vi "Path Generator.vi"() -> ()   [LabVIEW 2016]
uses:
  VIs/Waypoint.ctl
  VIs/Segment.ctl
  Constants/Private/Private Global.vi
  Pathfinder.lvlib
  Constants/Constants.lvlib
panel:
  in  "Name":string
  out "original":T1[](array[typedef])
  in  "Rear First?":bool=TRUE
  out "left":T1[](array[typedef])=[{"dt"=0.005, "x"=-0.0008758536007823281, "y"=232.00000002739714, "position"=-5.8139534883720933e-05, "velocity"=-0.023255813953488372, "acceleration"=-4.651162790697675, "jerk"=-930.232558139535, "heading"=-6.283122746208061}, {"dt"=0.005, "x"=-0.0008602070905170062, "y"=232.00000002642702, "position"=-7.378604517911754e-05, "velocity"=-0.003129302059079322, "acceleration"=4.02530237888181, "jerk"=1735.293033915897, "heading"=-6.2831238638159395}, {"dt"=0.005, "x"=-0.00082500305296863, "y"=232.0000000243082, "position"=-0.00010899008279125573, "velocity"=-0.007040807522427639, "acceleration"=-0.7823010926696634, "jerk"=-961.5206943102947, "heading"=-6.283126378390055}, {"dt"=0.005, "x"=-0.0007624201846368434, "y"=232.00000002076015, "position"=-0.0001715729512236183, "velocity"=-0.012516573686472514, "acceleration"=-1.095153232808975, "jerk"=-62.57042802786232, "heading"=-6.283130848594943}, {"dt"=0.005, "x"=-0.0006646398015586345, "y"=232.00000001577664, "position"=-0.0002693533344288234, "velocity"=-0.019556076641041014, "acceleration"=-1.4079005909137, "jerk"=-62.54947162094497, "heading"=-6.283137832908029}, {"dt"=0.005, "x"=-0.0005238475090722906, "y"=232.00000000980057, "position"=-0.0004101456270419971, "velocity"=-0.02815845852263474, "acceleration"=-1.7204763763187447, "jerk"=-62.515157081008965, "heading"=-6.283147889500358}, {"dt"=0.005, "x"=-0.00033223528885417756, "y"=232.00000000394215, "position"=-0.000601757847349669, "velocity"=-0.038322444061534386, "acceleration"=-2.0327971077799294, "jerk"=-62.46414629223693, "heading"=-6.283161576087523}, {"dt"=0.005, "x"=-8.200400317489167e-05, "y"=232.00000000024016, "position"=-0.000851989133056339, "velocity"=-0.05004625714133398, "acceleration"=-2.3447626159599193, "jerk"=-62.39310163599798, "heading"=-6.283179449750788}, {"dt"=0.005, "x"=0.0037243748096527536, "y"=232.0000000312099, "position"=-0.0046583679460099735, "velocity"=-0.7612757625907269, "acceleration"=-142.24590108987857, "jerk"=-27980.22769478373, "heading"=-1.6759390957965525e-05}, {"dt"=0.005, "x"=0.009929139702494224, "y"=232.00000022180532, "position"=-0.01086313284177876, "velocity"=-1.2409529791537575, "acceleration"=-95.9354433126061, "jerk"=9262.091555454495, "heading"=-4.4674576916869935e-05}, {"dt"=0.005, "x"=0.017436765282922654, "y"=232.00000068396733, "position"=-0.018370758436432308, "velocity"=-1.5015251189307095, "acceleration"=-52.114427955390404, "jerk"=8764.203071443138, "heading"=-7.844169176274285e-05}, {"dt"=0.005, "x"=0.02637126360589169, "y"=232.00000156426964, "position"=-0.027305256802768758, "velocity"=-1.78689967326729, "acceleration"=-57.074910867316085, "jerk"=-992.0965823851361, "heading"=-0.00011861272284025004}, {"dt"=0.005, "x"=0.0368565745058633, "y"=232.00000305503744, "position"=-0.03779056780871665, "velocity"=-2.097062201189579, "acceleration"=-62.03250558445781, "jerk"=-991.5189434283448, "heading"=-0.00016573742479814024}, {"dt"=0.005, "x"=0.04901668599989321, "y"=232.00000540258077, "position"=-0.04995067952934644, "velocity"=-2.432022344125958, "acceleration"=-66.99202858727577, "jerk"=-991.904600563592, "heading"=-0.00022036351598547776}, {"dt"=0.005, "x"=0.06297549095104837, "y"=232.00000891604873, "position"=-0.06390948492267617, "velocity"=-2.7917610786659455, "acceleration"=-71.94774690799753, "jerk"=-991.1436641443515, "heading"=-0.0002830356608759521}, {"dt"=0.005, "x"=0.07879481410486276, "y"=232.00001395498225, "position"=-0.07972880887901701, "velocity"=-3.163864791268167, "acceleration"=-74.42074252044435, "jerk"=-494.5991224893646, "heading"=-0.00035401708800802956}, {"dt"=0.005, "x"=0.09647442256013375, "y"=232.0000209147114, "position"=-0.09740841870416642, "velocity"=-3.5359219650298797, "acceleration"=-74.41143475234249, "jerk"=1.861553620372547, "heading"=-0.0004332902398125893}, {"dt"=0.005, "x"=0.11601398667715579, "y"=232.00003023642586, "position"=-0.11694798504473743, "velocity"=-3.9079132681142026, "acceleration"=-74.39826061686459, "jerk"=2.6348270955793396, "heading"=-0.0005208351885473417}, {"dt"=0.005, "x"=0.1374132670186076, "y"=232.00004240705323, "position"=-0.13834726884715046, "velocity"=-4.279856760482604, "acceleration"=-74.38869847368021, "jerk"=1.9124286368764842, "heading"=-0.000616630476134028}, {"dt"=0.005, "x"=0.16067187478210984, "y"=232.00005795891641, "position"=-0.16160588181002714, "velocity"=-4.651722592575338, "acceleration"=-74.37316641854679, "jerk"=3.106411026683986, "heading"=-0.0007206520430999008}, {"dt"=0.005, "x"=0.18578949376598203, "y"=232.00007746960773, "position"=-0.1867235083715885, "velocity"=-5.02352531231227, "acceleration"=-74.3605439473864, "jerk"=2.5244942320767905, "heading"=-0.0008328742248462917}, {"dt"=0.005, "x"=0.21276571116641288, "y"=232.00010156161397, "position"=-0.21369973653010008, "velocity"=-5.395245631702316, "acceleration"=-74.34406387800934, "jerk"=3.2960138754134505, "heading"=-0.0009532689972410191}, {"dt"=0.005, "x"=0.24160009922129633, "y"=232.0001309020737, "position"=-0.24253413951268638, "velocity"=-5.76688059651726, "acceleration"=-74.32699296298874, "jerk"=3.414183004119309, "heading"=-0.001081806344908287}, {"dt"=0.005, "x"=0.27229221516971464, "y"=232.00016620247234, "position"=-0.2732262757613951, "velocity"=-6.138427249741739, "acceleration"=-74.30933064489587, "jerk"=3.532463618574866, "heading"=-0.0012184542638269957}, {"dt"=0.005, "x"=0.30484160120819287, "y"=232.0002082183179, "position"=-0.30577568891759743, "velocity"=-6.509882631240475, "acceleration"=-74.29107629974716, "jerk"=3.6508690297409885, "heading"=-0.0013631787640525084}, {"dt"=0.005, "x"=0.33924770411668914, "y"=232.00025774867527, "position"=-0.3401818274775454, "velocity"=-6.881227711989586, "acceleration"=-74.26901614982224, "jerk"=4.412029984985111, "heading"=-0.0015159435161616885}, {"dt"=0.005, "x"=0.3755100406127911, "y"=232.00031563601584, "position"=-0.3764442101778138, "velocity"=-7.2524765400536815, "acceleration"=-74.24976561281902, "jerk"=3.85010740064331, "heading"=-0.0016767105896903223}, {"dt"=0.005, "x"=0.4136279823684332, "y"=232.0003827655038, "position"=-0.4145622110442637, "velocity"=-7.623600173289979, "acceleration"=-74.22472664725959, "jerk"=5.007793111886372, "heading"=-0.0018454395028453252}, {"dt"=0.005, "x"=0.4536009877800924, "y"=232.00046006494864, "position"=-0.45453529119634495, "velocity"=-7.994616030416249, "acceleration"=-74.20317142525387, "jerk"=4.311044401143249, "heading"=-0.0020220882541658325}, {"dt"=0.005, "x"=0.49542842005744236, "y"=232.0005485040674, "position"=-0.49636281697057677, "velocity"=-8.365505154846364, "acceleration"=-74.17782488602302, "jerk"=5.069307846170545, "heading"=-0.002206612520756379}, {"dt"=0.005, "x"=0.5391096274920242, "y"=232.0006490941584, "position"=-0.5400441402255948, "velocity"=-8.73626465100359, "acceleration"=-74.15189923144538, "jerk"=5.18513091552677, "heading"=-0.0023989660184867145}, {"dt"=0.005, "x"=0.5846439433956321, "y"=232.0007628876348, "position"=-0.5855785983179541, "velocity"=-9.106891618471872, "acceleration"=-74.12539349365623, "jerk"=5.301147557830177, "heading"=-0.0025991005059064487}, {"dt"=0.005, "x"=0.6320306093513414, "y"=232.0008909773236, "position"=-0.6329654373913335, "velocity"=-9.477367814675867, "acceleration"=-74.09523924079906, "jerk"=6.030850571434598, "heading"=-0.0028069654522328014}, {"dt"=0.005, "x"=0.6812689450670211, "y"=232.0010344963924, "position"=-0.6822039822700471, "velocity"=-9.84770897574272, "acceleration"=-74.06823221337042, "jerk"=5.401405485727651, "heading"=-0.0030225087880748625}, {"dt"=0.005, "x"=0.7323581382320017, "y"=232.00119461724273, "position"=-0.7332934263552533, "velocity"=-10.21788881704124, "acceleration"=-74.03596825970418, "jerk"=6.452790733249003, "heading"=-0.0032456759888707665}, {"dt"=0.005, "x"=0.7852974359433659, "y"=232.0013725515007, "position"=-0.786233023093164, "velocity"=-10.587919347582151, "acceleration"=-74.00610610818212, "jerk"=5.972430304410636, "heading"=-0.0034764109186699033}, {"dt"=0.005, "x"=0.8400859939140858, "y"=232.00156954897838, "position"=-0.8410219352243348, "velocity"=-10.957782426234143, "acceleration"=-73.97261573039842, "jerk"=6.698075556741401, "heading"=-0.003714655176530801}, {"dt"=0.005, "x"=0.8967229530826379, "y"=232.00178689730362, "position"=-0.897659311436115, "velocity"=-11.327475242356043, "acceleration"=-73.9385632243799, "jerk"=6.810501203702302, "heading"=-0.0039603484374847175}, {"dt"=0.005, "x"=0.95520743953518, "y"=232.00202592131672, "position"=-0.9561442863279315, "velocity"=-11.6969949783633, "acceleration"=-73.90394720145146, "jerk"=6.923204585689291, "heading"=-0.004213428457558621}, {"dt"=0.005, "x"=1.0155385644244324, "y"=232.00228798244848, "position"=-1.016475980373759, "velocity"=-12.066338809165526, "acceleration"=-73.86876616044518, "jerk"=7.0362082012565, "heading"=-0.004473831078898705}, {"dt"=0.005, "x"=1.0777153566651037, "y"=232.00257447776232, "position"=-1.0786534326607775, "velocity"=-12.435490457403692, "acceleration"=-73.83032964763316, "jerk"=7.687302562402465, "heading"=-0.004741489946012034}, {"dt"=0.005, "x"=1.1417368807834196, "y"=232.0028868397957, "position"=-1.1426757187842207, "velocity"=-12.804457224688617, "acceleration"=-73.79335345698514, "jerk"=7.395238129603854, "heading"=-0.005016337020701256}, {"dt"=0.005, "x"=1.2076021049041703, "y"=232.0032265352529, "position"=-1.208541818877367, "velocity"=-13.17322001862925, "acceleration"=-73.75255878812652, "jerk"=8.158933771724719, "heading"=-0.005298302020654566}, {"dt"=0.005, "x"=1.2753100465120997, "y"=232.00359506500843, "position"=-1.2762507634191589, "velocity"=-13.541788908358415, "acceleration"=-73.71377794583296, "jerk"=7.756168458712409, "heading"=-0.005587313051794995}, {"dt"=0.005, "x"=1.3448596413212155, "y"=232.00399396271462, "position"=-1.3458015021463083, "velocity"=-13.910147745429873, "acceleration"=-73.67176741429162, "jerk"=8.40210630826732, "heading"=-0.0058832960532334555}, {"dt"=0.005, "x"=1.4162498104026864, "y"=232.00442479438698, "position"=-1.4171929712263807, "velocity"=-14.278293816014447, "acceleration"=-73.62921411691481, "jerk"=8.510659475362559, "heading"=-0.006186175092258439}, {"dt"=0.005, "x"=1.4894794600891537, "y"=232.0048891576535, "position"=-1.490424093206356, "velocity"=-14.646224395995057, "acceleration"=-73.5861159961221, "jerk"=8.619624158541228, "heading"=-0.0064958723704272026}, {"dt"=0.005, "x"=1.5645474301298237, "y"=232.00538868063467, "position"=-1.5654937252104868, "velocity"=-15.01392640082618, "acceleration"=-73.5404009662247, "jerk"=9.1430059794817, "heading"=-0.006812308011973578}, {"dt"=0.005, "x"=1.6414525699167895, "y"=232.0059250216199, "position"=-1.6424007352115602, "velocity"=-15.381402000214662, "acceleration"=-73.49511987769617, "jerk"=9.056217705705194, "heading"=-0.007135400393883662}, {"dt"=0.005, "x"=1.7201936916842042, "y"=232.006499867955, "position"=-1.7211439552720822, "velocity"=-15.748644012104426, "acceleration"=-73.44840237795296, "jerk"=9.34349994864192, "heading"=-0.007465065955438832}, {"dt"=0.005, "x"=1.8007695950493774, "y"=232.00711493537773, "position"=-1.801722206128304, "velocity"=-16.115650171244383, "acceleration"=-73.40123182799125, "jerk"=9.434109992341178, "heading"=-0.007801219309015173}, {"dt"=0.005, "x"=1.8831790136592212, "y"=232.00777196675085, "position"=-1.884134243876668, "velocity"=-16.482407549672768, "acceleration"=-73.35147568567706, "jerk"=9.951228462838912, "heading"=-0.008143773025622747}, {"dt"=0.005, "x"=1.9674206668309744, "y"=232.00847273155964, "position"=-1.9683788116565977, "velocity"=-16.84891355598595, "acceleration"=-73.30120126263608, "jerk"=10.054884608194925, "heading"=-0.008492637859500662}, {"dt"=0.005, "x"=2.053493259443463, "y"=232.00921902504075, "position"=-2.0544546395817207, "velocity"=-17.215165585024632, "acceleration"=-73.25040580773674, "jerk"=10.159090979868779, "heading"=-0.008847722755006282}, {"dt"=0.005, "x"=2.1413954818246905, "y"=232.01001266729526, "position"=-2.1423604446664073, "velocity"=-17.58116101693729, "acceleration"=-73.19908638253168, "jerk"=10.263885041013054, "heading"=-0.009208934853559114}, {"dt"=0.005, "x"=2.2311259871620055, "y"=232.01085550217056, "position"=-2.2320949082727437, "velocity"=-17.9468927212673, "acceleration"=-73.14634086600194, "jerk"=10.549103305947938, "heading"=-0.009576179408844698}, {"dt"=0.005, "x"=2.3226833391094157, "y"=232.01174939578001, "position"=-2.3236566237514684, "velocity"=-18.31234309574498, "acceleration"=-73.09007489553565, "jerk"=11.25319409325698, "heading"=-0.009949359583154571}, {"dt"=0.005, "x"=2.416066177758609, "y"=232.01269623714148, "position"=-2.4170442624556623, "velocity"=-18.677527740838777, "acceleration"=-73.03692901875962, "jerk"=10.629175355205689, "heading"=-0.010328377133728417}, {"dt"=0.005, "x"=2.511273061021889, "y"=232.0136979357001, "position"=-2.5122564151501066, "velocity"=-19.042430538888823, "acceleration"=-72.98055961000927, "jerk"=11.273881750071268, "heading"=-0.010713131773046225}, {"dt"=0.005, "x"=2.608302510440957, "y"=232.01475642074277, "position"=-2.6092916378537883, "velocity"=-19.407044540736322, "acceleration"=-72.9228003694999, "jerk"=11.55184810187393, "heading"=-0.011103521366487179}, {"dt"=0.005, "x"=2.7071530335398117, "y"=232.0158736406307, "position"=-2.7081484742243456, "velocity"=-19.771367274111487, "acceleration"=-72.86454667503293, "jerk"=11.650738893393964, "heading"=-0.01149944203158998}, {"dt"=0.005, "x"=2.8078231236998734, "y"=232.01705156180276, "position"=-2.8088254554619776, "velocity"=-20.135396247526423, "acceleration"=-72.80579468298711, "jerk"=11.750398409162699, "heading"=-0.011900788145544128}, {"dt"=0.005, "x"=2.9103112600310195, "y"=232.0182921677638, "position"=-2.9113211002074113, "velocity"=-20.499128949086746, "acceleration"=-72.74654031206467, "jerk"=11.850874184489157, "heading"=-0.012307452352702253}, {"dt"=0.005, "x"=3.014615802597889, "y"=232.0195974567277, "position"=-3.0156338097847355, "velocity"=-20.862541915464828, "acceleration"=-72.68259327561637, "jerk"=12.789407289659493, "heading"=-0.012719325159919415}, {"dt"=0.005, "x"=3.1207352416957805, "y"=232.02096944363532, "position"=-3.121762117518939, "velocity"=-21.225661546840698, "acceleration"=-72.623926275174, "jerk"=11.7334000884739, "heading"=-0.013136295931937603}, {"dt"=0.005, "x"=3.2286678828591016, "y"=232.02241015513147, "position"=-3.229704373740056, "velocity"=-21.588451244223464, "acceleration"=-72.5579394765532, "jerk"=13.197359724159696, "heading"=-0.013558251657072029}, {"dt"=0.005, "x"=3.3384121057881533, "y"=232.02392163175864, "position"=-3.3394590047489383, "velocity"=-21.950926201776443, "acceleration"=-72.49499151059595, "jerk"=12.589593191449922, "heading"=-0.013985077976886029}, {"dt"=0.005, "x"=3.4499662436546443, "y"=232.0255059253226, "position"=-3.451024392128864, "velocity"=-22.313077475985125, "acceleration"=-72.43025484173629, "jerk"=12.947333771933245, "heading"=-0.014416658719868247}, {"dt"=0.005, "x"=3.5633285981346616, "y"=232.02716509795124, "position"=-3.5643988877928567, "velocity"=-22.674899132798593, "acceleration"=-72.36433136269369, "jerk"=13.184695808519109, "heading"=-0.014852875970709278}, {"dt"=0.005, "x"=3.6784974020173635, "y"=232.02890122037624, "position"=-3.679580776598549, "velocity"=-23.036377761138443, "acceleration"=-72.29572566796989, "jerk"=13.721138944760014, "heading"=-0.015293609937738706}, {"dt"=0.005, "x"=3.7954709407839147, "y"=232.03071637260283, "position"=-3.7965683979487395, "velocity"=-23.397524270038073, "acceleration"=-72.22930177992595, "jerk"=13.284777608788545, "heading"=-0.015738739428503346}, {"dt"=0.005, "x"=3.914247437266812, "y"=232.03261264105586, "position"=-3.915360030443616, "velocity"=-23.758326498975247, "acceleration"=-72.16044578743492, "jerk"=13.77119849820474, "heading"=-0.016188141415762913}, {"dt"=0.005, "x"=4.034825082010761, "y"=232.03459211782888, "position"=-4.035953922247027, "velocity"=-24.118778360682324, "acceleration"=-72.09037234141533, "jerk"=14.014689203918351, "heading"=-0.01664169116497438}, {"dt"=0.005, "x"=4.157202017359324, "y"=232.0366568992095, "position"=-4.158348275170093, "velocity"=-24.47887058461313, "acceleration"=-72.01844478616124, "jerk"=14.385511050818423, "heading"=-0.01709926218535751}, {"dt"=0.005, "x"=4.28137642432246, "y"=232.0388090859533, "position"=-4.282541331547761, "velocity"=-24.838611275533633, "acceleration"=-71.94813818410069, "jerk"=14.061320412110945, "heading"=-0.017560726563973728}, {"dt"=0.005, "x"=4.40734641963408, "y"=232.041050780364, "position"=-4.408531271275664, "velocity"=-25.197987945580614, "acceleration"=-71.87533400939614, "jerk"=14.560834940908762, "heading"=-0.018025954589003357}, {"dt"=0.005, "x"=4.535110106951593, "y"=232.04338408592685, "position"=-4.536316263007153, "velocity"=-25.55699834629788, "acceleration"=-71.8020801434534, "jerk"=14.650773188549238, "heading"=-0.01849481495111488}, {"dt"=0.005, "x"=4.664665502149558, "y"=232.04581110468416, "position"=-4.665894389421101, "velocity"=-25.915625282789705, "acceleration"=-71.72538729836475, "jerk"=15.338569017728787, "heading"=-0.018967174480118587}, {"dt"=0.005, "x"=4.796010725282278, "y"=232.0483339395721, "position"=-4.797263839201695, "velocity"=-26.273889956118634, "acceleration"=-71.65293466578575, "jerk"=14.490526515800184, "heading"=-0.019442898855028645}, {"dt"=0.005, "x"=4.929143750482188, "y"=232.05095468848643, "position"=-4.930422656873496, "velocity"=-26.631763534360207, "acceleration"=-71.57471564831468, "jerk"=15.643803494214126, "heading"=-0.019921851701201476}, {"dt"=0.005, "x"=5.064062616109224, "y"=232.0536754470116, "position"=-5.065368952965825, "velocity"=-26.989259218465765, "acceleration"=-71.49913682111162, "jerk"=15.115765440611995, "heading"=-0.02040389536281534}, {"dt"=0.005, "x"=5.200765274045972, "y"=232.05649830420577, "position"=-5.2021007532527745, "velocity"=-27.346360057389894, "acceleration"=-71.42016778482585, "jerk"=15.793807257153958, "heading"=-0.020888890368426838}, {"dt"=0.005, "x"=5.339249664073405, "y"=232.05942534274948, "position"=-5.340616073112733, "velocity"=-27.703063971991547, "acceleration"=-71.34078292033053, "jerk"=15.876972899064867, "heading"=-0.021376695709081128}, {"dt"=0.005, "x"=5.479513713696131, "y"=232.06245863766975, "position"=-5.480912917320434, "velocity"=-28.059368841540277, "acceleration"=-71.26097390974593, "jerk"=15.961802116919444, "heading"=-0.021867168845404295}, {"dt"=0.005, "x"=5.621555337961084, "y"=232.0656002550529, "position"=-5.622989279828798, "velocity"=-28.415272501672856, "acceleration"=-71.18073202651587, "jerk"=16.048376646011775, "heading"=-0.02236016571457}, {"dt"=0.005, "x"=5.7653724392696315, "y"=232.06885225074691, "position"=-5.766843143540506, "velocity"=-28.77077274234173, "acceleration"=-71.10004813377486, "jerk"=16.13677854820139, "heading"=-0.022855540737134694}, {"dt"=0.005, "x"=5.910962833735542, "y"=232.07221666733747, "position"=-5.912472406601659, "velocity"=-29.125852612230506, "acceleration"=-71.01597397775521, "jerk"=16.81483120393068, "heading"=-0.02335314657368609}, {"dt"=0.005, "x"=6.058324406713837, "y"=232.0756955363611, "position"=-6.059875037922544, "velocity"=-29.48052626417701, "acceleration"=-70.93473038930043, "jerk"=16.248717690956482, "heading"=-0.023852834667305756}, {"dt"=0.005, "x"=6.207454896354211, "y"=232.07929087191326, "position"=-6.209048860619793, "velocity"=-29.834764539449775, "acceleration"=-70.84765505455337, "jerk"=17.415066949411084, "heading"=-0.02435445451454049}, {"dt"=0.005, "x"=6.358352145790647, "y"=232.0830046752474, "position"=-6.359991804219972, "velocity"=-30.188588720035764, "acceleration"=-70.76483611719766, "jerk"=16.563787471142177, "heading"=-0.024857854528733958}, {"dt"=0.005, "x"=6.511013914784371, "y"=232.08683892894962, "position"=-6.512701716189517, "velocity"=-30.541982393908977, "acceleration"=-70.67873477464275, "jerk"=17.22026851098235, "heading"=-0.025362881410148364}, {"dt"=0.005, "x"=6.665437951155562, "y"=232.09079559725666, "position"=-6.667176433322331, "velocity"=-30.894943426562786, "acceleration"=-70.59220653076181, "jerk"=17.3056487761869, "heading"=-0.025869380395809882}, {"dt"=0.005, "x"=6.821621942756571, "y"=232.09487662342906, "position"=-6.823413733628769, "velocity"=-31.24746006128742, "acceleration"=-70.50332694492667, "jerk"=17.775917167028865, "heading"=-0.026377195110501683}, {"dt"=0.005, "x"=6.979563621943135, "y"=232.09908393107014, "position"=-6.981411440769911, "velocity"=-31.599541428228484, "acceleration"=-70.41627338821286, "jerk"=17.410711342762397, "heading"=-0.02688616791512355}, {"dt"=0.005, "x"=7.139260666788392, "y"=232.10341942018542, "position"=-7.14116732516287, "velocity"=-31.95117687859191, "acceleration"=-70.32709007268494, "jerk"=17.83666310558374, "heading"=-0.02739613959058068}, {"dt"=0.005, "x"=7.300710736537575, "y"=232.10788496667857, "position"=-7.302679139366967, "velocity"=-32.302362840819406, "acceleration"=-70.23719244549937, "jerk"=17.979525437112898, "heading"=-0.027906949461475872}, {"dt"=0.005, "x"=7.463911432514355, "y"=232.11248241982824, "position"=-7.465944578890367, "velocity"=-32.653087904679886, "acceleration"=-70.14501277209604, "jerk"=18.435934680667287, "heading"=-0.02841843528086402}, {"dt"=0.005, "x"=7.6288604046938335, "y"=232.1172136038516, "position"=-7.630961388716909, "velocity"=-33.00336196530847, "acceleration"=-70.05481212571709, "jerk"=18.04012927578924, "heading"=-0.02893043357182906}, {"dt"=0.005, "x"=7.795555243613974, "y"=232.1220803134656, "position"=-7.797727255083736, "velocity"=-33.35317327336539, "acceleration"=-69.96226161138424, "jerk"=18.510102866571287, "heading"=-0.029442779292969234}, {"dt"=0.005, "x"=7.963993521310489, "y"=232.12708431357262, "position"=-7.966239846335665, "velocity"=-33.70251825038574, "acceleration"=-69.86899540406881, "jerk"=18.65324146308467, "heading"=-0.02995530597451057}, {"dt"=0.005, "x"=8.134172755342203, "y"=232.13222733672063, "position"=-8.13649677683402, "velocity"=-34.05138609967093, "acceleration"=-69.77356985703835, "jerk"=19.08510940609176, "heading"=-0.030467845616262257}, {"dt"=0.005, "x"=8.306090538201579, "y"=232.13751108556986, "position"=-8.30849573632269, "velocity"=-34.39979189773406, "acceleration"=-69.68115961262669, "jerk"=18.4820488823334, "heading"=-0.030980229082420263}, {"dt"=0.005, "x"=8.47974432712428, "y"=232.14293722505158, "position"=-8.48223427953313, "velocity"=-34.747708642087595, "acceleration"=-69.58334887070663, "jerk"=19.56214838401138, "heading"=-0.03149228547556426}, {"dt"=0.005, "x"=8.65513165873618, "y"=232.14850738747435, "position"=-8.657710040820431, "velocity"=-35.09515225746054, "acceleration"=-69.48872307458913, "jerk"=18.925159223499577, "heading"=-0.03200384278277996}, {"dt"=0.005, "x"=8.832249986433196, "y"=232.1542231660108, "position"=-8.834920571349702, "velocity"=-35.44210610585407, "acceleration"=-69.39076967870648, "jerk"=19.59067917653101, "heading"=-0.03251472739815203}, {"dt"=0.005, "x"=9.011096753948054, "y"=232.1600861154812, "position"=-9.01386341257842, "velocity"=-35.78856824574363, "acceleration"=-69.29242797791204, "jerk"=19.668340158887077, "heading"=-0.033024764346155366}, {"dt"=0.005, "x"=9.191669395060012, "y"=232.16609775087773, "position"=-9.194536095843734, "velocity"=-36.13453665306298, "acceleration"=-69.19368146386944, "jerk"=19.749302808520497, "heading"=-0.033533777283453525}, {"dt"=0.005, "x"=9.373965333293208, "y"=232.17225954588017, "position"=-9.376936141934664, "velocity"=-36.48000921818594, "acceleration"=-69.09451302459217, "jerk"=19.83368785545281, "heading"=-0.034041588500349274}, {"dt"=0.005, "x"=9.557981981603383, "y"=232.17857293136328, "position"=-9.561061060649022, "velocity"=-36.82498374287164, "acceleration"=-68.99490493713927, "jerk"=19.92161749058141, "heading"=-0.03454801892188025}, {"dt"=0.005, "x"=9.743716677291463, "y"=232.1850392916245, "position"=-9.746908285533795, "velocity"=-37.16944497695459, "acceleration"=-68.89224681658987, "jerk"=20.53162410987852, "heading"=-0.03505288793361572}, {"dt"=0.005, "x"=9.931166827296574, "y"=232.19165996789127, "position"=-9.93447531912757, "velocity"=-37.51340671875481, "acceleration"=-68.79234836004429, "jerk"=19.979691309117698, "heading"=-0.03555601378151152}, {"dt"=0.005, "x"=10.120329712999787, "y"=232.19843624997839, "position"=-10.123759537504304, "velocity"=-37.85684367534683, "acceleration"=-68.68739131840442, "jerk"=20.99140832797275, "heading"=-0.036057213045198655}, {"dt"=0.005, "x"=10.311202693907404, "y"=232.2053693819383, "position"=-10.314758393938925, "velocity"=-38.199771286924374, "acceleration"=-68.58552231550874, "jerk"=20.373800579136514, "heading"=-0.0365563011874076}, {"dt"=0.005, "x"=10.503783070481315, "y"=232.21246055568147, "position"=-10.507469281504743, "velocity"=-38.542177513163494, "acceleration"=-68.48124524782406, "jerk"=20.85541353693543, "heading"=-0.03705309218711178}, {"dt"=0.005, "x"=10.69806813000994, "y"=232.21971091105453, "position"=-10.701889578822376, "velocity"=-38.88405946352661, "acceleration"=-68.3763900726234, "jerk"=20.971035040133756, "heading"=-0.03754739866352075}, {"dt"=0.005, "x"=10.894055118378315, "y"=232.22712153322956, "position"=-10.898016621656165, "velocity"=-39.22540856675767, "acceleration"=-68.26982064621205, "jerk"=21.313885282268075, "heading"=-0.03803903180539625}, {"dt"=0.005, "x"=11.091741299506669, "y"=232.23469345338236, "position"=-11.095847762238007, "velocity"=-39.56622811636853, "acceleration"=-68.16390992217123, "jerk"=21.18214480816505, "heading"=-0.03852780152119517}, {"dt"=0.005, "x"=11.291123919607498, "y"=232.24242764582416, "position"=-11.295380333341068, "velocity"=-39.90651422061238, "acceleration"=-68.05722084877033, "jerk"=21.337814680180145, "heading"=-0.03901351634569983}, {"dt"=0.005, "x"=11.492200174596395, "y"=232.25032502514583, "position"=-11.496611615502937, "velocity"=-40.24625643237385, "acceleration"=-67.94844235229363, "jerk"=21.75569929534049, "heading"=-0.03949598336140597}, {"dt"=0.005, "x"=11.69496725951251, "y"=232.25838644654192, "position"=-11.699538886317642, "velocity"=-40.58545416294082, "acceleration"=-67.83954611339453, "jerk"=21.779247779818434, "heading"=-0.03997500831889661}, {"dt"=0.005, "x"=11.899422370613742, "y"=232.26661270435605, "position"=-11.904159422366792, "velocity"=-40.924107209830176, "acceleration"=-67.73060937787108, "jerk"=21.787347104691435, "heading"=-0.04045039563659941}, {"dt"=0.005, "x"=12.105562668398935, "y"=232.2750045290249, "position"=-12.11047046204291, "velocity"=-41.26220793522368, "acceleration"=-67.62014507870049, "jerk"=22.092859834117462, "heading"=-0.040921948310822076}, {"dt"=0.005, "x"=12.313385304065063, "y"=232.28356258653767, "position"=-12.318469231855637, "velocity"=-41.59975396254553, "acceleration"=-67.50920546436987, "jerk"=22.1879228661237, "heading"=-0.0413894679751019}, {"dt"=0.005, "x"=12.522887390519298, "y"=232.2922874756424, "position"=-12.528152917245244, "velocity"=-41.93673707792135, "acceleration"=-67.39662307516454, "jerk"=22.516477841065807, "heading"=-0.04185275483144346}, {"dt"=0.005, "x"=12.734066052780351, "y"=232.3011797283262, "position"=-12.73951871285125, "velocity"=-42.27315912120136, "acceleration"=-67.28440865600192, "jerk"=22.44288383252524, "heading"=-0.042311607758638736}, {"dt"=0.005, "x"=12.946918397050695, "y"=232.31023980694772, "position"=-12.952563791381614, "velocity"=-42.6090157060729, "acceleration"=-67.17131697430858, "jerk"=22.618336338666722, "heading"=-0.042765824236329686}, {"dt"=0.005, "x"=13.161441504538459, "y"=232.3194681023479, "position"=-13.167285297249563, "velocity"=-42.944301173589984, "acceleration"=-67.05709350341635, "jerk"=22.84469417844548, "heading"=-0.04321520032698328}, {"dt"=0.005, "x"=13.377632416159262, "y"=232.3288649315395, "position"=-13.38368033107957, "velocity"=-43.27900676600132, "acceleration"=-66.9411184822664, "jerk"=23.19500422998999, "heading"=-0.04365953064015782}, {"dt"=0.005, "x"=13.595488206038283, "y"=232.33843053926833, "position"=-13.601746023096984, "velocity"=-43.613138403482964, "acceleration"=-66.82632749632944, "jerk"=22.95819718739267, "heading"=-0.04409860847703356}, {"dt"=0.005, "x"=13.815005905858886, "y"=232.34816509311503, "position"=-13.821479457223706, "velocity"=-43.946686825344464, "acceleration"=-66.70968437230016, "jerk"=23.32862480585618, "heading"=-0.044532225665005754}, {"dt"=0.005, "x"=14.036182524213768, "y"=232.35806868266545, "position"=-14.042877690262916, "velocity"=-44.27964660784193, "acceleration"=-66.59195649949368, "jerk"=23.54557456129669, "heading"=-0.0449601725916855}, {"dt"=0.005, "x"=14.259015056293384, "y"=232.3681413182868, "position"=-14.265937761412761, "velocity"=-44.612014229968956, "acceleration"=-66.47352442540466, "jerk"=23.68641481780287, "heading"=-0.045382238215472714}, {"dt"=0.005, "x"=14.483500519658685, "y"=232.37838293111682, "position"=-14.490656727892437, "velocity"=-44.94379329593529, "acceleration"=-66.35581319326747, "jerk"=23.542246427439295, "heading"=-0.045798210120846394}, {"dt"=0.005, "x"=14.709635837903399, "y"=232.38879336610046, "position"=-14.717031548299182, "velocity"=-45.27496408134917, "acceleration"=-66.23415708277491, "jerk"=24.331222098510352, "heading"=-0.04620787429158624}, {"dt"=0.005, "x"=14.937418003242483, "y"=232.39937238774368, "position"=-14.945059245181579, "velocity"=-45.60553937647911, "acceleration"=-66.11505902598793, "jerk"=23.819611357396298, "heading"=-0.04661101540011764}, {"dt"=0.005, "x"=15.166843942263128, "y"=232.4101196722917, "position"=-15.17473677046575, "velocity"=-45.93550505683414, "acceleration"=-65.99313607100612, "jerk"=24.384590996362476, "heading"=-0.0470074165486688}, {"dt"=0.005, "x"=15.397910572260642, "y"=232.42103480861653, "position"=-15.406061061666215, "velocity"=-46.264858240093005, "acceleration"=-65.8706366517734, "jerk"=24.49988384654489, "heading"=-0.04739685936065724}, {"dt"=0.005, "x"=15.630614800556488, "y"=232.43211729650523, "position"=-15.639029041020821, "velocity"=-46.59359587092137, "acceleration"=-65.74752616567281, "jerk"=24.62209722011721, "heading"=-0.04777912396457673}, {"dt"=0.005, "x"=15.864953523793961, "y"=232.44336654493742, "position"=-15.873637614604265, "velocity"=-46.92171471668871, "acceleration"=-65.62376915346846, "jerk"=24.75140244087015, "heading"=-0.048153988977164996}, {"dt"=0.005, "x"=16.100923627211305, "y"=232.45478187035107, "position"=-16.109883671420228, "velocity"=-47.24921136319276, "acceleration"=-65.499329300809, "jerk"=24.887970531892734, "heading"=-0.048521231485842475}, {"dt"=0.005, "x"=16.338521934198965, "y"=232.46636249246657, "position"=-16.347764032719738, "velocity"=-47.57607225990164, "acceleration"=-65.37217934177733, "jerk"=25.429991806333874, "heading"=-0.048880626956336604}, {"dt"=0.005, "x"=16.577745329194098, "y"=232.47810753853548, "position"=-16.587275574863657, "velocity"=-47.90230842878369, "acceleration"=-65.24723377640953, "jerk"=24.98911307355911, "heading"=-0.04923194940349945}, {"dt"=0.005, "x"=16.818590620295264, "y"=232.49001603492664, "position"=-16.82841509160014, "velocity"=-48.2279033472963, "acceleration"=-65.1189837025214, "jerk"=25.650014777625074, "heading"=-0.0495749711637084}, {"dt"=0.005, "x"=17.061054613836543, "y"=232.50208690900453, "position"=-17.07117936855412, "velocity"=-48.5528553907963, "acceleration"=-64.99040870000101, "jerk"=25.71500050407849, "heading"=-0.049909462990579245}, {"dt"=0.005, "x"=17.30513411636937, "y"=232.51431898750369, "position"=-17.315565185043297, "velocity"=-48.87716329783543, "acceleration"=-64.8615814078255, "jerk"=25.765458435103028, "heading"=-0.05023519403457111}, {"dt"=0.005, "x"=17.550825903190383, "y"=232.52671099320244, "position"=-17.561569282400516, "velocity"=-49.20081947144375, "acceleration"=-64.73123472166407, "jerk"=26.069337232286216, "heading"=-0.050551931778636094}, {"dt"=0.005, "x"=17.798126726314784, "y"=232.5392615435357, "position"=-17.809188371793226, "velocity"=-49.52381787854173, "acceleration"=-64.59968141959536, "jerk"=26.31066041374197, "heading"=-0.05085944202959397}, {"dt"=0.005, "x"=18.047033349946975, "y"=232.55196915062186, "position"=-18.058419169580805, "velocity"=-49.8461595575159, "acceleration"=-64.46833579483382, "jerk"=26.269124952307266, "heading"=-0.05115748893864153}, {"dt"=0.005, "x"=18.297542490160286, "y"=232.56483221641068, "position"=-18.30925833676149, "velocity"=-50.16783343613695, "acceleration"=-64.33477572421111, "jerk"=26.712014124541383, "heading"=-0.05144583490291749}, {"dt"=0.005, "x"=18.549650871378745, "y"=232.57784903376205, "position"=-18.56170253537685, "velocity"=-50.48883972307184, "acceleration"=-64.20125738697777, "jerk"=26.703667446668078, "heading"=-0.051724240609072214}, {"dt"=0.005, "x"=18.80335516660653, "y"=232.59101778156142, "position"=-18.81574836851652, "velocity"=-50.809166627934445, "acceleration"=-64.06538097252081, "jerk"=27.175282891391817, "heading"=-0.05199246493973941}, {"dt"=0.005, "x"=19.058652069287344, "y"=232.6043365266114, "position"=-19.07139245213303, "velocity"=-51.12881672330155, "acceleration"=-63.9300190734204, "jerk"=27.07237982008337, "heading"=-0.05225026502561936}, {"dt"=0.005, "x"=19.31553823733918, "y"=232.6178032189088, "position"=-19.328631358867195, "velocity"=-51.44778134683291, "acceleration"=-63.79292470627291, "jerk"=27.41887342949667, "heading"=-0.052497396156023224}, {"dt"=0.005, "x"=19.574010311488827, "y"=232.63141569074594, "position"=-19.587461636278356, "velocity"=-51.76605548223202, "acceleration"=-63.65482707982153, "jerk"=27.61952529027667, "heading"=-0.05273361177038338}, {"dt"=0.005, "x"=19.83406490413545, "y"=232.64517165426676, "position"=-19.847879795570265, "velocity"=-52.08363185838199, "acceleration"=-63.51527522999447, "jerk"=27.91036996541152, "heading"=-0.05295866341853034}, {"dt"=0.005, "x"=20.09569863634288, "y"=232.65906870155803, "position"=-20.109882348520053, "velocity"=-52.400510589957435, "acceleration"=-63.37574631508858, "jerk"=27.905782981179073, "heading"=-0.053172300761148206}, {"dt"=0.005, "x"=20.358908081003232, "y"=232.6731042997623, "position"=-20.37346575045455, "velocity"=-52.71668038689909, "acceleration"=-63.233959388331584, "jerk"=28.357385351398534, "heading"=-0.053374271488402514}, {"dt"=0.005, "x"=20.623689813993888, "y"=232.68727579189922, "position"=-20.638626451379334, "velocity"=-53.03214018495663, "acceleration"=-63.091959611507775, "jerk"=28.39995536476181, "heading"=-0.05356432132894945}, {"dt"=0.005, "x"=20.890040374846606, "y"=232.70158039286616, "position"=-20.90536085650057, "velocity"=-53.34688102424764, "acceleration"=-62.94816785820103, "jerk"=28.758350661348686, "heading"=-0.053742193984267494}, {"dt"=0.005, "x"=21.157956288534407, "y"=232.71601518868061, "position"=-21.173665347960135, "velocity"=-53.66089829191245, "acceleration"=-62.80345353296326, "jerk"=28.942865047554278, "heading"=-0.053907631109661125}, {"dt"=0.005, "x"=21.427434062974207, "y"=232.7305771344183, "position"=-21.443536282261505, "velocity"=-53.97418686027413, "acceleration"=-62.65771367233555, "jerk"=29.147972125542765, "heading"=-0.05406037227421545}, {"dt"=0.005, "x"=21.698470180035933, "y"=232.74526305178213, "position"=-21.714969981202362, "velocity"=-54.28673978817115, "acceleration"=-62.510585579403255, "jerk"=29.425618586458313, "heading"=-0.054200154916931975}, {"dt"=0.005, "x"=21.97106110694498, "y"=232.76006962775836, "position"=-21.98796274324061, "velocity"=-54.59855240765008, "acceleration"=-62.36252389578709, "jerk"=29.612336723232602, "heading"=-0.05432671431317021}, {"dt"=0.005, "x"=22.245203282920937, "y"=232.77499341191796, "position"=-22.262510830071452, "velocity"=-54.909617366168185, "acceleration"=-62.212991703620446, "jerk"=29.906438433329186, "heading"=-0.054439783526560204}, {"dt"=0.005, "x"=22.520893122869943, "y"=232.79003081462434, "position"=-22.53861047029444, "velocity"=-55.219928044597296, "acceleration"=-62.062135685822284, "jerk"=30.17120355963243, "heading"=-0.054539093369314506}, {"dt"=0.005, "x"=22.798127022256207, "y"=232.80517810529375, "position"=-22.816257864273812, "velocity"=-55.529478795874375, "acceleration"=-61.910150255415886, "jerk"=30.397086081279667, "heading"=-0.0546243723602482}, {"dt"=0.005, "x"=23.076901352771202, "y"=232.8204314101386, "position"=-23.095449179795576, "velocity"=-55.838263104353125, "acceleration"=-61.756861695749876, "jerk"=30.65771193320188, "heading"=-0.05469534667763892}, {"dt"=0.005, "x"=23.357212459268812, "y"=232.83578670996178, "position"=-23.37618054900567, "velocity"=-56.146273842018736, "acceleration"=-61.60214753312232, "jerk"=30.94283252551122, "heading"=-0.05475174011212991}, {"dt"=0.005, "x"=23.639056662287622, "y"=232.85123983824042, "position"=-23.65844807095764, "velocity"=-56.45350439039344, "acceleration"=-61.446109674940885, "jerk"=31.207571636286957, "heading"=-0.05479327401972045}, {"dt"=0.005, "x"=23.922430256443075, "y"=232.86678647896673, "position"=-23.942247810038655, "velocity"=-56.75994781620308, "acceleration"=-61.28868516192796, "jerk"=31.484902602585407, "heading"=-0.05481966727206555}, {"dt"=0.005, "x"=24.20732950855389, "y"=232.88242216445724, "position"=-24.22757579414477, "velocity"=-57.06559682122316, "acceleration"=-61.12980100401586, "jerk"=31.776831582419618, "heading"=-0.05483063620565576}, {"dt"=0.005, "x"=24.493750659336676, "y"=232.8981422733397, "position"=-24.514428016445752, "velocity"=-57.370444460196225, "acceleration"=-60.96952779461304, "jerk"=32.054641880563395, "heading"=-0.054825894569789146}, {"dt"=0.005, "x"=24.781631949327103, "y"=232.9139388479658, "position"=-24.802742374216, "velocity"=-57.66287155404955, "acceleration"=-58.485418770665376, "jerk"=496.8218047895334, "heading"=-0.05480515926312368}, {"dt"=0.005, "x"=25.070853843731797, "y"=232.92980061535675, "position"=-25.092398894715373, "velocity"=-57.93130409987497, "acceleration"=-53.68650916508386, "jerk"=959.7819211163028, "heading"=-0.054768166503874616}, {"dt"=0.005, "x"=25.361297143228736, "y"=232.94571619285443, "position"=-25.383277934575162, "velocity"=-58.175807971957994, "acceleration"=-48.90077441660452, "jerk"=957.1469496958684, "heading"=-0.05471467597547924}, {"dt"=0.005, "x"=25.652842986392535, "y"=232.9616741055907, "position"=-25.675260183427707, "velocity"=-58.39644977050885, "acceleration"=-44.128359710171594, "jerk"=954.4829412865852, "heading"=-0.05464447112317222}, {"dt"=0.005, "x"=25.94537285178495, "y"=232.97766280438464, "position"=-25.96822666723708, "velocity"=-58.593296761874335, "acceleration"=-39.36939827309658, "jerk"=951.7922874150031, "heading"=-0.054557359431673225}, {"dt"=0.005, "x"=26.238768559929433, "y"=232.99367068403154, "position"=-26.262058751544416, "velocity"=-58.76641686146704, "acceleration"=-34.62401991854165, "jerk"=949.075670910986, "heading"=-0.05445317268427069}, {"dt"=0.005, "x"=26.53291227516193, "y"=233.00968610193388, "position"=-26.5566381446142, "velocity"=-58.91587861395703, "acceleration"=-29.892350497996745, "jerk"=946.3338841089808, "heading"=-0.0543317672035496}, {"dt"=0.005, "x"=26.827686507858076, "y"=233.02569739705203, "position"=-26.851846900976476, "velocity"=-59.0417512724552, "acceleration"=-25.174531699634883, "jerk"=943.5637596723723, "heading"=-0.05419302407372539}, {"dt"=0.005, "x"=27.122974127042678, "y"=233.04169290966598, "position"=-27.147567435379305, "velocity"=-59.144106880565516, "acceleration"=-20.471121622063038, "jerk"=940.6820155143691, "heading"=-0.054036849338967796}, {"dt"=0.005, "x"=27.418658330179557, "y"=233.0576609990164, "position"=-27.44368249386535, "velocity"=-59.2230116972092, "acceleration"=-15.78096332873713, "jerk"=938.0316586651816, "heading"=-0.05386317420634379}, {"dt"=0.005, "x"=27.71462268425564, "y"=233.07359006495878, "position"=-27.740075196247627, "velocity"=-59.27854047645569, "acceleration"=-11.105755849297339, "jerk"=935.0414958879583, "heading"=-0.053671955193917265}, {"dt"=0.005, "x"=28.010751095921027, "y"=233.08946856587582, "position"=-28.03662900753124, "velocity"=-59.31076225672255, "acceleration"=-6.444356053371791, "jerk"=932.2799591851094, "heading"=-0.05346317429916836}, {"dt"=0.005, "x"=28.306927829841573, "y"=233.10528503924502, "position"=-28.333227757605613, "velocity"=-59.31975001487475, "acceleration"=-1.7975516304403527, "jerk"=929.3608845862877, "heading"=-0.053236839122346336}, {"dt"=0.005, "x"=28.60303749678439, "y"=233.12102812057682, "position"=-28.629755630607132, "velocity"=-59.305574600303736, "acceleration"=2.835082914202758, "jerk"=926.5269089286221, "heading"=-0.05299298299170385}, {"dt"=0.005, "x"=28.898965068985028, "y"=233.1366865637598, "position"=-28.926097181577425, "velocity"=-59.268310194058856, "acceleration"=7.452881248975984, "jerk"=923.5596669546453, "heading"=-0.0527316650505078}, {"dt"=0.005, "x"=29.19465313492539, "y"=233.15225226641317, "position"=-29.222194671331465, "velocity"=-59.21949795080808, "acceleration"=9.762448650154454, "jerk"=461.9134802356939, "heading"=-0.05245291464960161}, {"dt"=0.005, "x"=29.49010170963538, "y"=233.16772019425196, "position"=-29.518047873257338, "velocity"=-59.1706403851743, "acceleration"=9.771513126756304, "jerk"=1.8128953203699893, "heading"=-0.052156714461370934}, {"dt"=0.005, "x"=29.785310750472597, "y"=233.1830853177075, "position"=-29.813656507790963, "velocity"=-59.121726906725094, "acceleration"=9.782695689841603, "jerk"=2.236512617059816, "heading"=-0.05184304612444818}, {"dt"=0.005, "x"=30.080280246226685, "y"=233.19834261632923, "position"=-30.109020331890417, "velocity"=-59.07276481989091, "acceleration"=9.79241736683747, "jerk"=1.9443353991732693, "heading"=-0.05151189015327118}, {"dt"=0.005, "x"=30.37501010581721, "y"=233.21348707275214, "position"=-30.404139027832567, "velocity"=-59.02373918843039, "acceleration"=9.805126292103239, "jerk"=2.5417850531539443, "heading"=-0.05116322605858303}, {"dt"=0.005, "x"=30.669500273001184, "y"=233.2285136783902, "position"=-30.69901231832366, "velocity"=-58.97465809821897, "acceleration"=9.816218042284675, "jerk"=2.21835003628712, "heading"=-0.05079703222036941}, {"dt"=0.005, "x"=30.963750627509864, "y"=233.243417428109, "position"=-30.993639867755423, "velocity"=-58.92550988635239, "acceleration"=9.829642373316005, "jerk"=2.684866206266179, "heading"=-0.05041328600416811}, {"dt"=0.005, "x"=31.257761056611102, "y"=233.25819332365788, "position"=-31.288021354112097, "velocity"=-58.876297271334984, "acceleration"=9.842523003480608, "jerk"=2.576126032920456, "heading"=-0.050011963675561155}, {"dt"=0.005, "x"=31.5515314155381, "y"=233.27283637142045, "position"=-31.58215642959932, "velocity"=-58.8270150974447, "acceleration"=9.856434778056666, "jerk"=2.7823549152117266, "heading"=-0.049593040450436554}, {"dt"=0.005, "x"=31.845061528732884, "y"=233.2873415822749, "position"=-31.87604472214272, "velocity"=-58.777658508679885, "acceleration"=9.871317752963193, "jerk"=2.976594981305425, "heading"=-0.04915649049779214}, {"dt"=0.005, "x"=32.13835123149809, "y"=233.3017039734271, "position"=-32.16968587734361, "velocity"=-58.72823104017769, "acceleration"=9.885493700438985, "jerk"=2.8351894951583745, "heading"=-0.04870228687831463}, {"dt"=0.005, "x"=32.43140028397624, "y"=233.31591856396997, "position"=-32.46307947260881, "velocity"=-58.67871905304032, "acceleration"=9.902397427474341, "jerk"=3.3807454070711174, "heading"=-0.04823040167711945}, {"dt"=0.005, "x"=32.724208491006024, "y"=233.32998038052867, "position"=-32.75622513740522, "velocity"=-58.62913295928176, "acceleration"=9.917218751711232, "jerk"=2.9642648473782174, "heading"=-0.04774080581776119}, {"dt"=0.005, "x"=33.01677556882678, "y"=233.34388445059218, "position"=-33.049122420064016, "velocity"=-58.57945653175951, "acceleration"=9.935285504450064, "jerk"=3.6133505477664585, "heading"=-0.04723346927862704}, {"dt"=0.005, "x"=33.3091012563951, "y"=233.35762580768665, "position"=-33.341770899484445, "velocity"=-58.52969588408598, "acceleration"=9.952129534705989, "jerk"=3.368806051184947, "heading"=-0.04670836091198527}, {"dt"=0.005, "x"=33.60118525794875, "y"=233.37119948841112, "position"=-33.63417012788972, "velocity"=-58.47984568105524, "acceleration"=9.9700406061487, "jerk"=3.582214288542218, "heading"=-0.04616544854046578}, {"dt"=0.005, "x"=33.89302722944521, "y"=233.38460053166256, "position"=-33.92631961751304, "velocity"=-58.42989792466434, "acceleration"=9.989551278179931, "jerk"=3.902134406246205, "heading"=-0.045604698989398784}, {"dt"=0.005, "x"=34.184626870330014, "y"=233.39782398266084, "position"=-34.218218932723694, "velocity"=-58.37986304213154, "acceleration"=10.006976506559795, "jerk"=3.485045675972742, "heading"=-0.04502607791204849}, {"dt"=0.005, "x"=34.4759837678989, "y"=233.4108648856573, "position"=-34.509867534489466, "velocity"=-58.329720353154876, "acceleration"=10.028537795332682, "jerk"=4.312257754577331, "heading"=-0.04442955009455285}, {"dt"=0.005, "x"=34.76709755357121, "y"=233.4237182908803, "position"=-34.80126493707619, "velocity"=-58.27948051734474, "acceleration"=10.04796716202776, "jerk"=3.8858733390156885, "heading"=-0.04381507915168836}, {"dt"=0.005, "x"=35.057967812978156, "y"=233.4363792502773, "position"=-35.092410618308655, "velocity"=-58.22913624649281, "acceleration"=10.068854170386032, "jerk"=4.177401671654479, "heading"=-0.04318262770643133}, {"dt"=0.005, "x"=35.34859408215386, "y"=233.4488428172602, "position"=-35.38330401602838, "velocity"=-58.17867954394501, "acceleration"=10.091340509559643, "jerk"=4.497267834722152, "heading"=-0.042532157408386395}, {"dt"=0.005, "x"=35.63897594100262, "y"=233.46110405055097, "position"=-35.673944621915226, "velocity"=-58.12812117736892, "acceleration"=10.111673315218184, "jerk"=4.066561131708113, "heading"=-0.04186362872677135}, {"dt"=0.005, "x"=35.929112863508124, "y"=233.47315800763127, "position"=-35.96433183183029, "velocity"=-58.07744198301374, "acceleration"=10.135838871035219, "jerk"=4.833111163407011, "heading"=-0.04117700129097934}, {"dt"=0.005, "x"=36.219004339998456, "y"=233.48499974983008, "position"=-36.25446506846486, "velocity"=-58.02664732691285, "acceleration"=10.158931220178147, "jerk"=4.618469828585603, "heading"=-0.04047223361892255}, {"dt"=0.005, "x"=36.50864986476125, "y"=233.49662434155184, "position"=-36.54434376921366, "velocity"=-57.9757401497604, "acceleration"=10.181435430490637, "jerk"=4.500842062498123, "heading"=-0.0397492831385996}, {"dt"=0.005, "x"=36.798048833844334, "y"=233.5080268460489, "position"=-36.83396728416912, "velocity"=-57.924702991091905, "acceleration"=10.207431733698513, "jerk"=5.199260641575165, "heading"=-0.03900810644742114}, {"dt"=0.005, "x"=37.08720067704438, "y"=233.519202330619, "position"=-37.12333500849469, "velocity"=-57.87354486511449, "acceleration"=10.231625195483218, "jerk"=4.83869235694101, "heading"=-0.03824865898894908}, {"dt"=0.005, "x"=37.37610479491622, "y"=233.530145863902, "position"=-37.41244631966052, "velocity"=-57.822262233165624, "acceleration"=10.256526389773057, "jerk"=4.980238857967834, "heading"=-0.0374708952092942}, {"dt"=0.005, "x"=37.66476051523433, "y"=233.54085251418073, "position"=-37.701300534157305, "velocity"=-57.77084289935701, "acceleration"=10.28386676172346, "jerk"=5.468074390080346, "heading"=-0.03667476868408692}, {"dt"=0.005, "x"=37.95316719246809, "y"=233.5513173530317, "position"=-37.98989700732563, "velocity"=-57.71929463366451, "acceleration"=10.309653138499186, "jerk"=5.15727535514543, "heading"=-0.03586023185428849}, {"dt"=0.005, "x"=38.241324145571944, "y"=233.56153545283127, "position"=-38.27823507138519, "velocity"=-57.66761281191134, "acceleration"=10.336364350634142, "jerk"=5.342242426991106, "heading"=-0.03502723619537218}, {"dt"=0.005, "x"=38.52923062546143, "y"=233.5715018855853, "position"=-38.566314003180274, "velocity"=-57.6157863590164, "acceleration"=10.365290578988606, "jerk"=5.785245670892891, "heading"=-0.03417573232263721}, {"dt"=0.005, "x"=38.816885899983404, "y"=233.58121172585206, "position"=-38.854133109492416, "velocity"=-57.563821262427794, "acceleration"=10.393019317720587, "jerk"=5.545747746396046, "heading"=-0.03330566975052851}, {"dt"=0.005, "x"=39.10428922260308, "y"=233.59066004945785, "position"=-39.14169169599574, "velocity"=-57.51171730066439, "acceleration"=10.420792352681474, "jerk"=5.554606992177469, "heading"=-0.03241699698138045}, {"dt"=0.005, "x"=39.39143975686065, "y"=233.59984193098256, "position"=-39.4289889919676, "velocity"=-57.45945919437175, "acceleration"=10.4516212585267, "jerk"=6.165781169045204, "heading"=-0.03150966174817038}, {"dt"=0.005, "x"=39.67833667671374, "y"=233.60875244704866, "position"=-39.71602425098251, "velocity"=-57.40705180298169, "acceleration"=10.481478278012446, "jerk"=5.97140389714923, "heading"=-0.030583610714597365}, {"dt"=0.005, "x"=39.96497917231792, "y"=233.617386676261, "position"=-40.00279675698732, "velocity"=-57.354501200963, "acceleration"=10.510120403738199, "jerk"=5.728425145150595, "heading"=-0.02963878944937004}, {"dt"=0.005, "x"=40.25136632533163, "y"=233.6257396953659, "position"=-40.28930569984856, "velocity"=-57.30178857224853, "acceleration"=10.54252574289336, "jerk"=6.4810678310323055, "heading"=-0.028675142841681656}, {"dt"=0.005, "x"=40.537497220922006, "y"=233.63380658269625, "position"=-40.57555028771452, "velocity"=-57.24891757319116, "acceleration"=10.574199811475182, "jerk"=6.334813716364351, "heading"=-0.02769261474747392}, {"dt"=0.005, "x"=40.82337093127035, "y"=233.64158241754157, "position"=-40.86152973081467, "velocity"=-57.195888620028846, "acceleration"=10.60579063246223, "jerk"=6.318164197409715, "heading"=-0.026691148044279245}, {"dt"=0.005, "x"=41.10898652058099, "y"=233.64906228016847, "position"=-41.14724324677459, "velocity"=-57.14270319198561, "acceleration"=10.637085608647112, "jerk"=6.258995236976261, "heading"=-0.025670684615507144}, {"dt"=0.005, "x"=41.39434295718699, "y"=233.65624124952305, "position"=-41.43268997300117, "velocity"=-57.08934524531487, "acceleration"=10.671589334148734, "jerk"=6.900745100324457, "heading"=-0.024631165674522115}, {"dt"=0.005, "x"=41.679439219124866, "y"=233.6631144060541, "position"=-41.7178690726064, "velocity"=-57.03581992104566, "acceleration"=10.705064853841861, "jerk"=6.69510393862538, "heading"=-0.023572531400882835}, {"dt"=0.005, "x"=41.96427425786584, "y"=233.6696768306875, "position"=-42.0027796984378, "velocity"=-56.98212516628016, "acceleration"=10.738950953098936, "jerk"=6.777219851414884, "heading"=-0.022494721074098778}, {"dt"=0.005, "x"=42.24884703283148, "y"=233.67592360555022, "position"=-42.28742102791725, "velocity"=-56.92826589589032, "acceleration"=10.771854077968612, "jerk"=6.580624973935301, "heading"=-0.021397672947609525}, {"dt"=0.005, "x"=42.533156393582175, "y"=233.68184981137884, "position"=-42.57179214551886, "velocity"=-56.87422352032358, "acceleration"=10.808475113347527, "jerk"=7.3242070757828515, "heading"=-0.020281324711831306}, {"dt"=0.005, "x"=42.81720120206014, "y"=233.68745053032413, "position"=-42.85589216536397, "velocity"=-56.82000396902064, "acceleration"=10.84391026058853, "jerk"=7.08702944820061, "heading"=-0.01914561303977602}, {"dt"=0.005, "x"=43.100980290768575, "y"=233.6927208449863, "position"=-43.139720189711156, "velocity"=-56.76560486943771, "acceleration"=10.879819916586086, "jerk"=7.181931199511382, "heading"=-0.01799047375417162}, {"dt"=0.005, "x"=43.38449246921197, "y"=233.6976558385518, "position"=-43.42327531572233, "velocity"=-56.71102520223425, "acceleration"=10.915933440692527, "jerk"=7.222704821288062, "heading"=-0.016815841811278875}, {"dt"=0.005, "x"=43.667736534467714, "y"=233.70225059495533, "position"=-43.706556646362046, "velocity"=-56.65626612794306, "acceleration"=10.95181485823673, "jerk"=7.176283508840697, "heading"=-0.015621651264711545}, {"dt"=0.005, "x"=43.95071119809306, "y"=233.7065001977645, "position"=-43.98956321762482, "velocity"=-56.6013142525555, "acceleration"=10.990375077513193, "jerk"=7.71204385529245, "heading"=-0.01440783558692399}, {"dt"=0.005, "x"=44.23341517307498, "y"=233.7103997317168, "position"=-44.27229408582924, "velocity"=-56.5461736408834, "acceleration"=11.02812233441881, "jerk"=7.5494513811236175, "heading"=-0.013174327319233403}, {"dt"=0.005, "x"=44.51584714215469, "y"=233.7139442822114, "position"=-44.554748296271306, "velocity"=-56.4908420884132, "acceleration"=11.06631049404001, "jerk"=7.63763192423994, "heading"=-0.011921058214635183}, {"dt"=0.005, "x"=44.79800575767962, "y"=233.7171289353779, "position"=-44.83692488341265, "velocity"=-56.43531742826825, "acceleration"=11.104932028990788, "jerk"=7.724306990155583, "heading"=-0.01064795925167522}, {"dt"=0.005, "x"=45.07988964146061, "y"=233.71994877815283, "position"=-45.11882287107615, "velocity"=-56.37959753270012, "acceleration"=11.143979113626301, "jerk"=7.809416927102575, "heading"=-0.00935496064885355}, {"dt"=0.005, "x"=45.36149740601544, "y"=233.7223988985379, "position"=-45.400441294030806, "velocity"=-56.32368459093158, "acceleration"=11.182588353707956, "jerk"=7.721848016331023, "heading"=-0.008041991779076774}, {"dt"=0.005, "x"=45.64282759470994, "y"=233.72447438515155, "position"=-45.68177913847334, "velocity"=-56.26756888850583, "acceleration"=11.22314048514994, "jerk"=8.110426288396866, "heading"=-0.0067089814623131905}, {"dt"=0.005, "x"=45.9238787308381, "y"=233.72617032785163, "position"=-45.96283539145585, "velocity"=-56.21125059650211, "acceleration"=11.263658400743282, "jerk"=8.103583118668212, "heading"=-0.005355857757466886}, {"dt"=0.005, "x"=46.20464931265738, "y"=233.7274818177584, "position"=-46.24360903626767, "velocity"=-56.15472896236404, "acceleration"=11.304326827614375, "jerk"=8.133685374218658, "heading"=-0.003982547998840569}, {"dt"=0.005, "x"=46.48513780726226, "y"=233.7284039473204, "position"=-46.524099046657774, "velocity"=-56.09800207802121, "acceleration"=11.345376868565893, "jerk"=8.210008190303597, "heading"=-0.002588978841237932}, {"dt"=0.005, "x"=46.76534265047772, "y"=233.72893181044668, "position"=-46.80430438707954, "velocity"=-56.041068084353775, "acceleration"=11.386798733487069, "jerk"=8.284372984235233, "heading"=-0.0011750762778853785}, {"dt"=0.005, "x"=47.04526224675975, "y"=233.72906050264788, "position"=-47.084224012944496, "velocity"=-55.98392517299089, "acceleration"=11.428582272577614, "jerk"=8.356707818109044, "heading"=-6.282926072838585}, {"dt"=0.005, "x"=47.32489496910334, "y"=233.72878512118703, "position"=-47.36385687088547, "velocity"=-55.92657158819504, "acceleration"=11.470716959169636, "jerk"=8.42693731840427, "heading"=-6.281471278890596}, {"dt"=0.005, "x"=47.60423915895815, "y"=233.72810076524, "position"=-47.64320189902935, "velocity"=-55.86900562877523, "acceleration"=11.513191883962293, "jerk"=8.494984958531404, "heading"=-6.279995925736066}, {"dt"=0.005, "x"=47.88329312615206, "y"=233.72700253606544, "position"=-47.922258027279526, "velocity"=-55.81122565003555, "acceleration"=11.555995747934844, "jerk"=8.560772794510285, "heading"=-6.2784999369142875}, {"dt"=0.005, "x"=48.162055148823214, "y"=233.72548553718454, "position"=-48.201024177608645, "velocity"=-55.75323006582373, "acceleration"=11.599116842364765, "jerk"=8.624218885984192, "heading"=-6.2769832354026125}, {"dt"=0.005, "x"=48.44052347336074, "y"=233.7235448745706, "position"=-48.47949926436169, "velocity"=-55.6950173506101, "acceleration"=11.642543042725606, "jerk"=8.685240072168199, "heading"=-6.275445743638507}, {"dt"=0.005, "x"=48.71869631435453, "y"=233.7211756568483, "position"=-48.7576821945698, "velocity"=-55.63658604162263, "acceleration"=11.686261797494524, "jerk"=8.743750953783547, "heading"=-6.273887383542361}, {"dt"=0.005, "x"=48.99657185455442, "y"=233.71837299550293, "position"=-49.03557186827503, "velocity"=-55.57793474104465, "acceleration"=11.73026011559557, "jerk"=8.79966362020923, "heading"=-6.272308076541074}, {"dt"=0.005, "x"=49.274148244839054, "y"=233.71513200509966, "position"=-49.31316717886626, "velocity"=-55.51906211824652, "acceleration"=11.774524559626798, "jerk"=8.852888806245574, "heading"=-6.2707077435924266}, {"dt"=0.005, "x"=49.55142360419519, "y"=233.71144780351256, "position"=-49.590467013426995, "velocity"=-55.459966912146804, "acceleration"=11.819041219942505, "jerk"=8.903332063141534, "heading"=-6.269086305210262}, {"dt"=0.005, "x"=49.82839601970718, "y"=233.70731551216377, "position"=-49.867470253094574, "velocity"=-55.400647933515955, "acceleration"=11.863795726169712, "jerk"=8.9509012454414, "heading"=-6.267443681490498}, {"dt"=0.005, "x"=50.10506354655761, "y"=233.70273025627284, "position"=-50.14417577343185, "velocity"=-55.34110406745407, "acceleration"=11.908773212377355, "jerk"=8.995497241528483, "heading"=-6.2657797921379865}, {"dt"=0.005, "x"=50.38142420803939, "y"=233.69768716511572, "position"=-50.420582444811295, "velocity"=-55.28133427588989, "acceleration"=11.953958312835766, "jerk"=9.03702009168228, "heading"=-6.264094556494244}, {"dt"=0.005, "x"=50.65747599557904, "y"=233.69218137229439, "position"=-50.69668913281147, "velocity"=-55.22133760003561, "acceleration"=11.99933517085583, "jerk"=9.075371604012616, "heading"=-6.262387893566057}, {"dt"=0.005, "x"=50.93321686877289, "y"=233.68620801601597, "position"=-50.9724946986272, "velocity"=-55.16111316314567, "acceleration"=12.044887377987834, "jerk"=9.11044142640094, "heading"=-6.260659722055016}, {"dt"=0.005, "x"=51.208644755435074, "y"=233.67976223938248, "position"=-51.24799799949238, "velocity"=-55.10066017303485, "acceleration"=12.09059802216359, "jerk"=9.142128835151198, "heading"=-6.258909960387953}, {"dt"=0.005, "x"=51.48375755165901, "y"=233.67283919069035, "position"=-51.523197889116894, "velocity"=-55.03997792490358, "acceleration"=12.136449626254375, "jerk"=9.170320818157052, "heading"=-6.257138526748338}, {"dt"=0.005, "x"=51.75855312189213, "y"=233.66543402373992, "position"=-51.798093218137424, "velocity"=-54.97906580410681, "acceleration"=12.182424159354355, "jerk"=9.19490661999589, "heading"=-6.255345339108642}, {"dt"=0.005, "x"=52.03302929902426, "y"=233.65754189815553, "position"=-52.07268283458223, "velocity"=-54.91792328896199, "acceleration"=12.22850302896461, "jerk"=9.215773922051085, "heading"=-6.253530315263679}, {"dt"=0.005, "x"=52.307183898587475, "y"=233.64915797927068, "position"=-52.34696559845473, "velocity"=-54.85655277449944, "acceleration"=12.27410289250912, "jerk"=9.119972708901969, "heading"=-6.251693372769886}, {"dt"=0.005, "x"=52.581014699502795, "y"=233.64027743898316, "position"=-52.62094036285051, "velocity"=-54.79495287915629, "acceleration"=12.319979068630005, "jerk"=9.175235224176959, "heading"=-6.249834429106812}, {"dt"=0.005, "x"=52.85451942076768, "y"=233.63089545697738, "position"=-52.89460595100609, "velocity"=-54.73311763111589, "acceleration"=12.36704960808055, "jerk"=9.41410789010888, "heading"=-6.247953401878108}, {"dt"=0.005, "x"=53.12769577021988, "y"=233.62100721954917, "position"=-53.167961205463484, "velocity"=-54.671050891479, "acceleration"=12.413347927378027, "jerk"=9.259663859495504, "heading"=-6.2460502085209475}, {"dt"=0.005, "x"=53.40054142480029, "y"=233.61060792056574, "position"=-53.44100496870073, "velocity"=-54.60875264744948, "acceleration"=12.459648805904067, "jerk"=9.260175705207985, "heading"=-6.244124766477078}, {"dt"=0.005, "x"=53.673054030733454, "y"=233.59969276184418, "position"=-53.713736083688374, "velocity"=-54.54622299752815, "acceleration"=12.505929984266118, "jerk"=9.256235672410185, "heading"=-6.242176993232494}, {"dt"=0.005, "x"=53.94523123140558, "y"=233.58825695235012, "position"=-53.98615342216832, "velocity"=-54.48346769598968, "acceleration"=12.551060307693263, "jerk"=9.026064685428992, "heading"=-6.240206806156601}, {"dt"=0.005, "x"=54.21707061175909, "y"=233.576295710831, "position"=-54.25825582937866, "velocity"=-54.42048144206741, "acceleration"=12.597250784453706, "jerk"=9.238095352088749, "heading"=-6.238214122943167}, {"dt"=0.005, "x"=54.488569702916685, "y"=233.5638042662951, "position"=-54.530042129044396, "velocity"=-54.35725993314705, "acceleration"=12.644301784072809, "jerk"=9.410199923820528, "heading"=-6.2361988616334925}, {"dt"=0.005, "x"=54.759726030359886, "y"=233.55077785631926, "position"=-54.80151117197442, "velocity"=-54.29380858600484, "acceleration"=12.69026942844107, "jerk"=9.193528873652212, "heading"=-6.234160940309314}, {"dt"=0.005, "x"=55.03053710113032, "y"=233.53721172789847, "position"=-55.072661823627996, "velocity"=-54.230130330715205, "acceleration"=12.735651057927555, "jerk"=9.07632589729701, "heading"=-6.232100277227126}, {"dt"=0.005, "x"=55.30100042649221, "y"=233.5231011365741, "position"=-55.34349298718443, "velocity"=-54.166232711287506, "acceleration"=12.779523885539845, "jerk"=8.774565522458033, "heading"=-6.2300167906862045}, {"dt"=0.005, "x"=55.5711133913476, "y"=233.5084413537633, "position"=-55.61400347314576, "velocity"=-54.102097192264516, "acceleration"=12.827103804598039, "jerk"=9.515983811638762, "heading"=-6.227910400087494}, {"dt"=0.005, "x"=55.84087340471953, "y"=233.49322765961193, "position"=-55.884192150377345, "velocity"=-54.03773544631729, "acceleration"=12.872349189444776, "jerk"=9.049076969347425, "heading"=-6.225781024836646}, {"dt"=0.005, "x"=56.11027788974326, "y"=233.47745534351546, "position"=-56.15405793647471, "velocity"=-53.97315721947232, "acceleration"=12.915645368994433, "jerk"=8.65923590993134, "heading"=-6.223628584452614}, {"dt"=0.005, "x"=56.37932419296334, "y"=233.46111970975397, "position"=-56.42359970727615, "velocity"=-53.908354160289626, "acceleration"=12.96061183653876, "jerk"=8.993293508865463, "heading"=-6.221452999339665}, {"dt"=0.005, "x"=56.64800960629776, "y"=233.44421607711462, "position"=-56.692816319198776, "velocity"=-53.84332238452474, "acceleration"=13.006355152977278, "jerk"=9.148663287703585, "heading"=-6.219254190686253}, {"dt"=0.005, "x"=56.916331461892185, "y"=233.4267397734232, "position"=-56.961706704635574, "velocity"=-53.778077087359065, "acceleration"=13.049059433134857, "jerk"=8.540856031515887, "heading"=-6.217032079745915}, {"dt"=0.005, "x"=57.18428705015985, "y"=233.40868614092872, "position"=-57.230269790204154, "velocity"=-53.71261711371659, "acceleration"=13.091994728495138, "jerk"=8.587059072056036, "heading"=-6.2147865885543645}, {"dt"=0.005, "x"=57.45187356586966, "y"=233.39005054081414, "position"=-57.49850444303885, "velocity"=-53.64693056693782, "acceleration"=13.137309355754212, "jerk"=9.062925451814863, "heading"=-6.212517640457433}, {"dt"=0.005, "x"=57.71908828097319, "y"=233.37082834190042, "position"=-57.766409644367485, "velocity"=-53.581040265727644, "acceleration"=13.178060242034917, "jerk"=8.150177256140978, "heading"=-6.210225158716788}, {"dt"=0.005, "x"=57.98592837962764, "y"=233.35101493245284, "position"=-58.033984324492216, "velocity"=-53.51493602494658, "acceleration"=13.220848156213094, "jerk"=8.557582835635458, "heading"=-6.207909067962685}, {"dt"=0.005, "x"=58.25239099101944, "y"=233.3306057189108, "position"=-58.30122739599669, "velocity"=-53.44861430089409, "acceleration"=13.264344810497164, "jerk"=8.699330856813958, "heading"=-6.205569294001157}, {"dt"=0.005, "x"=58.51847335756178, "y"=233.3095961133373, "position"=-58.568137922786335, "velocity"=-53.38210535792931, "acceleration"=13.301788592956143, "jerk"=7.488756491795812, "heading"=-6.2032057623941865}, {"dt"=0.005, "x"=58.78417250902315, "y"=233.28798155925728, "position"=-58.8347147935673, "velocity"=-53.31537415619262, "acceleration"=13.346240347338778, "jerk"=8.890350876527009, "heading"=-6.2008184014030965}, {"dt"=0.005, "x"=59.04948559979517, "y"=233.26575750585263, "position"=-59.10095706046858, "velocity"=-53.24845338025643, "acceleration"=13.384155187237923, "jerk"=7.582967979828936, "heading"=-6.198407139073686}, {"dt"=0.005, "x"=59.31440969528062, "y"=233.2429194254461, "position"=-59.36686372508125, "velocity"=-53.18133292253504, "acceleration"=13.424091544277417, "jerk"=7.987271407898788, "heading"=-6.19597190520698}, {"dt"=0.005, "x"=59.57894183656435, "y"=233.21946280910024, "position"=-59.63243380363408, "velocity"=-53.11401571056468, "acceleration"=13.463442394072445, "jerk"=7.87016995900558, "heading"=-6.193512630863166}, {"dt"=0.005, "x"=59.84307910261579, "y"=233.19538316151414, "position"=-59.897666389763685, "velocity"=-53.046517225921875, "acceleration"=13.499696928560923, "jerk"=7.250906897695586, "heading"=-6.191029247850655}, {"dt"=0.005, "x"=60.10681844824245, "y"=233.17067601628537, "position"=-60.162560492108256, "velocity"=-52.97882046891379, "acceleration"=13.539351401617239, "jerk"=7.930894611263284, "heading"=-6.18852169032162}, {"dt"=0.005, "x"=60.370156944667364, "y"=233.14533691439252, "position"=-60.42711527619667, "velocity"=-52.91095681768425, "acceleration"=13.572730245907394, "jerk"=6.675768858031006, "heading"=-6.185989892580465}, {"dt"=0.005, "x"=60.63309148701355, "y"=233.1193614323627, "position"=-60.69132977092677, "velocity"=-52.84289894601939, "acceleration"=13.61157433297251, "jerk"=7.768817413023044, "heading"=-6.183433791951375}, {"dt"=0.005, "x"=60.895619118402166, "y"=233.09274515165768, "position"=-60.955203194448515, "velocity"=-52.77468470434832, "acceleration"=13.642848334214364, "jerk"=6.254800248370884, "heading"=-6.18085332574224}, {"dt"=0.005, "x"=61.15773670023185, "y"=233.06548369188013, "position"=-61.21873462311205, "velocity"=-52.70628573270722, "acceleration"=13.679794328218975, "jerk"=7.389198800922259, "heading"=-6.178248434533795}, {"dt"=0.005, "x"=61.419441228327685, "y"=233.0375726794494, "position"=-61.481923309496494, "velocity"=-52.637737276889716, "acceleration"=13.709691163501248, "jerk"=5.979367056454521, "heading"=-6.175619059161447}, {"dt"=0.005, "x"=61.680729555493166, "y"=233.00900777695716, "position"=-61.74476840373895, "velocity"=-52.56901884849147, "acceleration"=13.743685679649786, "jerk"=6.798903229707776, "heading"=-6.172965143553779}, {"dt"=0.005, "x"=61.94159861242743, "y"=232.97978466048949, "position"=-62.007269175931825, "velocity"=-52.50015443857446, "acceleration"=13.772881983400964, "jerk"=5.839260750235553, "heading"=-6.170286632611656}, {"dt"=0.005, "x"=62.20204526743896, "y"=232.9498990353293, "position"=-62.26942487527462, "velocity"=-52.431139868559775, "acceleration"=13.802914002937428, "jerk"=6.006403907292679, "heading"=-6.167583473711987}, {"dt"=0.005, "x"=62.462066369835945, "y"=232.91934663213019, "position"=-62.531234773928176, "velocity"=-52.36197973071086, "acceleration"=13.832027569783634, "jerk"=5.822713369241228, "heading"=-6.1648556163699935}, {"dt"=0.005, "x"=62.72165882630481, "y"=232.88812319838516, "position"=-62.79269824416899, "velocity"=-52.2926940481632, "acceleration"=13.857136509531642, "jerk"=5.02178794960173, "heading"=-6.162103011523147}, {"dt"=0.005, "x"=62.980819412603346, "y"=232.85622452157608, "position"=-63.053814568960775, "velocity"=-52.2232649583575, "acceleration"=13.88581796114039, "jerk"=5.736290321749493, "heading"=-6.159325613616925}, {"dt"=0.005, "x"=63.23954502821702, "y"=232.82364639911904, "position"=-63.314583198664394, "velocity"=-52.15372594072344, "acceleration"=13.907803526811335, "jerk"=4.397113134189112, "heading"=-6.156523377998246}, {"dt"=0.005, "x"=63.49783245898948, "y"=232.79038466805534, "position"=-63.575003512097105, "velocity"=-52.08406268654163, "acceleration"=13.93265083636237, "jerk"=4.969461910206974, "heading"=-6.15369626355041}, {"dt"=0.005, "x"=63.75567850722992, "y"=232.75643518991836, "position"=-63.835074947781585, "velocity"=-52.01428713689613, "acceleration"=13.955109929099763, "jerk"=4.491818547478488, "heading"=-6.150844231407743}, {"dt"=0.005, "x"=64.01308005257135, "y"=232.72179384279562, "position"=-64.09479706558182, "velocity"=-51.94442356004536, "acceleration"=13.972715370154276, "jerk"=3.5210882109026898, "heading"=-6.147967244360675}, {"dt"=0.005, "x"=64.27003382898073, "y"=232.6864565517745, "position"=-64.35416932190032, "velocity"=-51.8744512637, "acceleration"=13.994459269071058, "jerk"=4.348779783356349, "heading"=-6.1450652694423376}, {"dt"=0.005, "x"=64.5265366475664, "y"=232.65041926006404, "position"=-64.61319129459032, "velocity"=-51.804394538000494, "acceleration"=14.01134513990172, "jerk"=3.3771741661325905, "heading"=-6.142138275560648}, {"dt"=0.005, "x"=64.78258535534539, "y"=232.61367793445186, "position"=-64.87186264159851, "velocity"=-51.73426940163732, "acceleration"=14.025027272634816, "jerk"=2.7364265466189863, "heading"=-6.1391862340354955}, {"dt"=0.005, "x"=65.03817668924798, "y"=232.57622858700503, "position"=-65.13018295359565, "velocity"=-51.664062399426676, "acceleration"=14.041400442128804, "jerk"=3.274633898797674, "heading"=-6.136209120393161}, {"dt"=0.005, "x"=65.293307444818, "y"=232.53806725190532, "position"=-65.38815192447068, "velocity"=-51.59379417500639, "acceleration"=14.053644884057803, "jerk"=2.448888385799819, "heading"=-6.133206912545325}, {"dt"=0.005, "x"=65.5479744665308, "y"=232.49918998671967, "position"=-65.6457693417708, "velocity"=-51.52348346002454, "acceleration"=14.06214299636872, "jerk"=1.69962246218347, "heading"=-6.130179590980567}, {"dt"=0.005, "x"=65.80217450474439, "y"=232.45959289482755, "position"=-65.90303494210264, "velocity"=-51.453120066367106, "acceleration"=14.072678731487542, "jerk"=2.1071470237643553, "heading"=-6.127127140573875}, {"dt"=0.005, "x"=66.0559043523094, "y"=232.41927210566826, "position"=-66.15994854934016, "velocity"=-51.38272144750315, "acceleration"=14.079723772790942, "jerk"=1.4090082606799115, "heading"=-6.124049549092932}, {"dt"=0.005, "x"=66.30916082345276, "y"=232.3782237782526, "position"=-66.41651005338862, "velocity"=-51.312300809693156, "acceleration"=14.084127561999082, "jerk"=0.8807578416281103, "heading"=-6.120946807548997}, {"dt"=0.005, "x"=66.56194074817186, "y"=232.3364441024918, "position"=-66.67271940459906, "velocity"=-51.24187024208745, "acceleration"=14.08611352114093, "jerk"=0.3971918283696141, "heading"=-6.117818910371953}, {"dt"=0.005, "x"=66.81424090466436, "y"=232.29392931118656, "position"=-66.9285765452965, "velocity"=-51.17142813948687, "acceleration"=14.088420520116074, "jerk"=0.461399795028683, "heading"=-6.11466585636935}, {"dt"=0.005, "x"=67.06605811548185, "y"=232.2506756649629, "position"=-67.18408150723567, "velocity"=-51.10099238783646, "acceleration"=14.0871503300815, "jerk"=-0.25403800691492506, "heading"=-6.111487647660861}, {"dt"=0.005, "x"=67.31738921277234, "y"=232.20667945847828, "position"=-67.43923437641467, "velocity"=-51.030573835801086, "acceleration"=14.0837104070755, "jerk"=-0.687984601199787, "heading"=-6.108284290219658}, {"dt"=0.005, "x"=67.56823107285783, "y"=232.16193701483854, "position"=-67.69403532820647, "velocity"=-50.960190358357835, "acceleration"=14.07669548865016, "jerk"=-1.4029836850681932, "heading"=-6.10505579354443}, {"dt"=0.005, "x"=67.8185805128121, "y"=232.1164447046417, "position"=-67.94848452229532, "velocity"=-50.88983881777004, "acceleration"=14.070308117558739, "jerk"=-1.2774742182841692, "heading"=-6.101802172108957}, {"dt"=0.005, "x"=68.06843440064097, "y"=232.07019892722752, "position"=-68.20258221451593, "velocity"=-50.81953844412218, "acceleration"=14.060074729572136, "jerk"=-2.0466775973204676, "heading"=-6.098523444074759}, {"dt"=0.005, "x"=68.31778961928111, "y"=232.02319611751744, "position"=-68.4563287202726, "velocity"=-50.74930115133315, "acceleration"=14.04745855780618, "jerk"=-2.5232343531911283, "heading"=-6.095219631867775}, {"dt"=0.005, "x"=68.56664306806147, "y"=231.97543274634248, "position"=-68.70972441596585, "velocity"=-50.67913913865264, "acceleration"=14.032402536102495, "jerk"=-3.0112043407370948, "heading"=-6.091890762279957}, {"dt"=0.005, "x"=68.8149916853855, "y"=231.9269053165715, "position"=-68.96276976203437, "velocity"=-50.609069213702675, "acceleration"=14.013984989992423, "jerk"=-3.683509222014436, "heading"=-6.088536866282909}, {"dt"=0.005, "x"=69.06283238722524, "y"=231.87761037566796, "position"=-69.21546524020346, "velocity"=-50.539095633817, "acceleration"=13.994715977135286, "jerk"=-3.8538025714274227, "heading"=-6.0851579799781605}, {"dt"=0.005, "x"=69.31016212784438, "y"=231.82754450459893, "position"=-69.46781141521039, "velocity"=-50.469235001386465, "acceleration"=13.972126486106617, "jerk"=-4.5178982057336725, "heading"=-6.081754143905792}, {"dt"=0.005, "x"=69.55697788705884, "y"=231.7767043207379, "position"=-69.71980892172907, "velocity"=-50.39950130373575, "acceleration"=13.946739530143759, "jerk"=-5.0773911925716675, "heading"=-6.078325403332127}, {"dt"=0.005, "x"=69.80327666853086, "y"=231.7250864787153, "position"=-69.97145846249892, "velocity"=-50.329908153968724, "acceleration"=13.918629953404604, "jerk"=-5.621915347830964, "heading"=-6.074871808392415}, {"dt"=0.005, "x"=70.04905550127734, "y"=231.6726876706262, "position"=-70.22276080971315, "velocity"=-50.26046944284563, "acceleration"=13.887742224618194, "jerk"=-6.177545757282132, "heading"=-6.071393414189597}, {"dt"=0.005, "x"=70.29431144291739, "y"=231.6195046258361, "position"=-70.47371680817284, "velocity"=-50.19119969193616, "acceleration"=13.853950181893993, "jerk"=-6.758408544840222, "heading"=-6.067890280867222}, {"dt"=0.005, "x"=70.53904158747073, "y"=231.565534109714, "position"=-70.72432738309654, "velocity"=-50.122114984739305, "acceleration"=13.816941439371533, "jerk"=-7.401748504491934, "heading"=-6.064362473614072}, {"dt"=0.005, "x"=70.78324303572484, "y"=231.51077293066461, "position"=-70.9745935095705, "velocity"=-50.05322529479228, "acceleration"=13.777937989405586, "jerk"=-7.80068999318928, "heading"=-6.0608100632095585}, {"dt"=0.005, "x"=71.02691293329961, "y"=231.45521793227385, "position"=-71.22451625129341, "velocity"=-49.98454834458316, "acceleration"=13.735390041823337, "jerk"=-8.509589516449978, "heading"=-6.057233125594233}, {"dt"=0.005, "x"=71.27004845870232, "y"=231.39886599629457, "position"=-71.47409674813052, "velocity"=-49.916099367423755, "acceleration"=13.68979543188118, "jerk"=-9.118921988431339, "heading"=-6.053631742153799}, {"dt"=0.005, "x"=71.51264682481926, "y"=231.34171404271802, "position"=-71.72333621739698, "velocity"=-49.84789385329073, "acceleration"=13.641102826605334, "jerk"=-9.738521055169258, "heading"=-6.050005999810359}, {"dt"=0.005, "x"=71.75470528039709, "y"=231.28375902982162, "position"=-71.97223595511589, "velocity"=-49.77994754378426, "acceleration"=13.589261901293526, "jerk"=-10.36818506236159, "heading"=-6.046355991111911}, {"dt"=0.005, "x"=71.99622111151253, "y"=231.2249979541936, "position"=-72.22079733724985, "velocity"=-49.71227642679048, "acceleration"=13.534223398755785, "jerk"=-11.00770050754818, "heading"=-6.0426818143199315}, {"dt"=0.005, "x"=72.23719164302774, "y"=231.16542785073332, "position"=-72.46902182090325, "velocity"=-49.64489673067936, "acceleration"=13.475939222223587, "jerk"=-11.656835306439461, "heading"=-6.038983573494877}, {"dt"=0.005, "x"=72.47761424002928, "y"=231.10504579262837, "position"=-72.71691094549317, "velocity"=-49.577824917983044, "acceleration"=13.414362539263891, "jerk"=-12.315336591939285, "heading"=-6.035261378579466}, {"dt"=0.005, "x"=72.71748630924843, "y"=231.04384889130787, "position"=-72.96446633388676, "velocity"=-49.51107767871986, "acceleration"=13.349447852637297, "jerk"=-12.982937325318744, "heading"=-6.031515345479562}, {"dt"=0.005, "x"=72.95680530320968, "y"=230.9818342956545, "position"=-73.21168969634402, "velocity"=-49.44467249145303, "acceleration"=13.281037453366196, "jerk"=-13.68207985422032, "heading"=-6.027745596099019}, {"dt"=0.005, "x"=73.19556871381428, "y"=230.91899919392182, "position"=-73.45858282353329, "velocity"=-49.37862543785465, "acceleration"=13.209410719674963, "jerk"=-14.32534673824648, "heading"=-6.023952258537759}, {"dt"=0.005, "x"=73.43377407962957, "y"=230.85534081212103, "position"=-73.70514759367836, "velocity"=-49.31295402901411, "acceleration"=13.134281768108735, "jerk"=-15.02579031324558, "heading"=-6.02013546707234}, {"dt"=0.005, "x"=73.67141898776333, "y"=230.79085641371336, "position"=-73.95138597411469, "velocity"=-49.24767608726422, "acceleration"=13.055588349978109, "jerk"=-15.738683626125294, "heading"=-6.016295362216069}, {"dt"=0.005, "x"=73.90850107370177, "y"=230.72554329982302, "position"=-74.19730002072238, "velocity"=-49.182809321540056, "acceleration"=12.973353144832345, "jerk"=-16.447041029152842, "heading"=-6.012432090808252}, {"dt"=0.005, "x"=74.1450180225683, "y"=230.65939880905447, "position"=-74.4428918788125, "velocity"=-49.118371618025115, "acceleration"=12.887540702988076, "jerk"=-17.1624883688537, "heading"=-6.008545806077238}, {"dt"=0.005, "x"=74.38096757034694, "y"=230.59242031728905, "position"=-74.68816378396292, "velocity"=-49.054381030083945, "acceleration"=12.798117588233993, "jerk"=-17.88462295081672, "heading"=-6.004636667699919}, {"dt"=0.005, "x"=74.61634750506859, "y"=230.52460523746086, "position"=-74.93311806280221, "velocity"=-48.990855767856175, "acceleration"=12.705052445554088, "jerk"=-18.613028535980902, "heading"=-6.0007048418574795}, {"dt"=0.005, "x"=74.85115566795712, "y"=230.45595101931275, "position"=-75.17775713373858, "velocity"=-48.92781418727529, "acceleration"=12.60831611617732, "jerk"=-19.347265875353514, "heading"=-5.996750501287242}, {"dt"=0.005, "x"=75.0853899545334, "y"=230.3864551491339, "position"=-75.42208350763181, "velocity"=-48.86527477864661, "acceleration"=12.50788172573607, "jerk"=-20.08687808825016, "heading"=-5.992773825330433}, {"dt"=0.005, "x"=75.31904831567483, "y"=230.3161151494787, "position"=-75.66609978840586, "velocity"=-48.80325615480844, "acceleration"=12.403724767634117, "jerk"=-20.831391620390605, "heading"=-5.988774999975715}, {"dt"=0.005, "x"=75.5521287586282, "y"=230.2449285788691, "position"=-75.90980867359984, "velocity"=-48.74177703879596, "acceleration"=12.295823202495626, "jerk"=-21.58031302769814, "heading"=-5.984754217898294}, {"dt"=0.005, "x"=75.78462934797334, "y"=230.1728930314803, "position"=-76.1532129548552, "velocity"=-48.68085625107215, "acceleration"=12.184157544761831, "jerk"=-22.333131546758977, "heading"=-5.98071167849446}, {"dt"=0.005, "x"=76.016548206536, "y"=230.10000613681203, "position"=-76.39631551833695, "velocity"=-48.62051269634789, "acceleration"=12.068710944852512, "jerk"=-23.08931998186381, "heading"=-5.976647587911389}, {"dt"=0.005, "x"=76.24788351624723, "y"=230.02626555934523, "position"=-76.6391193450867, "velocity"=-48.560765349951176, "acceleration"=11.949469279342395, "jerk"=-23.84833310202339, "heading"=-5.972562159072042}, {"dt"=0.005, "x"=76.47863351894739, "y"=229.95166899818685, "position"=-76.88162751130545, "velocity"=-48.50163324375041, "acceleration"=11.82642124015274, "jerk"=-24.60960783793098, "heading"=-5.968455611695016}, {"dt"=0.005, "x"=76.70879651713322, "y"=229.87621418670273, "position"=-77.12384318856436, "velocity"=-48.44313545178342, "acceleration"=11.69955839339849, "jerk"=-25.37256935084997, "heading"=-5.96432817230919}, {"dt"=0.005, "x"=76.93837087195496, "y"=229.79989889304142, "position"=-77.36576964110404, "velocity"=-48.3852905079336, "acceleration"=11.568988769964506, "jerk"=-26.113924686796963, "heading"=-5.960180074311807}, {"dt"=0.005, "x"=77.1673550101893, "y"=229.72272091765754, "position"=-77.60741023257674, "velocity"=-48.32811829454015, "acceleration"=11.434442678690004, "jerk"=-26.909218254900225, "heading"=-5.956011557858135}, {"dt"=0.005, "x"=77.39574742068905, "y"=229.64467809425017, "position"=-77.84876842170502, "velocity"=-48.27163782565538, "acceleration"=11.296093776952887, "jerk"=-27.66978034742351, "heading"=-5.951822869932884}, {"dt"=0.005, "x"=77.62354665471095, "y"=229.5657682894353, "position"=-78.08984776199962, "velocity"=-48.21586805892173, "acceleration"=11.153953346730816, "jerk"=-28.428086044414158, "heading"=-5.947614264346094}, {"dt"=0.005, "x"=77.85075132696598, "y"=229.48598940214075, "position"=-78.3306519022308, "velocity"=-48.16082804623415, "acceleration"=11.008002537515438, "jerk"=-29.190161843075657, "heading"=-5.943386001708555}, {"dt"=0.005, "x"=78.0773601159858, "y"=229.40533936320224, "position"=-78.57118458616753, "velocity"=-48.106536787347856, "acceleration"=10.858251777258943, "jerk"=-29.95015205129903, "heading"=-5.9391383494123104}, {"dt"=0.005, "x"=78.30337176442083, "y"=229.32381613495897, "position"=-78.81144965223316, "velocity"=-48.053013213127635, "acceleration"=10.70471484404436, "jerk"=-30.70738664291639, "heading"=-5.934871581605034}, {"dt"=0.005, "x"=78.52878507926889, "y"=229.24141771085016, "position"=-79.05145103307586, "velocity"=-48.00027616854084, "acceleration"=10.547408917358325, "jerk"=-31.461185337207098, "heading"=-5.9305859791581845}, {"dt"=0.005, "x"=78.75359893203331, "y"=229.15814211501416, "position"=-79.29119275505313, "velocity"=-47.94834439545387, "acceleration"=10.386354617394034, "jerk"=-32.21085999285833, "heading"=-5.926281829628833}, {"dt"=0.005, "x"=78.97781225880973, "y"=229.07398740189245, "position"=-79.53067893762896, "velocity"=-47.89723651516734, "acceleration"=10.221576057305981, "jerk"=-32.955712017610495, "heading"=-5.921959427215067}, {"dt"=0.005, "x"=79.20142406030115, "y"=228.98895165583954, "position"=-79.7699137926836, "velocity"=-47.846971010926545, "acceleration"=10.053100848159602, "jerk"=-33.69504182927585, "heading"=-5.917619072704923}, {"dt"=0.005, "x"=79.4244333925326, "y"=228.9030329943193, "position"=-80.00890161383721, "velocity"=-47.79756423072276, "acceleration"=9.881356040756373, "jerk"=-34.34896148064581, "heading"=-5.913261073599663}, {"dt"=0.005, "x"=79.64683938431422, "y"=228.8162295608545, "position"=-80.24764679439933, "velocity"=-47.74903611242331, "acceleration"=9.70562365989025, "jerk"=-35.14647617322453, "heading"=-5.908885743708284}, {"dt"=0.005, "x"=79.86864123622914, "y"=228.72853952477934, "position"=-80.48615382561593, "velocity"=-47.701406243318466, "acceleration"=9.525973820969114, "jerk"=-35.9299677842273, "heading"=-5.904493403087157}, {"dt"=0.005, "x"=80.08983820579525, "y"=228.6399610865676, "position"=-80.724427279994, "velocity"=-47.65469087561411, "acceleration"=9.343073540871671, "jerk"=-36.58005601948844, "heading"=-5.900084378248678}, {"dt"=0.005, "x"=80.31042961410097, "y"=228.55049247482785, "position"=-80.96247181764387, "velocity"=-47.608907529974694, "acceleration"=9.156669127882822, "jerk"=-37.28088259776996, "heading"=-5.895659001940866}, {"dt"=0.005, "x"=80.5304148453827, "y"=228.46013194598916, "position"=-81.20029218505188, "velocity"=-47.56407348160227, "acceleration"=8.966809674484466, "jerk"=-37.971890679671105, "heading"=-5.891217613056247}, {"dt"=0.005, "x"=80.74979334612426, "y"=228.3688777841755, "position"=-81.43789321332392, "velocity"=-47.52020565440812, "acceleration"=8.773565438829678, "jerk"=-38.64884713095762, "heading"=-5.886760556542263}, {"dt"=0.005, "x"=80.96856458967152, "y"=228.27672831569924, "position"=-81.67527977895826, "velocity"=-47.477313126869, "acceleration"=8.57850550782473, "jerk"=-39.01198620098967, "heading"=-5.882288184010929}, {"dt"=0.005, "x"=81.18672817701427, "y"=228.1836818662178, "position"=-81.91245691234882, "velocity"=-47.43542667811265, "acceleration"=8.377289751270212, "jerk"=-40.24315131090361, "heading"=-5.877800851557132}, {"dt"=0.005, "x"=81.40428373889841, "y"=228.08973680097432, "position"=-82.14942969093387, "velocity"=-47.39455571701228, "acceleration"=8.17419222007345, "jerk"=-40.61950623935218, "heading"=-5.8732989216162235}, {"dt"=0.005, "x"=81.62123096602015, "y"=227.99489151179228, "position"=-82.38620327103908, "velocity"=-47.35471602104107, "acceleration"=7.967939194242035, "jerk"=-41.250605166283094, "heading"=-5.868782762212121}, {"dt"=0.005, "x"=81.83756958953268, "y"=227.89914442520302, "position"=-82.62278286570782, "velocity"=-47.31591893374809, "acceleration"=7.759417458596829, "jerk"=-41.70434712904125, "heading"=-5.8642527472177575}, {"dt"=0.005, "x"=82.05329939495758, "y"=227.80249399612524, "position"=-82.8591737589114, "velocity"=-47.27817864071531, "acceleration"=7.54805860655523, "jerk"=-42.27177040831975, "heading"=-5.859709255915605}, {"dt"=0.005, "x"=82.26842028090483, "y"=227.70493868062283, "position"=-83.09538136918995, "velocity"=-47.2415220557114, "acceleration"=7.331317000782178, "jerk"=-43.3483211546104, "heading"=-5.855152671587654}, {"dt"=0.005, "x"=82.48293216828338, "y"=227.60647697572537, "position"=-83.33141114942546, "velocity"=-47.205956047101445, "acceleration"=7.113201721990947, "jerk"=-43.62305575824621, "heading"=-5.85058338324868}, {"dt"=0.005, "x"=82.69683498324869, "y"=227.5071074277589, "position"=-83.56726856676302, "velocity"=-47.171483467511095, "acceleration"=6.894515918069999, "jerk"=-43.737160784189655, "heading"=-5.846001785852594}, {"dt"=0.005, "x"=82.91012876999085, "y"=227.40682857983035, "position"=-83.80295922590057, "velocity"=-47.13813182750815, "acceleration"=6.67032800058962, "jerk"=-44.837583496075695, "heading"=-5.841408277698225}, {"dt"=0.005, "x"=83.1228136367988, "y"=227.30563899528065, "position"=-84.0384888091602, "velocity"=-47.10591665192619, "acceleration"=6.443035116392082, "jerk"=-45.458576839507714, "heading"=-5.836803261367771}, {"dt"=0.005, "x"=83.33488966278009, "y"=227.20353730196283, "position"=-84.27386297208889, "velocity"=-47.07483258573859, "acceleration"=6.216813237519148, "jerk"=-45.24437577458684, "heading"=-5.832187145554138}, {"dt"=0.005, "x"=83.54635703209941, "y"=227.10052212819727, "position"=-84.50908749103363, "velocity"=-47.044903788947174, "acceleration"=5.98575935828336, "jerk"=-46.21077584715749, "heading"=-5.827560341953144}, {"dt"=0.005, "x"=83.75721601938125, "y"=226.99659210788795, "position"=-84.7441682466029, "velocity"=-47.01615111385376, "acceleration"=5.750535018682967, "jerk"=-47.04486792007856, "heading"=-5.822923265338563}, {"dt"=0.005, "x"=83.96746679614785, "y"=226.89174597584528, "position"=-84.97911100672813, "velocity"=-46.98855202504835, "acceleration"=5.519817761081924, "jerk"=-46.1434515202086, "heading"=-5.818276337606002}, {"dt"=0.005, "x"=84.17710976594904, "y"=226.78598240156728, "position"=-85.21392179956169, "velocity"=-46.96215856671103, "acceleration"=5.27869166746342, "jerk"=-48.22521872370089, "heading"=-5.813619980165323}, {"dt"=0.005, "x"=84.3861452435323, "y"=226.6793001479531, "position"=-85.44860655433853, "velocity"=-46.93695095536723, "acceleration"=5.0415222687604455, "jerk"=-47.433879740594875, "heading"=-5.80895462078329}, {"dt"=0.005, "x"=84.59457362492108, "y"=226.5716979863798, "position"=-85.68317129027211, "velocity"=-46.912947186716664, "acceleration"=4.800753730113172, "jerk"=-48.15370772945471, "heading"=-5.804280689592593}, {"dt"=0.005, "x"=84.80239537807476, "y"=226.4631746999684, "position"=-85.91762210553493, "velocity"=-46.890163052564766, "acceleration"=4.556826830379634, "jerk"=-48.78537994670751, "heading"=-5.799598619037334}, {"dt"=0.005, "x"=85.0096109287986, "y"=226.35372914276925, "position"=-86.15196504750762, "velocity"=-46.86858839453568, "acceleration"=4.314931605817662, "jerk"=-48.37904491239442, "heading"=-5.794908846195476}, {"dt"=0.005, "x"=85.21622084251726, "y"=226.24336014408578, "position"=-86.38620631696547, "velocity"=-46.848253891570415, "acceleration"=4.06690059305248, "jerk"=-49.60620255303638, "heading"=-5.790211808424604}, {"dt"=0.005, "x"=85.42222562338328, "y"=226.13206661408205, "position"=-86.62035203988253, "velocity"=-46.82914458341129, "acceleration"=3.8218616318246745, "jerk"=-49.00779224556118, "heading"=-5.785507947649204}, {"dt"=0.005, "x"=85.62762586655732, "y"=226.0198474626329, "position"=-86.85440843874385, "velocity"=-46.81127977226121, "acceleration"=3.5729622300166852, "jerk"=-49.77988036159786, "heading"=-5.7807977066471015}, {"dt"=0.005, "x"=85.8324222151638, "y"=225.90670162108776, "position"=-87.08838178308355, "velocity"=-46.79466886793957, "acceleration"=3.3221808643276063, "jerk"=-50.15627313781579, "heading"=-5.776081529749057}, {"dt"=0.005, "x"=86.03661521371392, "y"=225.7926281237268, "position"=-87.32227822054477, "velocity"=-46.7792874922443, "acceleration"=3.076275139054019, "jerk"=-49.18114505471749, "heading"=-5.771359865959071}, {"dt"=0.005, "x"=86.24020564285041, "y"=225.67762592126948, "position"=-87.55610415881085, "velocity"=-46.765187653216564, "acceleration"=2.8199678055472077, "jerk"=-51.261466701362224, "heading"=-5.766633160955895}, {"dt"=0.005, "x"=86.44319412751794, "y"=225.56169409907213, "position"=-87.7898658158584, "velocity"=-46.75233140951083, "acceleration"=2.5712487411468032, "jerk"=-49.743812880080895, "heading"=-5.761901865874054}, {"dt"=0.005, "x"=86.64558136446355, "y"=225.44483175044107, "position"=-88.0235694790861, "velocity"=-46.74073264554005, "acceleration"=2.3197527941562157, "jerk"=-50.299189398117505, "heading"=-5.757166431777991}, {"dt"=0.005, "x"=86.84736815826469, "y"=225.32703795373038, "position"=-88.25722154669104, "velocity"=-46.73041352098632, "acceleration"=2.063824910746348, "jerk"=-51.185576681973544, "heading"=-5.752427308515466}, {"dt"=0.005, "x"=87.04855525831216, "y"=225.20831186609587, "position"=-88.49082833835283, "velocity"=-46.7213583323566, "acceleration"=1.8110377259432653, "jerk"=-50.55743696061654, "heading"=-5.747684948252241}, {"dt"=0.005, "x"=87.2491433445387, "y"=225.08865273424684, "position"=-88.72439607621679, "velocity"=-46.71354757279168, "acceleration"=1.5621519129837225, "jerk"=-49.777162591908564, "heading"=-5.742939805564259}, {"dt"=0.005, "x"=87.44913328520552, "y"=224.96805974083426, "position"=-88.95793118370199, "velocity"=-46.707021497040365, "acceleration"=1.3052151502634501, "jerk"=-51.387352544054465, "heading"=-5.738192331064355}, {"dt"=0.005, "x"=87.64852589173636, "y"=224.84653214897057, "position"=-89.19143999964552, "velocity"=-46.70176318870619, "acceleration"=1.0516616668354573, "jerk"=-50.71069668559858, "heading"=-5.733442976902621}, {"dt"=0.005, "x"=87.84732197675088, "y"=224.72406926848385, "position"=-89.42492884416322, "velocity"=-46.69776890353801, "acceleration"=0.7988570336351586, "jerk"=-50.56092664005973, "heading"=-5.728692195128212}, {"dt"=0.005, "x"=88.04552236439807, "y"=224.60067044974483, "position"=-89.65840402941785, "velocity"=-46.695037050925265, "acceleration"=0.5463705225494664, "jerk"=-50.49730221713844, "heading"=-5.7239404371684195}, {"dt"=0.005, "x"=88.24312788880346, "y"=224.47633508457878, "position"=-89.89187185655149, "velocity"=-46.69356542672803, "acceleration"=0.294324839447313, "jerk"=-50.40913662043067, "heading"=-5.719188153589799}, {"dt"=0.005, "x"=88.44013939255632, "y"=224.35106260718567, "position"=-90.12533861265003, "velocity"=-46.69335121970629, "acceleration"=0.042841404348337164, "jerk"=-50.29668701979517, "heading"=-5.714435793860156}, {"dt"=0.005, "x"=88.63655772523919, "y"=224.22485249506548, "position"=-90.3588105677438, "velocity"=-46.694391018754594, "acceleration"=-0.2079598096614177, "jerk"=-50.16024280195097, "heading"=-5.709683806111728}, {"dt"=0.005, "x"=88.8323837420029, "y"=224.0977042699463, "position"=-90.5922939718489, "velocity"=-46.69668082101895, "acceleration"=-0.45796045287147535, "jerk"=-50.00012864201153, "heading"=-5.704932636905834}, {"dt"=0.005, "x"=89.02761830219066, "y"=223.9696174987111, "position"=-90.82579505205446, "velocity"=-46.70021604111164, "acceleration"=-0.7070440185373172, "jerk"=-49.81671313316838, "heading"=-5.700182730999352}, {"dt"=0.005, "x"=89.22226226801274, "y"=223.84059179432091, "position"=-91.05932000965927, "velocity"=-46.704991520963375, "acceleration"=-0.955095970347486, "jerk"=-49.61039036203374, "heading"=-5.695434531113294}, {"dt"=0.005, "x"=89.41631650327511, "y"=223.7106268167308, "position"=-91.29287501736252, "velocity"=-46.71100154064792, "acceleration"=-1.2020039369090796, "jerk"=-49.38159331231873, "heading"=-5.690688477703819}, {"dt"=0.005, "x"=89.60978187216426, "y"=223.57972227379557, "position"=-91.52646621651287, "velocity"=-46.71823983007033, "acceleration"=-1.447657884482112, "jerk"=-49.13078951460648, "heading"=-5.685945008735936}, {"dt"=0.005, "x"=89.80265923809017, "y"=223.44787792216155, "position"=-91.76009971441998, "velocity"=-46.726699581421755, "acceleration"=-1.6919502702847922, "jerk"=-48.85847716053604, "heading"=-5.681204559460232}, {"dt"=0.005, "x"=89.99494946258945, "y"=223.31509356814198, "position"=-91.99378158173188, "velocity"=-46.73637346238053, "acceleration"=-1.9347761917543949, "jerk"=-48.56518429392054, "heading"=-5.676467562192888}, {"dt"=0.005, "x"=90.18665333324071, "y"=223.1813691183836, "position"=-92.22751776311135, "velocity"=-46.74723627589463, "acceleration"=-2.1725627028203576, "jerk"=-47.55730221319254, "heading"=-5.671734447855372}, {"dt"=0.005, "x"=90.37777167610466, "y"=223.0467045028995, "position"=-92.46131421227716, "velocity"=-46.759289833161645, "acceleration"=-2.4107114534032803, "jerk"=-47.629750116584546, "heading"=-5.667005642971311}, {"dt"=0.005, "x"=90.56830541419946, "y"=222.9110996319214, "position"=-92.69517696344838, "velocity"=-46.77255023424255, "acceleration"=-2.6520802161812185, "jerk"=-48.273752555587635, "heading"=-5.662281567972211}, {"dt"=0.005, "x"=90.75825533329963, "y"=222.7745545616331, "position"=-92.92911184324657, "velocity"=-46.78697595963934, "acceleration"=-2.8851450793581535, "jerk"=-46.612972635386996, "heading"=-5.6575626427712296}, {"dt"=0.005, "x"=90.94762213919616, "y"=222.63706945727796, "position"=-93.16312453754968, "velocity"=-46.802538860619606, "acceleration"=-3.112580196052761, "jerk"=-45.48702333892152, "heading"=-5.652849285149673}, {"dt"=0.005, "x"=91.13640681933327, "y"=222.49864432955476, "position"=-93.39722103782181, "velocity"=-46.819300054424986, "acceleration"=-3.3522387610759097, "jerk"=-47.93171300462973, "heading"=-5.648141901534325}, {"dt"=0.005, "x"=91.32460994120129, "y"=222.35927954645476, "position"=-93.63140677148075, "velocity"=-46.83714673178905, "acceleration"=-3.5693354728124405, "jerk"=-43.419342347306156, "heading"=-5.643440904268049}, {"dt"=0.005, "x"=91.51223249169973, "y"=222.21897521773127, "position"=-93.8656876416219, "velocity"=-46.85617402822835, "acceleration"=-3.805459287860913, "jerk"=-47.22476300969447, "heading"=-5.63874669047986}, {"dt"=0.005, "x"=91.69927501867201, "y"=222.0777318308923, "position"=-94.10006895747689, "velocity"=-46.876263170998065, "acceleration"=-4.017828553942593, "jerk"=-42.47385321633601, "heading"=-5.634059663334965}, {"dt"=0.005, "x"=91.8857384891377, "y"=221.93554960965605, "position"=-94.3345565048089, "velocity"=-46.89750946640194, "acceleration"=-4.249259080775403, "jerk"=-46.28610536656197, "heading"=-5.6293802103784625}, {"dt"=0.005, "x"=92.07162338902816, "y"=221.79242919482704, "position"=-94.56915541603425, "velocity"=-46.91978224506933, "acceleration"=-4.45455573347715, "jerk"=-41.05933054034949, "heading"=-5.624708725920152}, {"dt"=0.005, "x"=92.25693060320356, "y"=221.6483709746439, "position"=-94.8038712749526, "velocity"=-46.94317178366881, "acceleration"=-4.677907719896268, "jerk"=-44.670397283823604, "heading"=-5.620045588785963}, {"dt"=0.005, "x"=92.44166083534682, "y"=221.50337552723857, "position"=-95.03870938607594, "velocity"=-46.96762222466816, "acceleration"=-4.89008819987049, "jerk"=-42.436095994844436, "heading"=-5.615391176713777}, {"dt"=0.005, "x"=92.62581460854227, "y"=221.35744362679526, "position"=-95.2736747702267, "velocity"=-46.993076830153626, "acceleration"=-5.09092109709286, "jerk"=-40.16657944447388, "heading"=-5.61074586621205}, {"dt"=0.005, "x"=92.80939267817044, "y"=221.21057591833883, "position"=-95.50877268905128, "velocity"=-47.01958376491507, "acceleration"=-5.301386952288567, "jerk"=-42.09317103914145, "heading"=-5.606110022003944}, {"dt"=0.005, "x"=92.9923957094773, "y"=221.06277317038067, "position"=-95.74400823434894, "velocity"=-47.04710905952992, "acceleration"=-5.505058922970818, "jerk"=-40.73439413645019, "heading"=-5.601484005010324}, {"dt"=0.005, "x"=93.1748243118783, "y"=220.91403625004537, "position"=-95.97938636936749, "velocity"=-47.07562700371031, "acceleration"=-5.703588836077245, "jerk"=-39.70598262128533, "heading"=-5.596868171361825}, {"dt"=0.005, "x"=93.35667907937052, "y"=220.7643660915951, "position"=-96.21491197899452, "velocity"=-47.10512192540535, "acceleration"=-5.8989843390079955, "jerk"=-39.07910058615016, "heading"=-5.592262871257847}, {"dt"=0.005, "x"=93.53794341661808, "y"=220.6137780310779, "position"=-96.45056749861611, "velocity"=-47.13110392431778, "acceleration"=-5.196399782485628, "jerk"=140.51691130447352, "heading"=-5.587668884272488}, {"dt"=0.005, "x"=93.71856596390948, "y"=220.46231728306705, "position"=-96.6862895017852, "velocity"=-47.14440063381708, "acceleration"=-2.6593418998601237, "jerk"=507.4115765251008, "heading"=-5.583087866632939}, {"dt"=0.005, "x"=93.89847821773314, "y"=220.31004532718293, "position"=-96.92199093925362, "velocity"=-47.14028749368559, "acceleration"=0.8226280262974228, "jerk"=696.3939852315093, "heading"=-5.578521906190406}, {"dt"=0.005, "x"=94.07761254818591, "y"=220.15702513942304, "position"=-97.1575844158374, "velocity"=-47.11869531675703, "acceleration"=4.31843538571286, "jerk"=699.1614718830874, "heading"=-5.5739730649440276}, {"dt"=0.005, "x"=94.25590219984323, "y"=220.0033211792382, "position"=-97.39298217977026, "velocity"=-47.07955278657126, "acceleration"=7.828506037152749, "jerk"=702.0141302879779, "heading"=-5.569443377687035}, {"dt"=0.005, "x"=94.43328129275567, "y"=219.8489993737289, "position"=-97.62809611440215, "velocity"=-47.02278692637901, "acceleration"=11.353172038450055, "jerk"=704.933200259461, "heading"=-5.564934850715913}, {"dt"=0.005, "x"=94.60968454193603, "y"=219.69412734731074, "position"=-97.8628373568123, "velocity"=-46.948248482028994, "acceleration"=14.90768887000371, "jerk"=710.9033663107311, "heading"=-5.560449467768328}, {"dt"=0.005, "x"=94.78504798318562, "y"=219.53877376648762, "position"=-98.09711725693492, "velocity"=-46.85598002452291, "acceleration"=18.453691501217406, "jerk"=709.2005262427392, "heading"=-5.555989170446278}, {"dt"=0.005, "x"=94.95930800748299, "y"=219.38300916583674, "position"=-98.3308460888835, "velocity"=-46.74576638971637, "acceleration"=22.04272696130687, "jerk"=717.8070920178925, "heading"=-5.55155588172029}, {"dt"=0.005, "x"=95.13240223695021, "y"=219.22690514919503, "position"=-98.563934218754, "velocity"=-46.61762597409962, "acceleration"=25.628083123351075, "jerk"=717.0712324088413, "heading"=-5.547151482680746}, {"dt"=0.005, "x"=95.3042688573329, "y"=219.07053495659085, "position"=-98.79629121205706, "velocity"=-46.471398660611385, "acceleration"=29.245462697646474, "jerk"=723.4759148590797, "heading"=-5.542777828624852}, {"dt"=0.005, "x"=95.47484690069037, "y"=218.9139731844157, "position"=-99.0278262145562, "velocity"=-46.30700049982998, "acceleration"=32.879632156280536, "jerk"=726.8338917268125, "heading"=-5.5384367410519815}, {"dt"=0.005, "x"=95.64407624658212, "y"=218.75729575097182, "position"=-99.25844796041186, "velocity"=-46.12434917113258, "acceleration"=36.53026573948068, "jerk"=730.1267166400294, "heading"=-5.534130006898206}, {"dt"=0.005, "x"=95.81189762337385, "y"=218.60057985901818, "position"=-99.4880647831821, "velocity"=-45.923364554047254, "acceleration"=40.19692341706502, "jerk"=733.3315355168679, "heading"=-5.529859377848392}, {"dt"=0.005, "x"=95.97825260963901, "y"=218.44390395533335, "position"=-99.716584629696, "velocity"=-45.703969302781495, "acceleration"=43.879050253151775, "jerk"=736.4253672173504, "heading"=-5.525626569726361}, {"dt"=0.005, "x"=96.14309948726446, "y"=218.28733256815713, "position"=-99.94393698254318, "velocity"=-45.470470569435996, "acceleration"=46.699746669099795, "jerk"=564.1392831896042, "heading"=-5.521432858738992}, {"dt"=0.005, "x"=96.30643106572214, "y"=218.13089848860767, "position"=-100.17009804410321, "velocity"=-45.23221231200626, "acceleration"=47.6516514859469, "jerk"=190.3809633694209, "heading"=-5.517278628273556}, {"dt"=0.005, "x"=96.46825687521489, "y"=217.9746186547454, "position"=-100.39506688436782, "velocity"=-44.99376805292228, "acceleration"=47.688851816796785, "jerk"=7.440066169976944, "heading"=-5.513163822743499}, {"dt"=0.005, "x"=96.62858643851132, "y"=217.81850983537262, "position"=-100.6188425138559, "velocity"=-44.755125897615564, "acceleration"=47.72843106134275, "jerk"=7.915848909192391, "heading"=-5.509088373742463}, {"dt"=0.005, "x"=96.78742927415253, "y"=217.66258862264178, "position"=-100.84142389451024, "velocity"=-44.51627613087056, "acceleration"=47.76995334900107, "jerk"=8.304457531664866, "heading"=-5.505052200442722}, {"dt"=0.005, "x"=96.94479469291728, "y"=217.5068716300131, "position"=-101.06280965922045, "velocity"=-44.27715294204161, "acceleration"=47.824637765789646, "jerk"=10.936883357715033, "heading"=-5.501055215236881}, {"dt"=0.005, "x"=97.10069207840789, "y"=217.35137521517308, "position"=-101.28299850959873, "velocity"=-44.03777007565612, "acceleration"=47.87657327709809, "jerk"=10.387102261688597, "heading"=-5.497097317069667}, {"dt"=0.005, "x"=97.25513057653413, "y"=217.19611578632217, "position"=-101.50198878324255, "velocity"=-43.79805472876607, "acceleration"=47.94306937801025, "jerk"=13.299220182432236, "heading"=-5.493178399776215}, {"dt"=0.005, "x"=97.4081194746473, "y"=217.04110942177766, "position"=-101.71977899421445, "velocity"=-43.558042194379816, "acceleration"=48.00250687725054, "jerk"=11.887499848057814, "heading"=-5.489298342901389}, {"dt"=0.005, "x"=97.55966785297545, "y"=216.88637221764301, "position"=-101.93636734412576, "velocity"=-43.317669982261144, "acceleration"=48.074442423734354, "jerk"=14.387109296762901, "heading"=-5.485457020980899}, {"dt"=0.005, "x"=97.7097847936565, "y"=216.73192007610496, "position"=-102.15175202302639, "velocity"=-43.07693578012661, "acceleration"=48.14684042690658, "jerk"=14.479600634444978, "heading"=-5.4816542986619865}, {"dt"=0.005, "x"=97.85847903249261, "y"=216.57776906389228, "position"=-102.36593071297767, "velocity"=-42.83573799025531, "acceleration"=48.239557974260094, "jerk"=18.543509470703157, "heading"=-5.4778900399363515}, {"dt"=0.005, "x"=98.00575981805663, "y"=216.42393452133072, "position"=-102.5789018290509, "velocity"=-42.594223214646355, "acceleration"=48.30295512179106, "jerk"=12.679429506192719, "heading"=-5.474164086793973}, {"dt"=0.005, "x"=98.15163562231925, "y"=216.27043240049883, "position"=-102.79066266435609, "velocity"=-42.35216706103836, "acceleration"=48.41123072159945, "jerk"=21.655119961678793, "heading"=-5.470476292252356}, {"dt"=0.005, "x"=98.29611545375033, "y"=216.11727789477527, "position"=-103.00121129131382, "velocity"=-42.10972539154514, "acceleration"=48.48833389864353, "jerk"=15.420635408815997, "heading"=-5.466826487516799}, {"dt"=0.005, "x"=98.43920797396383, "y"=215.96448636117833, "position"=-103.21054528778825, "velocity"=-41.86679929488552, "acceleration"=48.585219331924634, "jerk"=19.3770866562204, "heading"=-5.463214504699889}, {"dt"=0.005, "x"=98.58092185007224, "y"=215.81207295005413, "position"=-103.41866225147018, "velocity"=-41.62339273638557, "acceleration"=48.68131169998975, "jerk"=19.21847361302298, "heading"=-5.459640168274068}, {"dt"=0.005, "x"=98.72126546972561, "y"=215.6600529112918, "position"=-103.62555938475796, "velocity"=-41.379426657557474, "acceleration"=48.793215765618925, "jerk"=22.380813125835175, "heading"=-5.456103302609979}, {"dt"=0.005, "x"=98.86024757495846, "y"=215.5084409079104, "position"=-103.83123443220973, "velocity"=-41.1350094903517, "acceleration"=48.88343344115498, "jerk"=18.043535107210573, "heading"=-5.452603716342383}, {"dt"=0.005, "x"=98.9978764202938, "y"=215.35725192737274, "position"=-104.03568444298095, "velocity"=-40.890002154245366, "acceleration"=49.00146722126664, "jerk"=23.606756022331865, "heading"=-5.449141223918887}, {"dt"=0.005, "x"=99.13416054260253, "y"=215.2065004425958, "position"=-104.2389069125947, "velocity"=-40.64449392275076, "acceleration"=49.1016462989208, "jerk"=20.035815530832224, "heading"=-5.445715626532774}, {"dt"=0.005, "x"=99.26910819782367, "y"=215.05620102767128, "position"=-104.44089895148815, "velocity"=-40.398407778691556, "acceleration"=49.217228811841096, "jerk"=23.116502584059617, "heading"=-5.442326726612822}, {"dt"=0.005, "x"=99.40272764882154, "y"=214.90636804171837, "position"=-104.64165771559207, "velocity"=-40.15175282078612, "acceleration"=49.33099158108689, "jerk"=22.752553849159085, "heading"=-5.43897432088119}, {"dt"=0.005, "x"=99.5350271664979, "y"=214.75701562448228, "position"=-104.84118041332759, "velocity"=-39.90453954710392, "acceleration"=49.442654736439806, "jerk"=22.33263107058292, "heading"=-5.435658200625364}, {"dt"=0.005, "x"=99.66601472486198, "y"=214.60815804091916, "position"=-105.03946384841593, "velocity"=-39.65668701766879, "acceleration"=49.57050588702714, "jerk"=25.570230117466508, "heading"=-5.432378159620651}, {"dt"=0.005, "x"=99.79569861891906, "y"=214.45980898047705, "position"=-105.23650535701721, "velocity"=-39.40830172025505, "acceleration"=49.67705948274812, "jerk"=21.310719144196355, "heading"=-5.429133978923922}, {"dt"=0.005, "x"=99.92408661164838, "y"=214.31198252778464, "position"=-105.43230151835007, "velocity"=-39.15923226657295, "acceleration"=49.81389073641935, "jerk"=27.366250734246478, "heading"=-5.4259254484911}, {"dt"=0.005, "x"=100.05118686459713, "y"=214.16469209802318, "position"=-105.62684957153732, "velocity"=-38.90961063745068, "acceleration"=49.92432582445332, "jerk"=22.087017606793324, "heading"=-5.422752344150146}, {"dt"=0.005, "x"=100.17700724003429, "y"=214.01795123604902, "position"=-105.82014635746008, "velocity"=-38.65935718455165, "acceleration"=50.0506905798062, "jerk"=25.272951070576255, "heading"=-5.4196144452989365}, {"dt"=0.005, "x"=100.30155560755057, "y"=213.87177326406623, "position"=-106.01218878856312, "velocity"=-38.40848622060995, "acceleration"=50.17419278834012, "jerk"=24.700441706784204, "heading"=-5.4165115274752305}, {"dt"=0.005, "x"=100.42483960133256, "y"=213.72617156652456, "position"=-106.20297347728278, "velocity"=-38.15693774393209, "acceleration"=50.30969533557226, "jerk"=27.100509446427168, "heading"=-5.413443368629285}, {"dt"=0.005, "x"=100.54686707779278, "y"=213.58115905091807, "position"=-106.39249744593522, "velocity"=-37.904793730486965, "acceleration"=50.428802689025076, "jerk"=23.82147069056373, "heading"=-5.410409737947433}, {"dt"=0.005, "x"=100.66764563846844, "y"=213.43674870958066, "position"=-106.58075739229682, "velocity"=-37.65198927232085, "acceleration"=50.56089163322355, "jerk"=26.417788839694367, "heading"=-5.4074104079406}, {"dt"=0.005, "x"=100.78718297899216, "y"=213.29295320572368, "position"=-106.76775023362762, "velocity"=-37.398568266160225, "acceleration"=50.68420123212434, "jerk"=24.66191978015786, "heading"=-5.404445145967095}, {"dt"=0.005, "x"=100.90548655689294, "y"=213.1497852711033, "position"=-106.95347259105287, "velocity"=-37.14447148504877, "acceleration"=50.81935622229139, "jerk"=27.03099803341047, "heading"=-5.40151372267339}, {"dt"=0.005, "x"=101.02256383526574, "y"=213.00725741502035, "position"=-107.13792117161337, "velocity"=-36.88971611210098, "acceleration"=50.95107458955823, "jerk"=26.34367345336841, "heading"=-5.398615906126887}, {"dt"=0.005, "x"=101.13842228305377, "y"=212.8653819217271, "position"=-107.32109277290859, "velocity"=-36.63432025904228, "acceleration"=51.07917061173879, "jerk"=25.61920443611143, "heading"=-5.395751461995211}, {"dt"=0.005, "x"=101.25306937525453, "y"=212.7241708479944, "position"=-107.50298428753979, "velocity"=-36.378302926239996, "acceleration"=51.2034665604574, "jerk"=24.859189743722254, "heading"=-5.39292015372012}, {"dt"=0.005, "x"=101.36651219051636, "y"=212.58363652093334, "position"=-107.68359206538182, "velocity"=-36.121555568405974, "acceleration"=51.34947156680454, "jerk"=29.201001269427707, "heading"=-5.390121752610247}, {"dt"=0.005, "x"=101.47875827111794, "y"=212.44379047569038, "position"=-107.8629132827001, "velocity"=-35.86424346365766, "acceleration"=51.46242094966311, "jerk"=22.58987657171474, "heading"=-5.387356016771849}, {"dt"=0.005, "x"=101.58981451677691, "y"=212.30464482715155, "position"=-108.04094418228543, "velocity"=-35.60617991706339, "acceleration"=51.61270931885298, "jerk"=30.057673837973198, "heading"=-5.384622718540851}, {"dt"=0.005, "x"=101.69968821406812, "y"=212.1662109901465, "position"=-108.21768171815253, "velocity"=-35.34750717342159, "acceleration"=51.73454872836061, "jerk"=24.367881901525834, "heading"=-5.381921619250733}, {"dt"=0.005, "x"=101.80838647130483, "y"=212.02850038211528, "position"=-108.39312265605082, "velocity"=-35.08818757965617, "acceleration"=51.86391875308374, "jerk"=25.874004944625995, "heading"=-5.379252483299963}, {"dt"=0.005, "x"=101.91591621297158, "y"=211.89152443478864, "position"=-108.56726356304556, "velocity"=-34.82818139894811, "acceleration"=52.00123614161214, "jerk"=27.46347770568036, "heading"=-5.376615078401357}, {"dt"=0.005, "x"=102.02228437296662, "y"=211.75529435076314, "position"=-108.74010112046386, "velocity"=-34.56751148366078, "acceleration"=52.13398305746608, "jerk"=26.549383170788587, "heading"=-5.3740091709566045}, {"dt"=0.005, "x"=102.12749812183858, "y"=211.61982080822102, "position"=-108.91163249858636, "velocity"=-34.30627562449903, "acceleration"=52.24717183235015, "jerk"=22.637754976813085, "heading"=-5.371434520626398}, {"dt"=0.005, "x"=102.23156384174362, "y"=211.4851152816944, "position"=-109.0818536868567, "velocity"=-34.044237654070294, "acceleration"=52.40759408574718, "jerk"=32.08445067940602, "heading"=-5.36889090552446}, {"dt"=0.005, "x"=102.33448867980206, "y"=211.35118804087074, "position"=-109.25076202923206, "velocity"=-33.781668475072756, "acceleration"=52.51383579950755, "jerk"=21.248342752073768, "heading"=-5.366378084319444}, {"dt"=0.005, "x"=102.43627926265356, "y"=211.21804980890272, "position"=-109.41835412799813, "velocity"=-33.518419753214246, "acceleration"=52.649744371701956, "jerk"=27.181714438881954, "heading"=-5.363895827781472}, {"dt"=0.005, "x"=102.53694221721497, "y"=211.0857110922134, "position"=-109.58462669445457, "velocity"=-33.254513291288966, "acceleration"=52.78129238505613, "jerk"=26.309602670835375, "heading"=-5.3614439061364445}, {"dt"=0.005, "x"=102.63648417053147, "y"=210.95418217931189, "position"=-109.74957655168129, "velocity"=-32.989971445344224, "acceleration"=52.90836918894826, "jerk"=25.415360778424656, "heading"=-5.359022089169735}, {"dt"=0.005, "x"=102.73491174959024, "y"=210.82347313972937, "position"=-109.91320063715757, "velocity"=-32.72481709525798, "acceleration"=53.03087001724833, "jerk"=24.500165660015227, "heading"=-5.356630146326033}, {"dt"=0.005, "x"=102.83223118927496, "y"=210.6935943472737, "position"=-110.07549535078157, "velocity"=-32.45894272479966, "acceleration"=53.17487409166404, "jerk"=28.8008148831409, "heading"=-5.354267856310927}, {"dt"=0.005, "x"=102.92844925778462, "y"=210.5645552475361, "position"=-110.23645809792765, "velocity"=-32.192549429217166, "acceleration"=53.27865911649923, "jerk"=20.75700496703803, "heading"=-5.351934984698101}, {"dt"=0.005, "x"=103.02357194653416, "y"=210.43636610908032, "position"=-110.39608510420472, "velocity"=-31.92540125541253, "acceleration"=53.42963476092706, "jerk"=30.19512888556619, "heading"=-5.349631315795363}, {"dt"=0.005, "x"=103.1176058357349, "y"=210.30903619396275, "position"=-110.55437370013654, "velocity"=-31.657719186363163, "acceleration"=53.53641380987355, "jerk"=21.35580978929852, "heading"=-5.347356619600318}, {"dt"=0.005, "x"=103.21055711096828, "y"=210.18257507873372, "position"=-110.71132067599935, "velocity"=-31.389395172562157, "acceleration"=53.66480276020127, "jerk"=25.677790065543604, "heading"=-5.345110675704622}, {"dt"=0.005, "x"=103.30243195477381, "y"=210.05699212953198, "position"=-110.86692293836882, "velocity"=-31.1204524738941, "acceleration"=53.788539733611174, "jerk"=24.74739468198095, "heading"=-5.342893263864422}, {"dt"=0.005, "x"=103.39323654638876, "y"=209.932296501481, "position"=-111.02117751208831, "velocity"=-30.850914743900276, "acceleration"=53.907545998765016, "jerk"=23.80125303076852, "heading"=-5.34070416407318}, {"dt"=0.005, "x"=103.4829767619333, "y"=209.80849755233587, "position"=-111.17408103099949, "velocity"=-30.58070378223567, "acceleration"=54.042192332921246, "jerk"=26.929266831245968, "heading"=-5.338543163840311}, {"dt"=0.005, "x"=103.57165881064093, "y"=209.68560396732536, "position"=-111.32563082149659, "velocity"=-30.309958099420054, "acceleration"=54.14913656312308, "jerk"=21.388846040366616, "heading"=-5.33641004291532}, {"dt"=0.005, "x"=103.65928851289378, "y"=209.5636247550312, "position"=-111.47582367401903, "velocity"=-30.03857050448656, "acceleration"=54.27751898669868, "jerk"=25.676484715120296, "heading"=-5.334304590726418}, {"dt"=0.005, "x"=103.74587190384318, "y"=209.4425684127097, "position"=-111.62465687463153, "velocity"=-29.76664012249892, "acceleration"=54.38607639752817, "jerk"=21.711482165898133, "heading"=-5.332226591903446}, {"dt"=0.005, "x"=103.83141471339795, "y"=209.32244365063895, "position"=-111.77212731481897, "velocity"=-29.4940880374895, "acceleration"=54.51041700188384, "jerk"=24.868120871133215, "heading"=-5.330175838817026}, {"dt"=0.005, "x"=103.91592266548467, "y"=209.2032589776143, "position"=-111.91823200416837, "velocity"=-29.22093786987982, "acceleration"=54.63003352193638, "jerk"=23.923304010509128, "heading"=-5.3281521244238625}, {"dt"=0.005, "x"=103.99940147776147, "y"=209.08502270067805, "position"=-112.06296807183254, "velocity"=-28.94721353283493, "acceleration"=54.74486740897788, "jerk"=22.966777408299777, "heading"=-5.326155242318435}, {"dt"=0.005, "x"=104.0818568613182, "y"=208.96774292493072, "position"=-112.20633276789414, "velocity"=-28.67293921231885, "acceleration"=54.85486410321627, "jerk"=21.99933884767802, "heading"=-5.324184986782299}, {"dt"=0.005, "x"=104.16329452036487, "y"=208.8514275534206, "position"=-112.34832346463354, "velocity"=-28.398139347880115, "acceleration"=54.959972887746744, "jerk"=21.021756906094424, "heading"=-5.3222411528310944}, {"dt"=0.005, "x"=104.24371963824638, "y"=208.73608502529277, "position"=-112.48893675839047, "velocity"=-28.122658751385565, "acceleration"=55.09611929890994, "jerk"=27.229282232639207, "heading"=-5.32032354850015}, {"dt"=0.005, "x"=104.32313807759577, "y"=208.62172259857533, "position"=-112.62817056589925, "velocity"=-27.846761501757687, "acceleration"=55.1794499255756, "jerk"=16.666125333131276, "heading"=-5.3184319662441615}, {"dt"=0.005, "x"=104.40155497527017, "y"=208.5083483652342, "position"=-112.76602166900172, "velocity"=-27.57022062049128, "acceleration"=55.30817625328126, "jerk"=25.745265541132767, "heading"=-5.316566216469471}, {"dt"=0.005, "x"=104.4789757241026, "y"=208.39596984361117, "position"=-112.90248743200458, "velocity"=-27.293152600572906, "acceleration"=55.413603983674875, "jerk"=21.085546078722928, "heading"=-5.314726104152716}, {"dt"=0.005, "x"=104.55540569440883, "y"=208.28459437702782, "position"=-113.03756531664034, "velocity"=-27.0155769271522, "acceleration"=55.51513468414129, "jerk"=20.306140093282465, "heading"=-5.312911435511433}, {"dt"=0.005, "x"=104.63085012236432, "y"=208.17422929744254, "position"=-113.17125268515882, "velocity"=-26.737473703695972, "acceleration"=55.6206446912455, "jerk"=21.102001420842953, "heading"=-5.311122020675102}, {"dt"=0.005, "x"=104.70531398314961, "y"=208.06488211528247, "position"=-113.30354657318618, "velocity"=-26.45877760547287, "acceleration"=55.739219644620164, "jerk"=23.714990674932324, "heading"=-5.309357676698809}, {"dt"=0.005, "x"=104.77880255715218, "y"=207.9565596899474, "position"=-113.43444469517196, "velocity"=-26.17962439715568, "acceleration"=55.83064166343803, "jerk"=18.28440376357321, "heading"=-5.307618214161055}, {"dt"=0.005, "x"=104.85132096115507, "y"=207.84926891572252, "position"=-113.5639446146812, "velocity"=-25.89998390184873, "acceleration"=55.92809906138996, "jerk"=19.491479590385552, "heading"=-5.305903448303006}, {"dt"=0.005, "x"=104.92287395743529, "y"=207.74301700978012, "position"=-113.69204339997236, "velocity"=-25.61975705823114, "acceleration"=56.04536872351815, "jerk"=23.453932425638868, "heading"=-5.3042132035372}, {"dt"=0.005, "x"=104.99346659275064, "y"=207.637810567218, "position"=-113.81873876578084, "velocity"=-25.33907316169468, "acceleration"=56.13677930729182, "jerk"=18.282116754733124, "heading"=-5.302547298353757}, {"dt"=0.005, "x"=105.06310377209182, "y"=207.5336561915739, "position"=-113.94402831327946, "velocity"=-25.057909499723852, "acceleration"=56.23273239416591, "jerk"=19.190617374817975, "heading"=-5.3009055554160724}, {"dt"=0.005, "x"=105.13179024909641, "y"=207.43056051257992, "position"=-114.0679095110075, "velocity"=-24.776239545606597, "acceleration"=56.333990823451074, "jerk"=20.251685857033408, "heading"=-5.299287801786878}, {"dt"=0.005, "x"=105.19953076590545, "y"=207.328529978677, "position"=-114.19037994607682, "velocity"=-24.494087013863187, "acceleration"=56.43050634868203, "jerk"=19.30310504619115, "heading"=-5.29769386563739}, {"dt"=0.005, "x"=105.26633005289607, "y"=207.2275708572749, "position"=-114.31143732477278, "velocity"=-24.211475739193045, "acceleration"=56.52225493402838, "jerk"=18.349717069270355, "heading"=-5.296123576266811}, {"dt"=0.005, "x"=105.33219275953482, "y"=207.1276893396931, "position"=-114.43107934782584, "velocity"=-23.928404610612997, "acceleration"=56.614225716009514, "jerk"=18.394156396226435, "heading"=-5.29457676573744}, {"dt"=0.005, "x"=105.39712319898382, "y"=207.0288919320987, "position"=-114.54930324437139, "velocity"=-23.64477930910943, "acceleration"=56.72506030071318, "jerk"=22.166916940733472, "heading"=-5.2930532748674874}, {"dt"=0.005, "x"=105.46112626717459, "y"=206.931184058194, "position"=-114.66610744532672, "velocity"=-23.360840191064458, "acceleration"=56.787823608994614, "jerk"=12.552661656286546, "heading"=-5.291552931671084}, {"dt"=0.005, "x"=105.52420609377769, "y"=206.8345721138191, "position"=-114.78148912636914, "velocity"=-23.076336208485014, "acceleration"=56.900796515888885, "jerk"=22.594581378854173, "heading"=-5.290075583011444}, {"dt"=0.005, "x"=105.58636717204843, "y"=206.7390617467954, "position"=-114.89544626682459, "velocity"=-22.791428091090204, "acceleration"=56.98162347896201, "jerk"=16.165392614624352, "heading"=-5.2886210681029056}, {"dt"=0.005, "x"=105.6476138794456, "y"=206.64465858771018, "position"=-115.0079767765198, "velocity"=-22.506101939039837, "acceleration"=57.0652304100733, "jerk"=16.72138622225816, "heading"=-5.287189229759931}, {"dt"=0.005, "x"=105.70795045588545, "y"=206.5513682861192, "position"=-115.11907845439829, "velocity"=-22.220335575698204, "acceleration"=57.15327266832659, "jerk"=17.608451650659163, "heading"=-5.285779914900134}, {"dt"=0.005, "x"=105.76738112771751, "y"=206.45919632097005, "position"=-115.22874921583391, "velocity"=-21.93415228712394, "acceleration"=57.23665771485287, "jerk"=16.677009305254842, "heading"=-5.2843929716448965}, {"dt"=0.005, "x"=105.82591005246971, "y"=206.36814808671934, "position"=-115.336986991092, "velocity"=-21.647555051617005, "acceleration"=57.319447101387055, "jerk"=16.557877306837554, "heading"=-5.283028250611857}, {"dt"=0.005, "x"=105.88354108714185, "y"=206.27822925672905, "position"=-115.44378929511306, "velocity"=-21.360460804210486, "acceleration"=57.418849481303624, "jerk"=19.880475983313772, "heading"=-5.281685610309124}, {"dt"=0.005, "x"=105.94027868048352, "y"=206.18944439157497, "position"=-115.54915488142393, "velocity"=-21.0731172621734, "acceleration"=57.46870840741707, "jerk"=9.971785222688823, "heading"=-5.280364896349182}, {"dt"=0.005, "x"=105.99612634700317, "y"=206.10179932364056, "position"=-115.6530809117961, "velocity"=-20.785206074433418, "acceleration"=57.582237547996584, "jerk"=22.70582811590316, "heading"=-5.279065976987491}, {"dt"=0.005, "x"=106.0510883557414, "y"=206.01529851629093, "position"=-115.75556609158654, "velocity"=-20.497035958089366, "acceleration"=57.63402326881035, "jerk"=10.357144162753684, "heading"=-5.277788703806548}, {"dt"=0.005, "x"=106.10516845462497, "y"=205.9299470629452, "position"=-115.85660829902228, "velocity"=-20.208441487147592, "acceleration"=57.71889418835485, "jerk"=16.97418390889993, "heading"=-5.276532941399424}, {"dt"=0.005, "x"=106.15837037688655, "y"=205.84574989580682, "position"=-115.95620552532128, "velocity"=-19.919445259799513, "acceleration"=57.79924546961581, "jerk"=16.07025625219194, "heading"=-5.275298555577919}, {"dt"=0.005, "x"=106.21069784087307, "y"=205.76271178624097, "position"=-116.054355874926, "velocity"=-19.630069920945083, "acceleration"=57.87506777088609, "jerk"=15.164460254055712, "heading"=-5.274085413377754}, {"dt"=0.005, "x"=106.26215454985788, "y"=205.680837345182, "position"=-116.15105756569854, "velocity"=-19.34033815450704, "acceleration"=57.94635328760833, "jerk"=14.257103344448296, "heading"=-5.272893383063071}, {"dt"=0.005, "x"=106.31274419185591, "y"=205.60013102357235, "position"=-116.24630892907592, "velocity"=-19.050272675476048, "acceleration"=58.01309580619858, "jerk"=13.348503718049187, "heading"=-5.271722334130329}, {"dt"=0.005, "x"=106.36247035114711, "y"=205.52059725423524, "position"=-116.34010824348078, "velocity"=-18.759862880971305, "acceleration"=58.08195890094865, "jerk"=13.772618950014248, "heading"=-5.27057213935315}, {"dt"=0.005, "x"=106.41133626017513, "y"=205.44224085219994, "position"=-116.43245326394779, "velocity"=-18.469004093401647, "acceleration"=58.17175751393151, "jerk"=17.959722596572192, "heading"=-5.269442680505774}, {"dt"=0.005, "x"=106.45934568208399, "y"=205.36506560114415, "position"=-116.52334288913983, "velocity"=-18.17792503840552, "acceleration"=58.21581099922568, "jerk"=8.810697058834194, "heading"=-5.268333827957143}, {"dt"=0.005, "x"=106.50650190730661, "y"=205.28907586163598, "position"=-116.61277526631815, "velocity"=-17.88647543566563, "acceleration"=58.28992054797766, "jerk"=14.821909750395434, "heading"=-5.267245463865186}, {"dt"=0.005, "x"=106.55280806490953, "y"=205.21427607679897, "position"=-116.70074837609386, "velocity"=-17.594621955142, "acceleration"=58.37069610472625, "jerk"=16.155111349718254, "heading"=-5.266177474958598}, {"dt"=0.005, "x"=106.59826762565861, "y"=205.1406699597184, "position"=-116.78726098867247, "velocity"=-17.30252251572386, "acceleration"=58.41988788362755, "jerk"=9.8383557802606, "heading"=-5.26512974093265}, {"dt"=0.005, "x"=106.64288378263694, "y"=205.06826149321247, "position"=-116.87231148829036, "velocity"=-17.010099923579933, "acceleration"=58.48451842878575, "jerk"=12.926109031639044, "heading"=-5.264102148735701}, {"dt"=0.005, "x"=106.68665967980154, "y"=204.99705456277272, "position"=-116.955898306122, "velocity"=-16.71736356632528, "acceleration"=58.54727145093079, "jerk"=12.550604429009127, "heading"=-5.263094587286882}, {"dt"=0.005, "x"=106.72959820858433, "y"=204.92705328932368, "position"=-117.03801953077506, "velocity"=-16.42424493061167, "acceleration"=58.62372714272155, "jerk"=15.291138358151102, "heading"=-5.262106952147439}, {"dt"=0.005, "x"=106.7717026889082, "y"=204.8582609197434, "position"=-117.11867421058852, "velocity"=-16.130935962693595, "acceleration"=58.66179358361521, "jerk"=7.613288178731636, "heading"=-5.261139129851073}, {"dt"=0.005, "x"=106.81297599258203, "y"=204.79068125605286, "position"=-117.19786067749214, "velocity"=-15.837293380723132, "acceleration"=58.72851639409262, "jerk"=13.34456209548307, "heading"=-5.260191018063948}, {"dt"=0.005, "x"=106.85342102863325, "y"=204.72431786603366, "position"=-117.27557747410668, "velocity"=-15.543359322908278, "acceleration"=58.7868115629707, "jerk"=11.659033775615057, "heading"=-5.25926251441117}, {"dt"=0.005, "x"=106.89304057619808, "y"=204.65917435753065, "position"=-117.3518230329893, "velocity"=-15.24911177652469, "acceleration"=58.84950927671753, "jerk"=12.53954274936575, "heading"=-5.258353520309939}, {"dt"=0.005, "x"=106.93183759209843, "y"=204.59525387328424, "position"=-117.42659626850221, "velocity"=-14.954647102580617, "acceleration"=58.8929347888147, "jerk"=8.685102419434543, "heading"=-5.257463933907583}, {"dt"=0.005, "x"=106.96981476048958, "y"=204.53255983214427, "position"=-117.49989570992894, "velocity"=-14.659888285344119, "acceleration"=58.951763447299754, "jerk"=11.765731697011006, "heading"=-5.256593660407974}, {"dt"=0.005, "x"=107.00697474888125, "y"=204.47109550958618, "position"=-117.57171999332107, "velocity"=-14.36485667842762, "acceleration"=59.00632138329982, "jerk"=10.911587200013173, "heading"=-5.255742606188441}, {"dt"=0.005, "x"=107.0433202080249, "y"=204.41086403808694, "position"=-117.64206786151425, "velocity"=-14.069573638637042, "acceleration"=59.05660795811549, "jerk"=10.057314963134445, "heading"=-5.25491067879841}, {"dt"=0.005, "x"=107.07885377180617, "y"=204.35186840751962, "position"=-117.7109381641202, "velocity"=-13.774060521188174, "acceleration"=59.10262348977362, "jerk"=9.203106331625577, "heading"=-5.254097786957748}, {"dt"=0.005, "x"=107.11357789387182, "y"=204.29411173737856, "position"=-117.77832954041578, "velocity"=-13.478275259117847, "acceleration"=59.15705241406535, "jerk"=10.88578485834546, "heading"=-5.2533038442868785}, {"dt"=0.005, "x"=107.1474949513368, "y"=204.2375971064826, "position"=-117.84424061909294, "velocity"=-13.18221573543323, "acceleration"=59.211904736923415, "jerk"=10.970464571613547, "heading"=-5.252528766923235}, {"dt"=0.005, "x"=107.18060757049258, "y"=204.18232700989267, "position"=-117.90867065187594, "velocity"=-12.886006556597861, "acceleration"=59.24183576707378, "jerk"=5.986206030073049, "heading"=-5.2517724660762815}, {"dt"=0.005, "x"=107.21291795604398, "y"=204.12830447780738, "position"=-117.97161820931375, "velocity"=-12.589511487563056, "acceleration"=59.29901380696094, "jerk"=11.435607977432483, "heading"=-5.251034863347463}, {"dt"=0.005, "x"=107.24442834350765, "y"=204.07553232319057, "position"=-118.03308205902242, "velocity"=-12.292769941734702, "acceleration"=59.3483091656708, "jerk"=9.859071741971093, "heading"=-5.250315880382631}, {"dt"=0.005, "x"=107.27514111148182, "y"=204.02401295278892, "position"=-118.09306138582106, "velocity"=-11.99586535972674, "acceleration"=59.38091640159264, "jerk"=6.521447184368867, "heading"=-5.249615436310891}, {"dt"=0.005, "x"=107.30505840335925, "y"=203.97374900128457, "position"=-118.15155505363315, "velocity"=-11.698733562418376, "acceleration"=59.42635946167272, "jerk"=9.088612016014963, "heading"=-5.248933456370173}, {"dt"=0.005, "x"=107.33418234539224, "y"=203.9247429671735, "position"=-118.20856203021353, "velocity"=-11.401395316076298, "acceleration"=59.46764926841546, "jerk"=8.257961348547838, "heading"=-5.248269866923766}, {"dt"=0.005, "x"=107.3625150466134, "y"=203.87699721309656, "position"=-118.264081387116, "velocity"=-11.103871380493132, "acceleration"=59.504787116633295, "jerk"=7.427569643567722, "heading"=-5.247624595457939}, {"dt"=0.005, "x"=107.39005839652793, "y"=203.83051430772446, "position"=-118.31811190271918, "velocity"=-10.8061031206378, "acceleration"=59.5536519710663, "jerk"=9.772970886601229, "heading"=-5.2469975751821964}, {"dt"=0.005, "x"=107.41681438546037, "y"=203.7852964866115, "position"=-118.37065268963713, "velocity"=-10.508157383589657, "acceleration"=59.58914740962875, "jerk"=7.099087712489904, "heading"=-5.246388737727301}, {"dt"=0.005, "x"=107.44278510369863, "y"=203.74134565243102, "position"=-118.4217031943454, "velocity"=-10.21010094165479, "acceleration"=59.61128838697327, "jerk"=4.42819546890405, "heading"=-5.245798013166371}, {"dt"=0.005, "x"=107.46797211909276, "y"=203.69866442930305, "position"=-118.47126197310521, "velocity"=-9.911755751962858, "acceleration"=59.66903793838654, "jerk"=11.549910282653286, "heading"=-5.2452253441644885}, {"dt"=0.005, "x"=107.49237738707069, "y"=203.65725462350542, "position"=-118.51932848037661, "velocity"=-9.613301454280107, "acceleration"=59.69085953655018, "jerk"=4.3643196327280975, "heading"=-5.24467066527342}, {"dt"=0.005, "x"=107.51600267730167, "y"=203.6171181938986, "position"=-118.56590194191945, "velocity"=-9.314692308567817, "acceleration"=59.72182914245785, "jerk"=6.193921181534279, "heading"=-5.244133915968822}, {"dt"=0.005, "x"=107.53884961161661, "y"=203.57825718939802, "position"=-118.61098142814528, "velocity"=-9.015897245166322, "acceleration"=59.75901268029915, "jerk"=7.4367075682602035, "heading"=-5.243615039777961}, {"dt"=0.005, "x"=107.56091979450031, "y"=203.54067352812436, "position"=-118.65456611085897, "velocity"=-8.716936542737455, "acceleration"=59.79214048577326, "jerk"=6.625561094821819, "heading"=-5.243113981308587}, {"dt"=0.005, "x"=107.58221481303516, "y"=203.50436899765398, "position"=-118.69665526322717, "velocity"=-8.417830473641729, "acceleration"=59.82121381914531, "jerk"=5.814666674410773, "heading"=-5.242630686246613}, {"dt"=0.005, "x"=107.60273623684921, "y"=203.46934525528366, "position"=-118.73724825972877, "velocity"=-8.118599300319646, "acceleration"=59.84623466441654, "jerk"=5.004169054245722, "heading"=-5.242165101353676}, {"dt"=0.005, "x"=107.62248559747097, "y"=203.43560386351703, "position"=-118.77634453529713, "velocity"=-7.819255113672109, "acceleration"=59.86883732950741, "jerk"=4.520533018173012, "heading"=-5.241717174931665}, {"dt"=0.005, "x"=107.64146393933397, "y"=203.40314705870884, "position"=-118.8139426953349, "velocity"=-7.519632007554895, "acceleration"=59.92462122344282, "jerk"=11.156778787082544, "heading"=-5.241286866997227}, {"dt"=0.005, "x"=107.65967313872143, "y"=203.37197549618193, "position"=-118.8500431281952, "velocity"=-7.220086572060029, "acceleration"=59.909087098973224, "jerk"=-3.1068248939192245, "heading"=-5.240874119370667}, {"dt"=0.005, "x"=107.67711398355773, "y"=203.3420915352213, "position"=-118.8846442003072, "velocity"=-6.920214422401943, "acceleration"=59.974429931617124, "jerk"=13.068566528779968, "heading"=-5.240478899207243}, {"dt"=0.005, "x"=107.6937880542608, "y"=203.31349602055923, "position"=-118.91774598413527, "velocity"=-6.620356765613004, "acceleration"=59.97153135778781, "jerk"=-0.5797147658626045, "heading"=-5.240101156356424}, {"dt"=0.005, "x"=107.70969648428945, "y"=203.28619040474683, "position"=-118.94934780055253, "velocity"=-6.320363283452668, "acceleration"=59.998696432067256, "jerk"=5.433014855888985, "heading"=-5.239740851451684}, {"dt"=0.005, "x"=107.72484035905899, "y"=203.26017606591407, "position"=-118.97944900929805, "velocity"=-6.020241749103883, "acceleration"=60.02430686975693, "jerk"=5.122087537934306, "heading"=-5.239397946863345}, {"dt"=0.005, "x"=107.73922074649917, "y"=203.235454255529, "position"=-119.00804906964144, "velocity"=-5.7200120686773435, "acceleration"=60.04593608530797, "jerk"=4.3258431102088934, "heading"=-5.239072406003404}, {"dt"=0.005, "x"=107.75283869701983, "y"=203.21202609857113, "position"=-119.03514754035153, "velocity"=-5.419694142016637, "acceleration"=60.06358533214122, "jerk"=3.5298493666502395, "heading"=-5.238764193323682}, {"dt"=0.005, "x"=107.76569524348089, "y"=203.1898925937163, "position"=-119.06074407965012, "velocity"=-5.119307859716749, "acceleration"=60.07725645997759, "jerk"=2.7342255672735405, "heading"=-5.238473274313909}, {"dt"=0.005, "x"=107.77779121415188, "y"=203.16905493580512, "position"=-119.08483807254663, "velocity"=-4.818798579301537, "acceleration"=60.10185608304255, "jerk"=4.919924612991622, "heading"=-5.238199619730278}, {"dt"=0.005, "x"=107.78912742124479, "y"=203.14951419188827, "position"=-119.10742900577387, "velocity"=-4.518186645446236, "acceleration"=60.12238677106012, "jerk"=4.106137603514526, "heading"=-5.237943201324963}, {"dt"=0.005, "x"=107.79970484673821, "y"=203.13127098069913, "position"=-119.12851683839271, "velocity"=-4.217566523770043, "acceleration"=60.1240243352386, "jerk"=0.3275128356960977, "heading"=-5.23770398764198}, {"dt"=0.005, "x"=107.80952415572223, "y"=203.11432631192164, "position"=-119.14810103173588, "velocity"=-3.916838668632155, "acceleration"=60.145571027577645, "jerk"=4.309338467808743, "heading"=-5.237481955021797}, {"dt"=0.005, "x"=107.81858592844938, "y"=203.09868118691074, "position"=-119.16618101131455, "velocity"=-3.6159959157355313, "acceleration"=60.16855057932471, "jerk"=4.595910349412691, "heading"=-5.237277082348053}, {"dt"=0.005, "x"=107.826890984201, "y"=203.08433603946176, "position"=-119.18275681314645, "velocity"=-3.315160366380119, "acceleration"=60.16710987108249, "jerk"=-0.28814164844419565, "heading"=-5.237089343724299}, {"dt"=0.005, "x"=107.83443987397382, "y"=203.07129161176348, "position"=-119.19782807158023, "velocity"=-3.014251686755699, "acceleration"=60.18173592488392, "jerk"=2.925210760285779, "heading"=-5.236918719941918}, {"dt"=0.005, "x"=107.84123313122127, "y"=203.05954852185963, "position"=-119.211394519329, "velocity"=-2.7132895497545735, "acceleration"=60.19242740022514, "jerk"=2.1382950682450996, "heading"=-5.236765192808557}, {"dt"=0.005, "x"=107.84727127183724, "y"=203.04910726373694, "position"=-119.22345598745203, "velocity"=-2.4122936246047426, "acceleration"=60.19918502996617, "jerk"=1.3515259482062447, "heading"=-5.23662874514713}, {"dt"=0.005, "x"=107.85256696857485, "y"=203.0399471460634, "position"=-119.23403673221455, "velocity"=-2.1161489525041697, "acceleration"=59.228934420114584, "jerk"=-194.05012197031795, "heading"=-5.236509085717763}, {"dt"=0.005, "x"=107.85715789776785, "y"=203.03200403755156, "position"=-119.24321113157833, "velocity"=-1.834879872756916, "acceleration"=56.25381594945073, "jerk"=-595.0236941327702, "heading"=-5.2364053590698845}, {"dt"=0.005, "x"=107.86109493036061, "y"=203.02519076934627, "position"=-119.25108011177107, "velocity"=-1.5737960385474414, "acceleration"=52.21676684189491, "jerk"=-807.4098215111646, "heading"=-5.236316412467169}, {"dt"=0.005, "x"=107.8644280698076, "y"=203.01942148037344, "position"=-119.25774303258893, "velocity"=-1.3325841635725688, "acceleration"=48.242374994974526, "jerk"=-794.8783693840767, "heading"=-5.236241113541984}, {"dt"=0.005, "x"=107.86720816948622, "y"=203.01460867376713, "position"=-119.26330109534972, "velocity"=-1.1116125521563192, "acceleration"=44.19432228324993, "jerk"=-809.6105423449188, "heading"=-5.2361783113812415}, {"dt"=0.005, "x"=107.86948529293812, "y"=203.01066608123165, "position"=-119.26785404243002, "velocity"=-0.9105894160605831, "acceleration"=40.20462721914721, "jerk"=-797.9390128205438, "heading"=-5.236126873465969}, {"dt"=0.005, "x"=107.87130980640848, "y"=203.00750679592295, "position"=-119.27150232052595, "velocity"=-0.729655619186313, "acceleration"=36.186759374854006, "jerk"=-803.5735688586414, "heading"=-5.2360856608943855}, {"dt"=0.005, "x"=107.87273210198688, "y"=203.0050437732632, "position"=-119.27434650851812, "velocity"=-0.5688375984345158, "acceleration"=32.16360415035946, "jerk"=-804.631044898909, "heading"=-5.236053534550423}, {"dt"=0.005, "x"=107.87380240464388, "y"=203.0031901845223, "position"=-119.27648691478748, "velocity"=-0.42808125387206913, "acceleration"=28.151268912489325, "jerk"=-802.4670475740272, "heading"=-5.236029359385066}, {"dt"=0.005, "x"=107.87457093290513, "y"=203.00185915573317, "position"=-119.27802388366351, "velocity"=-0.30739377520380673, "acceleration"=24.13749573365248, "jerk"=-802.7546357673692, "heading"=-5.236012000718892}, {"dt"=0.005, "x"=107.87508790054409, "y"=203.00096377957746, "position"=-119.27905778597994, "velocity"=-0.2067804632885725, "acceleration"=20.122662383046848, "jerk"=-802.9666701211262, "heading"=-5.23600032414495}, {"dt"=0.005, "x"=107.87540351801557, "y"=203.00041712544797, "position"=-119.27968901107894, "velocity"=-0.12624501979874622, "acceleration"=16.107088697965256, "jerk"=-803.1147370163183, "heading"=-5.235993195446554}, {"dt"=0.005, "x"=107.87556799362923, "y"=203.0001322476851, "position"=-119.2800179602654, "velocity"=-0.06578983729172543, "acceleration"=12.09103650140416, "jerk"=-803.2104393122193, "heading"=-5.235989480529987}, {"dt"=0.005, "x"=107.8756315344632, "y"=203.00002219198825, "position"=-119.28014504171168, "velocity"=-0.02541628925470979, "acceleration"=8.074709607403127, "jerk"=-803.2653788002065, "heading"=-5.235988045372129}, {"dt"=0.005, "x"=107.87564434701756, "y"=203.0000000000005, "position"=-119.280170666814, "velocity"=-0.005125020464460322, "acceleration"=4.058253758049894, "jerk"=-803.2911698706467, "heading"=-5.235987755982995}, {"dt"=0.005, "x"=107.87564434701756, "y"=203.0000000000005, "position"=-119.280170666814, "velocity"=-0.0, "acceleration"=1.0250040928920643, "jerk"=-606.6499330315659, "heading"=-5.235987755982995}]
  out "right":T1[](array[typedef])=[{"dt"=0.005, "x"=0.0008758536007823281, "y"=259.9999999726029, "position"=-5.8139534883720933e-05, "velocity"=-0.023255813953488372, "acceleration"=-4.651162790697675, "jerk"=-930.232558139535, "heading"=-6.283122746208061}, {"dt"=0.005, "x"=0.0008602070905170062, "y"=259.999999973573, "position"=-7.378604517911578e-05, "velocity"=-0.00312930205907897, "acceleration"=4.02530237888188, "jerk"=1735.2930339159109, "heading"=-6.2831238638159395}, {"dt"=0.005, "x"=0.00082500305296863, "y"=259.99999997569176, "position"=-0.00010899008279125226, "velocity"=-0.0070408075224272955, "acceleration"=-0.7823010926696652, "jerk"=-961.520694310309, "heading"=-6.283126378390055}, {"dt"=0.005, "x"=0.0007624201846368434, "y"=259.9999999792398, "position"=-0.00017157295122361484, "velocity"=-0.012516573686472514, "acceleration"=-1.0951532328090436, "jerk"=-62.57042802787569, "heading"=-6.283130848594943}, {"dt"=0.005, "x"=0.0006646398015586345, "y"=259.99999998422334, "position"=-0.00026935333442881993, "velocity"=-0.019556076641041014, "acceleration"=-1.4079005909137, "jerk"=-62.54947162093125, "heading"=-6.283137832908029}, {"dt"=0.005, "x"=0.0005238475090722906, "y"=259.9999999901994, "position"=-0.00041014562704199363, "velocity"=-0.02815845852263474, "acceleration"=-1.7204763763187447, "jerk"=-62.515157081008965, "heading"=-6.283147889500358}, {"dt"=0.005, "x"=0.00033223528885417756, "y"=259.99999999605785, "position"=-0.0006017578473496664, "velocity"=-0.03832244406153456, "acceleration"=-2.032797107779964, "jerk"=-62.46414629224386, "heading"=-6.283161576087523}, {"dt"=0.005, "x"=8.200400317489167e-05, "y"=259.99999999975984, "position"=-0.0008519891330563364, "velocity"=-0.05004625714133398, "acceleration"=-2.3447626159598847, "jerk"=-62.393101635984124, "heading"=-6.283179449750788}, {"dt"=0.005, "x"=0.0032551118628516866, "y"=260.0000000272776, "position"=-0.004025096992852451, "velocity"=-0.6346215719592229, "acceleration"=-116.91506296357778, "jerk"=-22914.06006952358, "heading"=-1.6759390957965525e-05}, {"dt"=0.005, "x"=0.008678251549237957, "y"=260.00000019386385, "position"=-0.009448236681797293, "velocity"=-1.0846279377889683, "acceleration"=-90.00127316594907, "jerk"=5382.757959525742, "heading"=-4.4674576916869935e-05}, {"dt"=0.005, "x"=0.015240397915818266, "y"=260.00000059782394, "position"=-0.016010383060811317, "velocity"=-1.3124292758028053, "acceleration"=-45.56026760276741, "jerk"=8888.201112636332, "heading"=-7.844169176274285e-05}, {"dt"=0.005, "x"=0.023050107374152237, "y"=260.0000013673039, "position"=-0.023820092557053193, "velocity"=-1.5619418992483751, "acceleration"=-49.90252468911396, "jerk"=-868.4514172693099, "heading"=-0.00011861272284025004}, {"dt"=0.005, "x"=0.03221592663276095, "y"=260.00000267047295, "position"=-0.03298591190830226, "velocity"=-1.833163870249813, "acceleration"=-54.24439420028757, "jerk"=-868.3739022347226, "heading"=-0.00016573742479814024}, {"dt"=0.005, "x"=0.04284650760223722, "y"=260.0000047227397, "position"=-0.04361649307587677, "velocity"=-2.1261162335149013, "acceleration"=-58.59047265301766, "jerk"=-869.215690546018, "heading"=-0.00022036351598547776}, {"dt"=0.005, "x"=0.055050492552332575, "y"=260.0000077945201, "position"=-0.0558204784125604, "velocity"=-2.4407970673367263, "acceleration"=-62.936166764365, "jerk"=-869.1388222694669, "heading"=-0.0002830356608759521}, {"dt"=0.005, "x"=0.06888233584768995, "y"=260.0000122003889, "position"=-0.06965232240962031, "velocity"=-2.766368799411982, "acceleration"=-65.11434641505112, "jerk"=-435.6359301372237, "heading"=-0.00035401708800802956}, {"dt"=0.005, "x"=0.08434229622499637, "y"=260.0000182863454, "position"=-0.08511228398482323, "velocity"=-3.091992315040585, "acceleration"=-65.12470312572063, "jerk"=-2.0713421339024762, "heading"=-0.0004332902398125893}, {"dt"=0.005, "x"=0.10143060205716764, "y"=260.0000264386558, "position"=-0.10220059176160395, "velocity"=-3.417661555356143, "acceleration"=-65.13384806311161, "jerk"=-1.8289874781970639, "heading"=-0.0005208351885473417}, {"dt"=0.005, "x"=0.12014761478101707, "y"=260.0000370837894, "position"=-0.12091760751261538, "velocity"=-3.743403150202286, "acceleration"=-65.14831896922857, "jerk"=-2.8941812233910014, "heading"=-0.000616630476134028}, {"dt"=0.005, "x"=0.14049361932187313, "y"=260.0000506881656, "position"=-0.14126361660176076, "velocity"=-4.069201817829078, "acceleration"=-65.15973352535838, "jerk"=-2.2829112259614703, "heading"=-0.0007206520430999008}, {"dt"=0.005, "x"=0.16246901816644194, "y"=260.00006775809567, "position"=-0.16323902207607202, "velocity"=-4.395081094862253, "acceleration"=-65.17585540663511, "jerk"=-3.2243762553463284, "heading"=-0.0008328742248462917}, {"dt"=0.005, "x"=0.18607418328619355, "y"=260.00008883951, "position"=-0.18684419660956716, "velocity"=-4.721034906699031, "acceleration"=-65.1907623673555, "jerk"=-2.981392144079109, "heading"=-0.0009532689972410191}, {"dt"=0.005, "x"=0.21130952747206622, "y"=260.00011451780574, "position"=-0.21207955385994762, "velocity"=-5.047071450076093, "acceleration"=-65.20730867541235, "jerk"=-3.309261611369152, "heading"=-0.001081806344908287}, {"dt"=0.005, "x"=0.2381755042243468, "y"=260.0001454176438, "position"=-0.23894554838190926, "velocity"=-5.373198904392329, "acceleration"=-65.22549086324733, "jerk"=-3.6364375669961646, "heading"=-0.0012184542638269957}, {"dt"=0.005, "x"=0.2666726076360209, "y"=260.00018220273313, "position"=-0.26744267553533374, "velocity"=-5.699425430684901, "acceleration"=-65.24530525851428, "jerk"=-3.9628790533896563, "heading"=-0.0013631787640525084}, {"dt"=0.005, "x"=0.2968013019217378, "y"=260.000225575495, "position"=-0.29757140104038393, "velocity"=-6.025745101010039, "acceleration"=-65.26393406502766, "jerk"=-3.7257613026753233, "heading"=-0.0015159435161616885}, {"dt"=0.005, "x"=0.3285621660993529, "y"=260.00027627700746, "position"=-0.3293323056866984, "velocity"=-6.352180929262892, "acceleration"=-65.2871656505706, "jerk"=-4.64631710858896, "heading"=-0.0016767105896903223}, {"dt"=0.005, "x"=0.3619557056183644, "y"=260.00033508645987, "position"=-0.36272589699041224, "velocity"=-6.678718260742772, "acceleration"=-65.30746629597601, "jerk"=-4.060129081082664, "heading"=-0.0018454395028453252}, {"dt"=0.005, "x"=0.396982555247428, "y"=260.00040282119545, "position"=-0.3977528121119504, "velocity"=-7.005383024307628, "acceleration"=-65.33295271297116, "jerk"=-5.0972833990300614, "heading"=-0.0020220882541658325}, {"dt"=0.005, "x"=0.43364331961633074, "y"=260.0004803361516, "position"=-0.43441365842897695, "velocity"=-7.332169263405308, "acceleration"=-65.35724781953593, "jerk"=-4.859021312952905, "heading"=-0.002206612520756379}, {"dt"=0.005, "x"=0.47193864340303326, "y"=260.00056852366566, "position"=-0.4727090837558488, "velocity"=-7.659085065374374, "acceleration"=-65.38316039381317, "jerk"=-5.182514855448517, "heading"=-0.0023989660184867145}, {"dt"=0.005, "x"=0.5118692111664584, "y"=260.0006683131599, "position"=-0.5126397762098077, "velocity"=-7.9861384907917845, "acceleration"=-65.41068508348218, "jerk"=-5.504937933801557, "heading"=-0.0025991005059064487}, {"dt"=0.005, "x"=0.5534356798978805, "y"=260.0007806706253, "position"=-0.5542063967965275, "velocity"=-8.313324117343956, "acceleration"=-65.4371253104344, "jerk"=-5.288045390443585, "heading"=-0.0028069654522328014}, {"dt"=0.005, "x"=0.5966388278583057, "y"=260.00090659865856, "position"=-0.5974097282833464, "velocity"=-8.640666297363767, "acceleration"=-65.46843600396208, "jerk"=-6.262138705537268, "heading"=-0.0030225087880748625}, {"dt"=0.005, "x"=0.64147937010289, "y"=260.00104713559546, "position"=-0.6422504907592341, "velocity"=-8.968152495177554, "acceleration"=-65.49723956275741, "jerk"=-5.760711759066339, "heading"=-0.0032456759888707665}, {"dt"=0.005, "x"=0.6879581262855005, "y"=260.00120335561087, "position"=-0.6887295094771004, "velocity"=-9.295803743573256, "acceleration"=-65.53024967914034, "jerk"=-6.602023276585101, "heading"=-0.0034764109186699033}, {"dt"=0.005, "x"=0.7360758881716761, "y"=260.0013763679174, "position"=-0.7368475824039427, "velocity"=-9.623614585368435, "acceleration"=-65.56216835903577, "jerk"=-6.383735979085259, "heading"=-0.003714655176530801}, {"dt"=0.005, "x"=0.7858334867053101, "y"=260.00156731655414, "position"=-0.7866055473263164, "velocity"=-9.951592984474743, "acceleration"=-65.59567982126175, "jerk"=-6.7022924451976, "heading"=-0.0039603484374847175}, {"dt"=0.005, "x"=0.837231791794135, "y"=260.00177737997325, "position"=-0.8380042816749749, "velocity"=-10.27974686973171, "acceleration"=-65.63077705139335, "jerk"=-7.019446026319542, "heading"=-0.004213428457558621}, {"dt"=0.005, "x"=0.8902717120890209, "y"=260.0020077706125, "position"=-0.8910447023438809, "velocity"=-10.60808413378121, "acceleration"=-65.66745280989998, "jerk"=-7.335151701326481, "heading"=-0.004473831078898705}, {"dt"=0.005, "x"=0.9449541356283241, "y"=260.00225973417525, "position"=-0.9457277063740975, "velocity"=-10.93660080604332, "acceleration"=-65.70333445242191, "jerk"=-7.176328504385765, "heading"=-0.004741489946012034}, {"dt"=0.005, "x"=1.001280033273037, "y"=260.00253454961495, "position"=-1.0020542744304648, "velocity"=-11.265313611273436, "acceleration"=-65.74256104602334, "jerk"=-7.845318720285377, "heading"=-0.005016337020701256}, {"dt"=0.005, "x"=1.059250342416668, "y"=260.00283352811203, "position"=-1.060025354551072, "velocity"=-11.594216024121453, "acceleration"=-65.7804825696033, "jerk"=-7.584304715990697, "heading"=-0.005298302020654566}, {"dt"=0.005, "x"=1.1188660950444342, "y"=260.00315801320545, "position"=-1.1196419902490957, "velocity"=-11.92332713960474, "acceleration"=-65.8222230966576, "jerk"=-8.348105410860285, "heading"=-0.005587313051794995}, {"dt"=0.005, "x"=1.1801283021468916, "y"=260.0035093796981, "position"=-1.1809052049662203, "velocity"=-12.25264294342492, "acceleration"=-65.86316076403591, "jerk"=-8.187533475663145, "heading"=-0.0058832960532334555}, {"dt"=0.005, "x"=1.2430380125912346, "y"=260.0038890334238, "position"=-1.2438160609860085, "velocity"=-12.582171203957637, "acceleration"=-65.9056521065434, "jerk"=-8.498268501497819, "heading"=-0.006186175092258439}, {"dt"=0.005, "x"=1.3075963128578838, "y"=260.0042984107209, "position"=-1.3083756592119131, "velocity"=-12.91191964518092, "acceleration"=-65.94968824465646, "jerk"=-8.807227622611435, "heading"=-0.0064958723704272026}, {"dt"=0.005, "x"=1.3738042811226185, "y"=260.004738977581, "position"=-1.3745850932897117, "velocity"=-13.241886815559702, "acceleration"=-65.9934340757566, "jerk"=-8.74916622002786, "heading"=-0.006812308011973578}, {"dt"=0.005, "x"=1.4416630542433122, "y"=260.00521222950124, "position"=-1.4424455166366508, "velocity"=-13.572084669387827, "acceleration"=-66.03957076562494, "jerk"=-9.227337973669592, "heading"=-0.007135400393883662}, {"dt"=0.005, "x"=1.5111737862938894, "y"=260.005719690642, "position"=-1.5119581010154275, "velocity"=-13.90251687575534, "acceleration"=-66.08644127350267, "jerk"=-9.374101575545524, "heading"=-0.007465065955438832}, {"dt"=0.005, "x"=1.5823376700049316, "y"=260.00626291338097, "position"=-1.583124058015828, "velocity"=-14.233191400080083, "acceleration"=-66.1349048649484, "jerk"=-9.692718289144864, "heading"=-0.007801219309015173}, {"dt"=0.005, "x"=1.655155889416376, "y"=260.0068434773351, "position"=-1.6559445917460753, "velocity"=-14.564106746049493, "acceleration"=-66.1830691938821, "jerk"=-9.632865786741718, "heading"=-0.008143773025622747}, {"dt"=0.005, "x"=1.7296296652309573, "y"=260.00746298905926, "position"=-1.7304209442269594, "velocity"=-14.895270496176794, "acceleration"=-66.23275002546016, "jerk"=-9.936166315611672, "heading"=-0.008492637859500662}, {"dt"=0.005, "x"=1.8057602545134952, "y"=260.0081230814189, "position"=-1.8065543951301577, "velocity"=-15.226690180639665, "acceleration"=-66.28393689257415, "jerk"=-10.237373422796736, "heading"=-0.008847722755006282}, {"dt"=0.005, "x"=1.883548950384645, "y"=260.00882541294976, "position"=-1.8843462615103488, "velocity"=-15.558373276038207, "acceleration"=-66.33661907970847, "jerk"=-10.536437426864609, "heading"=-0.009208934853559114}, {"dt"=0.005, "x"=1.9629970618054824, "y"=260.0095716670126, "position"=-1.963797877626474, "velocity"=-15.890323223225023, "acceleration"=-66.38998943736318, "jerk"=-10.674071530942797, "heading"=-0.009576179408844698}, {"dt"=0.005, "x"=2.0441058668868397, "y"=260.0103635506265, "position"=-2.0449105482851544, "velocity"=-16.222534131736083, "acceleration"=-66.44218170221201, "jerk"=-10.438452969765422, "heading"=-0.009949359583154571}, {"dt"=0.005, "x"=2.126876759643103, "y"=260.01120279517863, "position"=-2.127685695636803, "velocity"=-16.55502947032969, "acceleration"=-66.49906771872125, "jerk"=-11.377203301847771, "heading"=-0.010328377133728417}, {"dt"=0.005, "x"=2.211311109285237, "y"=260.01209115437445, "position"=-2.212124718496799, "velocity"=-16.88780457199924, "acceleration"=-66.55502033391016, "jerk"=-11.190523037782896, "heading"=-0.010713131773046225}, {"dt"=0.005, "x"=2.2974103004940085, "y"=260.0130304038617, "position"=-2.2982290326535466, "velocity"=-17.220862831349535, "acceleration"=-66.61165187005906, "jerk"=-11.326307229779786, "heading"=-0.011103521366487179}, {"dt"=0.005, "x"=2.3851757529920103, "y"=260.0140223406932, "position"=-2.3860000904736314, "velocity"=-17.554211564016992, "acceleration"=-66.66974653349129, "jerk"=-11.61893268644576, "heading"=-0.01149944203158998}, {"dt"=0.005, "x"=2.4746089212069045, "y"=260.0150687825857, "position"=-2.47543938059597, "velocity"=-17.88785802446773, "acceleration"=-66.7292920901474, "jerk"=-11.909111331220856, "heading"=-0.011900788145544128}, {"dt"=0.005, "x"=2.5657112939295623, "y"=260.01617156716406, "position"=-2.5665484276194377, "velocity"=-18.221809404693506, "acceleration"=-66.7902760451554, "jerk"=-12.19679100159965, "heading"=-0.012307452352702253}, {"dt"=0.005, "x"=2.6584843008669403, "y"=260.01733255000755, "position"=-2.659328698676197, "velocity"=-18.556054211351785, "acceleration"=-66.84896133165594, "jerk"=-11.737057300109655, "heading"=-0.012719325159919415}, {"dt"=0.005, "x"=2.75292953404585, "y"=260.0185536065845, "position"=-2.753781824878471, "velocity"=-18.890625240454803, "acceleration"=-66.91420582060346, "jerk"=-13.04889778950269, "heading"=-0.013136295931937603}, {"dt"=0.005, "x"=2.8490484673755314, "y"=260.0198366279234, "position"=-2.8499093208834734, "velocity"=-19.225499201000524, "acceleration"=-66.97479210914423, "jerk"=-12.117257708155194, "heading"=-0.013558251657072029}, {"dt"=0.005, "x"=2.9468426867414497, "y"=260.02118352270196, "position"=-2.9477128150282836, "velocity"=-19.56069882896202, "acceleration"=-67.03992559229945, "jerk"=-13.026696631044388, "heading"=-0.013985077976886029}, {"dt"=0.005, "x"=3.046313782361921, "y"=260.0225962150383, "position"=-3.047193941698492, "velocity"=-19.896225334041684, "acceleration"=-67.10530101593264, "jerk"=-13.075084726636987, "heading"=-0.014416658719868247}, {"dt"=0.005, "x"=3.147463361876133, "y"=260.0240766437856, "position"=-3.1483543544357766, "velocity"=-20.232082547456898, "acceleration"=-67.17144268304267, "jerk"=-13.228333422006244, "heading"=-0.014852875970709278}, {"dt"=0.005, "x"=3.2502930166583095, "y"=260.02562676113115, "position"=-3.2511956922645244, "velocity"=-20.568267565749533, "acceleration"=-67.23700365852707, "jerk"=-13.112195096880441, "heading"=-0.015293609937738706}, {"dt"=0.005, "x"=3.3548044300756343, "y"=260.02724853332484, "position"=-3.355719687976204, "velocity"=-20.904799142335907, "acceleration"=-67.30631531727482, "jerk"=-13.862331749550094, "heading"=-0.015738739428503346}, {"dt"=0.005, "x"=3.460999274291608, "y"=260.0289439382591, "position"=-3.461928064933702, "velocity"=-21.241675391499573, "acceleration"=-67.37524983273318, "jerk"=-13.78690309167041, "heading"=-0.016188141415762913}, {"dt"=0.005, "x"=3.568879237050449, "y"=260.0307149649226, "position"=-3.5698225638680396, "velocity"=-21.578899786867538, "acceleration"=-67.444879073593, "jerk"=-13.925848171965072, "heading"=-0.01664169116497438}, {"dt"=0.005, "x"=3.678446007125939, "y"=260.03256361220355, "position"=-3.679404928332148, "velocity"=-21.916472892821677, "acceleration"=-67.51462119082774, "jerk"=-13.9484234469478, "heading"=-0.01709926218535751}, {"dt"=0.005, "x"=3.78970135182788, "y"=260.0344918892551, "position"=-3.7906769822232094, "velocity"=-22.254410778212264, "acceleration"=-67.58757707811753, "jerk"=-14.591177457958793, "heading"=-0.017560726563973728}, {"dt"=0.005, "x"=3.902647024597757, "y"=260.0365018129988, "position"=-3.9036405373677585, "velocity"=-22.592711028909797, "acceleration"=-67.66005013950647, "jerk"=-14.4946122777867, "heading"=-0.018025954589003357}, {"dt"=0.005, "x"=4.01728481056159, "y"=260.03859540790864, "position"=-4.018297439080373, "velocity"=-22.931380342522996, "acceleration"=-67.73386272263977, "jerk"=-14.762516626660727, "heading"=-0.01849481495111488}, {"dt"=0.005, "x"=4.133616459186402, "y"=260.0407747037669, "position"=-4.134649498805177, "velocity"=-23.270411944960774, "acceleration"=-67.80632048755564, "jerk"=-14.491552983173506, "heading"=-0.018967174480118587}, {"dt"=0.005, "x"=4.251643856354486, "y"=260.0430417378688, "position"=-4.252698666213897, "velocity"=-23.609833481743895, "acceleration"=-67.88430735662416, "jerk"=-15.597373813704962, "heading"=-0.019442898855028645}, {"dt"=0.005, "x"=4.371368799526998, "y"=260.0453985497973, "position"=-4.372446804321041, "velocity"=-23.94962762142881, "acceleration"=-67.95882793698311, "jerk"=-14.904116071789986, "heading"=-0.019921851701201476}, {"dt"=0.005, "x"=4.492793186256888, "y"=260.0478471839735, "position"=-4.493895878018861, "velocity"=-24.289814739564108, "acceleration"=-68.03742362705947, "jerk"=-15.719138015271028, "heading"=-0.02040389536281534}, {"dt"=0.005, "x"=4.615918878434284, "y"=260.05038968596153, "position"=-4.617047818281783, "velocity"=-24.630388052584266, "acceleration"=-68.11466260403165, "jerk"=-15.447795394436525, "heading"=-0.020888890368426838}, {"dt"=0.005, "x"=4.74074776886485, "y"=260.0530281026915, "position"=-4.741904588738843, "velocity"=-24.971354091412064, "acceleration"=-68.19320776555955, "jerk"=-15.70903230557974, "heading"=-0.021376695709081128}, {"dt"=0.005, "x"=4.867281780884391, "y"=260.05576448139686, "position"=-4.868468185267153, "velocity"=-25.31271930566186, "acceleration"=-68.27304284995961, "jerk"=-15.967016880011897, "heading"=-0.021867168845404295}, {"dt"=0.005, "x"=4.995522867970051, "y"=260.0586008685369, "position"=-4.996740635578668, "velocity"=-25.65449006230298, "acceleration"=-68.35415132822362, "jerk"=-16.221695652802737, "heading"=-0.02236016571457}, {"dt"=0.005, "x"=5.125473013348254, "y"=260.0615393087038, "position"=-5.126723998800391, "velocity"=-25.99667264434457, "acceleration"=-68.43651640831823, "jerk"=-16.473016018920816, "heading"=-0.022855540737134694}, {"dt"=0.005, "x"=5.257134163151461, "y"=260.06458184196185, "position"=-5.2584202985818544, "velocity"=-26.339259956292608, "acceleration"=-68.51746238960743, "jerk"=-16.189196257840877, "heading"=-0.02335314657368609}, {"dt"=0.005, "x"=5.390508366748472, "y"=260.0677305059157, "position"=-5.39183166342695, "velocity"=-26.682272969019028, "acceleration"=-68.60260254528399, "jerk"=-17.02803113531104, "heading"=-0.023852834667305756}, {"dt"=0.005, "x"=5.525597580691242, "y"=260.07098732998946, "position"=-5.526960130548882, "velocity"=-27.025693424386414, "acceleration"=-68.6840910734773, "jerk"=-16.29770563866373, "heading"=-0.02435445451454049}, {"dt"=0.005, "x"=5.662403896723788, "y"=260.0743543396459, "position"=-5.663807873900474, "velocity"=-27.369548670318423, "acceleration"=-68.77104918640171, "jerk"=-17.39162258488136, "heading"=-0.024857854528733958}, {"dt"=0.005, "x"=5.800929371042386, "y"=260.0778335511623, "position"=-5.802377033340693, "velocity"=-27.7138318880437, "acceleration"=-68.85664354505536, "jerk"=-17.118871730730234, "heading"=-0.025362881410148364}, {"dt"=0.005, "x"=5.941176088718928, "y"=260.08142697196166, "position"=-5.942669779026579, "velocity"=-28.058549137177252, "acceleration"=-68.94344982671043, "jerk"=-17.361256331014374, "heading"=-0.025869380395809882}, {"dt"=0.005, "x"=6.083146119830054, "y"=260.0851365982659, "position"=-6.084688267474425, "velocity"=-28.40369768956919, "acceleration"=-69.02971047838733, "jerk"=-17.25213033537898, "heading"=-0.026377195110501683}, {"dt"=0.005, "x"=6.226841614162525, "y"=260.0889644163277, "position"=-6.228434736239984, "velocity"=-28.749293753111743, "acceleration"=-69.11921270851096, "jerk"=-17.900446024725625, "heading"=-0.02688616791512355}, {"dt"=0.005, "x"=6.372264711260202, "y"=260.0929123988766, "position"=-6.373911413874877, "velocity"=-29.09533552697876, "acceleration"=-69.20835477340361, "jerk"=-17.828412978531105, "heading"=-0.02739613959058068}, {"dt"=0.005, "x"=6.519417572401147, "y"=260.0969825046785, "position"=-6.5211205518494095, "velocity"=-29.44182759490653, "acceleration"=-69.29841358555393, "jerk"=-18.011762430063527, "heading"=-0.027906949461475872}, {"dt"=0.005, "x"=6.668302344714063, "y"=260.10117667624917, "position"=-6.670064388586057, "velocity"=-29.78876734732943, "acceleration"=-69.38795048457962, "jerk"=-17.90737980513768, "heading"=-0.02841843528086402}, {"dt"=0.005, "x"=6.8189212581753775, "y"=260.10549684128756, "position"=-6.820745246422166, "velocity"=-30.136171567221897, "acceleration"=-69.48084397849357, "jerk"=-18.578698782789616, "heading"=-0.02893043357182906}, {"dt"=0.005, "x"=6.971276526867872, "y"=260.10994490862754, "position"=-6.973165432753974, "velocity"=-30.484037266361586, "acceleration"=-69.57313982793778, "jerk"=-18.459169888842553, "heading"=-0.029442779292969234}, {"dt"=0.005, "x"=7.1253703860902595, "y"=260.11452276794125, "position"=-7.127327277079816, "velocity"=-30.832368865168473, "acceleration"=-69.66631976137734, "jerk"=-18.635986687911554, "heading"=-0.02995530597451057}, {"dt"=0.005, "x"=7.281205059222914, "y"=260.11923228740045, "position"=-7.283233097766209, "velocity"=-31.181164137278582, "acceleration"=-69.7590544220219, "jerk"=-18.54693212891334, "heading"=-0.030467845616262257}, {"dt"=0.005, "x"=7.438782876073455, "y"=260.12407531591464, "position"=-7.440885320359397, "velocity"=-31.530444518637605, "acceleration"=-69.85607627180457, "jerk"=-19.40436995653272, "heading"=-0.030980229082420263}, {"dt"=0.005, "x"=7.598106080190919, "y"=260.1290536759196, "position"=-7.600286284718443, "velocity"=-31.88019287180921, "acceleration"=-69.94967063432114, "jerk"=-18.718872503313833, "heading"=-0.03149228547556426}, {"dt"=0.005, "x"=7.759177025414545, "y"=260.13416916801884, "position"=-7.761438441559889, "velocity"=-32.23043136828919, "acceleration"=-70.04769929599561, "jerk"=-19.605732334895265, "heading"=-0.03200384278277996}, {"dt"=0.005, "x"=7.921998026602283, "y"=260.13942356496494, "position"=-7.92434420301431, "velocity"=-32.581152290884106, "acceleration"=-70.14418451898337, "jerk"=-19.29704459755044, "heading"=-0.03251472739815203}, {"dt"=0.005, "x"=8.086571426930659, "y"=260.1448186123214, "position"=-8.089006009853728, "velocity"=-32.93236136788376, "acceleration"=-70.24181539993037, "jerk"=-19.526176189401667, "heading"=-0.033024764346155366}, {"dt"=0.005, "x"=8.252899597539573, "y"=260.15035602704546, "position"=-8.255426331028561, "velocity"=-33.284064234966436, "acceleration"=-70.34057341653579, "jerk"=-19.751603321083167, "heading"=-0.033533777283453525}, {"dt"=0.005, "x"=8.420984937175708, "y"=260.15603749605367, "position"=-8.423607663199187, "velocity"=-33.63626643412513, "acceleration"=-70.44043983173935, "jerk"=-19.973283040712886, "heading"=-0.034041588500349274}, {"dt"=0.005, "x"=8.590829871834611, "y"=260.1618646747692, "position"=-8.593552530262214, "velocity"=-33.988973412605354, "acceleration"=-70.54139569604416, "jerk"=-20.191172860961615, "heading"=-0.03454801892188025}, {"dt"=0.005, "x"=8.762436794535287, "y"=260.1678391835527, "position"=-8.765263422968529, "velocity"=-34.342178541262946, "acceleration"=-70.64102573151843, "jerk"=-19.926007094852594, "heading"=-0.03505288793361572}, {"dt"=0.005, "x"=8.935808199410692, "y"=260.1739626108457, "position"=-8.93874293296981, "velocity"=-34.69590200025618, "acceleration"=-70.74469179864735, "jerk"=-20.73321342578538, "heading"=-0.03555601378151152}, {"dt"=0.005, "x"=9.110946501237546, "y"=260.1802365053553, "position"=-9.11399357211019, "velocity"=-35.05012782807604, "acceleration"=-70.84516556397205, "jerk"=-20.094753064938686, "heading"=-0.036057213045198655}, {"dt"=0.005, "x"=9.287854223732928, "y"=260.1866623811653, "position"=-9.291017960708, "velocity"=-35.40487771956228, "acceleration"=-70.94997829724718, "jerk"=-20.962546655027836, "heading"=-0.0365563011874076}, {"dt"=0.005, "x"=9.466533872638394, "y"=260.19324171171024, "position"=-9.469818700425149, "velocity"=-35.7601479434298, "acceleration"=-71.05404477350419, "jerk"=-20.813295251400632, "heading"=-0.03705309218711178}, {"dt"=0.005, "x"=9.646987978110012, "y"=260.19997592971157, "position"=-9.65039841654424, "velocity"=-36.1159432238181, "acceleration"=-71.15905607765995, "jerk"=-21.002260831153308, "heading"=-0.03754739866352075}, {"dt"=0.005, "x"=9.82921906845559, "y"=260.206866424611, "position"=-9.832759731544153, "velocity"=-36.472262999982526, "acceleration"=-71.26395523288522, "jerk"=-20.979831045053743, "heading"=-0.03803903180539625}, {"dt"=0.005, "x"=10.013229725362212, "y"=260.2139145430488, "position"=-10.016905320219852, "velocity"=-36.82911773513995, "acceleration"=-71.37094703148534, "jerk"=-21.39835972002402, "heading"=-0.03852780152119517}, {"dt"=0.005, "x"=10.199022550756675, "y"=260.22112158603795, "position"=-10.202837876370475, "velocity"=-37.186511230124694, "acceleration"=-71.47869899694825, "jerk"=-21.550393092582, "heading"=-0.03901351634569983}, {"dt"=0.005, "x"=10.386600136407207, "y"=260.2284888061297, "position"=-10.3905600822236, "velocity"=-37.5444411706248, "acceleration"=-71.58598810002132, "jerk"=-21.45782061461432, "heading"=-0.03949598336140597}, {"dt"=0.005, "x"=10.57596510996823, "y"=260.23601740753134, "position"=-10.580074654356805, "velocity"=-37.90291442664106, "acceleration"=-71.69465120325214, "jerk"=-21.732620646162104, "heading"=-0.03997500831889661}, {"dt"=0.005, "x"=10.76712013707558, "y"=260.2437085445594, "position"=-10.77138434563562, "velocity"=-38.261938255763326, "acceleration"=-71.80476582445294, "jerk"=-22.0229242401615, "heading"=-0.04045039563659941}, {"dt"=0.005, "x"=10.960067886879717, "y"=260.2515633185814, "position"=-10.96449191055584, "velocity"=-38.62151298404387, "acceleration"=-71.91494565610839, "jerk"=-22.03596633108873, "heading"=-0.040921948310822076}, {"dt"=0.005, "x"=11.154811056837373, "y"=260.259582777295, "position"=-11.159400129887953, "velocity"=-38.98164386642278, "acceleration"=-72.02617647578222, "jerk"=-22.246163934767083, "heading"=-0.0413894679751019}, {"dt"=0.005, "x"=11.35135234564325, "y"=260.26776791188564, "position"=-11.356111783416008, "velocity"=-39.342330705611154, "acceleration"=-72.13736783767501, "jerk"=-22.238272378558577, "heading"=-0.04185275483144346}, {"dt"=0.005, "x"=11.5496945005979, "y"=260.2761196572408, "position"=-11.554629697173262, "velocity"=-39.703582751450696, "acceleration"=-72.25040916790846, "jerk"=-22.60826604668864, "heading"=-0.042311607758638736}, {"dt"=0.005, "x"=11.749840288802432, "y"=260.28463888901473, "position"=-11.754956714437611, "velocity"=-40.06540345286981, "acceleration"=-72.36414028382256, "jerk"=-22.746223182821268, "heading"=-0.042765824236329686}, {"dt"=0.005, "x"=11.951792491483708, "y"=260.2933264215933, "position"=-11.957095689873134, "velocity"=-40.42779508710461, "acceleration"=-72.47832684696078, "jerk"=-22.83731262764377, "heading"=-0.04321520032698328}, {"dt"=0.005, "x"=12.15555388969597, "y"=260.30218300564644, "position"=-12.161049475036602, "velocity"=-40.790757032693705, "acceleration"=-72.59238911781836, "jerk"=-22.812454171514673, "heading"=-0.04365953064015782}, {"dt"=0.005, "x"=12.36112733378129, "y"=260.31120932931776, "position"=-12.366820987720258, "velocity"=-41.15430253673117, "acceleration"=-72.7091008074936, "jerk"=-23.342337935048363, "heading"=-0.04409860847703356}, {"dt"=0.005, "x"=12.568515672347939, "y"=260.3204060133159, "position"=-12.574413140678882, "velocity"=-41.51843059172466, "acceleration"=-72.82561099869724, "jerk"=-23.30203824072896, "heading"=-0.044532225665005754}, {"dt"=0.005, "x"=12.777721770674273, "y"=260.32977360982, "position"=-12.783828859862497, "velocity"=-41.88314383672319, "acceleration"=-72.9426489997067, "jerk"=-23.407600201892365, "heading"=-0.0449601725916855}, {"dt"=0.005, "x"=12.988748520106649, "y"=260.3393126010029, "position"=-12.99507109363402, "velocity"=-42.24844675430456, "acceleration"=-73.06058351627343, "jerk"=-23.58690331334401, "heading"=-0.045382238215472714}, {"dt"=0.005, "x"=13.201598872292267, "y"=260.3490233986942, "position"=-13.208142846847213, "velocity"=-42.61435064263836, "acceleration"=-73.18077766675941, "jerk"=-24.038830097197206, "heading"=-0.045798210120846394}, {"dt"=0.005, "x"=13.416275729192673, "y"=260.35890633743463, "position"=-13.423047070553459, "velocity"=-42.98084474124913, "acceleration"=-73.29881972215446, "jerk"=-23.60841107901024, "heading"=-0.04620787429158624}, {"dt"=0.005, "x"=13.632782097588398, "y"=260.36896167957417, "position"=-13.639786816473418, "velocity"=-43.34794918399194, "acceleration"=-73.42088854856286, "jerk"=-24.413765281678934, "heading"=-0.04661101540011764}, {"dt"=0.005, "x"=13.851120962080863, "y"=260.3791896074794, "position"=-13.85836510967083, "velocity"=-43.71565863948235, "acceleration"=-73.54189109808118, "jerk"=-24.200509903664624, "heading"=-0.0470074165486688}, {"dt"=0.005, "x"=14.071295338884472, "y"=260.38959022398564, "position"=-14.078785002204528, "velocity"=-44.083978506739584, "acceleration"=-73.6639734514469, "jerk"=-24.41647067314534, "heading"=-0.04739685936065724}, {"dt"=0.005, "x"=14.293308275609283, "y"=260.4001635503703, "position"=-14.301049572714565, "velocity"=-44.45291410200736, "acceleration"=-73.78711905355573, "jerk"=-24.629120421764128, "heading"=-0.04777912396457673}, {"dt"=0.005, "x"=14.517162851042961, "y"=260.41090952429914, "position"=-14.525161926006998, "velocity"=-44.822470658486615, "acceleration"=-73.91131129585062, "jerk"=-24.8384484589792, "heading"=-0.048153988977164996}, {"dt"=0.005, "x"=14.742862174932165, "y"=260.42182799774594, "position"=-14.751125192637776, "velocity"=-45.19265332615563, "acceleration"=-74.03653353380264, "jerk"=-25.04444759040325, "heading"=-0.048521231485842475}, {"dt"=0.005, "x"=14.970409340141991, "y"=260.4329187325542, "position"=-14.978942480817613, "velocity"=-45.56345763596729, "acceleration"=-74.16086196233209, "jerk"=-24.865685705890428, "heading"=-0.048880626956336604}, {"dt"=0.005, "x"=15.19980754079359, "y"=260.4441814040479, "position"=-15.208616994491566, "velocity"=-45.93490273479059, "acceleration"=-74.28901976466022, "jerk"=-25.631560465626535, "heading"=-0.04923194940349945}, {"dt"=0.005, "x"=15.431059941266186, "y"=260.4556155925037, "position"=-15.440151901989292, "velocity"=-46.30698149954524, "acceleration"=-74.41575295092946, "jerk"=-25.346637253846893, "heading"=-0.0495749711637084}, {"dt"=0.005, "x"=15.664169748118129, "y"=260.46722078445606, "position"=-15.673550407834554, "velocity"=-46.67970116905244, "acceleration"=-74.54393390144105, "jerk"=-25.636190102318324, "heading"=-0.049909462990579245}, {"dt"=0.005, "x"=15.899140212664651, "y"=260.47899637063733, "position"=-15.908815755132284, "velocity"=-47.053069459545895, "acceleration"=-74.67365809869051, "jerk"=-25.944839449891788, "heading"=-0.05023519403457111}, {"dt"=0.005, "x"=16.135974601332546, "y"=260.4909416422589, "position"=-16.145951195692756, "velocity"=-47.42708811209419, "acceleration"=-74.8037305096588, "jerk"=-26.014482193659205, "heading"=-0.050551931778636094}, {"dt"=0.005, "x"=16.374676203903718, "y"=260.5030557891356, "position"=-16.384959998092576, "velocity"=-47.801760479963825, "acceleration"=-74.93447357392711, "jerk"=-26.148612853660325, "heading"=-0.05085944202959397}, {"dt"=0.005, "x"=16.61524836844311, "y"=260.5153378991604, "position"=-16.625845482457716, "velocity"=-48.17709687302813, "acceleration"=-75.06727861286038, "jerk"=-26.561007786654045, "heading"=-0.05115748893864153}, {"dt"=0.005, "x"=16.857694443763688, "y"=260.5277869530491, "position"=-16.868610962666654, "velocity"=-48.5530960417874, "acceleration"=-75.19983375185433, "jerk"=-26.51102779879011, "heading"=-0.05144583490291749}, {"dt"=0.005, "x"=17.102017834724208, "y"=260.54040182479287, "position"=-17.113259801534856, "velocity"=-48.92976777364034, "acceleration"=-75.33434637058889, "jerk"=-26.902523746912266, "heading"=-0.051724240609072214}, {"dt"=0.005, "x"=17.348221945110268, "y"=260.5531812763216, "position"=-17.35979535343836, "velocity"=-49.307110380701204, "acceleration"=-75.46852141217215, "jerk"=-26.83500831665242, "heading"=-0.05199246493973941}, {"dt"=0.005, "x"=17.596310248075316, "y"=260.5661239587112, "position"=-17.608221034670226, "velocity"=-49.6851362463729, "acceleration"=-75.60517313433905, "jerk"=-27.33034443338056, "heading"=-0.05225026502561936}, {"dt"=0.005, "x"=17.84628623271667, "y"=260.5792284069587, "position"=-17.858540269770696, "velocity"=-50.06384702009403, "acceleration"=-75.7421547442263, "jerk"=-27.39632197744868, "heading"=-0.052497396156023224}, {"dt"=0.005, "x"=18.09815342268908, "y"=260.5924930384409, "position"=-18.11075650999515, "velocity"=-50.44324804489035, "acceleration"=-75.88020495926457, "jerk"=-27.61004300765535, "heading"=-0.05273361177038338}, {"dt"=0.005, "x"=18.35191536622254, "y"=260.6059161498496, "position"=-18.364873223152248, "velocity"=-50.823342631419784, "acceleration"=-76.01891730588619, "jerk"=-27.742469324323338, "heading"=-0.05295866341853034}, {"dt"=0.005, "x"=18.60757567314709, "y"=260.61949591657765, "position"=-18.62089393052012, "velocity"=-51.20414147357386, "acceleration"=-76.15976843081569, "jerk"=-28.170224985899495, "heading"=-0.053172300761148206}, {"dt"=0.005, "x"=18.865137960378757, "y"=260.63323038722353, "position"=-18.878822152101105, "velocity"=-51.58564431619745, "acceleration"=-76.30056852471796, "jerk"=-28.160018780454266, "heading"=-0.053374271488402514}, {"dt"=0.005, "x"=19.12460590287351, "y"=260.64711748364385, "position"=-19.13866145749859, "velocity"=-51.96786107949678, "acceleration"=-76.44335265986513, "jerk"=-28.556827029433407, "heading"=-0.05356432132894945}, {"dt"=0.005, "x"=19.385983196182984, "y"=260.6611549962701, "position"=-19.400415428277487, "velocity"=-52.350794155779575, "acceleration"=-76.5866152565593, "jerk"=-28.65251933883428, "heading"=-0.053742193984267494}, {"dt"=0.005, "x"=19.649273578824875, "y"=260.67534058257064, "position"=-19.664087680231315, "velocity"=-52.734450390765666, "acceleration"=-76.73124699721825, "jerk"=-28.92634813179029, "heading"=-0.053907631109661125}, {"dt"=0.005, "x"=19.914480830959143, "y"=260.6896717642116, "position"=-19.929681861929325, "velocity"=-53.11883633960177, "acceleration"=-76.87718976722095, "jerk"=-29.18855400054099, "heading"=-0.05406037227421545}, {"dt"=0.005, "x"=20.181608766679226, "y"=260.70414592382605, "position"=-20.19720164687731, "velocity"=-53.50395698959749, "acceleration"=-77.02412999914401, "jerk"=-29.38804638461079, "heading"=-0.054200154916931975}, {"dt"=0.005, "x"=20.45066124640993, "y"=260.7187603028255, "position"=-20.46665074582325, "velocity"=-53.889819789188486, "acceleration"=-77.17255991819911, "jerk"=-29.685983811020833, "heading"=-0.05432671431317021}, {"dt"=0.005, "x"=20.72164216494947, "y"=260.73351199784815, "position"=-20.73803289468086, "velocity"=-54.27642977152194, "acceleration"=-77.32199646669073, "jerk"=-29.887309698324316, "heading"=-0.054439783526560204}, {"dt"=0.005, "x"=20.994555456331646, "y"=260.7483979580701, "position"=-21.011351859307872, "velocity"=-54.66379292540263, "acceleration"=-77.47263077613837, "jerk"=-30.126861889527845, "heading"=-0.054539093369314506}, {"dt"=0.005, "x"=21.2694050999328, "y"=260.7634149825399, "position"=-21.286611441541822, "velocity"=-55.05191644679024, "acceleration"=-77.62470427752106, "jerk"=-30.414700276537587, "heading"=-0.0546243723602482}, {"dt"=0.005, "x"=21.54619511752201, "y"=260.7785597169722, "position"=-21.56381547617707, "velocity"=-55.440806927049564, "acceleration"=-77.77809605186548, "jerk"=-30.678354868882707, "heading"=-0.05469534667763892}, {"dt"=0.005, "x"=21.824929571577282, "y"=260.79382865055715, "position"=-21.842967829221624, "velocity"=-55.83047060891085, "acceleration"=-77.93273637225724, "jerk"=-30.92806407835269, "heading"=-0.05475174011212991}, {"dt"=0.005, "x"=22.1056125691877, "y"=260.80921811302517, "position"=-22.12407240176114, "velocity"=-56.22091450790303, "acceleration"=-78.08877979843629, "jerk"=-31.208685235810663, "heading"=-0.05479327401972045}, {"dt"=0.005, "x"=22.388248261901676, "y"=260.82472427143676, "position"=-22.40713312977652, "velocity"=-56.612145603075525, "acceleration"=-78.24621903449867, "jerk"=-31.487847212474662, "heading"=-0.05481966727206555}, {"dt"=0.005, "x"=22.672840845341824, "y"=260.84034312690494, "position"=-22.692153983742106, "velocity"=-57.00417079311766, "acceleration"=-78.40503800842669, "jerk"=-31.763794785604205, "heading"=-0.05483063620565576}, {"dt"=0.005, "x"=22.959394562422652, "y"=260.8560705114596, "position"=-22.979138971847355, "velocity"=-57.39699762104985, "acceleration"=-78.56536558643796, "jerk"=-32.065515602255346, "heading"=-0.054825894569789146}, {"dt"=0.005, "x"=23.247855568958638, "y"=260.87189889541963, "position"=-23.268033918204228, "velocity"=-57.7789892713743, "acceleration"=-76.39833006489027, "jerk"=433.4071043095378, "heading"=-0.05480515926312368}, {"dt"=0.005, "x"=23.53811170649768, "y"=260.8878173823012, "position"=-23.55872623596251, "velocity"=-58.13846355165643, "acceleration"=-71.89485605642574, "jerk"=900.6948016929073, "heading"=-0.054768166503874616}, {"dt"=0.005, "x"=23.830050497276428, "y"=260.90381490698843, "position"=-23.851103010617194, "velocity"=-58.47535493093684, "acceleration"=-67.37827585608187, "jerk"=903.3160400687734, "heading"=-0.05471467597547924}, {"dt"=0.005, "x"=24.123559138403174, "y"=260.9198802517704, "position"=-24.145050995333932, "velocity"=-58.78959694334775, "acceleration"=-62.84840248218302, "jerk"=905.9746747797703, "heading"=-0.05464447112317222}, {"dt"=0.005, "x"=24.418524496223622, "y"=260.93600206298726, "position"=-24.4404566065045, "velocity"=-59.08112223411376, "acceleration"=-58.30505815320066, "jerk"=908.6688657964714, "heading"=-0.054557359431673225}, {"dt"=0.005, "x"=24.71483310107984, "y"=260.9521688682556, "position"=-24.737205919737782, "velocity"=-59.34986264665618, "acceleration"=-53.748082508484174, "jerk"=911.3951289432975, "heading"=-0.05445317268427069}, {"dt"=0.005, "x"=25.01237114244716, "y"=260.96836909423024, "position"=-25.035184666265668, "velocity"=-59.59574930557731, "acceleration"=-49.17733178422594, "jerk"=914.1501448516465, "heading"=-0.0543317672035496}, {"dt"=0.005, "x"=25.311024464949924, "y"=260.984591084886, "position"=-25.334278230259905, "velocity"=-59.818712798847336, "acceleration"=-44.59269865400586, "jerk"=916.9266260440168, "heading"=-0.05419302407372539}, {"dt"=0.005, "x"=25.610678575418692, "y"=261.00082312082486, "position"=-25.63437165723149, "velocity"=-60.01868539431677, "acceleration"=-39.99451909388654, "jerk"=919.635912023864, "heading"=-0.054036849338967796}, {"dt"=0.005, "x"=25.911218606986363, "y"=261.01705343663815, "position"=-25.935349619424898, "velocity"=-60.19559243868133, "acceleration"=-35.381408872912345, "jerk"=922.6220441948385, "heading"=-0.05386317420634379}, {"dt"=0.005, "x"=26.212529355999383, "y"=261.0332702425504, "position"=-26.237096454146958, "velocity"=-60.349366944411784, "acceleration"=-30.754901146090674, "jerk"=925.3015453643343, "heading"=-0.053671955193917265}, {"dt"=0.005, "x"=26.51449524740445, "y"=261.0494617424805, "position"=-26.539496130472916, "velocity"=-60.479935265191784, "acceleration"=-26.113664156000027, "jerk"=928.2473980181294, "heading"=-0.05346317429916836}, {"dt"=0.005, "x"=26.817000349595343, "y"=261.065616155017, "position"=-26.84243226548477, "velocity"=-60.58722700237102, "acceleration"=-21.458347435847713, "jerk"=931.0633440304628, "heading"=-0.053236839122346336}, {"dt"=0.005, "x"=27.11992835892783, "y"=261.0817217329536, "position"=-27.145788110127356, "velocity"=-60.67116892851687, "acceleration"=-16.788385229169478, "jerk"=933.9924413356471, "heading"=-0.05299298299170385}, {"dt"=0.005, "x"=27.423162612573094, "y"=261.0977667844818, "position"=-27.44944656343031, "velocity"=-60.73169066059091, "acceleration"=-12.10434641480731, "jerk"=936.8077628724336, "heading"=-0.0527316650505078}, {"dt"=0.005, "x"=27.726644898070056, "y"=261.11374278134326, "position"=-27.753349064384444, "velocity"=-60.78050019082672, "acceleration"=-9.761906047162938, "jerk"=468.48807352887434, "heading"=-0.05245291464960161}, {"dt"=0.005, "x"=28.0303757358102, "y"=261.1296443068974, "position"=-28.057495871550454, "velocity"=-60.82936143320187, "acceleration"=-9.772248475029244, "jerk"=-2.068485573261114, "heading"=-0.052156714461370934}, {"dt"=0.005, "x"=28.3343556185468, "y"=261.14546592460755, "position"=-28.361887219481904, "velocity"=-60.878269586290045, "acceleration"=-9.781630617635528, "jerk"=-1.876428521256912, "heading"=-0.05184304612444818}, {"dt"=0.005, "x"=28.638585102996913, "y"=261.1612021824392, "position"=-28.666523410731934, "velocity"=-60.92723825000581, "acceleration"=-9.793732743152361, "jerk"=-2.420425103366597, "heading"=-0.05151189015327118}, {"dt"=0.005, "x"=28.943064695136435, "y"=261.17684760650826, "position"=-28.971404701275894, "velocity"=-60.97625810879214, "acceleration"=-9.803971757266083, "jerk"=-2.0478028227444156, "heading"=-0.05116322605858303}, {"dt"=0.005, "x"=29.247794968425204, "y"=261.19239670680633, "position"=-29.276531419179666, "velocity"=-61.02534358075412, "acceleration"=-9.817094392396086, "jerk"=-2.624527026000578, "heading"=-0.05079703222036941}, {"dt"=0.005, "x"=29.552776461653945, "y"=261.2078439715461, "position"=-29.581903862599127, "velocity"=-61.074488683892405, "acceleration"=-9.829020627657314, "jerk"=-2.3852470522456315, "heading"=-0.05041328600416811}, {"dt"=0.005, "x"=29.858009752857967, "y"=261.22318387054776, "position"=-29.887522374081367, "velocity"=-61.12370229644828, "acceleration"=-9.842722511174884, "jerk"=-2.7403767035139026, "heading"=-0.050011963675561155}, {"dt"=0.005, "x"=30.16349541829863, "y"=261.23841085274245, "position"=-30.1933872997863, "velocity"=-61.172985140986015, "acceleration"=-9.856568907547114, "jerk"=-2.769279274446035, "heading"=-0.049593040450436554}, {"dt"=0.005, "x"=30.469234033584215, "y"=261.25351934584484, "position"=-30.499498990906666, "velocity"=-61.222338224073525, "acceleration"=-9.870616617502037, "jerk"=-2.8095419909845987, "heading"=-0.04915649049779214}, {"dt"=0.005, "x"=30.775226216993083, "y"=261.2685037580794, "position"=-30.805857847343596, "velocity"=-61.271771287385654, "acceleration"=-9.886612662425875, "jerk"=-3.1992089847676652, "heading"=-0.04870228687831463}, {"dt"=0.005, "x"=31.08147253969198, "y"=261.2833584733577, "position"=-31.112464228119656, "velocity"=-61.321276155212225, "acceleration"=-9.900973565314075, "jerk"=-2.872180577639938, "heading"=-0.04823040167711945}, {"dt"=0.005, "x"=31.387973650742826, "y"=261.298077856969, "position"=-31.41931857684116, "velocity"=-61.37086974430109, "acceleration"=-9.918717817772915, "jerk"=-3.5488504917680075, "heading"=-0.04774080581776119}, {"dt"=0.005, "x"=31.694730137701733, "y"=261.3126562484034, "position"=-31.72642128244335, "velocity"=-61.42054112043815, "acceleration"=-9.93427522741257, "jerk"=-3.1114819279309813, "heading"=-0.04723346927862704}, {"dt"=0.005, "x"=32.001742642940435, "y"=261.32708796654526, "position"=-32.03377279596081, "velocity"=-61.47030270349097, "acceleration"=-9.952316610564083, "jerk"=-3.6082766303024982, "heading"=-0.04670836091198527}, {"dt"=0.005, "x"=32.309011803453394, "y"=261.341367306347, "position"=-32.34137357058193, "velocity"=-61.52015492422391, "acceleration"=-9.970444146587454, "jerk"=-3.62550720467425, "heading"=-0.04616544854046578}, {"dt"=0.005, "x"=32.61653823633061, "y"=261.35548853777453, "position"=-32.6492240474294, "velocity"=-61.57009536949418, "acceleration"=-9.988089054054683, "jerk"=-3.5289814934458263, "heading"=-0.045604698989398784}, {"dt"=0.005, "x"=32.9243226353506, "y"=261.3694459098086, "position"=-32.95732475257983, "velocity"=-61.62014103008562, "acceleration"=-10.009132118287312, "jerk"=-4.208612846525739, "heading"=-0.04502607791204849}, {"dt"=0.005, "x"=33.23236560674666, "y"=261.3832336425083, "position"=-33.26567613298782, "velocity"=-61.67027608159838, "acceleration"=-10.027010302552242, "jerk"=-3.5756368529860083, "heading"=-0.04442955009455285}, {"dt"=0.005, "x"=33.54066783392077, "y"=261.39684593408026, "position"=-33.57427872170405, "velocity"=-61.72051774324547, "acceleration"=-10.048332329418486, "jerk"=-4.264405373248792, "heading"=-0.04381507915168836}, {"dt"=0.005, "x"=33.84922998243736, "y"=261.4102769561212, "position"=-33.88313304310855, "velocity"=-61.770864280900604, "acceleration"=-10.069307531026084, "jerk"=-4.1950403215196275, "heading"=-0.04318262770643133}, {"dt"=0.005, "x"=34.15805269562359, "y"=261.4235208530654, "position"=-34.192239608852425, "velocity"=-61.82131314877519, "acceleration"=-10.08977357491716, "jerk"=-4.093208778215285, "heading"=-0.042532157408386395}, {"dt"=0.005, "x"=34.46713669374983, "y"=261.4365717459908, "position"=-34.501599017475876, "velocity"=-61.871881724690745, "acceleration"=-10.113715183111083, "jerk"=-4.78832163878451, "heading"=-0.04186362872677135}, {"dt"=0.005, "x"=34.77648261463082, "y"=261.4494237253673, "position"=-34.81121179521543, "velocity"=-61.92255554791102, "acceleration"=-10.134764644054428, "jerk"=-4.209892188669073, "heading"=-0.04117700129097934}, {"dt"=0.005, "x"=35.08609114340593, "y"=261.4620708561662, "position"=-35.12107852625916, "velocity"=-61.97334620874717, "acceleration"=-10.158132167229894, "jerk"=-4.673504635093195, "heading"=-0.04047223361892255}, {"dt"=0.005, "x"=35.39596299946392, "y"=261.47450717674496, "position"=-35.43119984001615, "velocity"=-62.02426275139784, "acceleration"=-10.183308530135093, "jerk"=-5.035272581039862, "heading"=-0.0397492831385996}, {"dt"=0.005, "x"=35.70609882689767, "y"=261.48672669401054, "position"=-35.741576301849555, "velocity"=-62.07529236668101, "acceleration"=-10.205923056633992, "jerk"=-4.5229052997797226, "heading"=-0.03900810644742114}, {"dt"=0.005, "x"=36.016499335442845, "y"=261.4987233886552, "position"=-36.052208554501306, "velocity"=-62.12645053034933, "acceleration"=-10.231632733663787, "jerk"=-5.141935405958975, "heading"=-0.03824865898894908}, {"dt"=0.005, "x"=36.32716523301418, "y"=261.51049121194006, "position"=-36.36309725094855, "velocity"=-62.17773928944846, "acceleration"=-10.257751819825955, "jerk"=-5.223817232433703, "heading"=-0.0374708952092942}, {"dt"=0.005, "x"=36.638097178513256, "y"=261.5220240835242, "position"=-36.67424300756242, "velocity"=-62.22915132277389, "acceleration"=-10.282406665085375, "jerk"=-4.930969051883949, "heading"=-0.03667476868408692}, {"dt"=0.005, "x"=36.94929588859115, "y"=261.5333158950453, "position"=-36.98564651133457, "velocity"=-62.280700754431116, "acceleration"=-10.309886331445739, "jerk"=-5.495933272072762, "heading"=-0.03586023185428849}, {"dt"=0.005, "x"=37.26076207059669, "y"=261.5443605070877, "position"=-37.29730845316943, "velocity"=-62.33238836697154, "acceleration"=-10.337522508085328, "jerk"=-5.527235327917879, "heading"=-0.03502723619537218}, {"dt"=0.005, "x"=37.57249638699313, "y"=261.5551517475483, "position"=-37.60922949268077, "velocity"=-62.38420790226766, "acceleration"=-10.36390705922372, "jerk"=-5.2769102276784, "heading"=-0.03417573232263721}, {"dt"=0.005, "x"=37.88449954694724, "y"=261.5656834144273, "position"=-37.9214103502435, "velocity"=-62.43617151254575, "acceleration"=-10.392722055617298, "jerk"=-5.762999278715597, "heading"=-0.03330566975052851}, {"dt"=0.005, "x"=38.19677227241325, "y"=261.57594927406865, "position"=-38.233851773464146, "velocity"=-62.48828464412984, "acceleration"=-10.42262631681865, "jerk"=-5.980852240270451, "heading"=-0.03241699698138045}, {"dt"=0.005, "x"=38.509315215671776, "y"=261.58594305803905, "position"=-38.546554455094395, "velocity"=-62.54053632605029, "acceleration"=-10.450336384089098, "jerk"=-5.542013454089556, "heading"=-0.03150966174817038}, {"dt"=0.005, "x"=38.82212906793701, "y"=261.59565846630477, "position"=-38.8595191421228, "velocity"=-62.59293740568076, "acceleration"=-10.48021592609416, "jerk"=-5.975908401012475, "heading"=-0.030583610714597365}, {"dt"=0.005, "x"=39.1352145657247, "y"=261.6050891667772, "position"=-39.17274664256994, "velocity"=-62.64550008942885, "acceleration"=-10.512536749618562, "jerk"=-6.464164704880204, "heading"=-0.02963878944937004}, {"dt"=0.005, "x"=39.44857235439204, "y"=261.61422879071046, "position"=-39.48623768940242, "velocity"=-62.69820936649671, "acceleration"=-10.54185541357242, "jerk"=-5.863732790771792, "heading"=-0.028675142841681656}, {"dt"=0.005, "x"=39.76220310990168, "y"=261.623070936041, "position"=-39.79999306279958, "velocity"=-62.75107467943201, "acceleration"=-10.573062587059212, "jerk"=-6.241434697358272, "heading"=-0.02769261474747392}, {"dt"=0.005, "x"=40.07610752064636, "y"=261.6316091662809, "position"=-40.114013572417335, "velocity"=-62.804101923551514, "acceleration"=-10.605448823901042, "jerk"=-6.477247368366079, "heading"=-0.026691148044279245}, {"dt"=0.005, "x"=40.39028629274686, "y"=261.6398370101132, "position"=-40.428300063143084, "velocity"=-62.85729814514932, "acceleration"=-10.63924431956167, "jerk"=-6.759099132125357, "heading"=-0.025670684615507144}, {"dt"=0.005, "x"=40.70474005293069, "y"=261.6477479584239, "position"=-40.74285331840668, "velocity"=-62.910651052719246, "acceleration"=-10.6705815139847, "jerk"=-6.267438884606236, "heading"=-0.024631165674522115}, {"dt"=0.005, "x"=41.019469464127674, "y"=261.6553354669576, "position"=-41.05767417628962, "velocity"=-62.964171576587844, "acceleration"=-10.704104773719791, "jerk"=-6.704651947018192, "heading"=-0.023572531400882835}, {"dt"=0.005, "x"=41.33447518529154, "y"=261.66259295473907, "position"=-41.3727634898102, "velocity"=-63.017862704114116, "acceleration"=-10.738225505254206, "jerk"=-6.824146306882994, "heading"=-0.022494721074098778}, {"dt"=0.005, "x"=41.64975790927228, "y"=261.669513804416, "position"=-41.68812216529094, "velocity"=-63.07173509614856, "acceleration"=-10.774478406888477, "jerk"=-7.250580326854106, "heading"=-0.021397672947609525}, {"dt"=0.005, "x"=41.96531823186605, "y"=261.67609135892036, "position"=-42.003751031871204, "velocity"=-63.12577331605241, "acceleration"=-10.807643980770365, "jerk"=-6.633114776377624, "heading"=-0.020281324711831306}, {"dt"=0.005, "x"=42.281156786595595, "y"=261.68231892409676, "position"=-42.31965097682478, "velocity"=-63.17998899071582, "acceleration"=-10.84313493268212, "jerk"=-7.098190382350822, "heading"=-0.01914561303977602}, {"dt"=0.005, "x"=42.597274198023854, "y"=261.68818976715534, "position"=-42.6358228993706, "velocity"=-63.23438450916445, "acceleration"=-10.879103689725866, "jerk"=-7.193751408749449, "heading"=-0.01799047375417162}, {"dt"=0.005, "x"=42.91367108845417, "y"=261.69369711633647, "position"=-42.9522677178919, "velocity"=-63.28896370425989, "acceleration"=-10.91583901908848, "jerk"=-7.347065872522762, "heading"=-0.016815841811278875}, {"dt"=0.005, "x"=43.230348089315875, "y"=261.6988341605986, "position"=-43.26898638184859, "velocity"=-63.34373279133894, "acceleration"=-10.953817415808942, "jerk"=-7.595679344092332, "heading"=-0.015621651264711545}, {"dt"=0.005, "x"=43.54730575886572, "y"=261.7035940478698, "position"=-43.58597979000293, "velocity"=-63.3986816308674, "acceleration"=-10.989767905692815, "jerk"=-7.190097976774723, "heading"=-0.01440783558692399}, {"dt"=0.005, "x"=43.86454467872465, "y"=261.70796988625693, "position"=-43.903248887512994, "velocity"=-63.453819502012976, "acceleration"=-11.027574229115089, "jerk"=-7.561264684454727, "heading"=-0.013174327319233403}, {"dt"=0.005, "x"=44.18206541798674, "y"=261.7119547429676, "position"=-44.2207946305872, "velocity"=-63.5091486148415, "acceleration"=-11.065822565704764, "jerk"=-7.649667317934927, "heading"=-0.011921058214635183}, {"dt"=0.005, "x"=44.499868532459104, "y"=261.71554164386794, "position"=-44.538617986284045, "velocity"=-63.56467113936864, "acceleration"=-11.104504905428314, "jerk"=-7.736467944710057, "heading"=-0.01064795925167522}, {"dt"=0.005, "x"=44.817954563885706, "y"=261.71872357304585, "position"=-44.85671993230453, "velocity"=-63.62038920409682, "acceleration"=-11.143612945635084, "jerk"=-7.821608041354011, "heading"=-0.00935496064885355}, {"dt"=0.005, "x"=45.13632406334924, "y"=261.72149347257283, "position"=-45.175101480972245, "velocity"=-63.67630973354282, "acceleration"=-11.184105889201135, "jerk"=-8.09858871321012, "heading"=-0.008041991779076774}, {"dt"=0.005, "x"=45.45497752297473, "y"=261.7238442414635, "position"=-45.493763611520684, "velocity"=-63.73242610968749, "acceleration"=-11.223275228933005, "jerk"=-7.833867946374085, "heading"=-0.0067089814623131905}, {"dt"=0.005, "x"=45.77391543058627, "y"=261.72576873583915, "position"=-45.81270732534842, "velocity"=-63.788742765547624, "acceleration"=-11.263331172027335, "jerk"=-8.011188618866072, "heading"=-0.005355857757466886}, {"dt"=0.005, "x"=46.093138263464056, "y"=261.727259768412, "position"=-46.13193364038001, "velocity"=-63.845263006319016, "acceleration"=-11.304048154278235, "jerk"=-8.143396450179807, "heading"=-0.003982547998840569}, {"dt"=0.005, "x"=46.412646480690285, "y"=261.72831010801264, "position"=-46.451443584025526, "velocity"=-63.901988729102854, "acceleration"=-11.34514455676765, "jerk"=-8.219280497883119, "heading"=-0.002588978841237932}, {"dt"=0.005, "x"=46.73244052226883, "y"=261.72891247918926, "position"=-46.77123819292345, "velocity"=-63.95892177958466, "acceleration"=-11.386610096360528, "jerk"=-8.293107918575515, "heading"=-0.0011750762778853785}, {"dt"=0.005, "x"=47.052520808226504, "y"=261.7290595618137, "position"=-47.09131851267467, "velocity"=-64.01606395024419, "acceleration"=-11.428434131906329, "jerk"=-8.36480710916021, "heading"=-6.282926072838585}, {"dt"=0.005, "x"=47.372887737695464, "y"=261.7287439906954, "position"=-47.41168559756714, "velocity"=-64.07341697849445, "acceleration"=-11.470605650052335, "jerk"=-8.434303629201167, "heading"=-6.281471278890596}, {"dt"=0.005, "x"=47.693541687976705, "y"=261.7279583552048, "position"=-47.73234051029122, "velocity"=-64.1309825448163, "acceleration"=-11.5131132643711, "jerk"=-8.501522863753053, "heading"=-6.279995925736066}, {"dt"=0.005, "x"=48.01448301358395, "y"=261.72669519890434, "position"=-48.05328432164514, "velocity"=-64.18876227078202, "acceleration"=-11.555945193143202, "jerk"=-8.56638575442048, "heading"=-6.2784999369142875}, {"dt"=0.005, "x"=48.33571204526797, "y"=261.72494701919015, "position"=-48.374518110230596, "velocity"=-64.24675771709136, "acceleration"=-11.59908926186688, "jerk"=-8.628813744735453, "heading"=-6.2769832354026125}, {"dt"=0.005, "x"=48.65722908902099, "y"=261.7227062669434, "position"=-48.696042962138364, "velocity"=-64.30497038155356, "acceleration"=-11.642532892440727, "jerk"=-8.688726114769452, "heading"=-6.275445743638507}, {"dt"=0.005, "x"=48.97903442506069, "y"=261.7199653461923, "position"=-49.01785997062329, "velocity"=-64.36340169698605, "acceleration"=-11.686263086497206, "jerk"=-8.746038811295875, "heading"=-6.273887383542361}, {"dt"=0.005, "x"=49.30112830679377, "y"=261.7167166137851, "position"=-49.339970235768845, "velocity"=-64.42205302911049, "acceleration"=-11.730266424888214, "jerk"=-8.800667678201535, "heading"=-6.272308076541074}, {"dt"=0.005, "x"=49.62351095975838, "y"=261.71295237907566, "position"=-49.66237486414047, "velocity"=-64.4809256743249, "acceleration"=-11.774529042881454, "jerk"=-8.852523598648077, "heading"=-6.2707077435924266}, {"dt"=0.005, "x"=49.94618258054592, "y"=261.70866490362073, "position"=-49.98507496842839, "velocity"=-64.54002085758516, "acceleration"=-11.819036652053683, "jerk"=-8.901521834445703, "heading"=-6.269086305210262}, {"dt"=0.005, "x"=50.269143335700925, "y"=261.70384640089077, "position"=-50.308071667078465, "velocity"=-64.59933973001509, "acceleration"=-11.863774485985346, "jerk"=-8.947566786332573, "heading"=-6.267443681490498}, {"dt"=0.005, "x"=50.592393360599466, "y"=261.6984890359942, "position"=-50.6313660839117, "velocity"=-64.65888336664736, "acceleration"=-11.908727326454027, "jerk"=-8.990568093736329, "heading"=-6.2657797921379865}, {"dt"=0.005, "x"=50.91593275830586, "y"=261.6925849254165, "position"=-50.954959347732085, "velocity"=-64.7186527640766, "acceleration"=-11.953879485847096, "jerk"=-9.030431878613854, "heading"=-6.264094556494244}, {"dt"=0.005, "x"=51.23976159840675, "y"=261.6861261367741, "position"=-51.278852591921925, "velocity"=-64.77864883796761, "acceleration"=-11.999214778202827, "jerk"=-9.067058471146083, "heading"=-6.262387893566057}, {"dt"=0.005, "x"=51.56387991582318, "y"=261.6791046885843, "position"=-51.60304695402518, "velocity"=-64.83887242065151, "acceleration"=-12.044716536780697, "jerk"=-9.100351715574106, "heading"=-6.260659722055016}, {"dt"=0.005, "x"=51.888287709599695, "y"=261.6715125500518, "position"=-51.92754357531798, "velocity"=-64.89932425856007, "acceleration"=-12.090367581711803, "jerk"=-9.130208986221078, "heading"=-6.258909960387953}, {"dt"=0.005, "x"=52.212984941670896, "y"=261.66334164087255, "position"=-52.252343600366494, "velocity"=-64.96000500970273, "acceleration"=-12.13615022853105, "jerk"=-9.156529363849586, "heading"=-6.257138526748338}, {"dt"=0.005, "x"=52.53797153560452, "y"=261.65458383105573, "position"=-52.57744817657139, "velocity"=-65.02091524097924, "acceleration"=-12.18204625530177, "jerk"=-9.17920535414396, "heading"=-6.255345339108642}, {"dt"=0.005, "x"=52.8632473753216, "y"=261.64523094076475, "position"=-52.902858453699274, "velocity"=-65.08205542557681, "acceleration"=-12.228036919515262, "jerk"=-9.198132842698215, "heading"=-6.253530315263679}, {"dt"=0.005, "x"=53.188812320550646, "y"=261.6352747396501, "position"=-53.22857560016631, "velocity"=-65.1434292934071, "acceleration"=-12.274773566056751, "jerk"=-9.347329308297958, "heading"=-6.251693372769886}, {"dt"=0.005, "x"=53.51466618259969, "y"=261.62470694733855, "position"=-53.5546007796335, "velocity"=-65.20503589343905, "acceleration"=-12.321320006390124, "jerk"=-9.309288066674526, "heading"=-6.249834429106812}, {"dt"=0.005, "x"=53.84080869495552, "y"=261.61351923437934, "position"=-53.88093512242787, "velocity"=-65.26686855887304, "acceleration"=-12.366533086799336, "jerk"=-9.042616081842425, "heading"=-6.247953401878108}, {"dt"=0.005, "x"=54.167239569705636, "y"=261.601703220345, "position"=-54.20757978284311, "velocity"=-65.32893208304766, "acceleration"=-12.412704834923716, "jerk"=-9.234349624875904, "heading"=-6.2460502085209475}, {"dt"=0.005, "x"=54.493958472530046, "y"=261.5892504744806, "position"=-54.534535914980665, "velocity"=-65.3912264275107, "acceleration"=-12.458868892608166, "jerk"=-9.23281153689004, "heading"=-6.244124766477078}, {"dt"=0.005, "x"=54.82096502127804, "y"=261.57615251567626, "position"=-54.86180467219546, "velocity"=-65.45375144295862, "acceleration"=-12.50500308958351, "jerk"=-9.226839395068964, "heading"=-6.242176993232494}, {"dt"=0.005, "x"=55.14825881784163, "y"=261.5624008110328, "position"=-55.18938723987819, "velocity"=-65.51651353654546, "acceleration"=-12.552418717368141, "jerk"=-9.483125556926097, "heading"=-6.240206806156601}, {"dt"=0.005, "x"=55.47583937969954, "y"=261.54798677856695, "position"=-55.517284767833296, "velocity"=-65.57950559102211, "acceleration"=-12.598410895330403, "jerk"=-9.19843559245237, "heading"=-6.238214122943167}, {"dt"=0.005, "x"=55.80370614337205, "y"=261.5329017873627, "position"=-55.84549837462119, "velocity"=-65.64272135757754, "acceleration"=-12.643153311086053, "jerk"=-8.948483151129949, "heading"=-6.2361988616334925}, {"dt"=0.005, "x"=56.13185852065665, "y"=261.5171371551102, "position"=-56.17402920475375, "velocity"=-65.70616602651276, "acceleration"=-12.688933787043766, "jerk"=-9.15609519154259, "heading"=-6.234160940309314}, {"dt"=0.005, "x"=56.460295881527585, "y"=261.50068414871697, "position"=-56.502878412499854, "velocity"=-65.76984154922121, "acceleration"=-12.735104541690134, "jerk"=-9.23415092927371, "heading"=-6.232100277227126}, {"dt"=0.005, "x"=56.78901757993391, "y"=261.4835339828493, "position"=-56.83204718865037, "velocity"=-65.83375523010338, "acceleration"=-12.782736176433218, "jerk"=-9.52632694861677, "heading"=-6.2300167906862045}, {"dt"=0.005, "x"=57.118022793043885, "y"=261.4656778284749, "position"=-57.161536600472026, "velocity"=-65.8978823643311, "acceleration"=-12.825426845543575, "jerk"=-8.538133822071359, "heading"=-6.227910400087494}, {"dt"=0.005, "x"=57.44731070183177, "y"=261.44710680384605, "position"=-57.49134777346297, "velocity"=-65.96223459818874, "acceleration"=-12.870446771529487, "jerk"=-9.003985197182374, "heading"=-6.225781024836646}, {"dt"=0.005, "x"=57.77688047744513, "y"=261.42781197477626, "position"=-57.82148187867883, "velocity"=-66.0268210431719, "acceleration"=-12.917288996632692, "jerk"=-9.368445020641047, "heading"=-6.223628584452614}, {"dt"=0.005, "x"=58.10673116832879, "y"=261.4077843612192, "position"=-58.15194002062909, "velocity"=-66.09162839005185, "acceleration"=-12.961469375989054, "jerk"=-8.836075871272442, "heading"=-6.221452999339665}, {"dt"=0.005, "x"=58.436861724420424, "y"=261.3870149365612, "position"=-58.48272326244463, "velocity"=-66.15664836310762, "acceleration"=-13.003994611153757, "jerk"=-8.505047032940638, "heading"=-6.219254190686253}, {"dt"=0.005, "x"=58.76727111149005, "y"=261.36549462065193, "position"=-58.813832741409755, "velocity"=-66.22189579302511, "acceleration"=-13.049485983498244, "jerk"=-9.098274468897216, "heading"=-6.217032079745915}, {"dt"=0.005, "x"=59.09795820851794, "y"=261.343214286177, "position"=-59.14526956713232, "velocity"=-66.2873651445127, "acceleration"=-13.093870297518606, "jerk"=-8.876862804072516, "heading"=-6.2147865885543645}, {"dt"=0.005, "x"=59.42892173841102, "y"=261.32016476405806, "position"=-59.477034753053324, "velocity"=-66.3530371842014, "acceleration"=-13.134407937738501, "jerk"=-8.107528043979073, "heading"=-6.212517640457433}, {"dt"=0.005, "x"=59.76016047914256, "y"=261.29633682933644, "position"=-59.80912942906382, "velocity"=-66.41893520209914, "acceleration"=-13.17960357954746, "jerk"=-9.039128361791882, "heading"=-6.210225158716788}, {"dt"=0.005, "x"=60.09167305754802, "y"=261.2717212156293, "position"=-60.14155463580846, "velocity"=-66.48504134892696, "acceleration"=-13.221229365564113, "jerk"=-8.325157203330491, "heading"=-6.207909067962685}, {"dt"=0.005, "x"=60.42345798689033, "y"=261.2463086135083, "position"=-60.47431136329153, "velocity"=-66.55134549661354, "acceleration"=-13.260829537315999, "jerk"=-7.920034350377136, "heading"=-6.205569294001157}, {"dt"=0.005, "x"=60.755513874031685, "y"=261.2200896547936, "position"=-60.80740075967231, "velocity"=-66.61787927615767, "acceleration"=-13.306755908826062, "jerk"=-9.185274302012658, "heading"=-6.2032057623941865}, {"dt"=0.005, "x"=61.08783901072604, "y"=261.1930549447356, "position"=-61.140823722329124, "velocity"=-66.68459253136164, "acceleration"=-13.342651040795772, "jerk"=-7.179026393941967, "heading"=-6.2008184014030965}, {"dt"=0.005, "x"=61.42043179157971, "y"=261.16519502985415, "position"=-61.474581318097634, "velocity"=-66.75151915370203, "acceleration"=-13.385324468077897, "jerk"=-8.534685456424995, "heading"=-6.198407139073686}, {"dt"=0.005, "x"=61.7532904447491, "y"=261.13650041982316, "position"=-61.80867451412917, "velocity"=-66.81863920630815, "acceleration"=-13.42401052122284, "jerk"=-7.737210628988578, "heading"=-6.19597190520698}, {"dt"=0.005, "x"=62.08641310977368, "y"=261.1069615820994, "position"=-62.1431042569559, "velocity"=-66.8859485653452, "acceleration"=-13.46187180741083, "jerk"=-7.5722572375980235, "heading"=-6.193512630863166}, {"dt"=0.005, "x"=62.419797913330896, "y"=261.07656893562546, "position"=-62.47787154956761, "velocity"=-66.95345852234203, "acceleration"=-13.50199139936592, "jerk"=-8.023918391018015, "heading"=-6.191029247850655}, {"dt"=0.005, "x"=62.75344276199645, "y"=261.0453128702759, "position"=-62.81297724433002, "velocity"=-67.02113895248239, "acceleration"=-13.536086028071281, "jerk"=-6.818925741072235, "heading"=-6.18852169032162}, {"dt"=0.005, "x"=63.087345643222285, "y"=261.01318371992176, "position"=-63.14842234623701, "velocity"=-67.08902038139797, "acceleration"=-13.57628578311676, "jerk"=-8.039951009095603, "heading"=-6.185989892580465}, {"dt"=0.005, "x"=63.421504252175176, "y"=260.9801717983783, "position"=-63.48420763909738, "velocity"=-67.15705857207308, "acceleration"=-13.607638135022171, "jerk"=-6.270470381082305, "heading"=-6.183433791951375}, {"dt"=0.005, "x"=63.75591639974006, "y"=260.946267360929, "position"=-63.82033409642811, "velocity"=-67.22529146614671, "acceleration"=-13.64657881472624, "jerk"=-7.788135940813845, "heading"=-6.18085332574224}, {"dt"=0.005, "x"=64.090579590435, "y"=260.9114606469339, "position"=-64.1568024583067, "velocity"=-67.29367237571627, "acceleration"=-13.676181913911023, "jerk"=-5.9206198369565755, "heading"=-6.178248434533795}, {"dt"=0.005, "x"=64.42549142192192, "y"=260.87574184039806, "position"=-64.4936136339085, "velocity"=-67.36223512036042, "acceleration"=-13.71254892883087, "jerk"=-7.27340298396939, "heading"=-6.175619059161447}, {"dt"=0.005, "x"=64.76064922778384, "y"=260.83910110795836, "position"=-64.83076834335787, "velocity"=-67.43094188987672, "acceleration"=-13.741353903259323, "jerk"=-5.760994885690707, "heading"=-6.172965143553779}, {"dt"=0.005, "x"=65.09605035677808, "y"=260.80152857047045, "position"=-65.16826739951046, "velocity"=-67.49981123051748, "acceleration"=-13.77386812815189, "jerk"=-6.502844978513167, "heading"=-6.170286632611656}, {"dt"=0.005, "x"=65.43169198996455, "y"=260.76301432376255, "position"=-65.50611152499965, "velocity"=-67.56882509783865, "acceleration"=-13.802773464234974, "jerk"=-5.781067216616975, "heading"=-6.167583473711987}, {"dt"=0.005, "x"=65.76757119278521, "y"=260.723548434474, "position"=-65.84430140554723, "velocity"=-67.6379761095136, "acceleration"=-13.830202334989394, "jerk"=-5.485774150884026, "heading"=-6.1648556163699935}, {"dt"=0.005, "x"=66.10368501062857, "y"=260.68312092978545, "position"=-66.18283778716756, "velocity"=-67.70727632406465, "acceleration"=-13.860042910209813, "jerk"=-5.968115044083788, "heading"=-6.162103011523147}, {"dt"=0.005, "x"=66.44003022181627, "y"=260.64172182821835, "position"=-66.52172122833791, "velocity"=-67.77668823407194, "acceleration"=-13.882382001457927, "jerk"=-4.467818249622724, "heading"=-6.159325613616925}, {"dt"=0.005, "x"=66.77660366400396, "y"=260.5993411016284, "position"=-66.86095242969232, "velocity"=-67.84624027088294, "acceleration"=-13.910407362200772, "jerk"=-5.605072148568979, "heading"=-6.156523377998246}, {"dt"=0.005, "x"=67.11340192286991, "y"=260.5559687147102, "position"=-67.20053192130234, "velocity"=-67.91589832200371, "acceleration"=-13.931610224153701, "jerk"=-4.2405723905858395, "heading"=-6.15369626355041}, {"dt"=0.005, "x"=67.45042149724831, "y"=260.51159460646124, "position"=-67.54046022991622, "velocity"=-67.98566172277536, "acceleration"=-13.952680154329755, "jerk"=-4.213986035210837, "heading"=-6.150844231407743}, {"dt"=0.005, "x"=67.78765887578103, "y"=260.4662086808739, "position"=-67.88073795725235, "velocity"=-68.05554546722642, "acceleration"=-13.97674889021232, "jerk"=-4.813747176513061, "heading"=-6.147967244360675}, {"dt"=0.005, "x"=68.12511024144936, "y"=260.41980084801884, "position"=-68.22136548277211, "velocity"=-68.125505103954, "acceleration"=-13.99192734551491, "jerk"=-3.03569106051782, "heading"=-6.1450652694423376}, {"dt"=0.005, "x"=68.46277175942704, "y"=260.3723609875866, "position"=-68.56234325489343, "velocity"=-68.19555442426449, "acceleration"=-14.009864062097677, "jerk"=-3.587343316553415, "heading"=-6.142138275560648}, {"dt"=0.005, "x"=68.80063952023772, "y"=260.32387895732415, "position"=-68.90367173459238, "velocity"=-68.26569593978888, "acceleration"=-14.02830310487957, "jerk"=-3.6878085563785135, "heading"=-6.1391862340354955}, {"dt"=0.005, "x"=69.13870934336659, "y"=260.27434462316364, "position"=-69.24535119779013, "velocity"=-68.33589263955078, "acceleration"=-14.039339952378782, "jerk"=-2.207369499842571, "heading"=-6.136209120393161}, {"dt"=0.005, "x"=69.47697699580067, "y"=260.223747830287, "position"=-69.58738195683479, "velocity"=-68.40615180893303, "acceleration"=-14.051833876450814, "jerk"=-2.498784814406463, "heading"=-6.133206912545325}, {"dt"=0.005, "x"=69.81543817636992, "y"=260.17207840634813, "position"=-69.92976434557946, "velocity"=-68.47647774893382, "acceleration"=-14.065188000157036, "jerk"=-2.6708247412443598, "heading"=-6.130179590980567}, {"dt"=0.005, "x"=70.15408832198813, "y"=260.1193261930227, "position"=-70.27249852411724, "velocity"=-68.54683570755509, "acceleration"=-14.071591724254517, "jerk"=-1.280744819496249, "heading"=-6.127127140573875}, {"dt"=0.005, "x"=70.49292278502796, "y"=260.0654810216791, "position"=-70.61558465881305, "velocity"=-68.61722693916205, "acceleration"=-14.078246321392385, "jerk"=-1.3309194275734626, "heading"=-6.124049549092932}, {"dt"=0.005, "x"=70.8319368018925, "y"=260.0105327199398, "position"=-70.95902289124308, "velocity"=-68.68764648600504, "acceleration"=-14.083909368596892, "jerk"=-1.1326094409014331, "heading"=-6.120946807548997}, {"dt"=0.005, "x"=71.17112548199334, "y"=259.95447111546844, "position"=-71.3028133277076, "velocity"=-68.75808729290253, "acceleration"=-14.088161379498843, "jerk"=-0.8504021803901196, "heading"=-6.117818910371953}, {"dt"=0.005, "x"=71.51048371315224, "y"=259.89728605423005, "position"=-71.64695594390636, "velocity"=-68.82852323975385, "acceleration"=-14.087189370263786, "jerk"=0.19440184701124963, "heading"=-6.11466585636935}, {"dt"=0.005, "x"=71.85000628668256, "y"=259.8389673825605, "position"=-71.99145071222941, "velocity"=-68.89895366460968, "acceleration"=-14.086084971165747, "jerk"=0.22087981960794423, "heading"=-6.111487647660861}, {"dt"=0.005, "x"=72.18968784717471, "y"=259.77950495782096, "position"=-72.33629755141209, "velocity"=-68.96936783653712, "acceleration"=-14.082834385487786, "jerk"=0.6501171355921542, "heading"=-6.108284290219658}, {"dt"=0.005, "x"=72.52952293564121, "y"=259.7188886432803, "position"=-72.68149637085028, "velocity"=-69.03976388763961, "acceleration"=-14.07921022049834, "jerk"=0.7248329978892798, "heading"=-6.10505579354443}, {"dt"=0.005, "x"=72.8695058456947, "y"=259.65710833647245, "position"=-73.02704692494869, "velocity"=-69.1101108196811, "acceleration"=-14.069386408297646, "jerk"=1.9647624401386565, "heading"=-6.101802172108957}, {"dt"=0.005, "x"=73.20963076882373, "y"=259.59415394651546, "position"=-73.37294896100569, "velocity"=-69.18040721140093, "acceleration"=-14.059278343967208, "jerk"=2.0216128660877075, "heading"=-6.098523444074759}, {"dt"=0.005, "x"=73.54989174211067, "y"=259.5300154061281, "position"=-73.71920216648573, "velocity"=-69.2506410960078, "acceleration"=-14.046776921372839, "jerk"=2.500284518873741, "heading"=-6.095219631867775}, {"dt"=0.005, "x"=73.89028264655451, "y"=259.4646826749655, "position"=-74.06580616760121, "velocity"=-69.3208002230948, "acceleration"=-14.031825417401933, "jerk"=2.9903007941811666, "heading"=-6.091890762279957}, {"dt"=0.005, "x"=74.23079723456279, "y"=259.3981457373006, "position"=-74.41276055757238, "velocity"=-69.39087799423531, "acceleration"=-14.015554228100768, "jerk"=3.2542378602329336, "heading"=-6.088536866282909}, {"dt"=0.005, "x"=74.57142904205973, "y"=259.3303946223404, "position"=-74.7600648072685, "velocity"=-69.46084993922385, "acceleration"=-13.994388997707574, "jerk"=4.233046078638836, "heading"=-6.0851579799781605}, {"dt"=0.005, "x"=74.91217146799626, "y"=259.2614193922784, "position"=-75.1077183462915, "velocity"=-69.53070780459919, "acceleration"=-13.971573075068022, "jerk"=4.56318452791038, "heading"=-6.081754143905792}, {"dt"=0.005, "x"=75.25301775351265, "y"=259.1912101495828, "position"=-75.45572054184524, "velocity"=-69.60043911074554, "acceleration"=-13.946261229270362, "jerk"=5.062369159531954, "heading"=-6.078325403332127}, {"dt"=0.005, "x"=75.59396097617403, "y"=259.11975704160426, "position"=-75.80407069286935, "velocity"=-69.67003020482151, "acceleration"=-13.918218815194905, "jerk"=5.60848281509152, "heading"=-6.074871808392415}, {"dt"=0.005, "x"=75.93499404867549, "y"=259.04705026441553, "position"=-76.1527680286621, "velocity"=-69.73946715854878, "acceleration"=-13.887390745452421, "jerk"=6.165613948496684, "heading"=-6.071393414189597}, {"dt"=0.005, "x"=76.2761097200438, "y"=258.97308006620165, "position"=-76.50181170999275, "velocity"=-69.80873626613138, "acceleration"=-13.853821516519815, "jerk"=6.713845786521233, "heading"=-6.067890280867222}, {"dt"=0.005, "x"=76.61730058330596, "y"=258.8978367492566, "position"=-76.85120083678187, "velocity"=-69.87782535782469, "acceleration"=-13.817818338662846, "jerk"=7.200635571393832, "heading"=-6.064362473614072}, {"dt"=0.005, "x"=76.95855903099996, "y"=258.82131068367306, "position"=-77.20093440228027, "velocity"=-69.94671309967843, "acceleration"=-13.777548370748605, "jerk"=8.053993582848307, "heading"=-6.0608100632095585}, {"dt"=0.005, "x"=77.29987730510221, "y"=258.74349230039934, "position"=-77.5510113438395, "velocity"=-70.01538831184881, "acceleration"=-13.73504243407524, "jerk"=8.501187334672977, "heading"=-6.057233125594233}, {"dt"=0.005, "x"=77.64124747748116, "y"=258.6643720994849, "position"=-77.9014305225138, "velocity"=-70.08383573485914, "acceleration"=-13.68948460206525, "jerk"=9.111566401998061, "heading"=-6.053631742153799}, {"dt"=0.005, "x"=77.98266144912526, "y"=258.5839406543822, "position"=-78.25219072178834, "velocity"=-70.15203985490615, "acceleration"=-13.640824009402763, "jerk"=9.732118532497225, "heading"=-6.050005999810359}, {"dt"=0.005, "x"=78.32411094947166, "y"=258.5021886163193, "position"=-78.60329064633154, "velocity"=-70.21998490864165, "acceleration"=-13.589010747099906, "jerk"=10.362652460571553, "heading"=-6.046355991111911}, {"dt"=0.005, "x"=78.66558753584049, "y"=258.41910671874126, "position"=-78.95472892077426, "velocity"=-70.2876548885436, "acceleration"=-13.533995980390046, "jerk"=11.002953341971988, "heading"=-6.0426818143199315}, {"dt"=0.005, "x"=79.00708259297902, "y"=258.33468578181726, "position"=-79.30650408851805, "velocity"=-70.35503354875895, "acceleration"=-13.47573204307082, "jerk"=11.652787463845016, "heading"=-6.038983573494877}, {"dt"=0.005, "x"=79.34858733271906, "y"=258.2489167170108, "position"=-79.65861461057426, "velocity"=-70.4221044112409, "acceleration"=-13.414172496388233, "jerk"=12.311909336517601, "heading"=-6.035261378579466}, {"dt"=0.005, "x"=79.69009279375224, "y"=258.16179053171, "position"=-80.01105886443656, "velocity"=-70.48885077246028, "acceleration"=-13.349272243877408, "jerk"=12.980050502164886, "heading"=-6.031515345479562}, {"dt"=0.005, "x"=80.03158984545439, "y"=258.0732983328898, "position"=-80.3638351470482, "velocity"=-70.55525652232858, "acceleration"=-13.281149973659012, "jerk"=13.62445404367918, "heading"=-6.027745596099019}, {"dt"=0.005, "x"=80.37306917679541, "y"=257.98343133472065, "position"=-80.71694166227137, "velocity"=-70.62130304463247, "acceleration"=-13.209304460778526, "jerk"=14.369102576097248, "heading"=-6.023952258537759}, {"dt"=0.005, "x"=80.7145213049328, "y"=257.89218086123253, "position"=-81.07037652857824, "velocity"=-70.686973261375, "acceleration"=-13.134043348506452, "jerk"=15.052222454414732, "heading"=-6.02013546707234}, {"dt"=0.005, "x"=81.05593657630624, "y"=257.7995383509072, "position"=-81.42413777892425, "velocity"=-70.75225006920303, "acceleration"=-13.055361565605494, "jerk"=15.736356580191568, "heading"=-6.016295362216069}, {"dt"=0.005, "x"=81.39730516498848, "y"=257.7054953620919, "position"=-81.77822335768202, "velocity"=-70.81711575155394, "acceleration"=-12.973136470182567, "jerk"=16.44501908458551, "heading"=-6.012432090808252}, {"dt"=0.005, "x"=81.73861707324973, "y"=257.61004357791836, "position"=-82.13263111976244, "velocity"=-70.88155241608128, "acceleration"=-12.88733290546702, "jerk"=17.160712943109502, "heading"=-6.008545806077238}, {"dt"=0.005, "x"=82.07986213226573, "y"=257.5131748112563, "position"=-82.48735882978445, "velocity"=-70.94554200440318, "acceleration"=-12.79791766438052, "jerk"=17.8830482172998, "heading"=-6.004636667699919}, {"dt"=0.005, "x"=82.42103000297546, "y"=257.41488100969616, "position"=-82.84240416129826, "velocity"=-71.00906630276255, "acceleration"=-12.704859671873692, "jerk"=18.611598501365734, "heading"=-6.0007048418574795}, {"dt"=0.005, "x"=82.76211017708967, "y"=257.3151542605564, "position"=-83.19776469606226, "velocity"=-71.07210695280105, "acceleration"=-12.608130007700424, "jerk"=19.345932834653468, "heading"=-5.996750501287242}, {"dt"=0.005, "x"=83.10309197825539, "y"=257.21398679591056, "position"=-83.55343792337787, "velocity"=-71.1346454631202, "acceleration"=-12.507702063828674, "jerk"=20.08558877435007, "heading"=-5.992773825330433}, {"dt"=0.005, "x"=83.44396456337789, "y"=257.11137099762857, "position"=-83.90942123948291, "velocity"=-71.19666322100882, "acceleration"=-12.403551577725125, "jerk"=20.83009722070983, "heading"=-5.988774999975715}, {"dt"=0.005, "x"=83.7847169241049, "y"=257.0072994024275, "position"=-84.26571194700799, "velocity"=-71.25814150501563, "acceleration"=-12.295656801362043, "jerk"=21.57895527261644, "heading"=-5.984754217898294}, {"dt"=0.005, "x"=84.12533788847425, "y"=256.90176470692546, "position"=-84.6223072544962, "velocity"=-71.319061497644, "acceleration"=-12.183998525674156, "jerk"=22.3316551375774, "heading"=-5.98071167849446}, {"dt"=0.005, "x"=84.46581612272904, "y"=256.7947597726932, "position"=-84.97920427599023, "velocity"=-71.37940429880433, "acceleration"=-12.068560232066261, "jerk"=23.08765872157892, "heading"=-5.976647587911389}, {"dt"=0.005, "x"=84.80614013330172, "y"=256.6862776312975, "position"=-85.33640003068795, "velocity"=-71.43915093954497, "acceleration"=-11.949328148128302, "jerk"=23.846416787591806, "heading"=-5.972562159072042}, {"dt"=0.005, "x"=85.14629826897027, "y"=256.57631148933046, "position"=-85.69389144266958, "velocity"=-71.49828239632555, "acceleration"=-11.826291356115348, "jerk"=24.607358402590762, "heading"=-5.968455611695016}, {"dt"=0.005, "x"=85.48627872318788, "y"=256.46485473341727, "position"=-86.05167534069841, "velocity"=-71.55677960576651, "acceleration"=-11.699441888191586, "jerk"=25.36989358475239, "heading"=-5.96432817230919}, {"dt"=0.005, "x"=85.82606953260233, "y"=256.351900936532, "position"=-86.40974845389364, "velocity"=-71.61462263904757, "acceleration"=-11.568606656211955, "jerk"=26.167046395926263, "heading"=-5.960180074311807}, {"dt"=0.005, "x"=86.16565858912016, "y"=256.2374438598533, "position"=-86.76810742156223, "velocity"=-71.67179353371966, "acceleration"=-11.434178934419492, "jerk"=26.885544358492552, "heading"=-5.956011557858135}, {"dt"=0.005, "x"=86.50503363670202, "y"=256.12147745963335, "position"=-87.12674878685793, "velocity"=-71.72827305913928, "acceleration"=-11.295905083923685, "jerk"=27.654770099161397, "heading"=-5.951822869932884}, {"dt"=0.005, "x"=86.8441822741406, "y"=256.00399589216437, "position"=-87.48566899661411, "velocity"=-71.78404195123524, "acceleration"=-11.153778419190985, "jerk"=28.42533294654004, "heading"=-5.947614264346094}, {"dt"=0.005, "x"=87.18309195919339, "y"=255.88499351828264, "position"=-87.84486440250353, "velocity"=-71.83908117788349, "acceleration"=-11.007845329649513, "jerk"=29.186617908294465, "heading"=-5.943386001708555}, {"dt"=0.005, "x"=87.52175001198465, "y"=255.76446490811276, "position"=-88.20433126132345, "velocity"=-71.89337176398163, "acceleration"=-10.858117219629548, "jerk"=29.945622003992867, "heading"=-5.9391383494123104}, {"dt"=0.005, "x"=87.86014361858895, "y"=255.64240484574248, "position"=-88.56406573536854, "velocity"=-71.94689480901924, "acceleration"=-10.704609007521526, "jerk"=30.701642421604447, "heading"=-5.934871581605034}, {"dt"=0.005, "x"=88.19825983479609, "y"=255.51880833382148, "position"=-88.92406389289337, "velocity"=-71.9996315049654, "acceleration"=-10.547339189230343, "jerk"=31.453963658236717, "heading"=-5.9305859791581845}, {"dt"=0.005, "x"=88.53608559005689, "y"=255.3936705980768, "position"=-89.2843217086654, "velocity"=-72.05156315440591, "acceleration"=-10.386329888103774, "jerk"=32.201860225313794, "heading"=-5.926281829628833}, {"dt"=0.005, "x"=88.87360769160958, "y"=255.26698709173667, "position"=-89.64483506461103, "velocity"=-72.10267118912475, "acceleration"=-10.22160694376737, "jerk"=32.9445888672808, "heading"=-5.921959427215067}, {"dt"=0.005, "x"=89.2108128287856, "y"=255.13875349985622, "position"=-90.00559975055529, "velocity"=-72.15293718885303, "acceleration"=-10.053199945656388, "jerk"=33.681399622196295, "heading"=-5.917619072704923}, {"dt"=0.005, "x"=89.5476875635424, "y"=255.00896574894676, "position"=-90.36661145009367, "velocity"=-72.20233990767704, "acceleration"=-9.880543764802496, "jerk"=34.53123617077836, "heading"=-5.913261073599663}, {"dt"=0.005, "x"=89.88421836165021, "y"=254.8776200010133, "position"=-90.72786576989523, "velocity"=-72.25086396031128, "acceleration"=-9.70481052684704, "jerk"=35.146647591091096, "heading"=-5.908885743708284}, {"dt"=0.005, "x"=90.22039159640812, "y"=254.74471265766985, "position"=-91.08935823964005, "velocity"=-72.29849394896367, "acceleration"=-9.525997730477798, "jerk"=35.76255927384864, "heading"=-5.904493403087157}, {"dt"=0.005, "x"=90.55619353161921, "y"=254.61024037258215, "position"=-91.4510842895013, "velocity"=-72.34520997224976, "acceleration"=-9.343204657218962, "jerk"=36.55861465176713, "heading"=-5.900084378248678}, {"dt"=0.005, "x"=90.89161033730889, "y"=254.4742000511529, "position"=-91.81303926265906, "velocity"=-72.39099463155311, "acceleration"=-9.15693186067017, "jerk"=37.254559309758406, "heading"=-5.895659001940866}, {"dt"=0.005, "x"=91.22662809506568, "y"=254.3365888540998, "position"=-92.17521841662402, "velocity"=-72.43583079299192, "acceleration"=-8.967232287761817, "jerk"=37.939914581670564, "heading"=-5.891217613056247}, {"dt"=0.005, "x"=91.56123280292532, "y"=254.19740420114178, "position"=-92.53761692398972, "velocity"=-72.47970147313798, "acceleration"=-8.774136029211377, "jerk"=38.619251710088065, "heading"=-5.886760556542263}, {"dt"=0.005, "x"=91.8954103278018, "y"=254.05664379684669, "position"=-92.9002298161349, "velocity"=-72.52257842903516, "acceleration"=-8.57539117943702, "jerk"=39.74896995487143, "heading"=-5.882288184010929}, {"dt"=0.005, "x"=92.22914656617264, "y"=253.91430556870074, "position"=-93.26305215281451, "velocity"=-72.5644673359213, "acceleration"=-8.377781377225801, "jerk"=39.52196044224365, "heading"=-5.877800851557132}, {"dt"=0.005, "x"=92.56242730179656, "y"=253.77038773177736, "position"=-93.6260788632956, "velocity"=-72.60534209621842, "acceleration"=-8.174952059425777, "jerk"=40.5658635600048, "heading"=-5.8732989216162235}, {"dt"=0.005, "x"=92.89523825902431, "y"=253.62488877198115, "position"=-93.98930479925369, "velocity"=-72.64518719161825, "acceleration"=-7.969019079965278, "jerk"=41.18659589209983, "heading"=-5.868782762212121}, {"dt"=0.005, "x"=93.22756508037864, "y"=253.47780746138432, "position"=-94.35272470531052, "velocity"=-72.68398121136558, "acceleration"=-7.758803949465687, "jerk"=42.04302609991828, "heading"=-5.8642527472177575}, {"dt"=0.005, "x"=93.55939335556087, "y"=253.32914285118977, "position"=-94.71633324554949, "velocity"=-72.721708047793, "acceleration"=-7.545367285484872, "jerk"=42.68733279616299, "heading"=-5.859709255915605}, {"dt"=0.005, "x"=93.89070871992597, "y"=253.17889423213063, "position"=-95.08012510663706, "velocity"=-72.75837221751335, "acceleration"=-7.332833944070671, "jerk"=42.50666828284011, "heading"=-5.855152671587654}, {"dt"=0.005, "x"=94.22149672316192, "y"=253.0270611977874, "position"=-95.4440948490645, "velocity"=-72.79394848548992, "acceleration"=-7.11525359531322, "jerk"=43.51606975149025, "heading"=-5.85058338324868}, {"dt"=0.005, "x"=94.55174281105394, "y"=252.87364365946075, "position"=-95.8082368812912, "velocity"=-72.8284064453396, "acceleration"=-6.891591969935007, "jerk"=44.73232507564262, "heading"=-5.846001785852594}, {"dt"=0.005, "x"=94.88143250811424, "y"=252.71864176675143, "position"=-96.17254565567247, "velocity"=-72.86175487625493, "acceleration"=-6.6696861830678245, "jerk"=44.38115737343651, "heading"=-5.841408277698225}, {"dt"=0.005, "x"=95.21055134347274, "y"=252.56205594493233, "position"=-96.53701558225421, "velocity"=-72.8939853163484, "acceleration"=-6.44608801869424, "jerk"=44.71963287471681, "heading"=-5.836803261367771}, {"dt"=0.005, "x"=95.53908471538045, "y"=252.40388696457833, "position"=-96.9016408732082, "velocity"=-72.92505819079507, "acceleration"=-6.21457488933288, "jerk"=46.302625872272074, "heading"=-5.832187145554138}, {"dt"=0.005, "x"=95.86701810799066, "y"=252.24413584327448, "position"=-97.26641577742541, "velocity"=-72.95498084344301, "acceleration"=-5.984530529588028, "jerk"=46.00887194897041, "heading"=-5.827560341953144}, {"dt"=0.005, "x"=96.194337078454, "y"=252.08280385382457, "position"=-97.6313345618762, "velocity"=-72.98375689015855, "acceleration"=-5.755209343107026, "jerk"=45.86423729620037, "heading"=-5.822923265338563}, {"dt"=0.005, "x"=96.52102696577535, "y"=251.91989267246552, "position"=-97.99639118144341, "velocity"=-73.0113239134418, "acceleration"=-5.513404656650778, "jerk"=48.360937291249684, "heading"=-5.818276337606002}, {"dt"=0.005, "x"=96.84707342074924, "y"=251.75540412066286, "position"=-98.36157986483212, "velocity"=-73.03773667774185, "acceleration"=-5.2825528600095595, "jerk"=46.17035932824365, "heading"=-5.813619980165323}, {"dt"=0.005, "x"=97.17246191733855, "y"=251.58934041121125, "position"=-98.72689456383762, "velocity"=-73.06293980110033, "acceleration"=-5.040624671696037, "jerk"=48.38563766270454, "heading"=-5.80895462078329}, {"dt"=0.005, "x"=97.49717802663415, "y"=251.42170401561233, "position"=-99.09232925398821, "velocity"=-73.08693803012, "acceleration"=-4.799645803933572, "jerk"=48.19577355249294, "heading"=-5.804280689592593}, {"dt"=0.005, "x"=97.8212074124183, "y"=251.25249766802122, "position"=-99.45787792505239, "velocity"=-73.10973421283475, "acceleration"=-4.559236542951339, "jerk"=48.08185219644656, "heading"=-5.799598619037334}, {"dt"=0.005, "x"=98.14453566319625, "y"=251.08172445621327, "position"=-99.82353438625925, "velocity"=-73.13129224137424, "acceleration"=-4.31160570789757, "jerk"=49.52616701075385, "heading"=-5.794908846195476}, {"dt"=0.005, "x"=98.46714858565576, "y"=250.9093876707493, "position"=-100.18929259240359, "velocity"=-73.15164122886559, "acceleration"=-4.069797498269168, "jerk"=48.36164192568049, "heading"=-5.790211808424604}, {"dt"=0.005, "x"=98.78903190124835, "y"=250.73549096781838, "position"=-100.55514629560628, "velocity"=-73.17074064053894, "acceleration"=-3.8198823346704103, "jerk"=49.98303271975146, "heading"=-5.785507947649204}, {"dt"=0.005, "x"=99.11017149390067, "y"=250.56003824034698, "position"=-100.92108932060614, "velocity"=-73.18860499997157, "acceleration"=-3.572871886527196, "jerk"=49.4020896286429, "heading"=-5.7807977066471015}, {"dt"=0.005, "x"=99.43055335298814, "y"=250.38303364936624, "position"=-101.28711549570924, "velocity"=-73.20523502062068, "acceleration"=-3.3260041298206033, "jerk"=49.37355134131849, "heading"=-5.776081529749057}, {"dt"=0.005, "x"=99.75016335394339, "y"=250.20448174866908, "position"=-101.65321839648058, "velocity"=-73.2205801542663, "acceleration"=-3.0690267291248574, "jerk"=51.395480139149186, "heading"=-5.771359865959071}, {"dt"=0.005, "x"=100.06898779210653, "y"=250.02438718983282, "position"=-102.01939195163233, "velocity"=-73.23471103034808, "acceleration"=-2.826175216355864, "jerk"=48.57030255379868, "heading"=-5.766633160955895}, {"dt"=0.005, "x"=100.38701277944482, "y"=249.84275506028584, "position"=-102.38562974740891, "velocity"=-73.24755915531712, "acceleration"=-2.5696249938079063, "jerk"=51.310044509591535, "heading"=-5.761901865874054}, {"dt"=0.005, "x"=100.70422461047941, "y"=249.65959068133387, "position"=-102.75192544143927, "velocity"=-73.25913880607219, "acceleration"=-2.31593015101339, "jerk"=50.73896855890325, "heading"=-5.757166431777991}, {"dt"=0.005, "x"=101.02060982879536, "y"=249.47489956814115, "position"=-103.11827283621804, "velocity"=-73.26947895575367, "acceleration"=-2.0680299362965116, "jerk"=49.5800429433757, "heading"=-5.752427308515466}, {"dt"=0.005, "x"=101.33615498128633, "y"=249.28868757238558, "position"=-103.48466559081865, "velocity"=-73.2785509201217, "acceleration"=-1.8143928736066073, "jerk"=50.727412537980854, "heading"=-5.747684948252241}, {"dt"=0.005, "x"=101.65084660521062, "y"=249.10096089467888, "position"=-103.85109719929547, "velocity"=-73.28632169536257, "acceleration"=-1.554155048174266, "jerk"=52.04756508646824, "heading"=-5.742939805564259}, {"dt"=0.005, "x"=101.96467164213844, "y"=248.91172583874854, "position"=-104.21756146794345, "velocity"=-73.2928537295987, "acceleration"=-1.3064068472260715, "jerk"=49.54964018963892, "heading"=-5.738192331064355}, {"dt"=0.005, "x"=102.2776170628096, "y"=248.72098903302194, "position"=-104.5840520754327, "velocity"=-73.29812149784846, "acceleration"=-1.053553649950345, "jerk"=50.57063945514528, "heading"=-5.733442976902621}, {"dt"=0.005, "x"=102.58966996735482, "y"=248.52875737238338, "position"=-104.95056268453831, "velocity"=-73.30212182112285, "acceleration"=-0.8000646548794066, "jerk"=50.697799014187694, "heading"=-5.728692195128212}, {"dt"=0.005, "x"=102.9008176105834, "y"=248.3350380029084, "position"=-105.31708696749442, "velocity"=-73.30485659122118, "acceleration"=-0.5469540196656908, "jerk"=50.62212704274316, "heading"=-5.7239404371684195}, {"dt"=0.005, "x"=103.21104740844874, "y"=248.1398383174778, "position"=-105.68361860961521, "velocity"=-73.30632842415945, "acceleration"=-0.2943665876529167, "jerk"=50.51748640255482, "heading"=-5.719188153589799}, {"dt"=0.005, "x"=103.52034694438433, "y"=247.9431659511817, "position"=-106.05015131292349, "velocity"=-73.30654066165737, "acceleration"=-0.04244749958388638, "jerk"=50.38381761380606, "heading"=-5.714435793860156}, {"dt"=0.005, "x"=103.82870397550187, "y"=247.7450287765186, "position"=-106.41667879978237, "velocity"=-73.3054973717779, "acceleration"=0.208657975892379, "jerk"=50.22109509525308, "heading"=-5.709683806111728}, {"dt"=0.005, "x"=104.13610643864372, "y"=247.54543489839563, "position"=-106.78319481652632, "velocity"=-73.30320334879006, "acceleration"=0.45880459756801883, "jerk"=50.02932433512797, "heading"=-5.704932636905834}, {"dt"=0.005, "x"=104.44254245628238, "y"=247.3443926489366, "position"=-107.14969313708698, "velocity"=-73.29966411213209, "acceleration"=0.7078473315942801, "jerk"=49.80854680525226, "heading"=-5.700182730999352}, {"dt"=0.005, "x"=104.74800034225893, "y"=247.14191058210417, "position"=-107.5161675666097, "velocity"=-73.29488590454231, "acceleration"=0.9556415179559963, "jerk"=49.558837272343226, "heading"=-5.695434531113294}, {"dt"=0.005, "x"=105.05246860735357, "y"=246.93799746814383, "position"=-107.88261194505579, "velocity"=-73.28887568921857, "acceleration"=1.2020430647481817, "jerk"=49.28030935843708, "heading"=-5.690688477703819}, {"dt"=0.005, "x"=105.35593596468235, "y"=246.7326622878559, "position"=-108.24902015078811, "velocity"=-73.28164114646593, "acceleration"=1.446908550528292, "jerk"=48.97309715602205, "heading"=-5.685945008735936}, {"dt"=0.005, "x"=105.65839133491241, "y"=246.5259142267045, "position"=-108.61538610413378, "velocity"=-73.27319066913202, "acceleration"=1.6900954667818269, "jerk"=48.63738325070699, "heading"=-5.681204559460232}, {"dt"=0.005, "x"=105.95982385129084, "y"=246.31776266876997, "position"=-108.98170377092148, "velocity"=-73.26353335754303, "acceleration"=1.9314623177990597, "jerk"=48.273370203446575, "heading"=-5.676467562192888}, {"dt"=0.005, "x"=106.26022275316862, "y"=246.10821726859297, "position"=-109.34796703004629, "velocity"=-73.25265182496004, "acceleration"=2.1763065165970374, "jerk"=48.96883975959554, "heading"=-5.671734447855372}, {"dt"=0.005, "x"=106.55957756848557, "y"=245.8972878228348, "position"=-109.71416989259829, "velocity"=-73.24057251040155, "acceleration"=2.415862911698241, "jerk"=47.91127902024073, "heading"=-5.667005642971311}, {"dt"=0.005, "x"=106.85787821103581, "y"=245.68498419509086, "position"=-110.08030662074658, "velocity"=-73.22734562965688, "acceleration"=2.6453761489335648, "jerk"=45.90264744706474, "heading"=-5.662281567972211}, {"dt"=0.005, "x"=107.15511461922641, "y"=245.47131656764438, "position"=-110.44637128357633, "velocity"=-73.2129325659498, "acceleration"=2.882612741416324, "jerk"=47.447318496551816, "heading"=-5.6575626427712296}, {"dt"=0.005, "x"=107.45127685136525, "y"=245.25629537554272, "position"=-110.81235786912049, "velocity"=-73.1973171088337, "acceleration"=3.1230914232196483, "jerk"=48.09573636066489, "heading"=-5.652849285149673}, {"dt"=0.005, "x"=107.74635565603074, "y"=245.03993088649938, "position"=-111.17826098892381, "velocity"=-73.18062396066419, "acceleration"=3.3386296339017463, "jerk"=43.1076421364196, "heading"=-5.648141901534325}, {"dt"=0.005, "x"=108.0403413796742, "y"=244.8222339932066, "position"=-111.54407452483453, "velocity"=-73.16270718214226, "acceleration"=3.583355704387259, "jerk"=48.94521409710251, "heading"=-5.643440904268049}, {"dt"=0.005, "x"=108.33322528279129, "y"=244.60321524329493, "position"=-111.90979326036495, "velocity"=-73.14374710608396, "acceleration"=3.792015211658395, "jerk"=41.73190145422723, "heading"=-5.63874669047986}, {"dt"=0.005, "x"=108.62499820292103, "y"=244.3828858247605, "position"=-112.27541121615043, "velocity"=-73.12359115709612, "acceleration"=4.031189797569823, "jerk"=47.83491718228561, "heading"=-5.634059663334965}, {"dt"=0.005, "x"=108.91565189795271, "y"=244.1612565565287, "position"=-112.64092332671933, "velocity"=-73.10242211377921, "acceleration"=4.2338086633805005, "jerk"=40.52377316213551, "heading"=-5.6293802103784625}, {"dt"=0.005, "x"=109.20517764521, "y"=243.93833894246382, "position"=-113.00632368384187, "velocity"=-73.08007142450715, "acceleration"=4.47013785441186, "jerk"=47.26583820627184, "heading"=-5.624708725920152}, {"dt"=0.005, "x"=109.4935676163091, "y"=243.71414411945892, "position"=-113.37160726421845, "velocity"=-73.0567160753154, "acceleration"=4.67106983834924, "jerk"=40.18639678747604, "heading"=-5.620045588785963}, {"dt"=0.005, "x"=109.78081397548897, "y"=243.48868353924286, "position"=-113.73676879572672, "velocity"=-73.03230630165216, "acceleration"=4.881954732650229, "jerk"=42.17697886019778, "heading"=-5.615391176713777}, {"dt"=0.005, "x"=110.0669088838996, "y"=243.2619689692467, "position"=-114.1018027569783, "velocity"=-73.00679225031769, "acceleration"=5.102810266893698, "jerk"=44.17110684869385, "heading"=-5.61074586621205}, {"dt"=0.005, "x"=110.3518451433545, "y"=243.03401197929767, "position"=-114.46670419739581, "velocity"=-72.98028808350153, "acceleration"=5.300833363230595, "jerk"=39.60461926737935, "heading"=-5.606110022003944}, {"dt"=0.005, "x"=110.63561569646534, "y"=242.80482432685497, "position"=-114.83146810301838, "velocity"=-72.95278112451379, "acceleration"=5.501391797548649, "jerk"=40.111686863610885, "heading"=-5.601484005010324}, {"dt"=0.005, "x"=110.91821368162786, "y"=242.57441791042842, "position"=-115.19608946545954, "velocity"=-72.92427248823041, "acceleration"=5.701727256675326, "jerk"=40.06709182533541, "heading"=-5.596868171361825}, {"dt"=0.005, "x"=111.19963249685956, "y"=242.3428047130829, "position"=-115.5605633640463, "velocity"=-72.89477971735208, "acceleration"=5.898554175666959, "jerk"=39.36538379832655, "heading"=-5.592262871257847}, {"dt"=0.005, "x"=111.47983926670526, "y"=242.11001894209824, "position"=-115.92485040614399, "velocity"=-72.85740841953681, "acceleration"=7.47425956305392, "jerk"=315.1410774773922, "heading"=-5.587668884272488}, {"dt"=0.005, "x"=111.75874786687193, "y"=241.87614078350774, "position"=-116.2888407910618, "velocity"=-72.79807698356215, "acceleration"=11.866287194931147, "jerk"=878.4055263754453, "heading"=-5.583087866632939}, {"dt"=0.005, "x"=112.03624640150584, "y"=241.6412751396369, "position"=-116.6523890098648, "velocity"=-72.70964376059977, "acceleration"=17.686644592475886, "jerk"=1164.071479508948, "heading"=-5.578521906190406}, {"dt"=0.005, "x"=112.31222512270095, "y"=241.40552871631846, "position"=-117.01534993153534, "velocity"=-72.59218433410719, "acceleration"=23.491885298517445, "jerk"=1161.0481412083118, "heading"=-5.5739730649440276}, {"dt"=0.005, "x"=112.58657645192201, "y"=241.16900995764027, "position"=-117.37757883023343, "velocity"=-72.44577973961884, "acceleration"=29.28091889766904, "jerk"=1157.8067198303188, "heading"=-5.569443377687035}, {"dt"=0.005, "x"=112.85919499846916, "y"=240.93182897768858, "position"=-117.73893141313872, "velocity"=-72.27051658105782, "acceleration"=35.05263171220463, "jerk"=1154.342562907118, "heading"=-5.564934850715913}, {"dt"=0.005, "x"=113.1299771429194, "y"=240.69409787047957, "position"=-118.0992632728013, "velocity"=-72.06637193251603, "acceleration"=40.82892970835701, "jerk"=1155.259599230476, "heading"=-5.560449467768328}, {"dt"=0.005, "x"=113.39882216250689, "y"=240.45592966305333, "position"=-118.45843139441793, "velocity"=-71.83362432332811, "acceleration"=46.54952183758496, "jerk"=1144.1184258455905, "heading"=-5.555989170446278}, {"dt"=0.005, "x"=113.6656307567467, "y"=240.2174395444283, "position"=-118.81629220904004, "velocity"=-71.57216292442345, "acceleration"=52.292279780931494, "jerk"=1148.5515886693065, "heading"=-5.55155588172029}, {"dt"=0.005, "x"=113.9303063955144, "y"=239.97874360378586, "position"=-119.17270341233797, "velocity"=-71.28224065958396, "acceleration"=57.98445296789794, "jerk"=1138.4346373932885, "heading"=-5.547151482680746}, {"dt"=0.005, "x"=114.19275429810547, "y"=239.7399596644467, "position"=-119.52752262159922, "velocity"=-70.9638418522488, "acceleration"=63.679761467031426, "jerk"=1139.0616998266978, "heading"=-5.542777828624852}, {"dt"=0.005, "x"=114.4528818655155, "y"=239.5012068226167, "position"=-119.88060798069608, "velocity"=-70.61707181937253, "acceleration"=69.35400657525577, "jerk"=1134.8490216448681, "heading"=-5.5384367410519815}, {"dt"=0.005, "x"=114.71059867792447, "y"=239.2626053651942, "position"=-120.23181818966272, "velocity"=-70.24204179332621, "acceleration"=75.00600520926355, "jerk"=1130.3997268015564, "heading"=-5.534130006898206}, {"dt"=0.005, "x"=114.96581648948961, "y"=239.02427668574995, "position"=-120.58101253495734, "velocity"=-69.83886905892338, "acceleration"=80.63454688056595, "jerk"=1125.7083342604801, "heading"=-5.529859377848392}, {"dt"=0.005, "x"=115.2184492205032, "y"=238.78634319882846, "position"=-120.9280509204106, "velocity"=-69.4076770906519, "acceleration"=86.23839365429546, "jerk"=1120.769354745903, "heading"=-5.525626569726361}, {"dt"=0.005, "x"=115.46843696857354, "y"=238.54890534110615, "position"=-121.27282709485576, "velocity"=-68.9552348890323, "acceleration"=90.48844032392083, "jerk"=850.0093339250725, "heading"=-5.521432858738992}, {"dt"=0.005, "x"=115.71577279329364, "y"=238.31201475363008, "position"=-121.61530652580706, "velocity"=-68.49588619026024, "acceleration"=91.8697397544122, "jerk"=276.25988609827345, "heading"=-5.517278628273556}, {"dt"=0.005, "x"=115.96047542164747, "y"=238.07569862916742, "position"=-121.95548983963113, "velocity"=-68.03666276481438, "acceleration"=91.84468508917121, "jerk"=-5.01093304819733, "heading"=-5.513163822743499}, {"dt"=0.005, "x"=116.20256380879272, "y"=237.83998355504949, "position"=-122.29337796217617, "velocity"=-67.5776245090071, "acceleration"=91.80765116145722, "jerk"=-7.406785542798389, "heading"=-5.509088373742463}, {"dt"=0.005, "x"=116.44205712604376, "y"=237.60489551035315, "position"=-122.62897211851245, "velocity"=-67.11883126725576, "acceleration"=91.75864835026744, "jerk"=-9.800562237956001, "heading"=-5.505052200442722}, {"dt"=0.005, "x"=116.6789744382874, "y"=237.37046017230386, "position"=-122.96227339448815, "velocity"=-66.66025519513943, "acceleration"=91.71521442326593, "jerk"=-8.686785400300323, "heading"=-5.501055215236881}, {"dt"=0.005, "x"=116.91333511186019, "y"=237.1367025066028, "position"=-123.29328332121469, "velocity"=-66.20198534530633, "acceleration"=91.65396996662025, "jerk"=-12.248891329136313, "heading"=-5.497097317069667}, {"dt"=0.005, "x"=117.14515833257082, "y"=236.90364723661017, "position"=-123.62200320885762, "velocity"=-65.74397752858751, "acceleration"=91.60156334376381, "jerk"=-10.481324571287587, "heading"=-5.493178399776215}, {"dt"=0.005, "x"=117.37446366129055, "y"=236.67131828007808, "position"=-123.94843494417536, "velocity"=-65.28634706354846, "acceleration"=91.5260930078091, "jerk"=-15.09406719094386, "heading"=-5.489298342901389}, {"dt"=0.005, "x"=117.60127049671337, "y"=236.43973927987852, "position"=-124.27258024173179, "velocity"=-64.82905951128458, "acceleration"=91.45751045277564, "jerk"=-13.71651100669169, "heading"=-5.485457020980899}, {"dt"=0.005, "x"=117.82559837592802, "y"=236.20893329485338, "position"=-124.5944410814069, "velocity"=-64.3721679350234, "acceleration"=91.37831525223703, "jerk"=-15.839040107721303, "heading"=-5.4816542986619865}, {"dt"=0.005, "x"=118.04746644178955, "y"=235.9789233436574, "position"=-124.91401895344798, "velocity"=-63.91557440821657, "acceleration"=91.31870536136546, "jerk"=-11.921978174314063, "heading"=-5.4778900399363515}, {"dt"=0.005, "x"=118.26689471291319, "y"=235.74973108376057, "position"=-125.2313166971603, "velocity"=-63.459548742464555, "acceleration"=91.20513315040313, "jerk"=-22.714442192466322, "heading"=-5.474164086793973}, {"dt"=0.005, "x"=118.48390214888434, "y"=235.5213788160058, "position"=-125.5463357211184, "velocity"=-63.00380479162051, "acceleration"=91.14879016880906, "jerk"=-11.268596318814161, "heading"=-5.470476292252356}, {"dt"=0.005, "x"=118.69850859604284, "y"=235.2938874508813, "position"=-125.85907882394915, "velocity"=-62.54862056615055, "acceleration"=91.03684509399272, "jerk"=-22.389014963266618, "heading"=-5.466826487516799}, {"dt"=0.005, "x"=118.91073346089941, "y"=235.06727789115496, "position"=-126.16954828431966, "velocity"=-62.09389207410146, "acceleration"=90.94569840981706, "jerk"=-18.229336835133836, "heading"=-5.463214504699889}, {"dt"=0.005, "x"=119.12059622447292, "y"=234.8415704892323, "position"=-126.47774661464834, "velocity"=-61.63966606573506, "acceleration"=90.84520167328094, "jerk"=-20.09934730722307, "heading"=-5.459640168274068}, {"dt"=0.005, "x"=119.32811601069392, "y"=234.61678550903116, "position"=-126.78367593491242, "velocity"=-61.18586405281552, "acceleration"=90.76040258390776, "jerk"=-16.95981787463552, "heading"=-5.456103302609979}, {"dt"=0.005, "x"=119.53331251459826, "y"=234.39294211925923, "position"=-127.08733934785371, "velocity"=-60.7326825882586, "acceleration"=90.63629291138398, "jerk"=-24.821934504757337, "heading"=-5.452603716342383}, {"dt"=0.005, "x"=119.73620474859345, "y"=234.17005974937646, "position"=-127.38873909805288, "velocity"=-60.279950039832144, "acceleration"=90.54650968529074, "jerk"=-17.956645218646372, "heading"=-5.449141223918887}, {"dt"=0.005, "x"=119.93681217106922, "y"=233.9481568588428, "position"=-127.6878782475796, "velocity"=-59.82782990534417, "acceleration"=90.42402689759541, "jerk"=-24.496557539066544, "heading"=-5.445715626532774}, {"dt"=0.005, "x"=120.13515384725147, "y"=233.72725185391013, "position"=-127.98475943882467, "velocity"=-59.37623824901148, "acceleration"=90.31833126653765, "jerk"=-21.13912621155123, "heading"=-5.442326726612822}, {"dt"=0.005, "x"=120.33124886609893, "y"=233.5073626295884, "position"=-128.2793855194584, "velocity"=-58.925216126745674, "acceleration"=90.20442445316093, "jerk"=-22.781362675345918, "heading"=-5.43897432088119}, {"dt"=0.005, "x"=120.52511633391221, "y"=233.28850657216367, "position"=-128.57175954181304, "velocity"=-58.47480447092923, "acceleration"=90.0823311632891, "jerk"=-24.418657974365487, "heading"=-5.435658200625364}, {"dt"=0.005, "x"=120.71677492086116, "y"=233.0707010718924, "position"=-128.86188408386298, "velocity"=-58.02490840998908, "acceleration"=89.97921218802958, "jerk"=-20.623795051903926, "heading"=-5.432378159620651}, {"dt"=0.005, "x"=120.90624375910843, "y"=232.85396250500835, "position"=-129.14976261213786, "velocity"=-57.575705654978435, "acceleration"=89.84055100212913, "jerk"=-27.732237180089214, "heading"=-5.429133978923922}, {"dt"=0.005, "x"=121.09354118901648, "y"=232.63830766122996, "position"=-129.4353975870538, "velocity"=-57.12699498319239, "acceleration"=89.74213435720912, "jerk"=-19.68332898400149, "heading"=-5.4259254484911}, {"dt"=0.005, "x"=121.27868611301409, "y"=232.42375219591588, "position"=-129.71879252451427, "velocity"=-56.67898749209338, "acceleration"=89.60149821980252, "jerk"=-28.12722748132046, "heading"=-5.422752344150146}, {"dt"=0.005, "x"=121.46169697089529, "y"=232.21031180473224, "position"=-129.9999504422243, "velocity"=-56.231583542005126, "acceleration"=89.48079001765024, "jerk"=-24.1416404304573, "heading"=-5.4196144452989365}, {"dt"=0.005, "x"=121.64259218222409, "y"=231.99800171673797, "position"=-130.27887453753667, "velocity"=-55.784819062474774, "acceleration"=89.35289590607027, "jerk"=-25.57882231599251, "heading"=-5.4165115274752305}, {"dt"=0.005, "x"=121.82138978902364, "y"=231.78683711532472, "position"=-130.55556764024664, "velocity"=-55.33862054199273, "acceleration"=89.23970409640845, "jerk"=-22.63836193236557, "heading"=-5.413443368629285}, {"dt"=0.005, "x"=121.99810811534833, "y"=231.5768323628198, "position"=-130.8300332354196, "velocity"=-54.89311903459299, "acceleration"=89.10030147994803, "jerk"=-27.880523292083126, "heading"=-5.410409737947433}, {"dt"=0.005, "x"=122.1727650706547, "y"=231.36800182271818, "position"=-131.1022743904936, "velocity"=-54.448231014799966, "acceleration"=88.9776039586053, "jerk"=-24.539504268545898, "heading"=-5.4074104079406}, {"dt"=0.005, "x"=122.34537865144482, "y"=231.16035926671202, "position"=-131.37229453666413, "velocity"=-54.00402923410722, "acceleration"=88.84035613854877, "jerk"=-27.449564011305938, "heading"=-5.404445145967095}, {"dt"=0.005, "x"=122.51596645732069, "y"=230.95391845621535, "position"=-131.64009671692423, "velocity"=-53.56043605202119, "acceleration"=88.71863641720665, "jerk"=-24.343944268423456, "heading"=-5.40151372267339}, {"dt"=0.005, "x"=122.68454604000789, "y"=230.74869272790963, "position"=-131.9056841323972, "velocity"=-53.11748309459103, "acceleration"=88.59059148603166, "jerk"=-25.60898623499952, "heading"=-5.398615906126887}, {"dt"=0.005, "x"=122.85113489991319, "y"=230.5446949971176, "position"=-132.16906014195928, "velocity"=-52.67520191241584, "acceleration"=88.4562364350387, "jerk"=-26.871010198590284, "heading"=-5.395751461995211}, {"dt"=0.005, "x"=123.01575048282338, "y"=230.34193776126313, "position"=-132.43022826181354, "velocity"=-52.2336239708519, "acceleration"=88.31558831278699, "jerk"=-28.129624450343726, "heading"=-5.39292015372012}, {"dt"=0.005, "x"=123.17840959996867, "y"=230.14043381997186, "position"=-132.6891912451652, "velocity"=-51.792596670335165, "acceleration"=88.20546010334738, "jerk"=-22.025641887921665, "heading"=-5.390121752610247}, {"dt"=0.005, "x"=123.33912965939992, "y"=229.94019475675287, "position"=-132.9459530412767, "velocity"=-51.3523592222984, "acceleration"=88.04748960735225, "jerk"=-31.594099199026004, "heading"=-5.387356016771849}, {"dt"=0.005, "x"=123.49792707789881, "y"=229.7412329110977, "position"=-133.20051626750632, "velocity"=-50.91264524591942, "acceleration"=87.94279527579647, "jerk"=-20.93886631115538, "heading"=-5.384622718540851}, {"dt"=0.005, "x"=123.65481875355499, "y"=229.54355955067467, "position"=-133.45288456050514, "velocity"=-50.47365859976536, "acceleration"=87.7973292308127, "jerk"=-29.093208996755493, "heading"=-5.381921619250733}, {"dt"=0.005, "x"=123.80982125421392, "y"=229.34718588342855, "position"=-133.70306128284, "velocity"=-50.0353444669705, "acceleration"=87.66282655897157, "jerk"=-26.900534368223816, "heading"=-5.379252483299963}, {"dt"=0.005, "x"=123.9629508090095, "y"=229.1521230779733, "position"=-133.95104950559255, "velocity"=-49.597644550509344, "acceleration"=87.53998329223123, "jerk"=-24.568653348069347, "heading"=-5.376615078401357}, {"dt"=0.005, "x"=124.11422358265469, "y"=228.95838192118046, "position"=-134.19685245081848, "velocity"=-49.16058904518384, "acceleration"=87.41110106510064, "jerk"=-25.77644542611779, "heading"=-5.3740091709566045}, {"dt"=0.005, "x"=124.26365599593498, "y"=228.7659724048062, "position"=-134.44047401827535, "velocity"=-48.724313491376115, "acceleration"=87.25511076154504, "jerk"=-31.198060711119524, "heading"=-5.371434520626398}, {"dt"=0.005, "x"=124.41126326876554, "y"=228.57490560594835, "position"=-134.68191641019993, "velocity"=-48.288478384916736, "acceleration"=87.16702129187581, "jerk"=-17.617893933845608, "heading"=-5.36889090552446}, {"dt"=0.005, "x"=124.55706162487414, "y"=228.38519084998615, "position"=-134.92118372780467, "velocity"=-47.85346352094781, "acceleration"=87.00297279378475, "jerk"=-32.80969961821256, "heading"=-5.366378084319444}, {"dt"=0.005, "x"=124.7010664659048, "y"=228.19683806937468, "position"=-135.15827899179016, "velocity"=-47.41905279709345, "acceleration"=86.88214477087257, "jerk"=-24.165604582435662, "heading"=-5.363895827781472}, {"dt"=0.005, "x"=124.8432931101716, "y"=228.009856856189, "position"=-135.3932053471098, "velocity"=-46.98527106393293, "acceleration"=86.75634663210445, "jerk"=-25.15962775362368, "heading"=-5.3614439061364445}, {"dt"=0.005, "x"=124.98375679123617, "y"=227.82425646533397, "position"=-135.62596606283253, "velocity"=-46.55214314454277, "acceleration"=86.62558387803188, "jerk"=-26.152550814515507, "heading"=-5.359022089169735}, {"dt"=0.005, "x"=125.12247265657071, "y"=227.6400458177824, "position"=-135.85656453196637, "velocity"=-46.11969382677015, "acceleration"=86.48986355452308, "jerk"=-27.144064701758452, "heading"=-5.356630146326033}, {"dt"=0.005, "x"=125.25945521513212, "y"=227.4572342412232, "position"=-136.08500335063363, "velocity"=-45.68776373345166, "acceleration"=86.3860186636984, "jerk"=-20.768978164937835, "heading"=-5.354267856310927}, {"dt"=0.005, "x"=125.39471964010531, "y"=227.27582973838392, "position"=-136.31128648812668, "velocity"=-45.256627498608495, "acceleration"=86.22724696863315, "jerk"=-31.75433901304814, "heading"=-5.351934984698101}, {"dt"=0.005, "x"=125.52827992518334, "y"=227.0958414548325, "position"=-136.53541620941752, "velocity"=-44.82594425816736, "acceleration"=86.13664808822676, "jerk"=-18.119776081277905, "heading"=-5.349631315795363}, {"dt"=0.005, "x"=125.66015080449836, "y"=226.91727711018495, "position"=-136.75739628507912, "velocity"=-44.396015132318496, "acceleration"=85.98582516977302, "jerk"=-30.16458369074826, "heading"=-5.347356619600318}, {"dt"=0.005, "x"=125.79034637042635, "y"=226.74014485809633, "position"=-136.9772296768041, "velocity"=-43.966678344991394, "acceleration"=85.86735746542047, "jerk"=-23.693540870510787, "heading"=-5.345110675704622}, {"dt"=0.005, "x"=125.91888062398566, "y"=226.5644525518049, "position"=-137.19491945797915, "velocity"=-43.53795623501554, "acceleration"=85.74442199517023, "jerk"=-24.58709405004811, "heading"=-5.342893263864422}, {"dt"=0.005, "x"=126.04576747412811, "y"=226.39020774707387, "position"=-137.41046881361453, "velocity"=-43.1098711270745, "acceleration"=85.61702158820879, "jerk"=-25.48008139228841, "heading"=-5.34070416407318}, {"dt"=0.005, "x"=126.17102031926977, "y"=226.21741828285323, "position"=-137.6238803272724, "velocity"=-42.682302731571134, "acceleration"=85.51367910067285, "jerk"=-20.66849750718802, "heading"=-5.338543163840311}, {"dt"=0.005, "x"=126.29465293599596, "y"=226.04609106212425, "position"=-137.8351574923454, "velocity"=-42.25543301459882, "acceleration"=85.37394339446251, "jerk"=-27.94714124206621, "heading"=-5.33641004291532}, {"dt"=0.005, "x"=126.41667847147416, "y"=225.8762334450325, "position"=-138.04430299526817, "velocity"=-41.82910058455698, "acceleration"=85.26648600836779, "jerk"=-21.49147721894451, "heading"=-5.334304590726418}, {"dt"=0.005, "x"=126.5371102855982, "y"=225.70785208764192, "position"=-138.25132015245546, "velocity"=-41.40343143745711, "acceleration"=85.13382941997492, "jerk"=-26.531317678575306, "heading"=-5.332226591903446}, {"dt"=0.005, "x"=126.65596122720544, "y"=225.54095395334673, "position"=-138.45621166900054, "velocity"=-40.97830330901629, "acceleration"=85.02562568816359, "jerk"=-21.640746362265872, "heading"=-5.330175838817026}, {"dt"=0.005, "x"=126.7732440515888, "y"=225.3755457377588, "position"=-138.65898035168925, "velocity"=-40.553736537743724, "acceleration"=84.91335425451325, "jerk"=-22.454286730066997, "heading"=-5.3281521244238625}, {"dt"=0.005, "x"=126.88897142023313, "y"=225.21163387130832, "position"=-138.85962910901563, "velocity"=-40.12975146527767, "acceleration"=84.79701449321055, "jerk"=-23.26795226053946, "heading"=-5.326155242318435}, {"dt"=0.005, "x"=127.00315590059581, "y"=225.04922452184869, "position"=-139.05816095116595, "velocity"=-39.70636843006313, "acceleration"=84.67660704290836, "jerk"=-24.081490060439137, "heading"=-5.324184986782299}, {"dt"=0.005, "x"=127.11580996592957, "y"=224.88832359726626, "position"=-139.25457898997018, "velocity"=-39.283607760846195, "acceleration"=84.55213384338691, "jerk"=-24.894639904289306, "heading"=-5.3222411528310944}, {"dt"=0.005, "x"=127.22694528571745, "y"=224.72893776760952, "position"=-139.4488851967669, "velocity"=-38.861241359339836, "acceleration"=84.47328030127181, "jerk"=-15.770708423019641, "heading"=-5.32032354850015}, {"dt"=0.005, "x"=127.33657438555908, "y"=224.57107209312574, "position"=-139.6410832995471, "velocity"=-38.43962055603898, "acceleration"=84.32416066017083, "jerk"=-29.823928220196194, "heading"=-5.3184319662441615}, {"dt"=0.005, "x"=127.44470870606501, "y"=224.41473281107722, "position"=-139.83117538876368, "velocity"=-38.018417843318076, "acceleration"=84.2405425441811, "jerk"=-16.72362319794729, "heading"=-5.316566216469471}, {"dt"=0.005, "x"=127.5513599601115, "y"=224.25992539277883, "position"=-140.0191642893666, "velocity"=-37.5977801205869, "acceleration"=84.12754454623581, "jerk"=-22.599599589057107, "heading"=-5.314726104152716}, {"dt"=0.005, "x"=127.65653974835247, "y"=224.10665509684952, "position"=-140.2050528889866, "velocity"=-37.177719923993415, "acceleration"=84.01203931869645, "jerk"=-23.10104550787173, "heading"=-5.312911435511433}, {"dt"=0.005, "x"=127.76025940642326, "y"=223.95492719615692, "position"=-140.38884386623766, "velocity"=-36.75819545021562, "acceleration"=83.90489475555967, "jerk"=-21.428912627357022, "heading"=-5.311122020675102}, {"dt"=0.005, "x"=127.86252983217105, "y"=223.80474723928623, "position"=-140.57053937919358, "velocity"=-36.33910259118442, "acceleration"=83.8185718062391, "jerk"=-17.264589864112168, "heading"=-5.309357676698809}, {"dt"=0.005, "x"=127.96336226436767, "y"=223.65611991253198, "position"=-140.75014244609613, "velocity"=-35.92061338051016, "acceleration"=83.6978421348519, "jerk"=-24.14593427744194, "heading"=-5.307618214161055}, {"dt"=0.005, "x"=128.06276763884767, "y"=223.50904998471043, "position"=-140.9276558037483, "velocity"=-35.50267153043233, "acceleration"=83.58837001556623, "jerk"=-21.894423857133916, "heading"=-5.305903448303006}, {"dt"=0.005, "x"=128.1607563288094, "y"=223.36354270177205, "position"=-141.1030814368483, "velocity"=-35.08512661999562, "acceleration"=83.50898208734208, "jerk"=-15.877585644830106, "heading"=-5.3042132035372}, {"dt"=0.005, "x"=128.25733902146297, "y"=223.21960249307162, "position"=-141.27642214239935, "velocity"=-34.66814111020896, "acceleration"=83.39710195733261, "jerk"=-22.37602600189348, "heading"=-5.302547298353757}, {"dt"=0.005, "x"=128.35252613438146, "y"=223.07723383736968, "position"=-141.4476804869906, "velocity"=-34.251668918250935, "acceleration"=83.29443839160433, "jerk"=-20.532713145655634, "heading"=-5.3009055554160724}, {"dt"=0.005, "x"=128.44632780388585, "y"=222.9364412875089, "position"=-141.61685878139656, "velocity"=-33.835658881191925, "acceleration"=83.20200741180201, "jerk"=-18.486195960463192, "heading"=-5.299287801786878}, {"dt"=0.005, "x"=128.5387540772972, "y"=222.79722918775684, "position"=-141.783959423927, "velocity"=-33.4201285060882, "acceleration"=83.1060750207456, "jerk"=-19.18647821128161, "heading"=-5.29769386563739}, {"dt"=0.005, "x"=128.62981491322586, "y"=222.65960167571032, "position"=-141.9489849004818, "velocity"=-33.00509531096149, "acceleration"=83.00663902534211, "jerk"=-19.887199080699247, "heading"=-5.296123576266811}, {"dt"=0.005, "x"=128.71952008810746, "y"=222.52356282664405, "position"=-142.11193761403948, "velocity"=-32.5905427115372, "acceleration"=82.91051988485663, "jerk"=-19.223828097096884, "heading"=-5.29457676573744}, {"dt"=0.005, "x"=128.80787884990153, "y"=222.38911718607937, "position"=-142.2728192508183, "velocity"=-32.1763273557612, "acceleration"=82.84307115520022, "jerk"=-13.48974593128105, "heading"=-5.2930532748674874}, {"dt"=0.005, "x"=128.89490116975298, "y"=222.25626786923027, "position"=-142.4316330573327, "velocity"=-31.762761302885956, "acceleration"=82.71321057504935, "jerk"=-25.97211603017513, "heading"=-5.291552931671084}, {"dt"=0.005, "x"=128.98059590735326, "y"=222.12501935755887, "position"=-142.58838049708322, "velocity"=-31.349487950101196, "acceleration"=82.65467055695197, "jerk"=-11.708003619474994, "heading"=-5.290075583011444}, {"dt"=0.005, "x"=129.0649723489318, "y"=221.9953751595444, "position"=-142.7430640513877, "velocity"=-30.936710860897755, "acceleration"=82.55541784068825, "jerk"=-19.850543252744046, "heading"=-5.2886210681029056}, {"dt"=0.005, "x"=129.14803955592495, "y"=221.86733880586723, "position"=-142.89568603126148, "velocity"=-30.52439597475387, "acceleration"=82.46297722877713, "jerk"=-18.488122382223082, "heading"=-5.287189229759931}, {"dt"=0.005, "x"=129.22980633680316, "y"=221.74091389872183, "position"=-143.0462485219486, "velocity"=-30.11249813742463, "acceleration"=82.37956746584771, "jerk"=-16.68195258588412, "heading"=-5.285779914900134}, {"dt"=0.005, "x"=129.31028141626493, "y"=221.61610385527646, "position"=-143.19475369141824, "velocity"=-29.70103389393099, "acceleration"=82.292848698728, "jerk"=-17.34375342394401, "heading"=-5.2843929716448965}, {"dt"=0.005, "x"=129.38947336121137, "y"=221.49291202520524, "position"=-143.34120365263604, "velocity"=-29.289992243561457, "acceleration"=82.20833007390667, "jerk"=-16.90372496426562, "heading"=-5.283028250611857}, {"dt"=0.005, "x"=129.46739026860135, "y"=221.3713421823707, "position"=-143.4855998823099, "velocity"=-28.879245934775373, "acceleration"=82.14926175721686, "jerk"=-11.813663337960634, "heading"=-5.281685610309124}, {"dt"=0.005, "x"=129.5440409726094, "y"=221.2513966440825, "position"=-143.6279454568115, "velocity"=-28.46911490031259, "acceleration"=82.02620689255653, "jerk"=-24.61097293206649, "heading"=-5.280364896349182}, {"dt"=0.005, "x"=129.6194329830024, "y"=221.1330794947223, "position"=-143.7682412267542, "velocity"=-28.05915398854598, "acceleration"=81.99218235332211, "jerk"=-6.804907846884589, "heading"=-5.279065976987491}, {"dt"=0.005, "x"=129.6935747677132, "y"=221.01639301835078, "position"=-143.90649005317997, "velocity"=-27.649765285151002, "acceleration"=81.87774067899554, "jerk"=-22.888334865314164, "heading"=-5.277788703806548}, {"dt"=0.005, "x"=129.76647403080753, "y"=220.90134039925533, "position"=-144.04269360570493, "velocity"=-27.240710504993103, "acceleration"=81.8109560315797, "jerk"=-13.356929483165914, "heading"=-5.276532941399424}, {"dt"=0.005, "x"=129.83813839757624, "y"=220.78792465339552, "position"=-144.17685363281174, "velocity"=-26.832005421360645, "acceleration"=81.74101672649172, "jerk"=-13.98786101759697, "heading"=-5.275298555577919}, {"dt"=0.005, "x"=129.90857541495626, "y"=220.67614862969748, "position"=-144.30897196193808, "velocity"=-26.42366582526944, "acceleration"=81.66791921824128, "jerk"=-14.619501650088296, "heading"=-5.274085413377754}, {"dt"=0.005, "x"=129.97779255195962, "y"=220.566015011346, "position"=-144.4390504995457, "velocity"=-26.015707521520554, "acceleration"=81.5916607497769, "jerk"=-15.251693692874824, "heading"=-5.272893383063071}, {"dt"=0.005, "x"=130.04579720010852, "y"=220.4575263170776, "position"=-144.56709123116622, "velocity"=-25.608146324104407, "acceleration"=81.51223948322937, "jerk"=-15.884253309508267, "heading"=-5.271722334130329}, {"dt"=0.005, "x"=130.11259655530478, "y"=220.35068509236297, "position"=-144.69309599755684, "velocity"=-25.20095327812567, "acceleration"=81.43860919574735, "jerk"=-14.726057496403655, "heading"=-5.27057213935315}, {"dt"=0.005, "x"=130.178197285941, "y"=220.24549444666124, "position"=-144.81706586406943, "velocity"=-24.79397330251993, "acceleration"=81.39599512114799, "jerk"=-8.52281491987128, "heading"=-5.269442680505774}, {"dt"=0.005, "x"=130.2426067186446, "y"=220.141956155886, "position"=-144.93900335903245, "velocity"=-24.38749899260616, "acceleration"=81.29486198275373, "jerk"=-20.226627678852083, "heading"=-5.268333827957143}, {"dt"=0.005, "x"=130.30583149169493, "y"=220.04007282230475, "position"=-145.05890992928153, "velocity"=-23.981314049812312, "acceleration"=81.23698855876995, "jerk"=-11.574684796755719, "heading"=-5.267245463865186}, {"dt"=0.005, "x"=130.36787797465814, "y"=219.93984720982422, "position"=-145.17678672702053, "velocity"=-23.57535954780002, "acceleration"=81.19090040245851, "jerk"=-9.21763126228825, "heading"=-5.266177474958598}, {"dt"=0.005, "x"=130.42875294305736, "y"=219.841281155762, "position"=-145.29263589098386, "velocity"=-23.16983279266547, "acceleration"=81.10535102690974, "jerk"=-17.109875109753148, "heading"=-5.26512974093265}, {"dt"=0.005, "x"=130.48846274888416, "y"=219.74437691128102, "position"=-145.4064589708504, "velocity"=-22.76461597330723, "acceleration"=81.04336387164821, "jerk"=-12.397431052306729, "heading"=-5.264102148735701}, {"dt"=0.005, "x"=130.5470136278832, "y"=219.64913664936583, "position"=-145.51825750805565, "velocity"=-22.359707441049963, "acceleration"=80.9817064514533, "jerk"=-12.331484038980989, "heading"=-5.263094587286882}, {"dt"=0.005, "x"=130.6044114284781, "y"=219.5555629097596, "position"=-145.62803251548917, "velocity"=-21.955001486702333, "acceleration"=80.94119086952603, "jerk"=-8.103116385456133, "heading"=-5.262106952147439}, {"dt"=0.005, "x"=130.66066252283588, "y"=219.46365711611512, "position"=-145.73578621854327, "velocity"=-21.55074061081917, "acceleration"=80.85217517663281, "jerk"=-17.803138578642574, "heading"=-5.261139129851073}, {"dt"=0.005, "x"=130.71577263564166, "y"=219.3734214869058, "position"=-145.84151981449207, "velocity"=-21.146719189760315, "acceleration"=80.80428421177075, "jerk"=-9.57819297241258, "heading"=-5.260191018063948}, {"dt"=0.005, "x"=130.76974749379198, "y"=219.28485798005235, "position"=-145.9452347124505, "velocity"=-20.742979591689213, "acceleration"=80.74791961422036, "jerk"=-11.272919510076918, "heading"=-5.25926251441117}, {"dt"=0.005, "x"=130.82259260393437, "y"=219.1979686593929, "position"=-146.04693210529135, "velocity"=-20.33947856816584, "acceleration"=80.7002047046744, "jerk"=-9.542981909191894, "heading"=-5.258353520309939}, {"dt"=0.005, "x"=130.87431366335446, "y"=219.11275502111724, "position"=-146.14661375924888, "velocity"=-19.93633079150886, "acceleration"=80.62955533139657, "jerk"=-14.129874655566255, "heading"=-5.257463933907583}, {"dt"=0.005, "x"=130.92491595995293, "y"=219.02921898256477, "position"=-146.24428085789566, "velocity"=-19.533419729354815, "acceleration"=80.58221243080865, "jerk"=-9.468580117584224, "heading"=-5.256593660407974}, {"dt"=0.005, "x"=130.9744047145354, "y"=218.94736232259646, "position"=-146.33993465871555, "velocity"=-19.130760163979634, "acceleration"=80.53191307503624, "jerk"=-10.059871154481925, "heading"=-5.255742606188441}, {"dt"=0.005, "x"=131.02278508119022, "y"=218.86718668240522, "position"=-146.43357649315791, "velocity"=-18.72836688847119, "acceleration"=80.4786551016889, "jerk"=-10.651594669468523, "heading"=-5.25491067879841}, {"dt"=0.005, "x"=131.07006214766827, "y"=218.78869356632666, "position"=-146.5252077666757, "velocity"=-18.326254703558075, "acceleration"=80.42243698262297, "jerk"=-11.243623813186332, "heading"=-5.254097786957748}, {"dt"=0.005, "x"=131.11624071868692, "y"=218.7118847040416, "position"=-146.61482953717174, "velocity"=-17.924354099212316, "acceleration"=80.38012086915174, "jerk"=-8.463222694246042, "heading"=-5.2533038442868785}, {"dt"=0.005, "x"=131.16132545475512, "y"=218.63676182368397, "position"=-146.7024427814877, "velocity"=-17.522648863190327, "acceleration"=80.34104720439785, "jerk"=-7.81473295077717, "heading"=-5.252528766923235}, {"dt"=0.005, "x"=131.205321305497, "y"=218.56332593038115, "position"=-146.7880492374807, "velocity"=-17.121291198603128, "acceleration"=80.27153291743971, "jerk"=-13.902857391627776, "heading"=-5.2517724660762815}, {"dt"=0.005, "x"=131.24823261871745, "y"=218.49157879344563, "position"=-146.87164967085727, "velocity"=-16.720086675313187, "acceleration"=80.24090465798821, "jerk"=-6.125651890300787, "heading"=-5.251034863347463}, {"dt"=0.005, "x"=131.29006374247803, "y"=218.4215219460706, "position"=-146.9532450431476, "velocity"=-16.31907445806704, "acceleration"=80.20244344922958, "jerk"=-7.6922417517266695, "heading"=-5.250315880382631}, {"dt"=0.005, "x"=131.3308191743577, "y"=218.3531564350516, "position"=-147.032836803554, "velocity"=-15.918352081280679, "acceleration"=80.14447535727207, "jerk"=-11.593618391501082, "heading"=-5.249615436310891}, {"dt"=0.005, "x"=131.37050305979292, "y"=218.28648366270156, "position"=-147.11042590933616, "velocity"=-15.517821156432856, "acceleration"=80.10618496956461, "jerk"=-7.658077541492503, "heading"=-5.248933456370173}, {"dt"=0.005, "x"=131.40911948217885, "y"=218.22150490335238, "position"=-147.186013390075, "velocity"=-15.117496147770307, "acceleration"=80.0650017325097, "jerk"=-8.236647410981845, "heading"=-5.248269866923766}, {"dt"=0.005, "x"=131.44667246318696, "y"=218.15822130396862, "position"=-147.2596003477072, "velocity"=-14.717391526435733, "acceleration"=80.02092426691476, "jerk"=-8.81549311898766, "heading"=-5.247624595457939}, {"dt"=0.005, "x"=131.48316569518576, "y"=218.09663433719857, "position"=-147.33118743074354, "velocity"=-14.317416607270875, "acceleration"=79.99498383297166, "jerk"=-5.188086788621149, "heading"=-5.2469975751821964}, {"dt"=0.005, "x"=131.51860296633848, "y"=218.03674508675923, "position"=-147.40077566613527, "velocity"=-13.917647078349379, "acceleration"=79.9539057842992, "jerk"=-8.21560973449209, "heading"=-5.246388737727301}, {"dt"=0.005, "x"=131.55298815957826, "y"=217.97855424836908, "position"=-147.4683664583091, "velocity"=-13.518158434765464, "acceleration"=79.89772871678298, "jerk"=-11.235413503243308, "heading"=-5.245798013166371}, {"dt"=0.005, "x"=131.58632442909513, "y"=217.92206352553188, "position"=-147.53395996890254, "velocity"=-13.118702118685487, "acceleration"=79.89126321599542, "jerk"=-1.2931001575111623, "heading"=-5.2452253441644885}, {"dt"=0.005, "x"=131.6186154056758, "y"=217.86727359145948, "position"=-147.59755748492472, "velocity"=-12.719503204436158, "acceleration"=79.83978284986577, "jerk"=-10.296073225930513, "heading"=-5.24467066527342}, {"dt"=0.005, "x"=131.64986443795763, "y"=217.81418537404352, "position"=-147.6591599268159, "velocity"=-12.320488378234934, "acceleration"=79.80296524024482, "jerk"=-7.3635219241907635, "heading"=-5.244133915968822}, {"dt"=0.005, "x"=131.68007464327195, "y"=217.7627999726878, "position"=-147.71876794622287, "velocity"=-11.921603881395855, "acceleration"=79.7768993678158, "jerk"=-5.2131744858030515, "heading"=-5.243615039777961}, {"dt"=0.005, "x"=131.70924908071103, "y"=217.71311836607438, "position"=-147.77638226593226, "velocity"=-11.522863941878278, "acceleration"=79.7479879035155, "jerk"=-5.782292860061489, "heading"=-5.243113981308587}, {"dt"=0.005, "x"=131.73739075137325, "y"=217.6651414126013, "position"=-147.83200367990403, "velocity"=-11.124282794356915, "acceleration"=79.71622950427246, "jerk"=-6.351679848606295, "heading"=-5.242630686246613}, {"dt"=0.005, "x"=131.76450259860766, "y"=217.61886985082384, "position"=-147.88563305329012, "velocity"=-10.725874677220148, "acceleration"=79.68162342735354, "jerk"=-6.921215383783874, "heading"=-5.242165101353676}, {"dt"=0.005, "x"=131.79058748105757, "y"=217.57430434639656, "position"=-147.93727126856993, "velocity"=-10.32764305596132, "acceleration"=79.64632425176568, "jerk"=-7.059835117573243, "heading"=-5.241717174931665}, {"dt"=0.005, "x"=131.81564758019098, "y"=217.53144650691286, "position"=-147.986918050679, "velocity"=-9.929356421817497, "acceleration"=79.6573268287645, "jerk"=2.200515399763958, "heading"=-5.241286866997227}, {"dt"=0.005, "x"=131.8396861423132, "y"=217.4902959042947, "position"=-148.03457541700092, "velocity"=-9.531473264384587, "acceleration"=79.57663148658192, "jerk"=-16.139068436515913, "heading"=-5.240874119370667}, {"dt"=0.005, "x"=131.86270494345658, "y"=217.45085441225837, "position"=-148.08024265361678, "velocity"=-9.133447323173918, "acceleration"=79.6051882421338, "jerk"=5.711351110377905, "heading"=-5.240478899207243}, {"dt"=0.005, "x"=131.88470677282675, "y"=217.41312195714835, "position"=-148.12392123720488, "velocity"=-8.735716717621928, "acceleration"=79.546121110398, "jerk"=-11.813426347160316, "heading"=-5.240101156356424}, {"dt"=0.005, "x"=131.90569379689745, "y"=217.377099319656, "position"=-148.1656115909003, "velocity"=-8.33807073908529, "acceleration"=79.52919570732746, "jerk"=-3.385080614108915, "heading"=-5.239740851451684}, {"dt"=0.005, "x"=131.92566808636738, "y"=217.3427872340583, "position"=-148.20531412807227, "velocity"=-7.9405074343942035, "acceleration"=79.51266093821746, "jerk"=-3.306953821999059, "heading"=-5.239397946863345}, {"dt"=0.005, "x"=131.94463165671272, "y"=217.3101863193274, "position"=-148.24302933245372, "velocity"=-7.543040876286894, "acceleration"=79.49331162146187, "jerk"=-3.869863351118852, "heading"=-5.239072406003404}, {"dt"=0.005, "x"=131.9625864683533, "y"=217.27929707941223, "position"=-148.27875775816193, "velocity"=-7.145685141640041, "acceleration"=79.47114692937056, "jerk"=-4.432938418261756, "heading"=-5.238764193323682}, {"dt"=0.005, "x"=131.97953442681825, "y"=217.25011990352448, "position"=-148.31250002970543, "velocity"=-6.748454308698169, "acceleration"=79.44616658837447, "jerk"=-4.996068199218939, "heading"=-5.238473274313909}, {"dt"=0.005, "x"=131.99547713644262, "y"=217.22265549115323, "position"=-148.34425635091972, "velocity"=-6.351264242856643, "acceleration"=79.43801316830523, "jerk"=-1.630684013846917, "heading"=-5.238199619730278}, {"dt"=0.005, "x"=132.0104161491781, "y"=217.19690442488496, "position"=-148.37402699947603, "velocity"=-5.954129711263447, "acceleration"=79.42690631863911, "jerk"=-2.221369933224082, "heading"=-5.237943201324963}, {"dt"=0.005, "x"=132.02435320958375, "y"=217.17286674814966, "position"=-148.40181281520245, "velocity"=-5.557163145281169, "acceleration"=79.39331319645557, "jerk"=-6.7186244367093195, "heading"=-5.23770398764198}, {"dt"=0.005, "x"=132.03728961372275, "y"=217.1505430711526, "position"=-148.427613921898, "velocity"=-5.160221339113117, "acceleration"=79.38836123361045, "jerk"=-0.9903925690224469, "heading"=-5.237481955021797}, {"dt"=0.005, "x"=132.0492265152328, "y"=217.12993404451848, "position"=-148.45143033633147, "velocity"=-4.763282886694113, "acceleration"=79.38769048380081, "jerk"=-0.13414996192864237, "heading"=-5.237277082348053}, {"dt"=0.005, "x"=132.06016535205592, "y"=217.1110396227085, "position"=-148.47326281962074, "velocity"=-4.3664966578566995, "acceleration"=79.35724576748271, "jerk"=-6.088943263620195, "heading"=-5.237089343724299}, {"dt"=0.005, "x"=132.07010717829152, "y"=217.09386021792213, "position"=-148.4931115439554, "velocity"=-3.9697448669283437, "acceleration"=79.35035818567115, "jerk"=-1.377516362310871, "heading"=-5.236918719941918}, {"dt"=0.005, "x"=132.0790529946666, "y"=217.0783961302465, "position"=-148.51097675143407, "velocity"=-3.5730414957366734, "acceleration"=79.34067423833406, "jerk"=-1.9367894674189756, "heading"=-5.236765192808557}, {"dt"=0.005, "x"=132.08700374861928, "y"=217.06464754779446, "position"=-148.52685875407406, "velocity"=-3.17640052799536, "acceleration"=79.32819354826267, "jerk"=-2.496138014276994, "heading"=-5.23662874514713}, {"dt"=0.005, "x"=132.0939763633687, "y"=217.05258681723177, "position"=-148.54078996285685, "velocity"=-2.7862417565593884, "acceleration"=78.0317542871943, "jerk"=-259.28785221367434, "heading"=-5.236509085717763}, {"dt"=0.005, "x"=132.10002064629083, "y"=217.04212915320548, "position"=-148.55286870835997, "velocity"=-2.4157491006260434, "acceleration"=74.098531186669, "jerk"=-786.6446201050593, "heading"=-5.2364053590698845}, {"dt"=0.005, "x"=132.1052037360159, "y"=217.03315950930093, "position"=-148.5632281934279, "velocity"=-2.071897013585861, "acceleration"=68.77041740803644, "jerk"=-1065.622755726514, "heading"=-5.236316412467169}, {"dt"=0.005, "x"=132.10959159172086, "y"=217.0255646252826, "position"=-148.57199948415044, "velocity"=-1.7542581445059653, "acceleration"=63.52777381597918, "jerk"=-1048.528718411451, "heading"=-5.236241113541984}, {"dt"=0.005, "x"=132.11325125963927, "y"=217.01922914239967, "position"=-148.57931600741173, "velocity"=-1.4633046522602582, "acceleration"=58.19069844914142, "jerk"=-1067.4150733675517, "heading"=-5.2361783113812415}, {"dt"=0.005, "x"=132.11624871949613, "y"=217.01403936542744, "position"=-148.5853092161195, "velocity"=-1.1986417415551873, "acceleration"=52.93258214101417, "jerk"=-1051.62326162545, "heading"=-5.236126873465969}, {"dt"=0.005, "x"=132.11865032739894, "y"=217.00988079675346, "position"=-148.59011144621968, "velocity"=-0.9604460200342335, "acceleration"=47.63914430419076, "jerk"=-1058.687567364683, "heading"=-5.2360856608943855}, {"dt"=0.005, "x"=132.12052245554784, "y"=217.00663878846615, "position"=-148.59385517184276, "velocity"=-0.7487451246169743, "acceleration"=42.340179083451844, "jerk"=-1059.793044147783, "heading"=-5.236053534550423}, {"dt"=0.005, "x"=132.1219312419939, "y"=217.00419900129245, "position"=-148.5966724827421, "velocity"=-0.5634621798687216, "acceleration"=37.05658894965054, "jerk"=-1056.718026760261, "heading"=-5.236029359385066}, {"dt"=0.005, "x"=132.12294280544, "y"=217.00244705522007, "position"=-148.59869549427097, "velocity"=-0.40460230577654477, "acceleration"=31.771974818435368, "jerk"=-1056.9228262430343, "heading"=-5.236012000718892}, {"dt"=0.005, "x"=132.12362325032578, "y"=217.0012685402028, "position"=-148.6000563406578, "velocity"=-0.2721692773633899, "acceleration"=26.48660568263097, "jerk"=-1057.0738271608795, "heading"=-5.23600032414495}, {"dt"=0.005, "x"=132.12403867113122, "y"=217.0005490252225, "position"=-148.60088716931187, "velocity"=-0.16616573081747343, "acceleration"=21.200709309183296, "jerk"=-1057.1792746895349, "heading"=-5.235993195446554}, {"dt"=0.005, "x"=132.12425515589948, "y"=217.00017406570657, "position"=-148.6013201361622, "velocity"=-0.0865933700650372, "acceleration"=15.914472150487246, "jerk"=-1057.24743173921, "heading"=-5.235989480529987}, {"dt"=0.005, "x"=132.1243387889785, "y"=217.00002920930137, "position"=-148.6014874020285, "velocity"=-0.0334531732623033, "acceleration"=10.62803936054678, "jerk"=-1057.2865579880934, "heading"=-5.235988045372129}, {"dt"=0.005, "x"=132.12435565298176, "y"=217.00000000000068, "position"=-148.60152113002658, "velocity"=-0.006745599612317408, "acceleration"=5.3415147299971775, "jerk"=-1057.3049261099204, "heading"=-5.235987755982995}, {"dt"=0.005, "x"=132.12435565298176, "y"=217.00000000000068, "position"=-148.60152113002658, "velocity"=-0.0, "acceleration"=1.3491199224634816, "jerk"=-798.4789615067392, "heading"=-5.235987755982995}]
  in  "Tab Control":enum32{"Primary Path", "Tank Position"}(tab)=enum."Tank Position"
  out "Path":T2(graph)=[{"position"=5.8139534883720933e-05, "velocity"=0.023255813953488372, "acceleration"=4.651162790697675, "jerk"=930.232558139535, "heading"=359.99641552036934}, {"position"=0.00029069767441860465, "velocity"=0.06976744186046512, "acceleration"=9.30232558139535, "jerk"=930.232558139535, "heading"=359.9964795545839}, {"position"=0.000813953488372093, "velocity"=0.13953488372093023, "acceleration"=13.953488372093023, "jerk"=930.2325581395347, "heading"=359.99662362906804}, {"position"=0.0017441860465116279, "velocity"=0.23255813953488372, "acceleration"=18.6046511627907, "jerk"=930.2325581395351, "heading"=359.99687975294165}, {"position"=0.003197674418604651, "velocity"=0.3488372093023256, "acceleration"=23.255813953488374, "jerk"=930.2325581395351, "heading"=359.9972799246043}, {"position"=0.005290697674418605, "velocity"=0.4883720930232558, "acceleration"=27.90697674418604, "jerk"=930.232558139533, "heading"=359.9978561249011}, {"position"=0.00813953488372093, "velocity"=0.6511627906976745, "acceleration"=32.558139534883736, "jerk"=930.2325581395394, "heading"=359.99864030858157}, {"position"=0.01186046511627907, "velocity"=0.8372093023255814, "acceleration"=37.2093023255814, "jerk"=930.2325581395322, "heading"=359.9996643940511}, {"position"=0.016569767441860467, "velocity"=1.0465116279069768, "acceleration"=41.86046511627908, "jerk"=930.2325581395365, "heading"=0.0009602423691011383}, {"position"=0.02238372093023256, "velocity"=1.2790697674418605, "acceleration"=46.511627906976734, "jerk"=930.2325581395309, "heading"=0.002559664708869217}, {"position"=0.02941860465116279, "velocity"=1.5348837209302326, "acceleration"=51.16279069767442, "jerk"=930.2325581395365, "heading"=0.00449437787587128}, {"position"=0.0377906976744186, "velocity"=1.813953488372093, "acceleration"=55.81395348837206, "jerk"=930.232558139528, "heading"=0.006796008415301311}, {"position"=0.04761627906976744, "velocity"=2.116279069767442, "acceleration"=60.46511627906983, "jerk"=930.232558139555, "heading"=0.009496054948300307}, {"position"=0.05901162790697674, "velocity"=2.441860465116279, "acceleration"=65.11627906976737, "jerk"=930.2325581395081, "heading"=0.012625899424631526}, {"position"=0.07209302325581395, "velocity"=2.7906976744186047, "acceleration"=69.76744186046515, "jerk"=930.2325581395564, "heading"=0.01621674881988809}, {"position"=0.08691860465116279, "velocity"=3.13953488372093, "acceleration"=69.76744186046506, "jerk"=-1.9895196601282805e-11, "heading"=0.020283685018371522}, {"position"=0.10348837209302325, "velocity"=3.488372093023256, "acceleration"=69.76744186046515, "jerk"=1.9895196601282805e-11, "heading"=0.02482570204547268}, {"position"=0.12180232558139534, "velocity"=3.8372093023255816, "acceleration"=69.76744186046515, "jerk"=0.0, "heading"=0.029841658125663147}, {"position"=0.14186046511627906, "velocity"=4.186046511627907, "acceleration"=69.76744186046515, "jerk"=0.0, "heading"=0.03533032380162224}, {"position"=0.16366279069767442, "velocity"=4.534883720930233, "acceleration"=69.76744186046506, "jerk"=-1.9895196601282805e-11, "heading"=0.041290320567104216}, {"position"=0.1872093023255814, "velocity"=4.883720930232558, "acceleration"=69.76744186046506, "jerk"=0.0, "heading"=0.04772017794892248}, {"position"=0.2125, "velocity"=5.232558139534884, "acceleration"=69.76744186046524, "jerk"=3.694822225952521e-11, "heading"=0.054618290282578516}, {"position"=0.23953488372093024, "velocity"=5.5813953488372094, "acceleration"=69.76744186046506, "jerk"=-3.694822225952521e-11, "heading"=0.061982937813718705}, {"position"=0.2683139534883721, "velocity"=5.930232558139535, "acceleration"=69.76744186046506, "jerk"=0.0, "heading"=0.06981228684700659}, {"position"=0.2988372093023256, "velocity"=6.27906976744186, "acceleration"=69.76744186046506, "jerk"=0.0, "heading"=0.0781043899020686}, {"position"=0.3311046511627907, "velocity"=6.627906976744186, "acceleration"=69.76744186046524, "jerk"=3.694822225952521e-11, "heading"=0.08685716545628686}, {"position"=0.36511627906976746, "velocity"=6.976744186046512, "acceleration"=69.76744186046506, "jerk"=-3.694822225952521e-11, "heading"=0.09606844025414696}, {"position"=0.4008720930232558, "velocity"=7.325581395348837, "acceleration"=69.76744186046506, "jerk"=0.0, "heading"=0.10573589485975801}, {"position"=0.4383720930232558, "velocity"=7.674418604651163, "acceleration"=69.76744186046524, "jerk"=3.694822225952521e-11, "heading"=0.1158571227666791}, {"position"=0.47761627906976745, "velocity"=8.023255813953488, "acceleration"=69.76744186046506, "jerk"=-3.694822225952521e-11, "heading"=0.1264295844600643}, {"position"=0.5186046511627908, "velocity"=8.372093023255815, "acceleration"=69.76744186046524, "jerk"=3.694822225952521e-11, "heading"=0.13745062805459177}, {"position"=0.5613372093023257, "velocity"=8.720930232558139, "acceleration"=69.76744186046488, "jerk"=-7.105427357601002e-11, "heading"=0.1489174895187566}, {"position"=0.6058139534883722, "velocity"=9.069767441860465, "acceleration"=69.76744186046524, "jerk"=7.105427357601002e-11, "heading"=0.16082727365197}, {"position"=0.6520348837209303, "velocity"=9.418604651162791, "acceleration"=69.76744186046524, "jerk"=0.0, "heading"=0.173176997097891}, {"position"=0.7000000000000001, "velocity"=9.767441860465116, "acceleration"=69.76744186046488, "jerk"=-7.105427357601002e-11, "heading"=0.18596353582924488}, {"position"=0.7497093023255814, "velocity"=10.116279069767442, "acceleration"=69.76744186046524, "jerk"=7.105427357601002e-11, "heading"=0.19918367349298272}, {"position"=0.8011627906976745, "velocity"=10.465116279069768, "acceleration"=69.76744186046524, "jerk"=0.0, "heading"=0.2128340639616387}, {"position"=0.8543604651162792, "velocity"=10.813953488372093, "acceleration"=69.76744186046488, "jerk"=-7.105427357601002e-11, "heading"=0.2269112508691045}, {"position"=0.9093023255813955, "velocity"=11.162790697674419, "acceleration"=69.76744186046524, "jerk"=7.105427357601002e-11, "heading"=0.24141166789842528}, {"position"=0.9659883720930234, "velocity"=11.511627906976743, "acceleration"=69.76744186046488, "jerk"=-7.105427357601002e-11, "heading"=0.2563316390753554}, {"position"=1.024418604651163, "velocity"=11.86046511627907, "acceleration"=69.76744186046524, "jerk"=7.105427357601002e-11, "heading"=0.2716673625102021}, {"position"=1.084593023255814, "velocity"=12.209302325581396, "acceleration"=69.76744186046524, "jerk"=0.0, "heading"=0.2874149399014114}, {"position"=1.146511627906977, "velocity"=12.55813953488372, "acceleration"=69.76744186046488, "jerk"=-7.105427357601002e-11, "heading"=0.30357034436914254}, {"position"=1.2101744186046512, "velocity"=12.906976744186046, "acceleration"=69.76744186046524, "jerk"=7.105427357601002e-11, "heading"=0.3201294566862132}, {"position"=1.2755813953488373, "velocity"=13.255813953488373, "acceleration"=69.76744186046524, "jerk"=0.0, "heading"=0.3370880334762515}, {"position"=1.342732558139535, "velocity"=13.604651162790697, "acceleration"=69.76744186046488, "jerk"=-7.105427357601002e-11, "heading"=0.3544417241153612}, {"position"=1.4116279069767443, "velocity"=13.953488372093023, "acceleration"=69.76744186046524, "jerk"=7.105427357601002e-11, "heading"=0.37218607108112045}, {"position"=1.4822674418604653, "velocity"=14.30232558139535, "acceleration"=69.76744186046524, "jerk"=0.0, "heading"=0.39031649782924227}, {"position"=1.5546511627906978, "velocity"=14.651162790697674, "acceleration"=69.76744186046488, "jerk"=-7.105427357601002e-11, "heading"=0.4088283277055191}, {"position"=1.628779069767442, "velocity"=15.0, "acceleration"=69.76744186046524, "jerk"=7.105427357601002e-11, "heading"=0.4277167730334406}, {"position"=1.704651162790698, "velocity"=15.348837209302326, "acceleration"=69.76744186046524, "jerk"=0.0, "heading"=0.4469769414625338}, {"position"=1.7822674418604654, "velocity"=15.697674418604649, "acceleration"=69.76744186046453, "jerk"=-1.4210854715202004e-10, "heading"=0.4666038236806682}, {"position"=1.8616279069767445, "velocity"=16.046511627906977, "acceleration"=69.7674418604656, "jerk"=2.1316282072803006e-10, "heading"=0.4865923062824054}, {"position"=1.9427325581395352, "velocity"=16.3953488372093, "acceleration"=69.76744186046488, "jerk"=-1.4210854715202004e-10, "heading"=0.5069371721637213}, {"position"=2.0255813953488375, "velocity"=16.74418604651163, "acceleration"=69.7674418604656, "jerk"=1.4210854715202004e-10, "heading"=0.527633100919862}, {"position"=2.1101744186046516, "velocity"=17.093023255813954, "acceleration"=69.76744186046488, "jerk"=-1.4210854715202004e-10, "heading"=0.5486746639868849}, {"position"=2.196511627906977, "velocity"=17.441860465116278, "acceleration"=69.76744186046488, "jerk"=0.0, "heading"=0.5700563129727969}, {"position"=2.2845930232558143, "velocity"=17.790697674418606, "acceleration"=69.7674418604656, "jerk"=1.4210854715202004e-10, "heading"=0.5917724189820646}, {"position"=2.3744186046511633, "velocity"=18.13953488372093, "acceleration"=69.76744186046488, "jerk"=-1.4210854715202004e-10, "heading"=0.6138172359630532}, {"position"=2.465988372093024, "velocity"=18.488372093023255, "acceleration"=69.76744186046488, "jerk"=0.0, "heading"=0.636184912033048}, {"position"=2.559302325581396, "velocity"=18.837209302325583, "acceleration"=69.7674418604656, "jerk"=1.4210854715202004e-10, "heading"=0.6588694951654509}, {"position"=2.6543604651162793, "velocity"=19.186046511627907, "acceleration"=69.76744186046488, "jerk"=-1.4210854715202004e-10, "heading"=0.6818649336190002}, {"position"=2.7511627906976748, "velocity"=19.53488372093023, "acceleration"=69.76744186046488, "jerk"=0.0, "heading"=0.7051650763681947}, {"position"=2.8497093023255817, "velocity"=19.88372093023256, "acceleration"=69.7674418604656, "jerk"=1.4210854715202004e-10, "heading"=0.7287636499179433}, {"position"=2.95, "velocity"=20.232558139534884, "acceleration"=69.76744186046488, "jerk"=-1.4210854715202004e-10, "heading"=0.7526543153348971}, {"position"=3.0520348837209306, "velocity"=20.58139534883721, "acceleration"=69.76744186046488, "jerk"=0.0, "heading"=0.7768305975264821}, {"position"=3.1558139534883725, "velocity"=20.930232558139537, "acceleration"=69.7674418604656, "jerk"=1.4210854715202004e-10, "heading"=0.8012859442369253}, {"position"=3.261337209302326, "velocity"=21.27906976744186, "acceleration"=69.76744186046488, "jerk"=-1.4210854715202004e-10, "heading"=0.8260136993289268}, {"position"=3.368604651162791, "velocity"=21.627906976744185, "acceleration"=69.76744186046488, "jerk"=0.0, "heading"=0.8510071067529174}, {"position"=3.477616279069768, "velocity"=21.976744186046513, "acceleration"=69.7674418604656, "jerk"=1.4210854715202004e-10, "heading"=0.8762593029517616}, {"position"=3.5883720930232563, "velocity"=22.325581395348838, "acceleration"=69.76744186046488, "jerk"=-1.4210854715202004e-10, "heading"=0.9017633441093831}, {"position"=3.700872093023256, "velocity"=22.674418604651162, "acceleration"=69.76744186046488, "jerk"=0.0, "heading"=0.9275121812841483}, {"position"=3.815116279069768, "velocity"=23.023255813953487, "acceleration"=69.76744186046488, "jerk"=0.0, "heading"=0.9534986677131823}, {"position"=3.931104651162791, "velocity"=23.372093023255815, "acceleration"=69.7674418604656, "jerk"=1.4210854715202004e-10, "heading"=0.9797155560086303}, {"position"=4.048837209302326, "velocity"=23.72093023255814, "acceleration"=69.76744186046488, "jerk"=-1.4210854715202004e-10, "heading"=1.0061555172989665}, {"position"=4.168313953488373, "velocity"=24.069767441860463, "acceleration"=69.76744186046488, "jerk"=0.0, "heading"=1.0328111196443708}, {"position"=4.289534883720931, "velocity"=24.41860465116279, "acceleration"=69.7674418604656, "jerk"=1.4210854715202004e-10, "heading"=1.0596748395743365}, {"position"=4.4125000000000005, "velocity"=24.767441860465116, "acceleration"=69.76744186046488, "jerk"=-1.4210854715202004e-10, "heading"=1.0867390469990363}, {"position"=4.537209302325582, "velocity"=25.11627906976744, "acceleration"=69.76744186046488, "jerk"=0.0, "heading"=1.113996045892882}, {"position"=4.663662790697675, "velocity"=25.46511627906977, "acceleration"=69.7674418604656, "jerk"=1.4210854715202004e-10, "heading"=1.1414380225643639}, {"position"=4.7918604651162795, "velocity"=25.813953488372093, "acceleration"=69.76744186046488, "jerk"=-1.4210854715202004e-10, "heading"=1.1690570899158705}, {"position"=4.921802325581396, "velocity"=26.162790697674417, "acceleration"=69.76744186046488, "jerk"=0.0, "heading"=1.1968452568223331}, {"position"=5.053488372093024, "velocity"=26.511627906976745, "acceleration"=69.7674418604656, "jerk"=1.4210854715202004e-10, "heading"=1.2247944440657652}, {"position"=5.186918604651163, "velocity"=26.86046511627907, "acceleration"=69.76744186046488, "jerk"=-1.4210854715202004e-10, "heading"=1.2528964847416273}, {"position"=5.322093023255815, "velocity"=27.209302325581394, "acceleration"=69.76744186046488, "jerk"=0.0, "heading"=1.2811431246579856}, {"position"=5.459011627906977, "velocity"=27.558139534883722, "acceleration"=69.7674418604656, "jerk"=1.4210854715202004e-10, "heading"=1.3095260227271406}, {"position"=5.597674418604652, "velocity"=27.906976744186046, "acceleration"=69.76744186046488, "jerk"=-1.4210854715202004e-10, "heading"=1.338036737022612}, {"position"=5.738081395348838, "velocity"=28.25581395348837, "acceleration"=69.76744186046488, "jerk"=0.0, "heading"=1.366666755859957}, {"position"=5.880232558139536, "velocity"=28.6046511627907, "acceleration"=69.7674418604656, "jerk"=1.4210854715202004e-10, "heading"=1.3954074560265044}, {"position"=6.024127906976745, "velocity"=28.953488372093023, "acceleration"=69.76744186046488, "jerk"=-1.4210854715202004e-10, "heading"=1.4242501522466158}, {"position"=6.169767441860466, "velocity"=29.302325581395348, "acceleration"=69.76744186046488, "jerk"=0.0, "heading"=1.453186061092315}, {"position"=6.317151162790698, "velocity"=29.651162790697676, "acceleration"=69.7674418604656, "jerk"=1.4210854715202004e-10, "heading"=1.4822063152983773}, {"position"=6.466279069767443, "velocity"=30.0, "acceleration"=69.76744186046488, "jerk"=-1.4210854715202004e-10, "heading"=1.5113019552248577}, {"position"=6.617151162790698, "velocity"=30.348837209302324, "acceleration"=69.76744186046488, "jerk"=0.0, "heading"=1.5404639488166272}, {"position"=6.769767441860465, "velocity"=30.697674418604652, "acceleration"=69.7674418604656, "jerk"=1.4210854715202004e-10, "heading"=1.569683173491536}, {"position"=6.924127906976745, "velocity"=31.04651162790698, "acceleration"=69.7674418604656, "jerk"=0.0, "heading"=1.5989504232274532}, {"position"=7.080232558139535, "velocity"=31.395348837209298, "acceleration"=69.76744186046346, "jerk"=-4.263256414560601e-10, "heading"=1.6282564019591845}, {"position"=7.238081395348837, "velocity"=31.74418604651163, "acceleration"=69.7674418604663, "jerk"=5.684341886080801e-10, "heading"=1.6575917431493925}, {"position"=7.397674418604652, "velocity"=32.093023255813954, "acceleration"=69.76744186046488, "jerk"=-2.842170943040401e-10, "heading"=1.6869469906223111}, {"position"=7.559011627906977, "velocity"=32.44186046511628, "acceleration"=69.76744186046488, "jerk"=0.0, "heading"=1.7163126063624752}, {"position"=7.722093023255814, "velocity"=32.7906976744186, "acceleration"=69.76744186046488, "jerk"=0.0, "heading"=1.745678964667994}, {"position"=7.8869186046511635, "velocity"=33.13953488372093, "acceleration"=69.76744186046488, "jerk"=0.0, "heading"=1.7750363747711322}, {"position"=8.053488372093025, "velocity"=33.48837209302326, "acceleration"=69.7674418604663, "jerk"=2.842170943040401e-10, "heading"=1.804375044970975}, {"position"=8.221802325581397, "velocity"=33.83720930232558, "acceleration"=69.76744186046488, "jerk"=-2.842170943040401e-10, "heading"=1.8336851196535113}, {"position"=8.391860465116281, "velocity"=34.18604651162791, "acceleration"=69.76744186046488, "jerk"=0.0, "heading"=1.8629566519324958}, {"position"=8.563662790697677, "velocity"=34.53488372093023, "acceleration"=69.76744186046488, "jerk"=0.0, "heading"=1.89217961644882}, {"position"=8.737209302325583, "velocity"=34.883720930232556, "acceleration"=69.76744186046488, "jerk"=0.0, "heading"=1.9213439094735618}, {"position"=8.912500000000001, "velocity"=35.23255813953488, "acceleration"=69.76744186046488, "jerk"=0.0, "heading"=1.9504393489910907}, {"position"=9.089534883720932, "velocity"=35.58139534883721, "acceleration"=69.7674418604663, "jerk"=2.842170943040401e-10, "heading"=1.979455674761847}, {"position"=9.268313953488374, "velocity"=35.93023255813954, "acceleration"=69.76744186046488, "jerk"=-2.842170943040401e-10, "heading"=2.00838253834123}, {"position"=9.448837209302328, "velocity"=36.27906976744186, "acceleration"=69.76744186046488, "jerk"=0.0, "heading"=2.0372095259896006}, {"position"=9.631104651162794, "velocity"=36.627906976744185, "acceleration"=69.76744186046488, "jerk"=0.0, "heading"=2.065926128493938}, {"position"=9.81511627906977, "velocity"=36.97674418604651, "acceleration"=69.76744186046488, "jerk"=0.0, "heading"=2.0945217726475356}, {"position"=10.000872093023258, "velocity"=37.325581395348834, "acceleration"=69.76744186046488, "jerk"=0.0, "heading"=2.12298580023067}, {"position"=10.188372093023258, "velocity"=37.674418604651166, "acceleration"=69.7674418604663, "jerk"=2.842170943040401e-10, "heading"=2.1513074751148866}, {"position"=10.37761627906977, "velocity"=38.02325581395349, "acceleration"=69.76744186046488, "jerk"=-2.842170943040401e-10, "heading"=2.1794759792131093}, {"position"=10.568604651162794, "velocity"=38.372093023255815, "acceleration"=69.76744186046488, "jerk"=0.0, "heading"=2.207480421082196}, {"position"=10.761337209302328, "velocity"=38.72093023255814, "acceleration"=69.76744186046488, "jerk"=0.0, "heading"=2.2353098305732506}, {"position"=10.955813953488374, "velocity"=39.06976744186046, "acceleration"=69.76744186046488, "jerk"=0.0, "heading"=2.2629531543274846}, {"position"=11.152034883720932, "velocity"=39.41860465116279, "acceleration"=69.76744186046488, "jerk"=0.0, "heading"=2.2903992626731315}, {"position"=11.350000000000001, "velocity"=39.76744186046512, "acceleration"=69.7674418604663, "jerk"=2.842170943040401e-10, "heading"=2.3176369496115474}, {"position"=11.549709302325583, "velocity"=40.116279069767444, "acceleration"=69.76744186046488, "jerk"=-2.842170943040401e-10, "heading"=2.344654927662613}, {"position"=11.751162790697677, "velocity"=40.46511627906977, "acceleration"=69.76744186046488, "jerk"=0.0, "heading"=2.37144183126522}, {"position"=11.954360465116281, "velocity"=40.81395348837209, "acceleration"=69.76744186046488, "jerk"=0.0, "heading"=2.3979862128374756}, {"position"=12.159302325581397, "velocity"=41.16279069767442, "acceleration"=69.76744186046488, "jerk"=0.0, "heading"=2.4242765489829883}, {"position"=12.365988372093025, "velocity"=41.51162790697674, "acceleration"=69.76744186046488, "jerk"=0.0, "heading"=2.450301236139978}, {"position"=12.574418604651164, "velocity"=41.86046511627907, "acceleration"=69.7674418604663, "jerk"=2.842170943040401e-10, "heading"=2.476048589548517}, {"position"=12.784593023255816, "velocity"=42.2093023255814, "acceleration"=69.76744186046488, "jerk"=-2.842170943040401e-10, "heading"=2.5015068412031445}, {"position"=12.99651162790698, "velocity"=42.55813953488372, "acceleration"=69.76744186046488, "jerk"=0.0, "heading"=2.5266641481338583}, {"position"=13.210174418604653, "velocity"=42.906976744186046, "acceleration"=69.76744186046488, "jerk"=0.0, "heading"=2.5515085829289954}, {"position"=13.42558139534884, "velocity"=43.25581395348837, "acceleration"=69.76744186046488, "jerk"=0.0, "heading"=2.576028135683339}, {"position"=13.642732558139537, "velocity"=43.604651162790695, "acceleration"=69.76744186046488, "jerk"=0.0, "heading"=2.6002107146039033}, {"position"=13.861627906976747, "velocity"=43.95348837209303, "acceleration"=69.7674418604663, "jerk"=2.842170943040401e-10, "heading"=2.6240441491778306}, {"position"=14.082267441860468, "velocity"=44.30232558139535, "acceleration"=69.76744186046488, "jerk"=-2.842170943040401e-10, "heading"=2.64751617717895}, {"position"=14.3046511627907, "velocity"=44.651162790697676, "acceleration"=69.76744186046488, "jerk"=0.0, "heading"=2.670614461246025}, {"position"=14.528779069767443, "velocity"=45.0, "acceleration"=69.76744186046488, "jerk"=0.0, "heading"=2.693326574052145}, {"position"=14.754651162790699, "velocity"=45.348837209302324, "acceleration"=69.76744186046488, "jerk"=0.0, "heading"=2.7156400035407895}, {"position"=14.982267441860467, "velocity"=45.69767441860465, "acceleration"=69.76744186046488, "jerk"=0.0, "heading"=2.737542152002616}, {"position"=15.211627906976746, "velocity"=46.04651162790697, "acceleration"=69.76744186046488, "jerk"=0.0, "heading"=2.759020335111042}, {"position"=15.442732558139538, "velocity"=46.395348837209305, "acceleration"=69.7674418604663, "jerk"=2.842170943040401e-10, "heading"=2.7800617809160584}, {"position"=15.67558139534884, "velocity"=46.74418604651163, "acceleration"=69.76744186046488, "jerk"=-2.842170943040401e-10, "heading"=2.80065362455149}, {"position"=15.910174418604653, "velocity"=47.093023255813954, "acceleration"=69.76744186046488, "jerk"=0.0, "heading"=2.8207829180221298}, {"position"=16.14651162790698, "velocity"=47.44186046511628, "acceleration"=69.76744186046488, "jerk"=0.0, "heading"=2.8404366171632507}, {"position"=16.384593023255814, "velocity"=47.7906976744186, "acceleration"=69.76744186046488, "jerk"=0.0, "heading"=2.859601587124571}, {"position"=16.62441860465116, "velocity"=48.13953488372093, "acceleration"=69.76744186046488, "jerk"=0.0, "heading"=2.8782646012016944}, {"position"=16.86598837209302, "velocity"=48.48837209302326, "acceleration"=69.7674418604663, "jerk"=2.842170943040401e-10, "heading"=2.896412337149113}, {"position"=17.109302325581393, "velocity"=48.83720930232558, "acceleration"=69.76744186046488, "jerk"=-2.842170943040401e-10, "heading"=2.914031376686008}, {"position"=17.354360465116276, "velocity"=49.18604651162791, "acceleration"=69.76744186046488, "jerk"=0.0, "heading"=2.9311082066713525}, {"position"=17.60116279069767, "velocity"=49.53488372093023, "acceleration"=69.76744186046488, "jerk"=0.0, "heading"=2.9476292134639954}, {"position"=17.84970930232558, "velocity"=49.883720930232556, "acceleration"=69.76744186046488, "jerk"=0.0, "heading"=2.9635806854190205}, {"position"=18.099999999999998, "velocity"=50.23255813953488, "acceleration"=69.76744186046488, "jerk"=0.0, "heading"=2.9789488075289725}, {"position"=18.35203488372093, "velocity"=50.58139534883721, "acceleration"=69.7674418604663, "jerk"=2.842170943040401e-10, "heading"=2.9937196644080037}, {"position"=18.605813953488372, "velocity"=50.93023255813954, "acceleration"=69.76744186046488, "jerk"=-2.842170943040401e-10, "heading"=3.0078792351664423}, {"position"=18.861337209302327, "velocity"=51.27906976744186, "acceleration"=69.76744186046488, "jerk"=0.0, "heading"=3.0214133929243694}, {"position"=19.11860465116279, "velocity"=51.627906976744185, "acceleration"=69.76744186046488, "jerk"=0.0, "heading"=3.0343079025356525}, {"position"=19.377616279069766, "velocity"=51.97674418604651, "acceleration"=69.76744186046488, "jerk"=0.0, "heading"=3.0465484206140467}, {"position"=19.638372093023253, "velocity"=52.325581395348834, "acceleration"=69.76744186046488, "jerk"=0.0, "heading"=3.0581204908709068}, {"position"=19.900872093023253, "velocity"=52.674418604651166, "acceleration"=69.7674418604663, "jerk"=2.842170943040401e-10, "heading"=3.0690095446313803}, {"position"=20.165116279069764, "velocity"=53.02325581395349, "acceleration"=69.76744186046488, "jerk"=-2.842170943040401e-10, "heading"=3.07920089707189}, {"position"=20.431104651162787, "velocity"=53.372093023255815, "acceleration"=69.76744186046488, "jerk"=0.0, "heading"=3.0886797461317217}, {"position"=20.698837209302322, "velocity"=53.72093023255814, "acceleration"=69.76744186046488, "jerk"=0.0, "heading"=3.0974311702185973}, {"position"=20.96831395348837, "velocity"=54.06976744186046, "acceleration"=69.76744186046488, "jerk"=0.0, "heading"=3.105440125695439}, {"position"=21.23953488372093, "velocity"=54.41860465116279, "acceleration"=69.76744186046488, "jerk"=0.0, "heading"=3.1126914449576137}, {"position"=21.5125, "velocity"=54.76744186046512, "acceleration"=69.7674418604663, "jerk"=2.842170943040401e-10, "heading"=3.1191698336777245}, {"position"=21.787209302325582, "velocity"=55.116279069767444, "acceleration"=69.76744186046488, "jerk"=-2.842170943040401e-10, "heading"=3.124859868531654}, {"position"=22.063662790697677, "velocity"=55.46511627906977, "acceleration"=69.76744186046488, "jerk"=0.0, "heading"=3.129745994793289}, {"position"=22.34186046511628, "velocity"=55.81395348837209, "acceleration"=69.76744186046488, "jerk"=0.0, "heading"=3.1338125236335994}, {"position"=22.621802325581395, "velocity"=56.16279069767442, "acceleration"=69.76744186046488, "jerk"=0.0, "heading"=3.137043629422181}, {"position"=22.903488372093022, "velocity"=56.51162790697674, "acceleration"=69.76744186046488, "jerk"=0.0, "heading"=3.139423347033805}, {"position"=23.18691860465116, "velocity"=56.86046511627907, "acceleration"=69.7674418604663, "jerk"=2.842170943040401e-10, "heading"=3.1409355690008027}, {"position"=23.472093023255812, "velocity"=57.2093023255814, "acceleration"=69.76744186046488, "jerk"=-2.842170943040401e-10, "heading"=3.141564042601281}, {"position"=23.759011627906975, "velocity"=57.55813953488372, "acceleration"=69.76744186046488, "jerk"=0.0, "heading"=3.1412923668781363}, {"position"=24.047616279069768, "velocity"=57.883720930232556, "acceleration"=65.11627906976685, "jerk"=-930.2325581396076, "heading"=3.140104321319296}, {"position"=24.337790697674418, "velocity"=58.18604651162791, "acceleration"=60.46511627907023, "jerk"=-930.2325581393234, "heading"=3.137984792341781}, {"position"=24.62941860465116, "velocity"=58.46511627906977, "acceleration"=55.81395348837219, "jerk"=-930.2325581396076, "heading"=3.134920010820801}, {"position"=24.92238372093023, "velocity"=58.72093023255814, "acceleration"=51.162790697674154, "jerk"=-930.2325581396076, "heading"=3.13089756908227}, {"position"=25.216569767441857, "velocity"=58.95348837209303, "acceleration"=46.51162790697754, "jerk"=-930.2325581393234, "heading"=3.1259064368131315}, {"position"=25.511860465116275, "velocity"=59.16279069767442, "acceleration"=41.86046511627808, "jerk"=-930.2325581398918, "heading"=3.119936975905771}, {"position"=25.80813953488372, "velocity"=59.348837209302324, "acceleration"=37.20930232558146, "jerk"=-930.2325581393234, "heading"=3.112980954250695}, {"position"=26.105290697674416, "velocity"=59.51162790697674, "acceleration"=32.55813953488342, "jerk"=-930.2325581396076, "heading"=3.1050315584753325}, {"position"=26.403197674418603, "velocity"=59.651162790697676, "acceleration"=27.906976744186807, "jerk"=-930.2325581393234, "heading"=3.096083405307147}, {"position"=26.70174418604651, "velocity"=59.76744186046512, "acceleration"=23.25581395348877, "jerk"=-930.2325581396076, "heading"=3.0861325532014163}, {"position"=27.00081395348837, "velocity"=59.86046511627907, "acceleration"=18.60465116279073, "jerk"=-930.2325581396076, "heading"=3.0751765108267173}, {"position"=27.30029069767442, "velocity"=59.93023255813954, "acceleration"=13.953488372092693, "jerk"=-930.2325581396076, "heading"=3.0632142467146397}, {"position"=27.600058139534884, "velocity"=59.97674418604651, "acceleration"=9.302325581394655, "jerk"=-930.2325581396076, "heading"=3.050246196327391}, {"position"=27.9, "velocity"=60.0, "acceleration"=4.651162790698038, "jerk"=-930.2325581393234, "heading"=3.0362742692331857}, {"position"=28.2, "velocity"=60.0, "acceleration"=0.0, "jerk"=-930.2325581396076, "heading"=3.0213018540916043}, {"position"=28.5, "velocity"=60.0, "acceleration"=0.0, "jerk"=0.0, "heading"=3.0053306325821}, {"position"=28.8, "velocity"=60.0, "acceleration"=0.0, "jerk"=0.0, "heading"=2.9883596119055014}, {"position"=29.1, "velocity"=60.0, "acceleration"=0.0, "jerk"=0.0, "heading"=2.97038774003294}, {"position"=29.400000000000002, "velocity"=60.0, "acceleration"=0.0, "jerk"=0.0, "heading"=2.951413900523942}, {"position"=29.700000000000003, "velocity"=60.0, "acceleration"=0.0, "jerk"=0.0, "heading"=2.9314369194305616}, {"position"=30.000000000000004, "velocity"=60.0, "acceleration"=0.0, "jerk"=0.0, "heading"=2.910455558017224}, {"position"=30.300000000000004, "velocity"=60.0, "acceleration"=0.0, "jerk"=0.0, "heading"=2.8884685194247752}, {"position"=30.600000000000005, "velocity"=60.0, "acceleration"=0.0, "jerk"=0.0, "heading"=2.8654744437712343}, {"position"=30.900000000000006, "velocity"=60.0, "acceleration"=0.0, "jerk"=0.0, "heading"=2.8414719110315856}, {"position"=31.200000000000006, "velocity"=60.0, "acceleration"=0.0, "jerk"=0.0, "heading"=2.8164594411984245}, {"position"=31.500000000000007, "velocity"=60.0, "acceleration"=0.0, "jerk"=0.0, "heading"=2.790435490762797}, {"position"=31.800000000000008, "velocity"=60.0, "acceleration"=0.0, "jerk"=0.0, "heading"=2.7633984603196318}, {"position"=32.10000000000001, "velocity"=60.0, "acceleration"=0.0, "jerk"=0.0, "heading"=2.735346683911323}, {"position"=32.400000000000006, "velocity"=60.0, "acceleration"=0.0, "jerk"=0.0, "heading"=2.7062784414261625}, {"position"=32.7, "velocity"=60.0, "acceleration"=0.0, "jerk"=0.0, "heading"=2.676191948230581}, {"position"=33.0, "velocity"=60.0, "acceleration"=0.0, "jerk"=0.0, "heading"=2.6450853606970757}, {"position"=33.3, "velocity"=60.0, "acceleration"=0.0, "jerk"=0.0, "heading"=2.612956778057081}, {"position"=33.599999999999994, "velocity"=60.0, "acceleration"=0.0, "jerk"=0.0, "heading"=2.5798042323875965}, {"position"=33.89999999999999, "velocity"=60.0, "acceleration"=0.0, "jerk"=0.0, "heading"=2.545625706082946}, {"position"=34.19999999999999, "velocity"=60.0, "acceleration"=0.0, "jerk"=0.0, "heading"=2.5104191144233865}, {"position"=34.499999999999986, "velocity"=60.0, "acceleration"=0.0, "jerk"=0.0, "heading"=2.4741823158632097}, {"position"=34.79999999999998, "velocity"=60.0, "acceleration"=0.0, "jerk"=0.0, "heading"=2.4369131130866175}, {"position"=35.09999999999998, "velocity"=60.0, "acceleration"=0.0, "jerk"=0.0, "heading"=2.3986092411466307}, {"position"=35.39999999999998, "velocity"=60.0, "acceleration"=0.0, "jerk"=0.0, "heading"=2.359268386977859}, {"position"=35.699999999999974, "velocity"=60.0, "acceleration"=0.0, "jerk"=0.0, "heading"=2.318888173831744}, {"position"=35.99999999999997, "velocity"=60.0, "acceleration"=0.0, "jerk"=0.0, "heading"=2.2774661625122836}, {"position"=36.29999999999997, "velocity"=60.0, "acceleration"=0.0, "jerk"=0.0, "heading"=2.2349998662342867}, {"position"=36.599999999999966, "velocity"=60.0, "acceleration"=0.0, "jerk"=0.0, "heading"=2.1914867321019007}, {"position"=36.89999999999996, "velocity"=60.0, "acceleration"=0.0, "jerk"=0.0, "heading"=2.146924150069533}, {"position"=37.19999999999996, "velocity"=60.0, "acceleration"=0.0, "jerk"=0.0, "heading"=2.101309460216741}, {"position"=37.49999999999996, "velocity"=60.0, "acceleration"=0.0, "jerk"=0.0, "heading"=2.054639937611325}, {"position"=37.799999999999955, "velocity"=60.0, "acceleration"=0.0, "jerk"=0.0, "heading"=2.006912802002701}, {"position"=38.09999999999995, "velocity"=60.0, "acceleration"=0.0, "jerk"=0.0, "heading"=1.9581252238559423}, {"position"=38.39999999999995, "velocity"=60.0, "acceleration"=0.0, "jerk"=0.0, "heading"=1.9082743105618172}, {"position"=38.699999999999946, "velocity"=60.0, "acceleration"=0.0, "jerk"=0.0, "heading"=1.8573571115214296}, {"position"=38.99999999999994, "velocity"=60.0, "acceleration"=0.0, "jerk"=0.0, "heading"=1.8053706320549743}, {"position"=39.29999999999994, "velocity"=60.0, "acceleration"=0.0, "jerk"=0.0, "heading"=1.7523118162175126}, {"position"=39.59999999999994, "velocity"=60.0, "acceleration"=0.0, "jerk"=0.0, "heading"=1.6981775453257764}, {"position"=39.899999999999935, "velocity"=60.0, "acceleration"=0.0, "jerk"=0.0, "heading"=1.642964661763133}, {"position"=40.19999999999993, "velocity"=60.0, "acceleration"=0.0, "jerk"=0.0, "heading"=1.5866699487119975}, {"position"=40.49999999999993, "velocity"=60.0, "acceleration"=0.0, "jerk"=0.0, "heading"=1.529290133296062}, {"position"=40.799999999999926, "velocity"=60.0, "acceleration"=0.0, "jerk"=0.0, "heading"=1.4708218856799717}, {"position"=41.09999999999992, "velocity"=60.0, "acceleration"=0.0, "jerk"=0.0, "heading"=1.4112618376376207}, {"position"=41.39999999999992, "velocity"=60.0, "acceleration"=0.0, "jerk"=0.0, "heading"=1.3506065617101926}, {"position"=41.69999999999992, "velocity"=60.0, "acceleration"=0.0, "jerk"=0.0, "heading"=1.28885257886985}, {"position"=41.999999999999915, "velocity"=60.0, "acceleration"=0.0, "jerk"=0.0, "heading"=1.2259963512992815}, {"position"=42.29999999999991, "velocity"=60.0, "acceleration"=0.0, "jerk"=0.0, "heading"=1.1620343089223144}, {"position"=42.59999999999991, "velocity"=60.0, "acceleration"=0.0, "jerk"=0.0, "heading"=1.0969628233698008}, {"position"=42.899999999999906, "velocity"=60.0, "acceleration"=0.0, "jerk"=0.0, "heading"=1.0307782175549116}, {"position"=43.1999999999999, "velocity"=60.0, "acceleration"=0.0, "jerk"=0.0, "heading"=0.9634767647459053}, {"position"=43.4999999999999, "velocity"=60.0, "acceleration"=0.0, "jerk"=0.0, "heading"=0.8950546864931762}, {"position"=43.7999999999999, "velocity"=60.0, "acceleration"=0.0, "jerk"=0.0, "heading"=0.825508171049138}, {"position"=44.099999999999895, "velocity"=60.0, "acceleration"=0.0, "jerk"=0.0, "heading"=0.754833353315974}, {"position"=44.39999999999989, "velocity"=60.0, "acceleration"=0.0, "jerk"=0.0, "heading"=0.6830263230283563}, {"position"=44.69999999999989, "velocity"=60.0, "acceleration"=0.0, "jerk"=0.0, "heading"=0.6100831255482685}, {"position"=44.999999999999886, "velocity"=60.0, "acceleration"=0.0, "jerk"=0.0, "heading"=0.5359997626902745}, {"position"=45.29999999999988, "velocity"=60.0, "acceleration"=0.0, "jerk"=0.0, "heading"=0.4607721878200035}, {"position"=45.59999999999988, "velocity"=60.0, "acceleration"=0.0, "jerk"=0.0, "heading"=0.3843963226220532}, {"position"=45.89999999999988, "velocity"=60.0, "acceleration"=0.0, "jerk"=0.0, "heading"=0.30686804517525423}, {"position"=46.199999999999875, "velocity"=60.0, "acceleration"=0.0, "jerk"=0.0, "heading"=0.22818319204183646}, {"position"=46.49999999999987, "velocity"=60.0, "acceleration"=0.0, "jerk"=0.0, "heading"=0.14833756085160393}, {"position"=46.79999999999987, "velocity"=60.0, "acceleration"=0.0, "jerk"=0.0, "heading"=0.0673269113287741}, {"position"=47.099999999999866, "velocity"=60.0, "acceleration"=0.0, "jerk"=0.0, "heading"=359.9851469663557}, {"position"=47.399999999999864, "velocity"=60.0, "acceleration"=0.0, "jerk"=0.0, "heading"=359.9017934130748}, {"position"=47.69999999999986, "velocity"=60.0, "acceleration"=0.0, "jerk"=0.0, "heading"=359.81726190402895}, {"position"=47.99999999999986, "velocity"=60.0, "acceleration"=0.0, "jerk"=0.0, "heading"=359.7315480583423}, {"position"=48.299999999999855, "velocity"=60.0, "acceleration"=0.0, "jerk"=0.0, "heading"=359.6446474629422}, {"position"=48.59999999999985, "velocity"=60.0, "acceleration"=0.0, "jerk"=0.0, "heading"=359.5565556738228}, {"position"=48.89999999999985, "velocity"=60.0, "acceleration"=0.0, "jerk"=0.0, "heading"=359.46726821735206}, {"position"=49.19999999999985, "velocity"=60.0, "acceleration"=0.0, "jerk"=0.0, "heading"=359.37678059162283}, {"position"=49.499999999999844, "velocity"=60.0, "acceleration"=0.0, "jerk"=0.0, "heading"=359.28508826784963}, {"position"=49.79999999999984, "velocity"=60.0, "acceleration"=0.0, "jerk"=0.0, "heading"=359.19218669181106}, {"position"=50.09999999999984, "velocity"=60.0, "acceleration"=0.0, "jerk"=0.0, "heading"=359.0980712853405}, {"position"=50.399999999999835, "velocity"=60.0, "acceleration"=0.0, "jerk"=0.0, "heading"=359.0027374478649}, {"position"=50.69999999999983, "velocity"=60.0, "acceleration"=0.0, "jerk"=0.0, "heading"=358.90618055799337}, {"position"=50.99999999999983, "velocity"=60.0, "acceleration"=0.0, "jerk"=0.0, "heading"=358.8083959751568}, {"position"=51.29999999999983, "velocity"=60.0, "acceleration"=0.0, "jerk"=0.0, "heading"=358.7093790412995}, {"position"=51.599999999999824, "velocity"=60.0, "acceleration"=0.0, "jerk"=0.0, "heading"=358.609125082623}, {"position"=51.89999999999982, "velocity"=60.0, "acceleration"=0.0, "jerk"=0.0, "heading"=358.5076294113855}, {"position"=52.19999999999982, "velocity"=60.0, "acceleration"=0.0, "jerk"=0.0, "heading"=358.40488732775594}, {"position"=52.499999999999815, "velocity"=60.0, "acceleration"=0.0, "jerk"=0.0, "heading"=358.3008941217239}, {"position"=52.79999999999981, "velocity"=60.0, "acceleration"=0.0, "jerk"=0.0, "heading"=358.1956450696213}, {"position"=53.09999999999981, "velocity"=60.0, "acceleration"=0.0, "jerk"=0.0, "heading"=358.0891354433747}, {"position"=53.39999999999981, "velocity"=60.0, "acceleration"=0.0, "jerk"=0.0, "heading"=357.98136052202074}, {"position"=53.699999999999804, "velocity"=60.0, "acceleration"=0.0, "jerk"=0.0, "heading"=357.8723155750581}, {"position"=53.9999999999998, "velocity"=60.0, "acceleration"=0.0, "jerk"=0.0, "heading"=357.7619958722473}, {"position"=54.2999999999998, "velocity"=60.0, "acceleration"=0.0, "jerk"=0.0, "heading"=357.6503966858842}, {"position"=54.599999999999795, "velocity"=60.0, "acceleration"=0.0, "jerk"=0.0, "heading"=357.53751328158427}, {"position"=54.89999999999979, "velocity"=60.0, "acceleration"=0.0, "jerk"=0.0, "heading"=357.4233409435479}, {"position"=55.19999999999979, "velocity"=60.0, "acceleration"=0.0, "jerk"=0.0, "heading"=357.30787497588756}, {"position"=55.49999999999979, "velocity"=60.0, "acceleration"=0.0, "jerk"=0.0, "heading"=357.19111068503247}, {"position"=55.799999999999784, "velocity"=60.0, "acceleration"=0.0, "jerk"=0.0, "heading"=357.0730433874246}, {"position"=56.09999999999978, "velocity"=60.0, "acceleration"=0.0, "jerk"=0.0, "heading"=356.95366840195754}, {"position"=56.39999999999978, "velocity"=60.0, "acceleration"=0.0, "jerk"=0.0, "heading"=356.8329811106454}, {"position"=56.699999999999775, "velocity"=60.0, "acceleration"=0.0, "jerk"=0.0, "heading"=356.7109768957722}, {"position"=56.99999999999977, "velocity"=60.0, "acceleration"=0.0, "jerk"=0.0, "heading"=356.5876511461136}, {"position"=57.29999999999977, "velocity"=60.0, "acceleration"=0.0, "jerk"=0.0, "heading"=356.46299930117016}, {"position"=57.59999999999977, "velocity"=60.0, "acceleration"=0.0, "jerk"=0.0, "heading"=356.3370168453728}, {"position"=57.899999999999764, "velocity"=60.0, "acceleration"=0.0, "jerk"=0.0, "heading"=356.20969926688156}, {"position"=58.19999999999976, "velocity"=60.0, "acceleration"=0.0, "jerk"=0.0, "heading"=356.08104209867196}, {"position"=58.49999999999976, "velocity"=60.0, "acceleration"=0.0, "jerk"=0.0, "heading"=355.95104094878354}, {"position"=58.799999999999756, "velocity"=60.0, "acceleration"=0.0, "jerk"=0.0, "heading"=355.81969142043374}, {"position"=59.09999999999975, "velocity"=60.0, "acceleration"=0.0, "jerk"=0.0, "heading"=355.6869891952544}, {"position"=59.39999999999975, "velocity"=60.0, "acceleration"=0.0, "jerk"=0.0, "heading"=355.55293002224425}, {"position"=59.69999999999975, "velocity"=60.0, "acceleration"=0.0, "jerk"=0.0, "heading"=355.4175096364191}, {"position"=59.999999999999744, "velocity"=60.0, "acceleration"=0.0, "jerk"=0.0, "heading"=355.2807239274554}, {"position"=60.29999999999974, "velocity"=60.0, "acceleration"=0.0, "jerk"=0.0, "heading"=355.14256877268133}, {"position"=60.59999999999974, "velocity"=60.0, "acceleration"=0.0, "jerk"=0.0, "heading"=355.0030401499917}, {"position"=60.899999999999736, "velocity"=60.0, "acceleration"=0.0, "jerk"=0.0, "heading"=354.8621341094264}, {"position"=61.19999999999973, "velocity"=60.0, "acceleration"=0.0, "jerk"=0.0, "heading"=354.719846743895}, {"position"=61.49999999999973, "velocity"=60.0, "acceleration"=0.0, "jerk"=0.0, "heading"=354.57617428059507}, {"position"=61.79999999999973, "velocity"=60.0, "acceleration"=0.0, "jerk"=0.0, "heading"=354.4311129554461}, {"position"=62.099999999999724, "velocity"=60.0, "acceleration"=0.0, "jerk"=0.0, "heading"=354.2846591773885}, {"position"=62.39999999999972, "velocity"=60.0, "acceleration"=0.0, "jerk"=0.0, "heading"=354.136809354429}, {"position"=62.69999999999972, "velocity"=60.0, "acceleration"=0.0, "jerk"=0.0, "heading"=353.9875600820943}, {"position"=62.999999999999716, "velocity"=60.0, "acceleration"=0.0, "jerk"=0.0, "heading"=353.83690797050315}, {"position"=63.29999999999971, "velocity"=60.0, "acceleration"=0.0, "jerk"=0.0, "heading"=353.6848498069999}, {"position"=63.59999999999971, "velocity"=60.0, "acceleration"=0.0, "jerk"=0.0, "heading"=353.53138243463667}, {"position"=63.89999999999971, "velocity"=60.0, "acceleration"=0.0, "jerk"=0.0, "heading"=353.3765028383323}, {"position"=64.1999999999997, "velocity"=60.0, "acceleration"=0.0, "jerk"=0.0, "heading"=353.2202081255224}, {"position"=64.4999999999997, "velocity"=60.0, "acceleration"=0.0, "jerk"=0.0, "heading"=353.0624954851308}, {"position"=64.7999999999997, "velocity"=60.0, "acceleration"=0.0, "jerk"=0.0, "heading"=352.90336230707584}, {"position"=65.0999999999997, "velocity"=60.0, "acceleration"=0.0, "jerk"=0.0, "heading"=352.7428060329243}, {"position"=65.3999999999997, "velocity"=60.0, "acceleration"=0.0, "jerk"=0.0, "heading"=352.58082430686284}, {"position"=65.69999999999969, "velocity"=60.0, "acceleration"=0.0, "jerk"=0.0, "heading"=352.41741490205237}, {"position"=65.99999999999969, "velocity"=60.0, "acceleration"=0.0, "jerk"=0.0, "heading"=352.25257568654155}, {"position"=66.29999999999968, "velocity"=60.0, "acceleration"=0.0, "jerk"=0.0, "heading"=352.08630477146795}, {"position"=66.59999999999968, "velocity"=60.0, "acceleration"=0.0, "jerk"=0.0, "heading"=351.9186003753866}, {"position"=66.89999999999968, "velocity"=60.0, "acceleration"=0.0, "jerk"=0.0, "heading"=351.74946085504797}, {"position"=67.19999999999968, "velocity"=60.0, "acceleration"=0.0, "jerk"=0.0, "heading"=351.5788848082114}, {"position"=67.49999999999967, "velocity"=60.0, "acceleration"=0.0, "jerk"=0.0, "heading"=351.40687096930935}, {"position"=67.79999999999967, "velocity"=60.0, "acceleration"=0.0, "jerk"=0.0, "heading"=351.2334182204197}, {"position"=68.09999999999967, "velocity"=60.0, "acceleration"=0.0, "jerk"=0.0, "heading"=351.0585256949433}, {"position"=68.39999999999966, "velocity"=60.0, "acceleration"=0.0, "jerk"=0.0, "heading"=350.8821926920199}, {"position"=68.69999999999966, "velocity"=60.0, "acceleration"=0.0, "jerk"=0.0, "heading"=350.70441869663244}, {"position"=68.99999999999966, "velocity"=60.0, "acceleration"=0.0, "jerk"=0.0, "heading"=350.52520338963694}, {"position"=69.29999999999966, "velocity"=60.0, "acceleration"=0.0, "jerk"=0.0, "heading"=350.344546702711}, {"position"=69.59999999999965, "velocity"=60.0, "acceleration"=0.0, "jerk"=0.0, "heading"=350.16244875730285}, {"position"=69.89999999999965, "velocity"=60.0, "acceleration"=0.0, "jerk"=0.0, "heading"=349.97890989565013}, {"position"=70.19999999999965, "velocity"=60.0, "acceleration"=0.0, "jerk"=0.0, "heading"=349.79393066198753}, {"position"=70.49999999999964, "velocity"=60.0, "acceleration"=0.0, "jerk"=0.0, "heading"=349.6075118856016}, {"position"=70.79999999999964, "velocity"=60.0, "acceleration"=0.0, "jerk"=0.0, "heading"=349.41965460707087}, {"position"=71.09999999999964, "velocity"=60.0, "acceleration"=0.0, "jerk"=0.0, "heading"=349.2303601113068}, {"position"=71.39999999999964, "velocity"=60.0, "acceleration"=0.0, "jerk"=0.0, "heading"=349.0396299333754}, {"position"=71.69999999999963, "velocity"=60.0, "acceleration"=0.0, "jerk"=0.0, "heading"=348.84746584781874}, {"position"=71.99999999999963, "velocity"=60.0, "acceleration"=0.0, "jerk"=0.0, "heading"=348.6538699231021}, {"position"=72.29999999999963, "velocity"=60.0, "acceleration"=0.0, "jerk"=0.0, "heading"=348.45884448200104}, {"position"=72.59999999999962, "velocity"=60.0, "acceleration"=0.0, "jerk"=0.0, "heading"=348.2623921180848}, {"position"=72.89999999999962, "velocity"=60.0, "acceleration"=0.0, "jerk"=0.0, "heading"=348.0645157038915}, {"position"=73.19999999999962, "velocity"=60.0, "acceleration"=0.0, "jerk"=0.0, "heading"=347.86521839658724}, {"position"=73.49999999999962, "velocity"=60.0, "acceleration"=0.0, "jerk"=0.0, "heading"=347.66450364214353}, {"position"=73.79999999999961, "velocity"=60.0, "acceleration"=0.0, "jerk"=0.0, "heading"=347.4623751756024}, {"position"=74.09999999999961, "velocity"=60.0, "acceleration"=0.0, "jerk"=0.0, "heading"=347.2588370523254}, {"position"=74.39999999999961, "velocity"=60.0, "acceleration"=0.0, "jerk"=0.0, "heading"=347.05389362338565}, {"position"=74.6999999999996, "velocity"=60.0, "acceleration"=0.0, "jerk"=0.0, "heading"=346.8475495518405}, {"position"=74.9999999999996, "velocity"=60.0, "acceleration"=0.0, "jerk"=0.0, "heading"=346.6398098179595}, {"position"=75.2999999999996, "velocity"=60.0, "acceleration"=0.0, "jerk"=0.0, "heading"=346.4306797243524}, {"position"=75.5999999999996, "velocity"=60.0, "acceleration"=0.0, "jerk"=0.0, "heading"=346.220164900987}, {"position"=75.8999999999996, "velocity"=60.0, "acceleration"=0.0, "jerk"=0.0, "heading"=346.00827131008845}, {"position"=76.19999999999959, "velocity"=60.0, "acceleration"=0.0, "jerk"=0.0, "heading"=345.7950052509103}, {"position"=76.49999999999959, "velocity"=60.0, "acceleration"=0.0, "jerk"=0.0, "heading"=345.58037336436956}, {"position"=76.79999999999959, "velocity"=60.0, "acceleration"=0.0, "jerk"=0.0, "heading"=345.3643826350424}, {"position"=77.09999999999958, "velocity"=60.0, "acceleration"=0.0, "jerk"=0.0, "heading"=345.1470404025137}, {"position"=77.39999999999958, "velocity"=60.0, "acceleration"=0.0, "jerk"=0.0, "heading"=344.92835436026365}, {"position"=77.69999999999958, "velocity"=60.0, "acceleration"=0.0, "jerk"=0.0, "heading"=344.7083325591116}, {"position"=77.99999999999957, "velocity"=60.0, "acceleration"=0.0, "jerk"=0.0, "heading"=344.4869834123302}, {"position"=78.29999999999957, "velocity"=60.0, "acceleration"=0.0, "jerk"=0.0, "heading"=344.26431569925694}, {"position"=78.59999999999957, "velocity"=60.0, "acceleration"=0.0, "jerk"=0.0, "heading"=344.04033856870393}, {"position"=78.89999999999957, "velocity"=60.0, "acceleration"=0.0, "jerk"=0.0, "heading"=343.8150615421517}, {"position"=79.19999999999956, "velocity"=60.0, "acceleration"=0.0, "jerk"=0.0, "heading"=343.5884945167197}, {"position"=79.49999999999956, "velocity"=60.0, "acceleration"=0.0, "jerk"=0.0, "heading"=343.3606477679034}, {"position"=79.79999999999956, "velocity"=60.0, "acceleration"=0.0, "jerk"=0.0, "heading"=343.13153195206814}, {"position"=80.09999999999955, "velocity"=60.0, "acceleration"=0.0, "jerk"=0.0, "heading"=342.9011581086901}, {"position"=80.39999999999955, "velocity"=60.0, "acceleration"=0.0, "jerk"=0.0, "heading"=342.6695376623351}, {"position"=80.69999999999955, "velocity"=60.0, "acceleration"=0.0, "jerk"=0.0, "heading"=342.4366824243662}, {"position"=80.99999999999955, "velocity"=60.0, "acceleration"=0.0, "jerk"=0.0, "heading"=342.2026045943706}, {"position"=81.29999999999954, "velocity"=60.0, "acceleration"=0.0, "jerk"=0.0, "heading"=341.9673167612965}, {"position"=81.59999999999954, "velocity"=60.0, "acceleration"=0.0, "jerk"=0.0, "heading"=341.73083190429264}, {"position"=81.89999999999954, "velocity"=60.0, "acceleration"=0.0, "jerk"=0.0, "heading"=341.49316339603587}, {"position"=82.19999999999953, "velocity"=60.0, "acceleration"=0.0, "jerk"=0.0, "heading"=341.25432499640965}, {"position"=82.49999999999953, "velocity"=60.0, "acceleration"=0.0, "jerk"=0.0, "heading"=341.01433085659534}, {"position"=82.79999999999953, "velocity"=60.0, "acceleration"=0.0, "jerk"=0.0, "heading"=340.77319551883716}, {"position"=83.09999999999953, "velocity"=60.0, "acceleration"=0.0, "jerk"=0.0, "heading"=340.5309339150333}, {"position"=83.39999999999952, "velocity"=60.0, "acceleration"=0.0, "jerk"=0.0, "heading"=340.2875613656194}, {"position"=83.69999999999952, "velocity"=60.0, "acceleration"=0.0, "jerk"=0.0, "heading"=340.0430935781002}, {"position"=83.99999999999952, "velocity"=60.0, "acceleration"=0.0, "jerk"=0.0, "heading"=339.79754664522477}, {"position"=84.29999999999951, "velocity"=60.0, "acceleration"=0.0, "jerk"=0.0, "heading"=339.5509370427997}, {"position"=84.59999999999951, "velocity"=60.0, "acceleration"=0.0, "jerk"=0.0, "heading"=339.30328162713374}, {"position"=84.89999999999951, "velocity"=60.0, "acceleration"=0.0, "jerk"=0.0, "heading"=339.05459763211195}, {"position"=85.1999999999995, "velocity"=60.0, "acceleration"=0.0, "jerk"=0.0, "heading"=338.80490267625873}, {"position"=85.4999999999995, "velocity"=60.0, "acceleration"=0.0, "jerk"=0.0, "heading"=338.5542147395053}, {"position"=85.7999999999995, "velocity"=60.0, "acceleration"=0.0, "jerk"=0.0, "heading"=338.30255215973085}, {"position"=86.0999999999995, "velocity"=60.0, "acceleration"=0.0, "jerk"=0.0, "heading"=338.04993364471767}, {"position"=86.3999999999995, "velocity"=60.0, "acceleration"=0.0, "jerk"=0.0, "heading"=337.7963782595229}, {"position"=86.69999999999949, "velocity"=60.0, "acceleration"=0.0, "jerk"=0.0, "heading"=337.54190542125787}, {"position"=86.99999999999949, "velocity"=60.0, "acceleration"=0.0, "jerk"=0.0, "heading"=337.28653489395526}, {"position"=87.29999999999949, "velocity"=60.0, "acceleration"=0.0, "jerk"=0.0, "heading"=337.03028682349964}, {"position"=87.59999999999948, "velocity"=60.0, "acceleration"=0.0, "jerk"=0.0, "heading"=336.77318161262497}, {"position"=87.89999999999948, "velocity"=60.0, "acceleration"=0.0, "jerk"=0.0, "heading"=336.5152400273473}, {"position"=88.19999999999948, "velocity"=60.0, "acceleration"=0.0, "jerk"=0.0, "heading"=336.25648315388395}, {"position"=88.49999999999947, "velocity"=60.0, "acceleration"=0.0, "jerk"=0.0, "heading"=335.9969324135759}, {"position"=88.79999999999947, "velocity"=60.0, "acceleration"=0.0, "jerk"=0.0, "heading"=335.7366095377082}, {"position"=89.09999999999947, "velocity"=60.0, "acceleration"=0.0, "jerk"=0.0, "heading"=335.4755364867212}, {"position"=89.39999999999947, "velocity"=60.0, "acceleration"=0.0, "jerk"=0.0, "heading"=335.2137355495196}, {"position"=89.69999999999946, "velocity"=60.0, "acceleration"=0.0, "jerk"=0.0, "heading"=334.9512293552957}, {"position"=89.99999999999946, "velocity"=60.0, "acceleration"=0.0, "jerk"=0.0, "heading"=334.68804072489144}, {"position"=90.29999999999946, "velocity"=60.0, "acceleration"=0.0, "jerk"=0.0, "heading"=334.4241927245676}, {"position"=90.59999999999945, "velocity"=60.0, "acceleration"=0.0, "jerk"=0.0, "heading"=334.1597087707029}, {"position"=90.89999999999945, "velocity"=60.0, "acceleration"=0.0, "jerk"=0.0, "heading"=333.89461245173}, {"position"=91.19999999999945, "velocity"=60.0, "acceleration"=0.0, "jerk"=0.0, "heading"=333.6289275324357}, {"position"=91.49999999999945, "velocity"=60.0, "acceleration"=0.0, "jerk"=0.0, "heading"=333.3626781856576}, {"position"=91.79999999999944, "velocity"=60.0, "acceleration"=0.0, "jerk"=0.0, "heading"=333.0958885564024}, {"position"=92.09999999999944, "velocity"=60.0, "acceleration"=0.0, "jerk"=0.0, "heading"=332.82858315390007}, {"position"=92.39999999999944, "velocity"=60.0, "acceleration"=0.0, "jerk"=0.0, "heading"=332.5607866229386}, {"position"=92.69999999999943, "velocity"=60.0, "acceleration"=0.0, "jerk"=0.0, "heading"=332.2925237407398}, {"position"=92.99999999999943, "velocity"=60.0, "acceleration"=0.0, "jerk"=0.0, "heading"=332.02381955002625}, {"position"=93.29999999999943, "velocity"=60.0, "acceleration"=0.0, "jerk"=0.0, "heading"=331.7546991095418}, {"position"=93.59999999999943, "velocity"=60.0, "acceleration"=0.0, "jerk"=0.0, "heading"=331.48518773969425}, {"position"=93.89999999999942, "velocity"=60.0, "acceleration"=0.0, "jerk"=0.0, "heading"=331.2153108097843}, {"position"=94.19999999999942, "velocity"=60.0, "acceleration"=0.0, "jerk"=0.0, "heading"=330.9450937780892}, {"position"=94.49999999999942, "velocity"=60.0, "acceleration"=0.0, "jerk"=0.0, "heading"=330.6745623706433}, {"position"=94.79999999999941, "velocity"=60.0, "acceleration"=0.0, "jerk"=0.0, "heading"=330.40374212295796}, {"position"=95.09999999999941, "velocity"=60.0, "acceleration"=0.0, "jerk"=0.0, "heading"=330.1326588831375}, {"position"=95.39999999999941, "velocity"=60.0, "acceleration"=0.0, "jerk"=0.0, "heading"=329.8613384952707}, {"position"=95.6999999999994, "velocity"=60.0, "acceleration"=0.0, "jerk"=0.0, "heading"=329.5898067337357}, {"position"=95.9999999999994, "velocity"=60.0, "acceleration"=0.0, "jerk"=0.0, "heading"=329.31808950572236}, {"position"=96.2999999999994, "velocity"=60.0, "acceleration"=0.0, "jerk"=0.0, "heading"=329.04621285651365}, {"position"=96.5999999999994, "velocity"=60.0, "acceleration"=0.0, "jerk"=0.0, "heading"=328.7742026043232}, {"position"=96.8999999999994, "velocity"=60.0, "acceleration"=0.0, "jerk"=0.0, "heading"=328.50208465544296}, {"position"=97.19999999999939, "velocity"=60.0, "acceleration"=0.0, "jerk"=0.0, "heading"=328.2298849103816}, {"position"=97.49999999999939, "velocity"=60.0, "acceleration"=0.0, "jerk"=0.0, "heading"=327.9576292340178}, {"position"=97.79999999999939, "velocity"=60.0, "acceleration"=0.0, "jerk"=0.0, "heading"=327.6853434419135}, {"position"=98.09999999999938, "velocity"=60.0, "acceleration"=0.0, "jerk"=0.0, "heading"=327.41305328667704}, {"position"=98.39999999999938, "velocity"=60.0, "acceleration"=0.0, "jerk"=0.0, "heading"=327.1407844443942}, {"position"=98.69999999999938, "velocity"=60.0, "acceleration"=0.0, "jerk"=0.0, "heading"=326.86856250114397}, {"position"=98.99999999999937, "velocity"=60.0, "acceleration"=0.0, "jerk"=0.0, "heading"=326.5964129396183}, {"position"=99.29999999999937, "velocity"=60.0, "acceleration"=0.0, "jerk"=0.0, "heading"=326.3243611258627}, {"position"=99.59999999999937, "velocity"=60.0, "acceleration"=0.0, "jerk"=0.0, "heading"=326.05243229615616}, {"position"=99.89999999999937, "velocity"=60.0, "acceleration"=0.0, "jerk"=0.0, "heading"=325.7806515440451}, {"position"=100.19999999999936, "velocity"=60.0, "acceleration"=0.0, "jerk"=0.0, "heading"=325.50904380755145}, {"position"=100.49999999999936, "velocity"=60.0, "acceleration"=0.0, "jerk"=0.0, "heading"=325.2376338565677}, {"position"=100.79999999999936, "velocity"=60.0, "acceleration"=0.0, "jerk"=0.0, "heading"=324.9664463810751}, {"position"=101.09999999999935, "velocity"=60.0, "acceleration"=0.0, "jerk"=0.0, "heading"=324.6955058190776}, {"position"=101.39999999999935, "velocity"=60.0, "acceleration"=0.0, "jerk"=0.0, "heading"=324.4248362595259}, {"position"=101.69999999999935, "velocity"=60.0, "acceleration"=0.0, "jerk"=0.0, "heading"=324.1544617616717}, {"position"=101.99999999999935, "velocity"=60.0, "acceleration"=0.0, "jerk"=0.0, "heading"=323.8844062626207}, {"position"=102.29999999999934, "velocity"=60.0, "acceleration"=0.0, "jerk"=0.0, "heading"=323.6146930489122}, {"position"=102.59999999999934, "velocity"=60.0, "acceleration"=0.0, "jerk"=0.0, "heading"=323.3453457460521}, {"position"=102.89999999999934, "velocity"=60.0, "acceleration"=0.0, "jerk"=0.0, "heading"=323.0763871078567}, {"position"=103.19999999999933, "velocity"=60.0, "acceleration"=0.0, "jerk"=0.0, "heading"=322.807840233991}, {"position"=103.49999999999933, "velocity"=60.0, "acceleration"=0.0, "jerk"=0.0, "heading"=322.5397273291534}, {"position"=103.79999999999933, "velocity"=60.0, "acceleration"=0.0, "jerk"=0.0, "heading"=322.2720709856312}, {"position"=104.09999999999933, "velocity"=60.0, "acceleration"=0.0, "jerk"=0.0, "heading"=322.0048929085515}, {"position"=104.39999999999932, "velocity"=60.0, "acceleration"=0.0, "jerk"=0.0, "heading"=321.7382147407004}, {"position"=104.69999999999932, "velocity"=60.0, "acceleration"=0.0, "jerk"=0.0, "heading"=321.4720580544237}, {"position"=104.99999999999932, "velocity"=60.0, "acceleration"=0.0, "jerk"=0.0, "heading"=321.20644374681905}, {"position"=105.29999999999932, "velocity"=60.0, "acceleration"=0.0, "jerk"=0.0, "heading"=320.94139249712885}, {"position"=105.59999999999931, "velocity"=60.0, "acceleration"=0.0, "jerk"=0.0, "heading"=320.6769247101354}, {"position"=105.89999999999931, "velocity"=60.0, "acceleration"=0.0, "jerk"=0.0, "heading"=320.41306045078625}, {"position"=106.19997153467163, "velocity"=59.98861386892982, "acceleration"=-2.277226214036432, "jerk"=-455.4452428072864, "heading"=320.14984438538715}, {"position"=106.49982799915372, "velocity"=59.953971923906145, "acceleration"=-6.92838900473447, "jerk"=-930.2325581396076, "heading"=319.887371408766}, {"position"=106.79945311437581, "velocity"=59.896074164929, "acceleration"=-11.579551795429666, "jerk"=-930.2325581390392, "heading"=319.6257611459852}, {"position"=107.09873060126813, "velocity"=59.81492059199835, "acceleration"=-16.230714586129125, "jerk"=-930.2325581398918, "heading"=319.3651317408927}, {"position"=107.39754418076092, "velocity"=59.710511205114216, "acceleration"=-20.881877376827163, "jerk"=-930.2325581396076, "heading"=319.10559977855286}, {"position"=107.6957775737844, "velocity"=59.582846004276604, "acceleration"=-25.53304016752236, "jerk"=-930.2325581390392, "heading"=318.84728021128666}, {"position"=107.9933145012688, "velocity"=59.431924989485495, "acceleration"=-30.184202958221817, "jerk"=-930.2325581398918, "heading"=318.5902866988901}, {"position"=108.29003868414436, "velocity"=59.257748160740896, "acceleration"=-34.835365748919855, "jerk"=-930.2325581396076, "heading"=318.3347304869631}, {"position"=108.58583384334132, "velocity"=59.060315518042806, "acceleration"=-39.48652853961789, "jerk"=-930.2325581396076, "heading"=318.0807217536011}, {"position"=108.88058369978991, "velocity"=58.83962706139123, "acceleration"=-44.13769133031593, "jerk"=-930.2325581396076, "heading"=317.82836827734377}, {"position"=109.17417197442035, "velocity"=58.595682790786164, "acceleration"=-48.78885412101255, "jerk"=-930.2325581393234, "heading"=317.57777635889073}, {"position"=109.46648238816289, "velocity"=58.328482706227604, "acceleration"=-53.44001691171201, "jerk"=-930.2325581398918, "heading"=317.32905036246854}, {"position"=109.75739866194775, "velocity"=58.03802680771557, "acceleration"=-58.0911797024072, "jerk"=-930.2325581390392, "heading"=317.08229267197237}, {"position"=110.04680451670517, "velocity"=57.724315095250034, "acceleration"=-62.74234249310666, "jerk"=-930.2325581398918, "heading"=316.837603651552}, {"position"=110.33458367336537, "velocity"=57.38734756883102, "acceleration"=-67.39350528380328, "jerk"=-930.2325581393234, "heading"=316.595081610671}, {"position"=110.62064831818627, "velocity"=57.038510359528686, "acceleration"=-69.7674418604663, "jerk"=-474.78731533260543, "heading"=316.3547996705971}, {"position"=110.90496877696066, "velocity"=56.68967315022636, "acceleration"=-69.76744186046488, "jerk"=2.842170943040401e-10, "heading"=316.11677979780296}, {"position"=111.18754504968854, "velocity"=56.34083594092404, "acceleration"=-69.76744186046488, "jerk"=0.0, "heading"=315.88101880741357}, {"position"=111.4683771363699, "velocity"=55.99199873162171, "acceleration"=-69.76744186046488, "jerk"=0.0, "heading"=315.6475127800334}, {"position"=111.74746503700474, "velocity"=55.64316152231939, "acceleration"=-69.76744186046488, "jerk"=0.0, "heading"=315.41625708457485}, {"position"=112.02480875159308, "velocity"=55.294324313017064, "acceleration"=-69.76744186046488, "jerk"=0.0, "heading"=315.1872467015039}, {"position"=112.30040828013492, "velocity"=54.94548710371473, "acceleration"=-69.7674418604663, "jerk"=-2.842170943040401e-10, "heading"=314.96047584078}, {"position"=112.57426362263024, "velocity"=54.59664989441241, "acceleration"=-69.76744186046488, "jerk"=2.842170943040401e-10, "heading"=314.7359384196044}, {"position"=112.84637477907904, "velocity"=54.247812685110084, "acceleration"=-69.76744186046488, "jerk"=0.0, "heading"=314.51362753640615}, {"position"=113.11674174948133, "velocity"=53.89897547580776, "acceleration"=-69.76744186046488, "jerk"=0.0, "heading"=314.293536002611}, {"position"=113.38536453383712, "velocity"=53.550138266505435, "acceleration"=-69.76744186046488, "jerk"=0.0, "heading"=314.0756560630771}, {"position"=113.6522431321464, "velocity"=53.20130105720311, "acceleration"=-69.76744186046488, "jerk"=0.0, "heading"=313.8599799251029}, {"position"=113.91737754440915, "velocity"=52.85246384790078, "acceleration"=-69.7674418604663, "jerk"=-2.842170943040401e-10, "heading"=313.6464985353811}, {"position"=114.1807677706254, "velocity"=52.503626638598455, "acceleration"=-69.76744186046488, "jerk"=2.842170943040401e-10, "heading"=313.4352034724351}, {"position"=114.44241381079513, "velocity"=52.15478942929613, "acceleration"=-69.76744186046488, "jerk"=0.0, "heading"=313.22608506504076}, {"position"=114.70231566491836, "velocity"=51.805952219993806, "acceleration"=-69.76744186046488, "jerk"=0.0, "heading"=313.01913369395805}, {"position"=114.96047333299508, "velocity"=51.45711501069148, "acceleration"=-69.76744186046488, "jerk"=0.0, "heading"=312.8143393021986}, {"position"=115.21688681502528, "velocity"=51.10827780138916, "acceleration"=-69.76744186046488, "jerk"=0.0, "heading"=312.6116918269417}, {"position"=115.47155611100897, "velocity"=50.759440592086825, "acceleration"=-69.7674418604663, "jerk"=-2.842170943040401e-10, "heading"=312.4111803037664}, {"position"=115.72448122094615, "velocity"=50.4106033827845, "acceleration"=-69.76744186046488, "jerk"=2.842170943040401e-10, "heading"=312.2127941013041}, {"position"=115.97566214483682, "velocity"=50.06176617348218, "acceleration"=-69.76744186046488, "jerk"=0.0, "heading"=312.0165218287688}, {"position"=116.22509888268097, "velocity"=49.71292896417985, "acceleration"=-69.76744186046488, "jerk"=0.0, "heading"=311.82235216616334}, {"position"=116.47279143447861, "velocity"=49.36409175487753, "acceleration"=-69.76744186046488, "jerk"=0.0, "heading"=311.63027346652535}, {"position"=116.71873980022974, "velocity"=49.0152545455752, "acceleration"=-69.76744186046488, "jerk"=0.0, "heading"=311.44027377150866}, {"position"=116.96294397993437, "velocity"=48.66641733627287, "acceleration"=-69.7674418604663, "jerk"=-2.842170943040401e-10, "heading"=311.25234126530876}, {"position"=117.20540397359247, "velocity"=48.31758012697055, "acceleration"=-69.76744186046488, "jerk"=2.842170943040401e-10, "heading"=311.0664634034083}, {"position"=117.44611978120406, "velocity"=47.96874291766822, "acceleration"=-69.76744186046488, "jerk"=0.0, "heading"=310.8826281511684}, {"position"=117.68509140276915, "velocity"=47.6199057083659, "acceleration"=-69.76744186046488, "jerk"=0.0, "heading"=310.7008226644771}, {"position"=117.92231883828772, "velocity"=47.271068499063574, "acceleration"=-69.76744186046488, "jerk"=0.0, "heading"=310.5210343037638}, {"position"=118.15780208775979, "velocity"=46.92223128976125, "acceleration"=-69.76744186046488, "jerk"=0.0, "heading"=310.34325020828953}, {"position"=118.39154115118534, "velocity"=46.57339408045892, "acceleration"=-69.7674418604663, "jerk"=-2.842170943040401e-10, "heading"=310.16745765554117}, {"position"=118.62353602856437, "velocity"=46.224556871156594, "acceleration"=-69.76744186046488, "jerk"=2.842170943040401e-10, "heading"=309.99364342086966}, {"position"=118.8537867198969, "velocity"=45.87571966185427, "acceleration"=-69.76744186046488, "jerk"=0.0, "heading"=309.8217944701111}, {"position"=119.08229322518292, "velocity"=45.526882452551945, "acceleration"=-69.76744186046488, "jerk"=0.0, "heading"=309.6518974738787}, {"position"=119.30905554442242, "velocity"=45.17804524324962, "acceleration"=-69.76744186046488, "jerk"=0.0, "heading"=309.48393929118305}, {"position"=119.53407367761541, "velocity"=44.829208033947296, "acceleration"=-69.76744186046488, "jerk"=0.0, "heading"=309.31790663326524}, {"position"=119.75734762476189, "velocity"=44.48037082464497, "acceleration"=-69.76744186046488, "jerk"=0.0, "heading"=309.1537860738692}, {"position"=119.97887738586186, "velocity"=44.13153361534264, "acceleration"=-69.7674418604663, "jerk"=-2.842170943040401e-10, "heading"=308.99156405920604}, {"position"=120.19866296091533, "velocity"=43.782696406040316, "acceleration"=-69.76744186046488, "jerk"=2.842170943040401e-10, "heading"=308.83122748622554}, {"position"=120.41670434992227, "velocity"=43.43385919673799, "acceleration"=-69.76744186046488, "jerk"=0.0, "heading"=308.6727624954373}, {"position"=120.6330015528827, "velocity"=43.08502198743567, "acceleration"=-69.76744186046488, "jerk"=0.0, "heading"=308.51615604265055}, {"position"=120.84755456979663, "velocity"=42.73618477813334, "acceleration"=-69.76744186046488, "jerk"=0.0, "heading"=308.361394453281}, {"position"=121.06036340066404, "velocity"=42.38734756883102, "acceleration"=-69.76744186046488, "jerk"=0.0, "heading"=308.20846422835524}, {"position"=121.27142804548494, "velocity"=42.038510359528686, "acceleration"=-69.7674418604663, "jerk"=-2.842170943040401e-10, "heading"=308.05735205879796}, {"position"=121.48074850425932, "velocity"=41.68967315022636, "acceleration"=-69.76744186046488, "jerk"=2.842170943040401e-10, "heading"=307.90804456041195}, {"position"=121.6883247769872, "velocity"=41.34083594092404, "acceleration"=-69.76744186046488, "jerk"=0.0, "heading"=307.7605279627691}, {"position"=121.89415686366857, "velocity"=40.99199873162171, "acceleration"=-69.76744186046488, "jerk"=0.0, "heading"=307.61478955272236}, {"position"=122.09824476430342, "velocity"=40.643161522319396, "acceleration"=-69.76744186046346, "jerk"=2.842170943040401e-10, "heading"=307.47081550300396}, {"position"=122.30058847889175, "velocity"=40.29432431301707, "acceleration"=-69.76744186046488, "jerk"=-2.842170943040401e-10, "heading"=307.3285926797094}, {"position"=122.50118800743358, "velocity"=39.94548710371475, "acceleration"=-69.76744186046488, "jerk"=0.0, "heading"=307.1881079177526}, {"position"=122.7000433499289, "velocity"=39.59664989441242, "acceleration"=-69.76744186046488, "jerk"=0.0, "heading"=307.0493480268069}, {"position"=122.89715450637772, "velocity"=39.2478126851101, "acceleration"=-69.76744186046488, "jerk"=0.0, "heading"=306.9122997970263}, {"position"=123.09252147678001, "velocity"=38.89897547580777, "acceleration"=-69.7674418604663, "jerk"=-2.842170943040401e-10, "heading"=306.7769505491748}, {"position"=123.28614426113579, "velocity"=38.55013826650544, "acceleration"=-69.76744186046488, "jerk"=2.842170943040401e-10, "heading"=306.643286851614}, {"position"=123.47802285944506, "velocity"=38.20130105720312, "acceleration"=-69.76744186046488, "jerk"=0.0, "heading"=306.51129634609157}, {"position"=123.66815727170783, "velocity"=37.85246384790079, "acceleration"=-69.76744186046488, "jerk"=0.0, "heading"=306.38096585444106}, {"position"=123.85654749792407, "velocity"=37.50362663859847, "acceleration"=-69.76744186046488, "jerk"=0.0, "heading"=306.2522827481945}, {"position"=124.0431935380938, "velocity"=37.154789429296144, "acceleration"=-69.76744186046488, "jerk"=0.0, "heading"=306.1252344083087}, {"position"=124.22809539221703, "velocity"=36.80595221999381, "acceleration"=-69.7674418604663, "jerk"=-2.842170943040401e-10, "heading"=305.99980822933753}, {"position"=124.41125306029375, "velocity"=36.45711501069149, "acceleration"=-69.76744186046488, "jerk"=2.842170943040401e-10, "heading"=305.8759920364673}, {"position"=124.59266654232395, "velocity"=36.108277801389164, "acceleration"=-69.76744186046488, "jerk"=0.0, "heading"=305.75377321027435}, {"position"=124.77233583830764, "velocity"=35.75944059208684, "acceleration"=-69.76744186046488, "jerk"=0.0, "heading"=305.63313968588375}, {"position"=124.95026094824482, "velocity"=35.410603382784515, "acceleration"=-69.76744186046488, "jerk"=0.0, "heading"=305.51407912349424}, {"position"=125.12644187213549, "velocity"=35.06176617348219, "acceleration"=-69.76744186046488, "jerk"=0.0, "heading"=305.39657962681895}, {"position"=125.30087860997965, "velocity"=34.71292896417986, "acceleration"=-69.7674418604663, "jerk"=-2.842170943040401e-10, "heading"=305.2806293331508}, {"position"=125.47357116177729, "velocity"=34.364091754877535, "acceleration"=-69.76744186046488, "jerk"=2.842170943040401e-10, "heading"=305.1662164163246}, {"position"=125.64451952752842, "velocity"=34.01525454557521, "acceleration"=-69.76744186046488, "jerk"=0.0, "heading"=305.0533290895417}, {"position"=125.81372370723304, "velocity"=33.666417336272886, "acceleration"=-69.76744186046488, "jerk"=0.0, "heading"=304.94195560806344}, {"position"=125.98118370089115, "velocity"=33.31758012697056, "acceleration"=-69.76744186046488, "jerk"=0.0, "heading"=304.8320849731243}, {"position"=126.14689950850274, "velocity"=32.96874291766824, "acceleration"=-69.76744186046488, "jerk"=0.0, "heading"=304.7237052932544}, {"position"=126.31087113006782, "velocity"=32.619905708365906, "acceleration"=-69.7674418604663, "jerk"=-2.842170943040401e-10, "heading"=304.6168057055371}, {"position"=126.4730985655864, "velocity"=32.27106849906358, "acceleration"=-69.76744186046488, "jerk"=2.842170943040401e-10, "heading"=304.511375035957}, {"position"=126.63358181505846, "velocity"=31.922231289761257, "acceleration"=-69.76744186046488, "jerk"=0.0, "heading"=304.40740218159675}, {"position"=126.79232087848402, "velocity"=31.573394080458932, "acceleration"=-69.76744186046488, "jerk"=0.0, "heading"=304.3048762636769}, {"position"=126.94931575586305, "velocity"=31.224556871156604, "acceleration"=-69.7674418604656, "jerk"=-1.4210854715202004e-10, "heading"=304.203786800226}, {"position"=127.10456644719558, "velocity"=30.87571966185428, "acceleration"=-69.76744186046488, "jerk"=1.4210854715202004e-10, "heading"=304.10412293819155}, {"position"=127.2580729524816, "velocity"=30.526882452551952, "acceleration"=-69.7674418604656, "jerk"=-1.4210854715202004e-10, "heading"=304.00587409167224}, {"position"=127.40983527172111, "velocity"=30.178045243249635, "acceleration"=-69.76744186046346, "jerk"=4.263256414560601e-10, "heading"=303.90903020024746}, {"position"=127.5598534049141, "velocity"=29.829208033947303, "acceleration"=-69.7674418604663, "jerk"=-5.684341886080801e-10, "heading"=303.8135808641672}, {"position"=127.70812735206057, "velocity"=29.48037082464498, "acceleration"=-69.76744186046488, "jerk"=2.842170943040401e-10, "heading"=303.7195159227925}, {"position"=127.85465711316054, "velocity"=29.131533615342654, "acceleration"=-69.76744186046488, "jerk"=0.0, "heading"=303.6268254675477}, {"position"=127.999442688214, "velocity"=28.782696406040326, "acceleration"=-69.7674418604656, "jerk"=-1.4210854715202004e-10, "heading"=303.5354996533687}, {"position"=128.14248407722096, "velocity"=28.433859196738002, "acceleration"=-69.76744186046488, "jerk"=1.4210854715202004e-10, "heading"=303.4455286998202}, {"position"=128.2837812801814, "velocity"=28.085021987435677, "acceleration"=-69.76744186046488, "jerk"=0.0, "heading"=303.3569029847809}, {"position"=128.42333429709532, "velocity"=27.73618477813336, "acceleration"=-69.76744186046346, "jerk"=2.842170943040401e-10, "heading"=303.26961338780586}, {"position"=128.56114312796274, "velocity"=27.387347568831036, "acceleration"=-69.76744186046488, "jerk"=-2.842170943040401e-10, "heading"=303.18365005483076}, {"position"=128.69720777278363, "velocity"=27.03851035952871, "acceleration"=-69.76744186046488, "jerk"=0.0, "heading"=303.09900421176417}, {"position"=128.83152823155802, "velocity"=26.689673150226383, "acceleration"=-69.7674418604656, "jerk"=-1.4210854715202004e-10, "heading"=303.015666646266}, {"position"=128.9641045042859, "velocity"=26.34083594092406, "acceleration"=-69.76744186046488, "jerk"=1.4210854715202004e-10, "heading"=302.93362835226856}, {"position"=129.09493659096725, "velocity"=25.991998731621734, "acceleration"=-69.76744186046488, "jerk"=0.0, "heading"=302.8528805587971}, {"position"=129.2240244916021, "velocity"=25.643161522319406, "acceleration"=-69.7674418604656, "jerk"=-1.4210854715202004e-10, "heading"=302.7734145638479}, {"position"=129.35136820619044, "velocity"=25.294324313017082, "acceleration"=-69.76744186046488, "jerk"=1.4210854715202004e-10, "heading"=302.695221808442}, {"position"=129.47696773473228, "velocity"=24.945487103714758, "acceleration"=-69.76744186046488, "jerk"=0.0, "heading"=302.6182941856912}, {"position"=129.6008230772276, "velocity"=24.59664989441243, "acceleration"=-69.7674418604656, "jerk"=-1.4210854715202004e-10, "heading"=302.54262284984253}, {"position"=129.7229342336764, "velocity"=24.247812685110105, "acceleration"=-69.76744186046488, "jerk"=1.4210854715202004e-10, "heading"=302.46820025248985}, {"position"=129.8433012040787, "velocity"=23.89897547580778, "acceleration"=-69.76744186046488, "jerk"=0.0, "heading"=302.3950178899365}, {"position"=129.96192398843448, "velocity"=23.550138266505453, "acceleration"=-69.7674418604656, "jerk"=-1.4210854715202004e-10, "heading"=302.3230680039371}, {"position"=130.07880258674376, "velocity"=23.201301057203125, "acceleration"=-69.7674418604656, "jerk"=0.0, "heading"=302.2523429060741}, {"position"=130.19393699900652, "velocity"=22.8524638479008, "acceleration"=-69.76744186046488, "jerk"=1.4210854715202004e-10, "heading"=302.18283497805544}, {"position"=130.30732722522276, "velocity"=22.503626638598476, "acceleration"=-69.76744186046488, "jerk"=0.0, "heading"=302.1145366719725}, {"position"=130.4189732653925, "velocity"=22.154789429296148, "acceleration"=-69.7674418604656, "jerk"=-1.4210854715202004e-10, "heading"=302.0474405105231}, {"position"=130.52887511951573, "velocity"=21.805952219993824, "acceleration"=-69.76744186046488, "jerk"=1.4210854715202004e-10, "heading"=301.9815392041727}, {"position"=130.63703278759243, "velocity"=21.4571150106915, "acceleration"=-69.76744186046488, "jerk"=0.0, "heading"=301.91682597908436}, {"position"=130.74344626962264, "velocity"=21.10827780138917, "acceleration"=-69.7674418604656, "jerk"=-1.4210854715202004e-10, "heading"=301.85329340794544}, {"position"=130.84811556560632, "velocity"=20.759440592086847, "acceleration"=-69.76744186046488, "jerk"=1.4210854715202004e-10, "heading"=301.79093473890276}, {"position"=130.9510406755435, "velocity"=20.410603382784522, "acceleration"=-69.76744186046488, "jerk"=0.0, "heading"=301.7297434819884}, {"position"=131.05222159943418, "velocity"=20.061766173482194, "acceleration"=-69.7674418604656, "jerk"=-1.4210854715202004e-10, "heading"=301.66971274424935}, {"position"=131.15165833727832, "velocity"=19.71292896417987, "acceleration"=-69.76744186046488, "jerk"=1.4210854715202004e-10, "heading"=301.6108360483036}, {"position"=131.24935088907597, "velocity"=19.364091754877546, "acceleration"=-69.76744186046488, "jerk"=0.0, "heading"=301.5531070296862}, {"position"=131.3452992548271, "velocity"=19.015254545575218, "acceleration"=-69.7674418604656, "jerk"=-1.4210854715202004e-10, "heading"=301.4965197044973}, {"position"=131.43950343453173, "velocity"=18.666417336272893, "acceleration"=-69.76744186046488, "jerk"=1.4210854715202004e-10, "heading"=301.4410675715969}, {"position"=131.53196342818984, "velocity"=18.31758012697057, "acceleration"=-69.76744186046488, "jerk"=0.0, "heading"=301.386744767688}, {"position"=131.62267923580143, "velocity"=17.96874291766824, "acceleration"=-69.7674418604656, "jerk"=-1.4210854715202004e-10, "heading"=301.33354542712135}, {"position"=131.71165085736652, "velocity"=17.619905708365916, "acceleration"=-69.76744186046488, "jerk"=1.4210854715202004e-10, "heading"=301.28146390151846}, {"position"=131.7988782928851, "velocity"=17.271068499063592, "acceleration"=-69.76744186046488, "jerk"=0.0, "heading"=301.2304943551513}, {"position"=131.88436154235714, "velocity"=16.922231289761267, "acceleration"=-69.76744186046488, "jerk"=0.0, "heading"=301.1806313566016}, {"position"=131.9681006057827, "velocity"=16.57339408045894, "acceleration"=-69.7674418604656, "jerk"=-1.4210854715202004e-10, "heading"=301.1318695416856}, {"position"=132.05009548316173, "velocity"=16.224556871156615, "acceleration"=-69.76744186046488, "jerk"=1.4210854715202004e-10, "heading"=301.0842036133755}, {"position"=132.13034617449426, "velocity"=15.875719661854289, "acceleration"=-69.76744186046524, "jerk"=-7.105427357601002e-11, "heading"=301.0376283417049}, {"position"=132.20885267978028, "velocity"=15.526882452551963, "acceleration"=-69.76744186046524, "jerk"=0.0, "heading"=300.9921387774887}, {"position"=132.28561499901977, "velocity"=15.178045243249636, "acceleration"=-69.76744186046524, "jerk"=0.0, "heading"=300.94773011575586}, {"position"=132.36063313221277, "velocity"=14.829208033947312, "acceleration"=-69.76744186046488, "jerk"=7.105427357601002e-11, "heading"=300.9043972691833}, {"position"=132.43390707935924, "velocity"=14.480370824644986, "acceleration"=-69.76744186046524, "jerk"=-7.105427357601002e-11, "heading"=300.8621357458646}, {"position"=132.50543684045923, "velocity"=14.131533615342661, "acceleration"=-69.76744186046488, "jerk"=7.105427357601002e-11, "heading"=300.82094105643796}, {"position"=132.57522241551268, "velocity"=13.782696406040335, "acceleration"=-69.76744186046524, "jerk"=-7.105427357601002e-11, "heading"=300.78080856734226}, {"position"=132.64326380451962, "velocity"=13.43385919673801, "acceleration"=-69.76744186046488, "jerk"=7.105427357601002e-11, "heading"=300.74173399502655}, {"position"=132.70956100748006, "velocity"=13.085021987435685, "acceleration"=-69.76744186046524, "jerk"=-7.105427357601002e-11, "heading"=300.703713120418}, {"position"=132.77411402439398, "velocity"=12.736184778133358, "acceleration"=-69.76744186046524, "jerk"=0.0, "heading"=300.6667417887859}, {"position"=132.8369228552614, "velocity"=12.387347568831034, "acceleration"=-69.76744186046488, "jerk"=7.105427357601002e-11, "heading"=300.6308161733167}, {"position"=132.8979875000823, "velocity"=12.038510359528708, "acceleration"=-69.76744186046524, "jerk"=-7.105427357601002e-11, "heading"=300.59593235674174}, {"position"=132.9573079588567, "velocity"=11.689673150226382, "acceleration"=-69.76744186046524, "jerk"=0.0, "heading"=300.5620863325457}, {"position"=133.01488423158457, "velocity"=11.340835940924057, "acceleration"=-69.76744186046488, "jerk"=7.105427357601002e-11, "heading"=300.5292748156799}, {"position"=133.07071631826594, "velocity"=10.991998731621731, "acceleration"=-69.76744186046524, "jerk"=-7.105427357601002e-11, "heading"=300.49749405623663}, {"position"=133.12480421890078, "velocity"=10.643161522319405, "acceleration"=-69.76744186046524, "jerk"=0.0, "heading"=300.4667405864266}, {"position"=133.17714793348912, "velocity"=10.29432431301708, "acceleration"=-69.76744186046488, "jerk"=7.105427357601002e-11, "heading"=300.43701117060044}, {"position"=133.22774746203095, "velocity"=9.945487103714754, "acceleration"=-69.76744186046524, "jerk"=-7.105427357601002e-11, "heading"=300.40830263501607}, {"position"=133.27660280452628, "velocity"=9.596649894412428, "acceleration"=-69.76744186046524, "jerk"=0.0, "heading"=300.38061186770545}, {"position"=133.32371396097508, "velocity"=9.247812685110103, "acceleration"=-69.76744186046488, "jerk"=7.105427357601002e-11, "heading"=300.353935818335}, {"position"=133.36908093137737, "velocity"=8.898975475807777, "acceleration"=-69.76744186046524, "jerk"=-7.105427357601002e-11, "heading"=300.32827152482145}, {"position"=133.41270371573316, "velocity"=8.550138266505451, "acceleration"=-69.76744186046524, "jerk"=0.0, "heading"=300.3036166962871}, {"position"=133.45458231404243, "velocity"=8.201301057203127, "acceleration"=-69.76744186046488, "jerk"=7.105427357601002e-11, "heading"=300.2799679992812}, {"position"=133.4947167263052, "velocity"=7.8524638479008, "acceleration"=-69.76744186046524, "jerk"=-7.105427357601002e-11, "heading"=300.25732355193855}, {"position"=133.53310695252145, "velocity"=7.503626638598476, "acceleration"=-69.76744186046488, "jerk"=7.105427357601002e-11, "heading"=300.23568048084536}, {"position"=133.56975299269118, "velocity"=7.15478942929615, "acceleration"=-69.76744186046524, "jerk"=-7.105427357601002e-11, "heading"=300.2150365304659}, {"position"=133.6046548468144, "velocity"=6.805952219993824, "acceleration"=-69.76744186046524, "jerk"=0.0, "heading"=300.19538954477844}, {"position"=133.63781251489112, "velocity"=6.457115010691498, "acceleration"=-69.76744186046506, "jerk"=3.694822225952521e-11, "heading"=300.1767374274448}, {"position"=133.6692259969213, "velocity"=6.108277801389173, "acceleration"=-69.76744186046506, "jerk"=0.0, "heading"=300.1590781417043}, {"position"=133.698895292905, "velocity"=5.759440592086847, "acceleration"=-69.76744186046524, "jerk"=-3.694822225952521e-11, "heading"=300.1424097102642}, {"position"=133.72682040284218, "velocity"=5.4106033827845215, "acceleration"=-69.76744186046506, "jerk"=3.694822225952521e-11, "heading"=300.12673045757765}, {"position"=133.75300132673286, "velocity"=5.061766173482196, "acceleration"=-69.76744186046506, "jerk"=0.0, "heading"=300.1120387651637}, {"position"=133.777438064577, "velocity"=4.71292896417987, "acceleration"=-69.76744186046524, "jerk"=-3.694822225952521e-11, "heading"=300.098332830727}, {"position"=133.80013061637464, "velocity"=4.364091754877545, "acceleration"=-69.76744186046506, "jerk"=3.694822225952521e-11, "heading"=300.0856112986762}, {"position"=133.82107898212578, "velocity"=4.015254545575219, "acceleration"=-69.76744186046506, "jerk"=0.0, "heading"=300.0738729591331}, {"position"=133.8402831618304, "velocity"=3.6664173362728936, "acceleration"=-69.76744186046515, "jerk"=-1.9895196601282805e-11, "heading"=300.0631163283404}, {"position"=133.85774315548852, "velocity"=3.3175801269705683, "acceleration"=-69.76744186046506, "jerk"=1.9895196601282805e-11, "heading"=300.05334030572544}, {"position"=133.87345896310012, "velocity"=2.9687429176682425, "acceleration"=-69.76744186046515, "jerk"=-1.9895196601282805e-11, "heading"=300.0445438489431}, {"position"=133.8874305846652, "velocity"=2.6199057083659167, "acceleration"=-69.76744186046515, "jerk"=0.0, "heading"=300.03672597381893}, {"position"=133.89968648551144, "velocity"=2.2824546301337705, "acceleration"=-67.49021564642925, "jerk"=455.4452428071812, "heading"=300.0298699935373}, {"position"=133.9103132705014, "velocity"=1.9682593658551124, "acceleration"=-62.839052855731616, "jerk"=930.2325581395265, "heading"=300.02392689439074}, {"position"=133.91942721870487, "velocity"=1.6773199155299428, "acceleration"=-58.18789006503393, "jerk"=930.2325581395365, "heading"=300.01883062945313}, {"position"=133.9271446091916, "velocity"=1.4096362791582615, "acceleration"=-53.53672727433625, "jerk"=930.2325581395365, "heading"=300.01451631883816}, {"position"=133.93358172103135, "velocity"=1.1652084567400687, "acceleration"=-48.88556448363857, "jerk"=930.2325581395365, "heading"=300.0109180200833}, {"position"=133.93885483329387, "velocity"=0.944036448275364, "acceleration"=-44.23440169294093, "jerk"=930.232558139528, "heading"=300.00797084463125}, {"position"=133.94308022504896, "velocity"=0.7461202537641479, "acceleration"=-39.583238902243224, "jerk"=930.2325581395407, "heading"=300.0056095382167}, {"position"=133.94637417536637, "velocity"=0.5714598732064201, "acceleration"=-34.93207611154556, "jerk"=930.2325581395322, "heading"=300.00376883429635}, {"position"=133.9488529633159, "velocity"=0.4200553066021807, "acceleration"=-30.28091332084788, "jerk"=930.2325581395365, "heading"=300.00238369935244}, {"position"=133.95063286796727, "velocity"=0.29190655395142967, "acceleration"=-25.629750530150208, "jerk"=930.2325581395344, "heading"=300.0013891210427}, {"position"=133.95183016839027, "velocity"=0.187013615254167, "acceleration"=-20.978587739452536, "jerk"=930.2325581395344, "heading"=300.0007201026366}, {"position"=133.9525611436547, "velocity"=0.10537649051039268, "acceleration"=-16.32742494875486, "jerk"=930.2325581395351, "heading"=300.0003116583051}, {"position"=133.95294207283027, "velocity"=0.04699517972010674, "acceleration"=-11.676262158057186, "jerk"=930.2325581395347, "heading"=300.0000988092646}, {"position"=133.95308923498678, "velocity"=0.011869682883309187, "acceleration"=-7.025099367359511, "jerk"=930.2325581395351, "heading"=300.0000165807764}, {"position"=133.953118909194, "velocity"=0.0, "acceleration"=-2.3739365766618374, "jerk"=930.2325581395347, "heading"=300.0000000000004}, {"position"=133.953118909194, "velocity"=0.0, "acceleration"=0.0, "jerk"=474.7873153323675, "heading"=300.0000000000004}]
  out "Position":cluster{dbl[], dbl[]}[](graph)
  out "error out":errorcluster
  in  "path":T3[](array[typedef])=[{"x"=0.0, "y"=246.0, "angle"=0.0}, {"x"=120.0, "y"=210.0, "angle"=-60.0}]
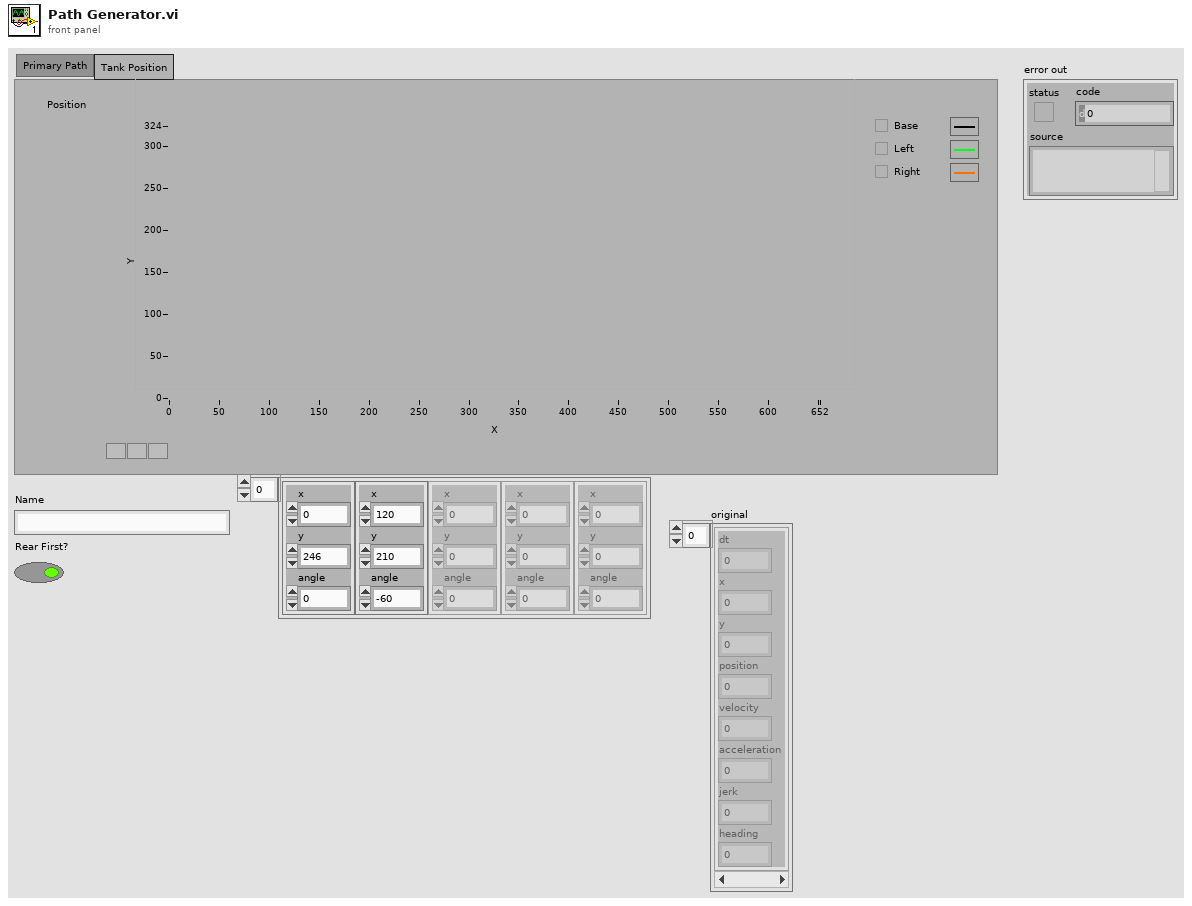
[diagram p1: front panel]
types:
  T1 = typedef "Pathfinder.lvlib/Segment.ctl" = cluster{"dt":dbl, "x":dbl, "y":dbl, "position":dbl, "velocity":dbl, "acceleration":dbl, "jerk":dbl, "heading":dbl}
  T2 = cluster{"position":dbl, "velocity":dbl, "acceleration":dbl, "jerk":dbl, "heading":dbl}[]
  T3 = typedef "Pathfinder.lvlib/Waypoint.ctl" = cluster{"x":dbl, "y":dbl, "angle":dbl}
  T4 = typedef "Constants.lvlib/Constants.ctl" = cluster{"Port Layout":cluster{"RightMotorInverted":bool, "LeftMotorInverted":bool, "Left Motors":T5, "Right Motors":T5, "Auton List":string[], "XBOX Port":T6, "Encoder L A":T7, "Encoder L B":T7, "Encoder R A":T7, "Encoder R B":T7, "L Encoder Inverse":bool, "R Encoder Inverse":bool, "Drive Distance per Count":dbl, "Gyro Bus":T8, "Fuel Roller 1":T5, "Front Roller":T5, "Gear Flipper":T5, "Climber 1":T5, "Fuel Roller Invert":bool, "Front Roller Invert":bool, "Gear Flipper Invert":bool, "Climber Invert":bool, "PCM":u8, "Fuel Roller 2":T5, "Gear Sensor":T9, "Gear Release Fwd":T10, "Gear Release Rvrs":T10, "Fuel Arm Fwd":T10, "Fuel Arm Rvrs":T10, "Shifter Fwrd":T10, "Shifter Rvrs":T10, "Climber 2":T5, "PDP":u8, "Shooter Front Channel":u8, "Shooter Rear Channel":u8, "Shooter Feed Channel":u8, "Camera Servo":T5, "Gear Servo":T5, "Gear Puncher Fwrd":T10, "Gear Puncher Rvrs":T10, "Shooter Inverse":bool, "Ring Light Switch":T7}, "Drive Constants":cluster{"Wheelbase In.":dbl, "Max Velocity (In/sec)":dbl, "Max Accel (In/sec^2)":dbl, "Max Jerk (In/sec^3)":dbl, "Path dt":dbl, "Path Sample Count":i32, "Deadband":dbl}, "Arm System":cluster{"Front Roller Gear Speed":dbl, "Front Roller Fuel Speed":dbl, "Gear Flipper Speed":dbl, "Fuel Roller Speed":dbl, "Gear Release Wait (ms)":i32, "Gear Sensor Threshold":dbl, "Flappy Open Angle":i32, "Flappy Close Angle":i32, "Ramp Rate (EGU/min)":dbl}, "Shooter":cluster{"Shooter Wheels":cluster{"P":dbl, "I":dbl, "D":dbl, "F":dbl, "IZone":dbl}, "Feeder":cluster{"P":dbl, "I":dbl, "D":dbl, "F":dbl, "IZone":dbl}, "Front Shooter RPM":dbl, "Rear Shooter RPM":dbl, "Agitator Speed":dbl, "Feeder Speed":dbl, "Shooter CPR":u32, "Feeder CPR":u32}, "Vision":cluster{"High Goal Height (in.)":dbl, "Low Goal Height (in.)":dbl, "Camera Height High (in.)":dbl, "Camera Height Low (in.)":dbl, "Servo Pitch Gear (deg)":dbl, "Camera Yaw (deg)":dbl, "Servo Gear":i32, "Servo Boiler":i32, "Servo Pitch Boiler (deg)":dbl}}
  T5 = typedef "FPGA_DIOPWMChannel.ctl" = enum8{"PWM 0", "PWM 1", "PWM 2", "PWM 3", "PWM 4", "PWM 5", "PWM 6", "PWM 7", "PWM 8", "PWM 9", "PWM MXP 0", "PWM MXP 1", "PWM MXP 2", "PWM MXP 3", "PWM MXP 4", "PWM MXP 5", "PWM MXP 6", "PWM MXP 7", "PWM MXP 8", "PWM MXP 9", "Invalid"}
  T6 = typedef "WPI_JoystickDeviceEnum.ctl" = enum16{"USB 0", "USB 1", "USB 2", "USB 3", "USB 4", "USB 5"}
  T7 = typedef "FPGA_DIOChannel.ctl" = enum8{"DIO 0", "DIO 1", "DIO 2", "DIO 3", "DIO 4", "DIO 5", "DIO 6", "DIO 7", "DIO 8", "DIO 9", "DIO MXP 0", "DIO MXP 1", "DIO MXP 2", "DIO MXP 3", "DIO MXP 4", "DIO MXP 5", "DIO MXP 6", "DIO MXP 7", "DIO MXP 8", "DIO MXP 9", "DIO MXP 10", "DIO MXP 11", "DIO MXP 12", "DIO MXP 13", "DIO MXP 14", "DIO MXP 15", "SPI Port CS1", "SPI Port CS2", "SPI Port CS3", "SPI Port MISO", "SPI Port MOSI", "Invalid"}
  T8 = typedef "spi_bus.ctl" = enum16{"SPI On-Board, CS0", "SPI On-Board, CS1", "SPI On-Board, CS2", "SPI On-Board, CS3", "SPI MXP", "Invalid"}
  T9 = typedef "FPGA_AIChannel.ctl" = enum8{"AI 0", "AI 1", "AI 2", "AI 3", "AI MXP 0", "AI MXP 1", "AI MXP 2", "AI MXP 3", "Invalid"}
  T10 = typedef "WPI_SolenoidChannel.ctl" = enum8{"Solenoid 0", "Solenoid 1", "Solenoid 2", "Solenoid 3", "Solenoid 4", "Solenoid 5", "Solenoid 6", "Solenoid 7", "Invalid"}
  T11 = cluster{"position":dbl, "velocity":dbl, "acceleration":dbl, "jerk":dbl, "heading":dbl}
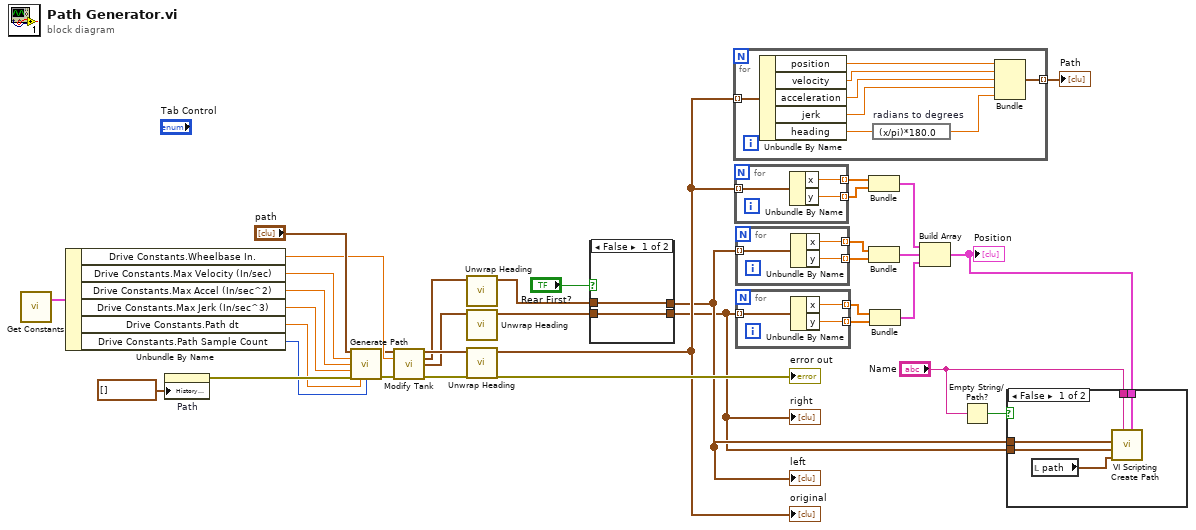
[diagram p0: block diagram]
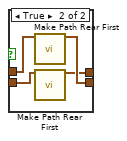
[diagram p3: hidden frame]
diagram:
  n1 = call "Get Constants.vi"() -> ("Constants"=w20:T4)  [unwired: 3 in]
  n2 = Unbundle By Name(w20) -> ("Drive Constants.Wheelbase In."=w19:dbl, "Drive Constants.Max Velocity (In/sec)"=w18:dbl, "Drive Constants.Max Accel (In/sec^2)"=w17:dbl, "Drive Constants.Max Jerk (In/sec^3)"=w16:dbl, "Drive Constants.Path dt"=w15:dbl, "Drive Constants.Path Sample Count"=w14:i32)
  n3 = property on="Path" class="WFChart (strict)"("History Data"=T2 []) -> (error out=w22:errorcluster)  [unwired: 2 in, 1 out]
  n4 = call "Generate Path.vi"("path"="path", "max_velocity"=w18, "max_acceleration"=w17, "max_jerk"=w16, "error in"=w22, "dt (.001)"=w15, "sample_count (100000)"=w14) -> ("Segments"=w10:T1[], "error out"=w11:errorcluster)  [unwired: 7 in]
  n5 = call "Modify Tank.vi"("Original"=w10, "wheelbase_width"=w19, "error in"=w11) -> ("original"=w27:T1[], "left"=w9:T1[], "right"=w12:T1[], "error out"=→"error out":errorcluster)  [unwired: 9 in]
  n6 = call "Unwrap Heading.vi"("input"=w9) -> ("output"=w8:T1[])  [unwired: 10 in]
  n7 = call "Unwrap Heading.vi"("input"=w12) -> ("output"=w7:T1[])  [unwired: 10 in]
  n8 = call "Unwrap Heading.vi"("input"=w27) -> ("output"=w6:T1[])  [unwired: 10 in]
  "original" <- w6
  n9 = case shown="False" "Rear First?" {
    tunnel: w8 -> [w37 w41]
    tunnel: [w37 w38] -> w2
    tunnel: w7 -> [w36 w39]
    tunnel: [w36 w40] -> w1
    frame False {
    }
    frame True {
      n10 = call "Make Path Rear First.vi"("Segments in"=w41) -> ("Segments out"=w40:T1[])  [unwired: 13 in, 1 out]
      n11 = call "Make Path Rear First.vi"("Segments in"=w39) -> ("Segments out"=w38:T1[])  [unwired: 13 in, 1 out]
    }
  }
  "right" <- w1
  "left" <- w2
  n12 = for {
    tunnel: w6 -> [w49] mode=indexing
    tunnel: [w43] -> w34 mode=indexing
    n13 = Unbundle By Name(w49) -> ("position"=w48:dbl, "velocity"=w47:dbl, "acceleration"=w46:dbl, "jerk"=w45:dbl, "heading"=w44:dbl)
    n14 = expression code="(x/pi)*180.0" "radians to degrees"(w44) -> (w42:dbl)
    n15 = Bundle("position"=w48, "velocity"=w47, "acceleration"=w46, "jerk"=w45, "heading"=w42) -> (w43:T11)  [unwired: 1 in]
  }
  "Path" <- w34
  n16 = for {
    tunnel: w6 -> [w52] mode=indexing
    tunnel: [w51] -> w26 mode=indexing
    tunnel: [w50] -> w25 mode=indexing
    n17 = Unbundle By Name(w52) -> ("x"=w51:dbl, "y"=w50:dbl)
  }
  n18 = for {
    tunnel: w2 -> [w55] mode=indexing
    tunnel: [w54] -> w33 mode=indexing
    tunnel: [w53] -> w32 mode=indexing
    n19 = Unbundle By Name(w55) -> ("x"=w54:dbl, "y"=w53:dbl)
  }
  n20 = for {
    tunnel: [w58] -> w31 mode=indexing
    tunnel: [w57] -> w30 mode=indexing
    tunnel: w1 -> [w56] mode=indexing
    n21 = Unbundle By Name(w56) -> ("x"=w58:dbl, "y"=w57:dbl)
  }
  n22 = Bundle(w26, w25) -> (w24:cluster{dbl[], dbl[]})  [unwired: 1 in]
  n23 = Bundle(w33, w32) -> (w28:cluster{dbl[], dbl[]})  [unwired: 1 in]
  n24 = Bundle(w31, w30) -> (w29:cluster{dbl[], dbl[]})  [unwired: 1 in]
  n25 = Build Array(w24, w28, w29) -> (w5:cluster{dbl[], dbl[]}[])
  "Position" <- w5
  n26 = Empty String/Path?(string/path="Name") -> (empty?=w3:bool)
  n27 = case shown="False" w3 {
    tunnel: w1 -> [w63 _]
    tunnel: w2 -> [w61 _]
    tunnel: w5 -> [w60 _]
    tunnel: "Name" -> [w59 _]
    frame False {
      n28 = local read "path"() -> (w62:T3[])
      n29 = call "VI Scripting Create Path.vi"("Porition"=w60, "Name"=w59, "path"=w62, "right"=w63, "left"=w61) -> ()  [unwired: 7 in]
    }
    frame True {
    }
  }
